vi "main4ChBK.vi"() -> ()   [LabVIEW 2024]
doc: "Main VI for FLS imaging system."
uses:
  <userlib>/_OpenG.lib/file/file.llb/openg_file.lvlib
  <vilib>/event_ctls.llb/usereventprio.ctl
  <instrlib>/niScope/Acquire/Fetch/niScope Multi Fetch Binary 16.vi
  <instrlib>/niScope/Controls/niScope trigger source.ctl
  <userlib>/_OpenG.lib/time/time.llb/openg_time.lvlib
  LaguerreDeconLib/DeconEngineClass/LaguerreDeconEngineClass.lvclass
  SubVI/GlobalVariables.vi
  SubVI/LabJack/LJ Pin Setting.ctl
  <vilib>/Utility/error.llb/DialogType.ctl
  <vilib>/Analysis/NI_AALBase.lvlib
  <vilib>/Utility/miscctls.llb/LVMinMaxIncTypeDef.ctl
  <vilib>/Analysis/baseanly.llb/Mean (DBL).vi
  <vilib>/Utility/miscctls.llb/LVPointTypeDef.ctl
  SubVI/APD/APDClass.lvclass
  ConfigFiles/AimingBeamVideoConfig.ctl
  <vilib>/addons/control/pid/NI_PID_pid.lvlib
  <vilib>/addons/control/pid/pid.llb/PID (DBL).vi
  <vilib>/Instr/_visa.llb/VISA Configure Serial Port (Instr).vi
  SubVI/DigitizerConfiguration/FLImDAQ.ctl
panel:
  out "Record Backlog 2":i32
  in  "Auto gain ch4":bool=TRUE caption="Auto gain ch3"
  in  "V 4":dbl caption="Gain 3" min=0.0 max=4.66 step=0.1
  out "Gain4":dbl
  out "Lifetime 4":dbl caption="Lifetime 3"
  out "IntR4":dbl format="%#_2g"
  out "SNR4":dbl format="%#_3g"
  out "Channel 4":dbl[][](graph) caption="Channel 3"
  out "RunStartTime":u32
  out "Dig1 Temp":dbl
  out "Dig2 Temp":dbl
  out "Visualization PC video source":T1
  in  "V target(1.0)":dbl=1.0 caption="V target(1.5)" min=0.3 max=1.5 step=0.1 format="%#_4g"
  out "SNR3":dbl format="%#_3g"
  out "SNR2":dbl format="%#_3g"
  out "SNR1":dbl format="%#_3g"
  in  "Show BG removed?":bool=TRUE
  out "IntR3":dbl format="%#_2g"
  out "IntR2":dbl format="%#_2g"
  out "IntR1":dbl format="%#_2g"
  in  "Video Display":bool
  out "Gain3":dbl
  out "Gain2":dbl
  out "Gain1":dbl
  in  "Skip Data Save?":bool
  out "Aq Loop?":bool
  out "ML?":bool
  out "aquisition loop Error Out":errorcluster
  out "Laser f (Hz)":dbl
  out "Record Backlog":i32
  out "Fetch Record #":i32
  out "Sync Success?":bool
  out "Disclamer":picture
  out "Calibration #":i8
  out "BG #":i8
  in  "TCP Connect":bool
  out "Help":string
  in  "355nm Laser toggle":bool caption="355nm 460Hz"
  in  "Cali&iRF alignment":bool
  in  "Background":bool
  in  "Aiming beam toggle":bool caption="445nm 15Hz 20mA"
  out "Lifetime 3":dbl
  out "Lifetime 2":dbl
  in  "Auto gain ch3":bool=TRUE
  in  "Auto gain ch2":bool=TRUE
  in  "Auto gain ch1":bool=TRUE
  out "Run #":i8
  in  "StopButton":bool caption="Stop"
  out "Aquisition Status:":bool
  in  "StartButton":bool caption="Start"
  in  "V 3":dbl caption="Gain 3" min=0.0 max=4.65 step=0.1
  in  "V 2":dbl caption="Gain 2" min=0.0 max=4.59 step=0.1
  out "Lifetime 1":dbl
  in  "V 1":dbl caption="Gain 1" min=0.0 max=4.63 step=0.1 format="%#_4g"
  in  "Video Source":enum32{"Camera", "FrameGrabber"}(radio)
  out "Case #":string
  out "System Hardware Connection Status":T2
  out "Channel 3":dbl[][](graph)
  out "Channel 2":dbl[][](graph)
  out "Channel 1":dbl[][](graph)
  in  "Tab Control":T3(tab)
  out "display loop timing(ms)":u32
  out "Aquisition loop timing(ms)":u32 format="%.2f"
  out "DisplayLoop":i32
  out "PID loop":i32 caption="processing loop"
  out "PID loop timing(ms)":u32 caption="processing loop timing(ms)"
  out "Communication loop(ms)":u32
  out "laser EM lamp V":dbl format="%0.6f"
  out "Decon Loop timing (ms)":dbl
  out "Auisition Loop idx":i32
  out "LJ process (ms)":u32
  out "LJ time(ms)":u32[](array[numeric])
  in  "Show BG":bool
  out "iRF length":i32
  out "BG length":i32
  out "data length":i32
  out "SysConfigCluster":T4
  out "LJ Pinout":T5={"Ch1 Bias"="DAC0", "Ch2 Bias"="DAC1", "Ch3 Bias"="DAC2", "Ch4 Bias"="DAC0", "355 PWM"="FIO0", "AimingBeam PWM"="FIO2", "Laser Ready"="FIO3", "Interlock"="FIO1", "Laser Start/Stop"="FIO1", "Red LED"="FIO1", "Green LED"="DIO3", "Foot Pedal"="DIO15"}
  out "FLImDAQ":T6={"Digitizer 1"="", "Digitizer 2"="", "Channel"=enum."Channel 0", "trigger source"="VAL_EXTERNAL", "trigger level"=0.5, "trigger delay"=1.35e-07, "min sample rate"=12500000000.0, "min record length"=2500, "vertical range"=1.0, "vertical offset"=-0.25, "Waveform to Avg"=2000} caption="FLIm DAQ Configuration" {"trigger delay" format="%^#.4e"; "trigger level" min=0.0 max=3.5 step=0.5 format="%.2f"; "vertical offset" format="%.4f"; "vertical range" format="%.2f"; "min sample rate" format="%#.2p"}
  in  "Sys Reconfig":bool
  out "data out(communcation loop)":string
  out "PID loop error out":errorcluster caption="processing Error Out"
  out "decon error out":errorcluster
  out "Laser Rep Rate":dbl
  out "V4 Size":i32 caption="V3 Size"
  in  "Data Class":enum16{"Data", "BG", "Cali"}(ring)
  out "V1 Size":i32
  out "V2 Size":i32
  out "V3 Size":i32
  out "data Size":i32[](array[numeric])
  out "State log":string
  in  "Ch4 PID gains":T8={"proportional gain (Kc)"=30.0, "integral time (Ti, min)"=0.0003, "derivative time (Td, min)"=1e-05}
  in  "Ch3 PID gains":T8={"proportional gain (Kc)"=30.0, "integral time (Ti, min)"=0.0003, "derivative time (Td, min)"=1e-05}
  in  "Ch2 PID gains":T8={"proportional gain (Kc)"=30.0, "integral time (Ti, min)"=0.0003, "derivative time (Td, min)"=1e-05}
  in  "Ch1 PID gains":T8={"proportional gain (Kc)"=30.0, "integral time (Ti, min)"=0.0003, "derivative time (Td, min)"=1e-05}
  in  "Quit":bool
  in  "Radio Buttons":T9(radio)=enum."Ch2" caption="DeCon Chan"
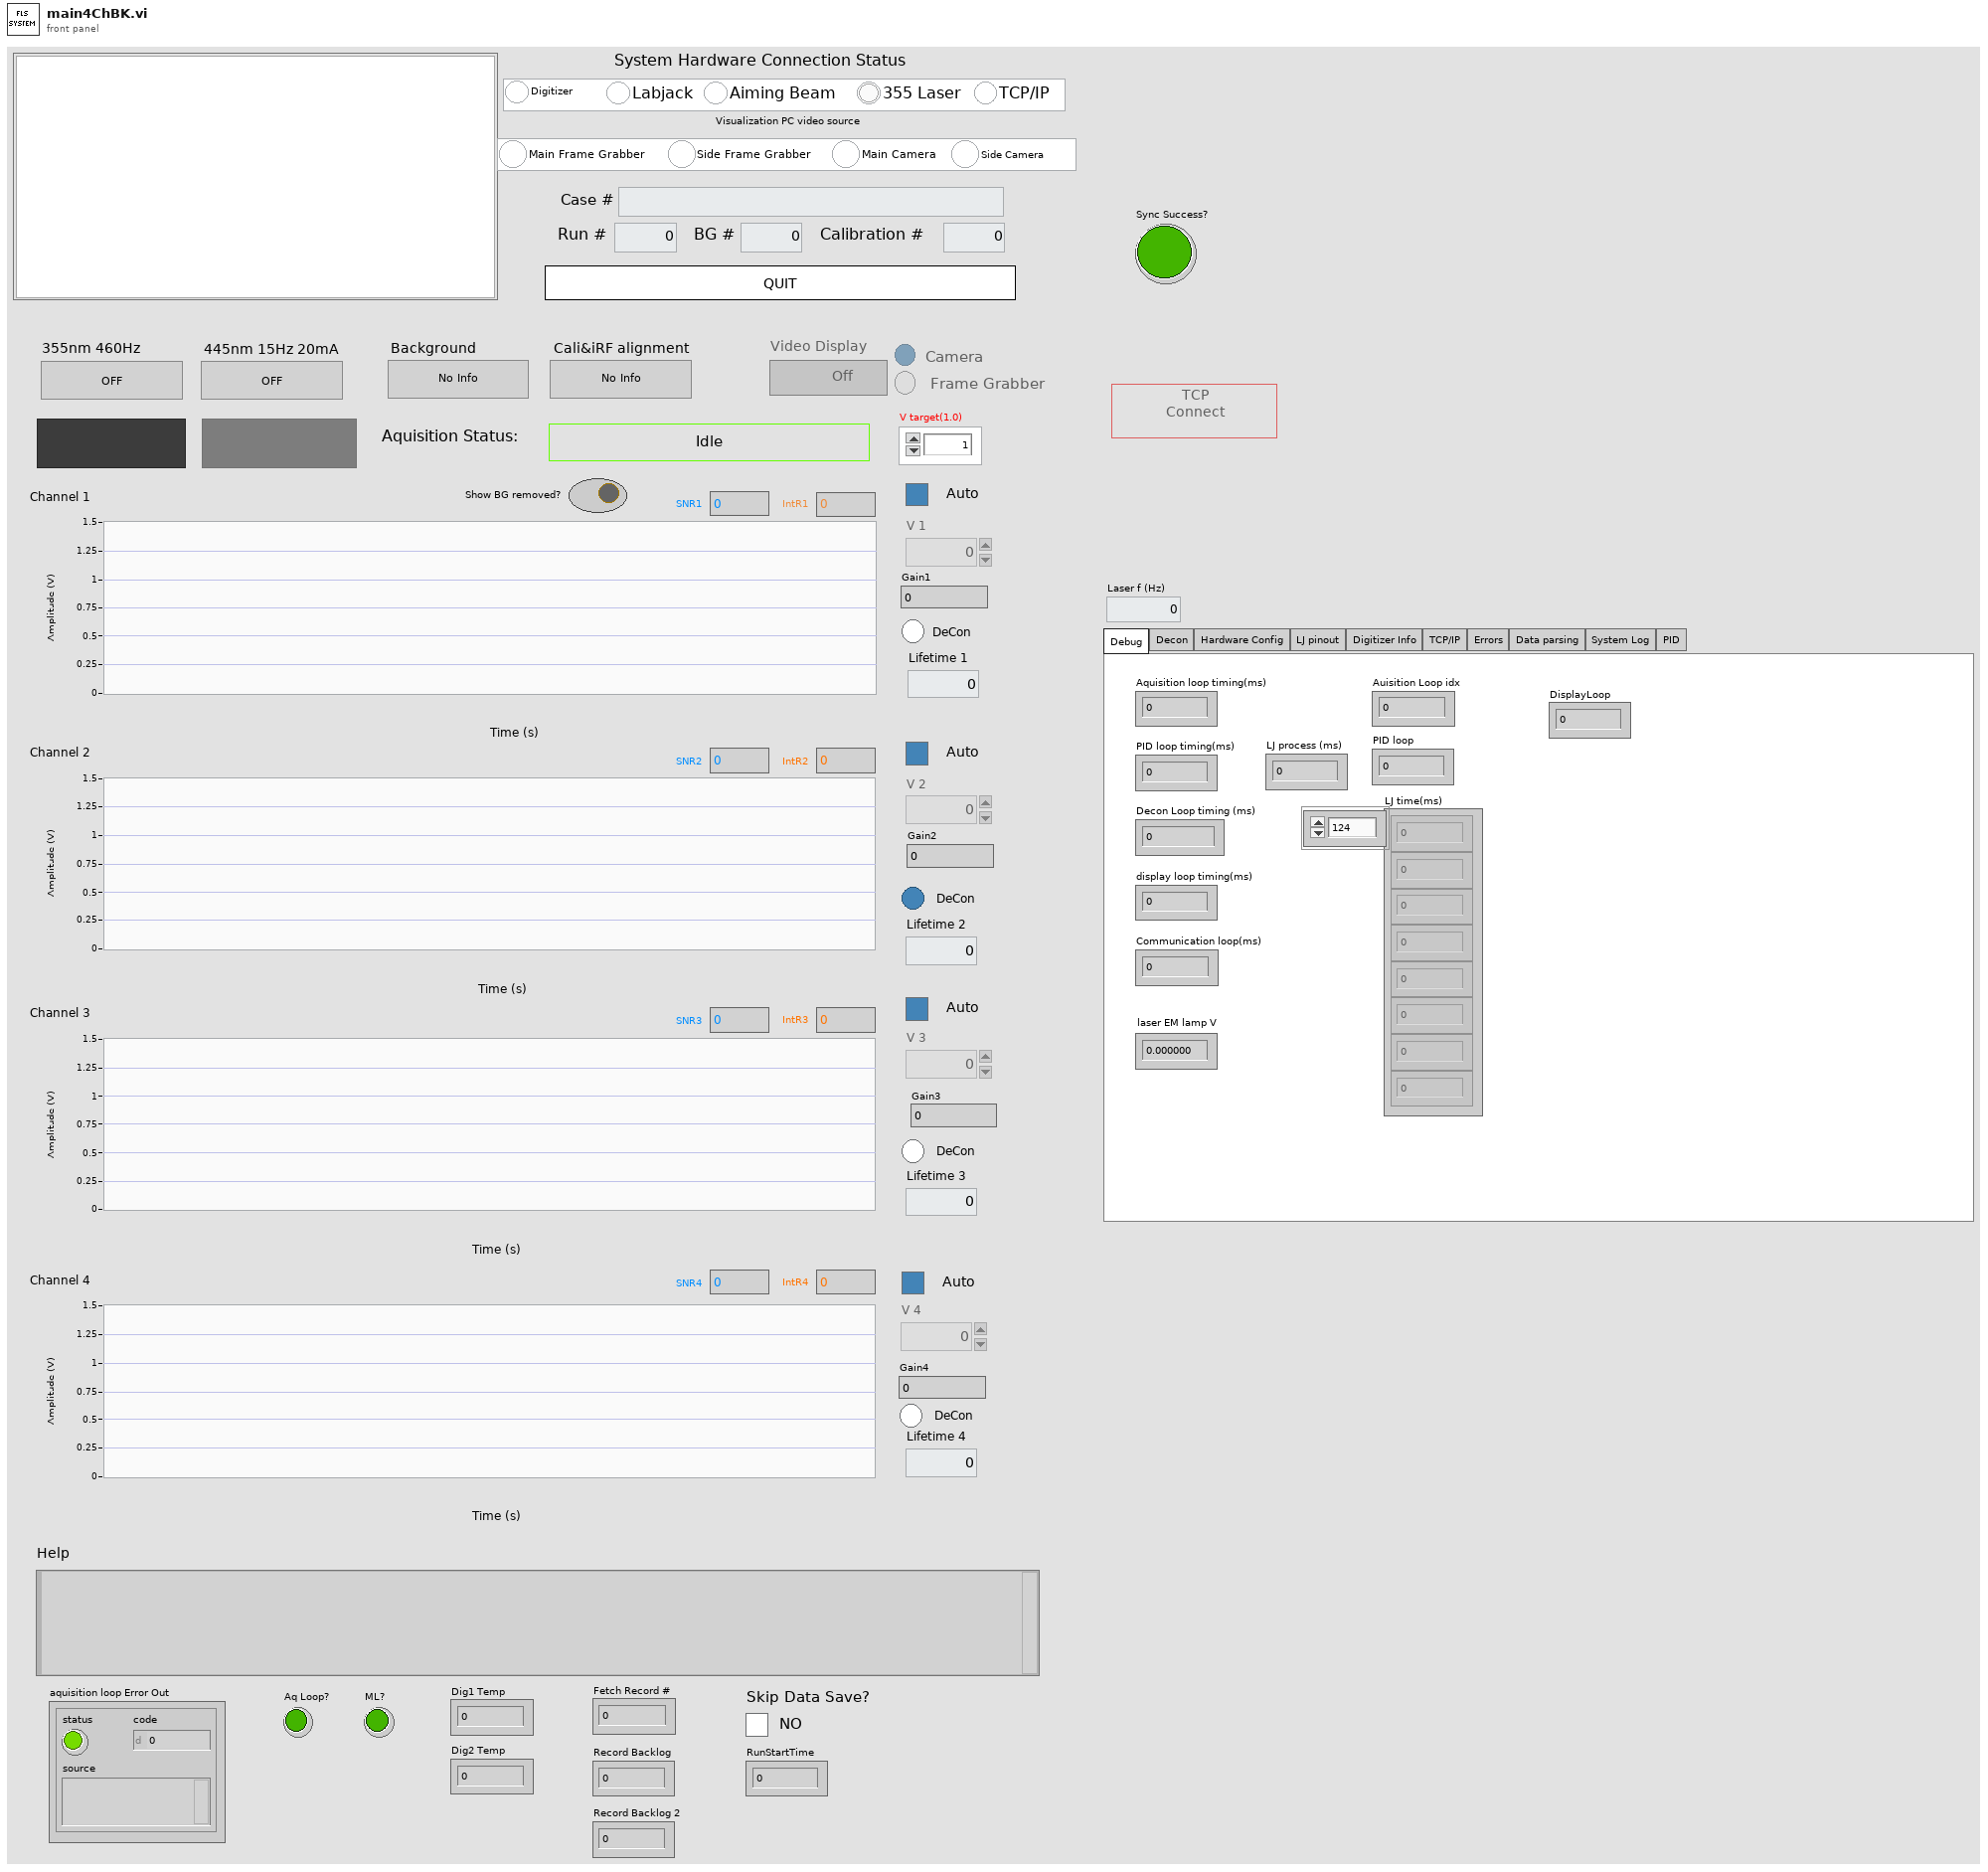
[diagram p1: front panel]
types:
  T1 = cluster{"Main Frame Grabber":bool, "Side Frame Grabber":bool, "Main Camera":bool, "Side Camera":bool}
  T2 = cluster{"Digitizer":bool, "Labjack":bool, "Aiming Beam":bool, "355 Laser":bool, "TCP/IP":bool}
  T3 = enum32{"Debug", "Decon", "Hardware Config", "LJ pinout", "Digitizer Info", "TCP/IP", "Errors", "Data parsing", "System Log", "PID"}
  T4 = cluster{"Ch1Enable?":bool, "Ch2Enable?":bool, "Ch3Enable?":bool, "Ch1AutoGain?":bool, "Ch2AutoGain?":bool, "Ch3AutoGain?":bool, "AimingBeamEnable?":bool}
  T5 = typedef "LJ Pin Setting.ctl" = cluster{"Ch1 Bias":string, "Ch2 Bias":string, "Ch3 Bias":string, "Ch4 Bias":string, "355 PWM":string, "AimingBeam PWM":string, "Laser Ready":string, "Interlock":string, "Laser Start/Stop":string, "Red LED":string, "Green LED":string, "Foot Pedal":string}
  T6 = typedef "FLImDAQ.ctl" = cluster{"Digitizer 1":refnum<k15>, "Digitizer 2":refnum<k15>, "Channel":enum16{"Channel 0", "Channel 1", "Channel 0&1"}, "trigger source":T7, "trigger level":dbl, "trigger delay":dbl, "min sample rate":dbl, "min record length":i32, "vertical range":dbl, "vertical offset":dbl, "Waveform to Avg":i16}
  T7 = typedef "niScope trigger source.ctl" = string
  T8 = cluster{"proportional gain (Kc)":dbl, "integral time (Ti, min)":dbl, "derivative time (Td, min)":dbl}
  T9 = enum32{"No Selection", "Ch1", "Ch2", "Ch3", "Ch4"}
  T10 = cluster{"remote start event":refnum<user-event>, "remote stop  event":refnum<user-event>}
  T11 = enum8{"Enabled", "Disabled", "Disabled and Grayed Out"}
  T12 = enum16{"open", "replace", "create", "open or create", "replace or create", "replace or create with confirmation"}
  T13 = cluster{"CH1":dbl[][], "CH2":dbl[][], "CH3":dbl[][], "CH4":dbl[][], "Gain cluster":cluster{"V1":dbl, "V2":dbl, "V3":dbl, "V4":dbl}}
  T14 = cluster{"idx":i32, "CH1&2":dbl[][], "CH3":dbl[][], "V cluster":cluster{"V1":dbl, "V2":dbl, "V3":dbl, "V4":dbl}}
  T15 = cluster{"Ch1 iRF":dbl[], "Ch2 iRF":dbl[], "Ch3 iRF":dbl[], "Ch4 iRF":dbl[]}
  T16 = enum16{"open", "open or create", "create or replace", "create", "open (read-only)"}
  T17 = enum32{"Invalid", "Standard", "Closed", "Hidden", "Minimized", "Maximized"}
  T18 = enum32{"invalid app kind", "Development System", "Run Time System", "Student Edition", "Embedded LabVIEW", "Evaluation", "Custom"}
  T19 = typedef "usereventprio.ctl" = enum32{"high priority", "normal priority"}
  T20 = enum32{"Bad", "Idle", "Run top level", "Running"}
  T21 = enum16{"Standard", "Buffered", "CRLF", "Immediate"}
  T22 = typedef "AimingBeamVideoConfig.ctl" = cluster{"DeCon Channel":enum16{"1", "2", "3"}, "Scale Bar":bool, "Scale Low":dbl, "Scale High":dbl, "ANSI":dbl, "Radius":dbl, "3D?":bool, "Firefly?":bool, "Pentero?":bool}
  T23 = cluster{"Core":cluster{"Current VI Reference":refnum<vi>, "Close Panel on Exit?":bool}, "SysConfigCluster":cluster{"Ch1Enable?":bool, "Ch2Enable?":bool, "Ch3Enable?":bool, "Ch1AutoGain?":bool, "Ch2AutoGain?":bool, "Ch3AutoGain?":bool, "AimingBeamEnable?":bool}, "System Status":cluster{"Digitizer":bool, "Labjack":bool, "Aiming Beam":bool, "355 Laser":bool, "TCP/IP":bool}, "IDs":cluster{"RunID":i8, "BG ID":i8, "Cali ID":i8}, "CaseID":string, "DefaultPath":path, "Pathes":cluster{"DataPath":path, "BG Path":path, "iRFPath":path, "CaliPath":path}, "FLImDAQ":cluster{"resource name":refnum<k15>, "resource name 2":refnum<k15>, "Channel":enum16{"Channel 0", "Channel 1", "Channel 0&1"}, "trigger source":T7, "trigger level":dbl, "trigger delay":dbl, "min sample rate":dbl, "min record length":i32, "vertical range":dbl, "vertical offset":dbl, "Waveform to Avg":i32}, "SysRunning?":bool, "AB Cluster":cluster{"Aiming Beam COM Port":refnum<visa-resource-name>, "Min Current":dbl, "Max Current":dbl, "Default Current":dbl, "Freq":i32}, "LJ Pinout":T5, "355 PWM setting":cluster{"DIO_EF_CLOCK1_DIVISOR":i16, "DIO_EF_CLOCK1_ROLL_VALUE":i32, "DIO#_EF_INDEX":i16, "DIO#_EF_OPTIONS":i16, "DIO#_EF_CONFIG_A":i32}, "AB PWM setting":cluster{"DIO_EF_CLOCK1_DIVISOR":i16, "DIO_EF_CLOCK1_ROLL_VALUE":i32, "DIO#_EF_INDEX":i16, "DIO#_EF_OPTIONS":i16, "DIO#_EF_CONFIG_A":i32}, "Last Trigger":u32, "niTClk sessions":refnum<k20>[], "Laser start tic":u32, "TCP attempt count":i32, "Ch1Data":dbl[][], "Ch2Data":dbl[][], "Ch3Data":dbl[][], "Ch4Data":dbl[][], "V1":dbl[], "V2":dbl[], "V3":dbl[], "V4":dbl[], "SlowTimer":u32, "FastTimer":u32, "listener ID":refnum<k5>, "TempPath":path, "CaliPath":path, "LED vi reference":refnum<vi>, "Aquisition Timer":u32, "APDSerialNum":cluster{"Ch1APDSerial#":string, "Ch2APDSerial#":string, "Ch3APDSerial#":string, "Ch4APDSerial#":string}, "VideoConfig":T22, "LED vi ref open?":bool, "video source":cluster{"Main Frame Grabber":bool, "Side Frame Grabber":bool, "Main Camera":bool, "Side Camera":bool}, "bothVidSourceAvail":bool}
  T24 = typedef "LVCursorListTypeDef.ctl" = cluster{"Name":string, "Color":u32, "Style":u8, "Point Style":u8, "Name Visible":bool, "Allow Drag":bool, "Cursor Mode":u32, "Plot":i32, "Index":i32, "Position":cluster{"X":dbl, "Y":dbl}, "X Scale":u32, "Y Scale":u32, "Watch Plots":i32[], "Watch All Plots":bool, "Plot Area":i32, "Label Offset":cluster{"X":dbl, "Y":dbl}}[]
  T25 = cluster{"Name":string, "Color":u32, "Style":u8, "Point Style":u8, "Name Visible":bool, "Allow Drag":bool, "Cursor Mode":u32, "Plot":i32, "Index":i32, "Position":cluster{"X":dbl, "Y":dbl}, "X Scale":u32, "Y Scale":u32, "Watch Plots":i32[], "Watch All Plots":bool, "Plot Area":i32, "Label Offset":cluster{"X":dbl, "Y":dbl}}
  T26 = cluster{"Ch1APDSerial#":string, "Ch2APDSerial#":string, "Ch3APDSerial#":string, "Ch4APDSerial#":string}
  T27 = cluster{"DataPath":path, "BG Path":path, "iRFPath":path, "CaliPath":path}
  T28 = cluster{"DIO_EF_CLOCK1_DIVISOR":i16, "DIO_EF_CLOCK1_ROLL_VALUE":i32, "DIO#_EF_INDEX":i16, "DIO#_EF_OPTIONS":i16, "DIO#_EF_CONFIG_A":i32}
  T29 = cluster{"Aiming Beam COM Port":refnum<visa-resource-name>, "Min Current":dbl, "Max Current":dbl, "Default Current":dbl, "Freq":i32}
  T30 = cluster{"resource name":refnum<k15>, "resource name 2":refnum<k15>, "Channel":enum16{"Channel 0", "Channel 1", "Channel 0&1"}, "trigger source":T7, "trigger level":dbl, "trigger delay":dbl, "min sample rate":dbl, "min record length":i32, "vertical range":dbl, "vertical offset":dbl, "Waveform to Avg":i32}
  T31 = cluster{"Current VI Reference":refnum<vi>, "Close Panel on Exit?":bool}
  T32 = typedef "iRFData.ctl" = cluster{"dt":dbl, "NumOfWFs":i32, "WFLength":i32, "iRFCtrlV":dbl[], "iRFWFsAvg":dbl[][], "iRFRaw":dbl[][]}
  T33 = cluster{"V 1":dbl[], "V 2":dbl[], "V 3":dbl[], "V 4":dbl[]}
  T34 = cluster{"Channel 1":dbl[], "Channel 2":dbl[], "Channel 3":dbl[], "Channel 4":dbl[]}
  T35 = cluster{"Ch1 WF":dbl[], "Ch2 WF":dbl[], "Ch3 WF":dbl[], "Ch4 WF":dbl[], "V1":dbl, "V2":dbl, "V3":dbl, "V4":dbl}
  T36 = cluster{"mean":dbl, "mean":dbl, "mean":dbl, "mean":dbl}
  T37 = cluster{"V1":dbl, "V2":dbl, "V3":dbl, "V4":dbl}[]
  T38 = cluster{"DataPath":path, "CaseID":string, "RunID":i16, "Ch1Data":dbl[][], "Ch2Data":dbl[][], "Ch3Data":dbl[][], "Ch4Data":dbl[][], "V1":dbl[], "V2":dbl[], "V3":dbl[], "V4":dbl[], "LaserRepRate":u16, "WFAverage":i16, "RunStartTime":u64}
  T39 = typedef "DialogType.ctl" = u16
  T40 = typedef "LJ PWM Setting.ctl" = cluster{"DIO_EF_CLOCK1_DIVISOR":i16, "DIO_EF_CLOCK1_ROLL_VALUE":i32, "DIO#_EF_INDEX":i16, "DIO#_EF_OPTIONS":i16, "DIO#_EF_CONFIG_A":i32}
  T41 = typedef "AimingBeam.ctl" = cluster{"Aiming Beam COM Port":refnum<visa-resource-name>, "Min Current":dbl, "Max Current":dbl, "Default Current":dbl, "Frequency(Hz)":u32}
  T42 = cluster{"DC1":i32, "DC2":i32, "BG1":i32, "BG2":i32}
  T43 = typedef "LVMinMaxIncTypeDef.ctl" = cluster{"Minimum":dbl, "Maximum":dbl, "Increment":dbl}
  T44 = typedef "LVBoundsTypeDef.ctl" = cluster{"Width":u32, "Height":u32}
  T45 = typedef "imagedata.ctl" = cluster{"image type":i32, "image depth":i32, "image":u8[], "mask":u8[], "colors":u32[], "Rectangle":cluster{"left":i16, "top":i16, "right":i16, "bottom":i16}}
  T46 = cluster{"DC Idx1":i32, "DC Idx2":i32, "BG Idx1":i32, "BG Idx2":i32}
  T47 = cluster{dbl[][], dbl[][], dbl[][], dbl[][], "V cluster":cluster{"V1":dbl, "V2":dbl, "V3":dbl, "V4":dbl}}
  T48 = typedef "LVPointTypeDef.ctl" = cluster{"Horizontal":i16, "Vertical":i16}
  T49 = cluster{"actualSamples":i32, "absoluteInitialX":dbl, "relativeInitialX":dbl, "xIncrement":dbl, "offset":dbl, "gain":dbl, "reserved1":dbl, "reserved2":dbl}[]
  T50 = cluster{"V1 out":dbl, "V2 out":dbl, "V3 out":dbl, "V3 out":dbl}
  T51 = cluster{i32, dbl[][], dbl[][], cluster{"V1 out":dbl, "V2 out":dbl, "V3 out":dbl, "V3 out":dbl}}
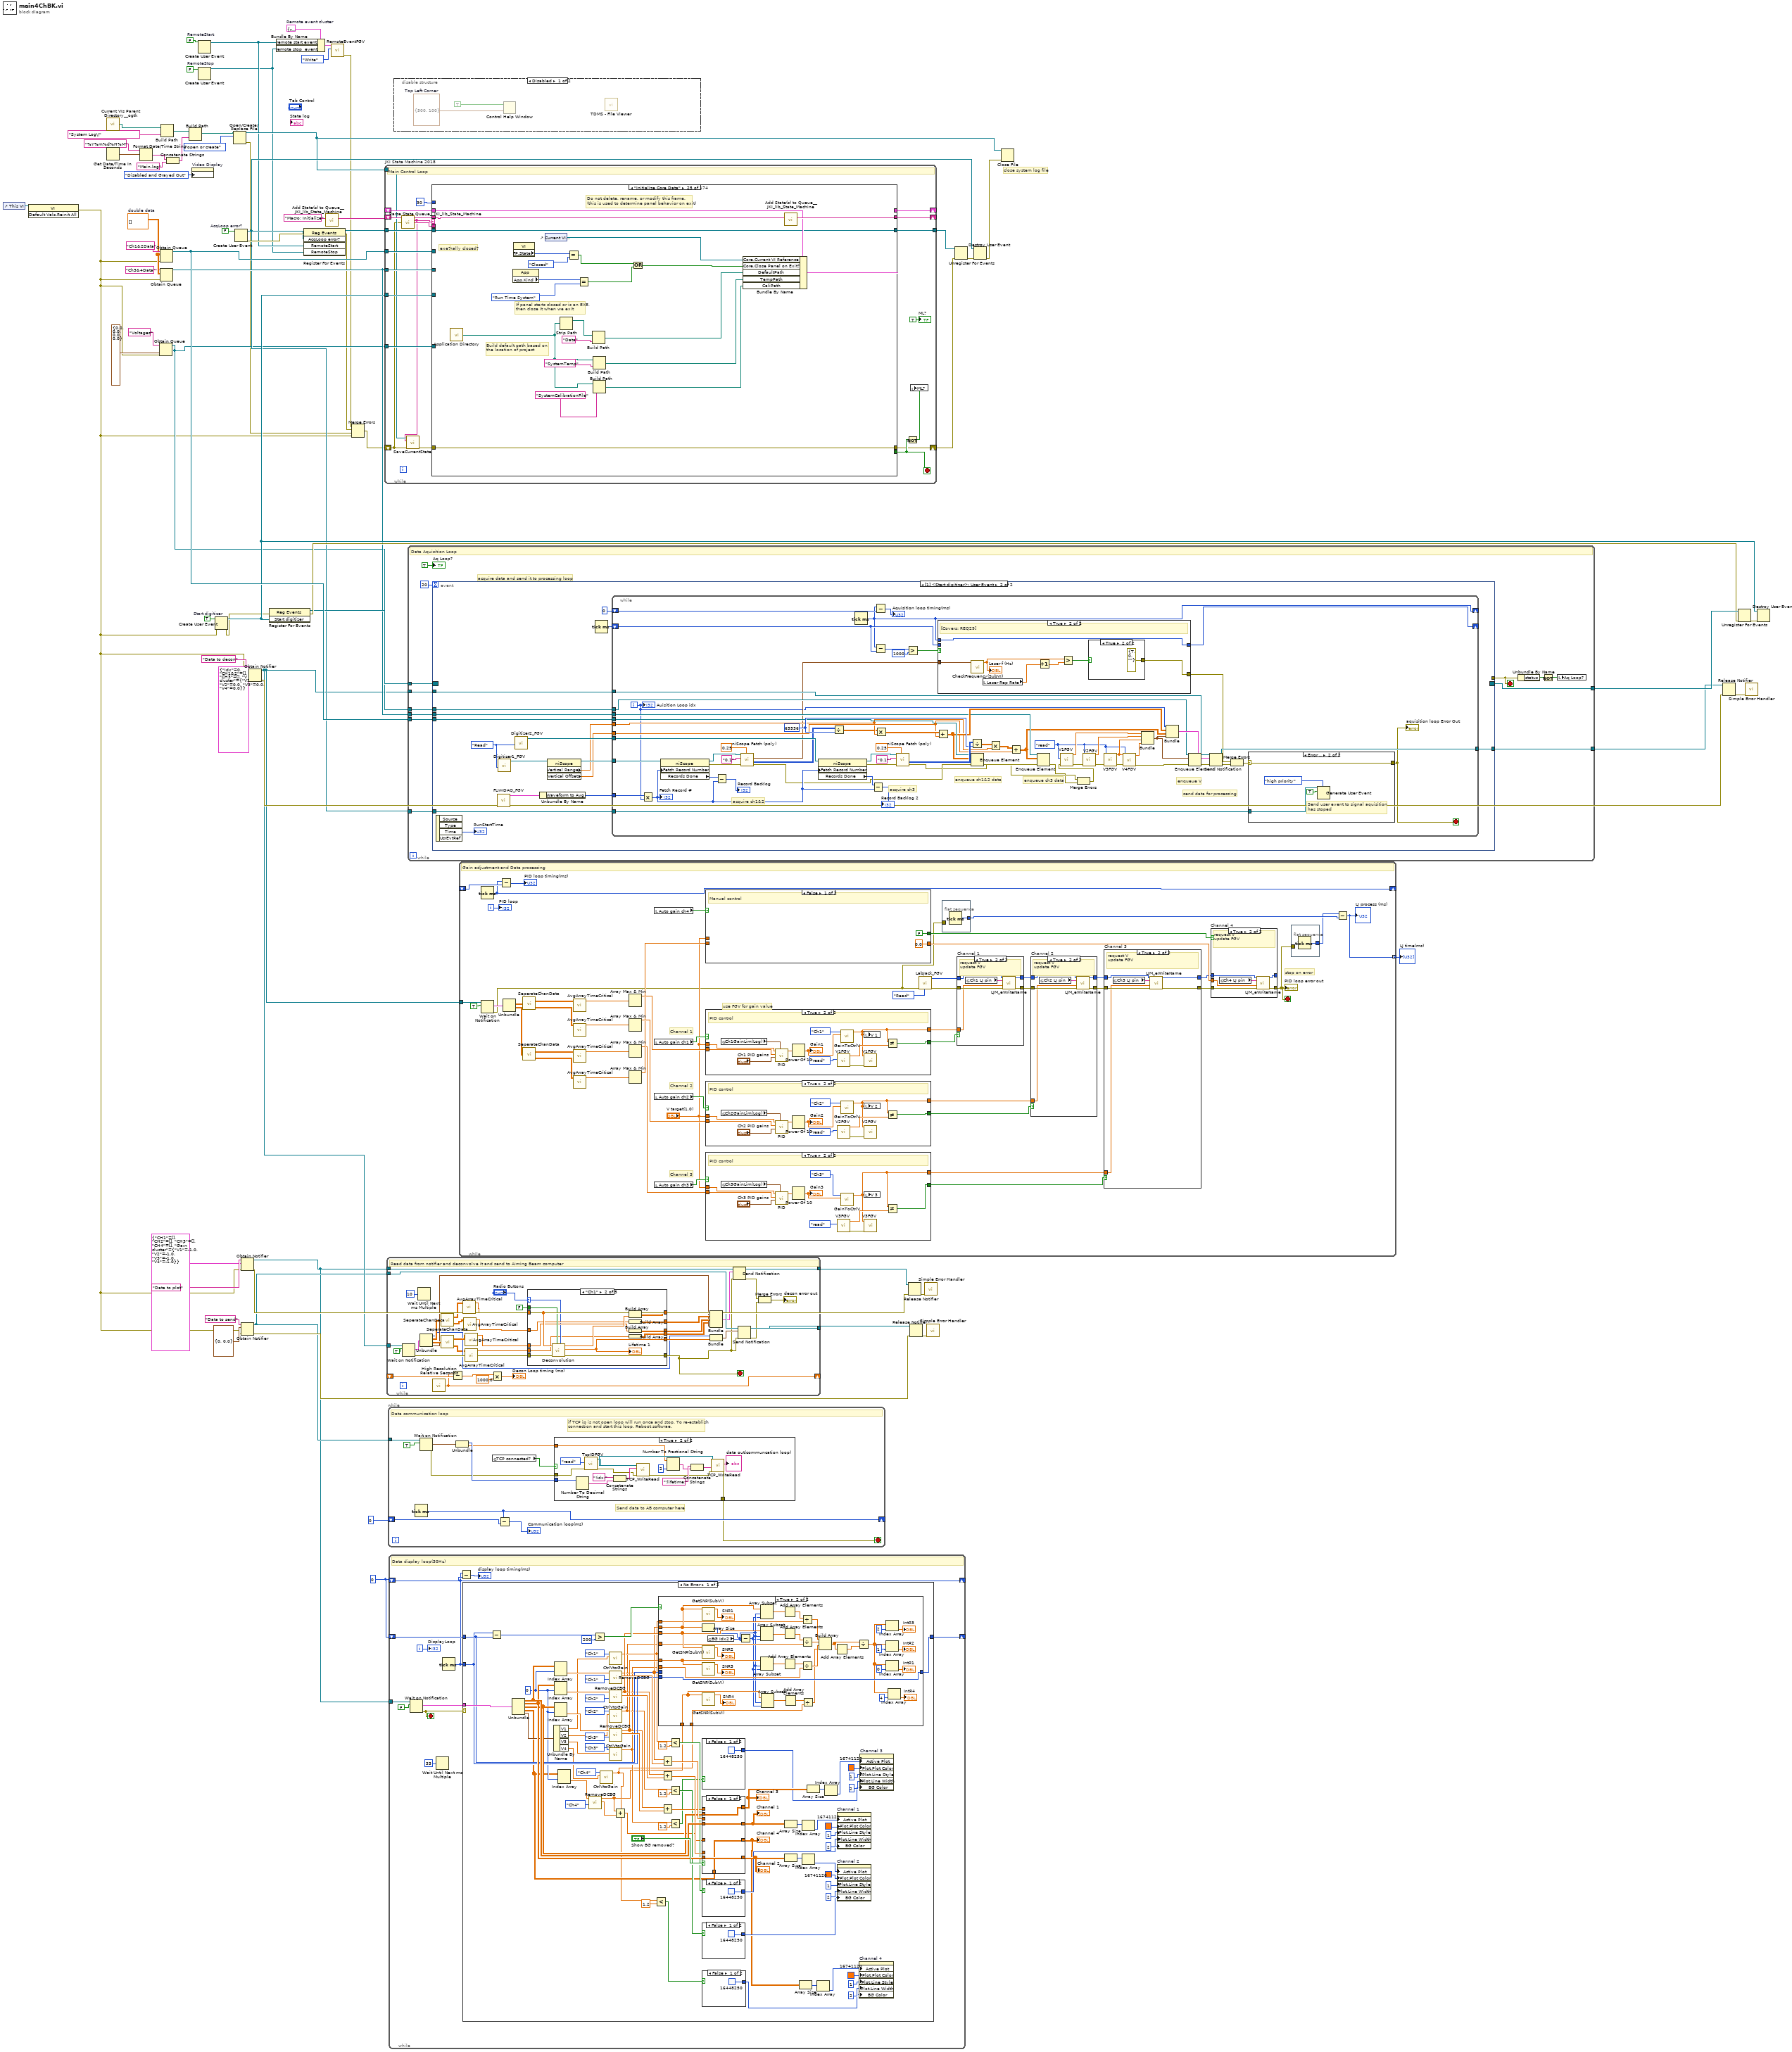
[diagram p0: block diagram]
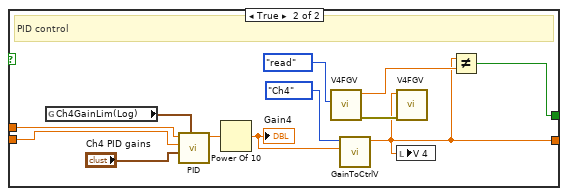
[diagram p6: hidden frame]
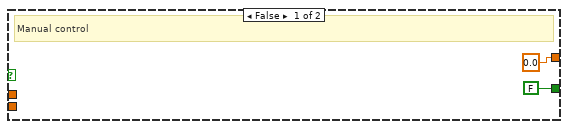
[diagram p7: hidden frame]
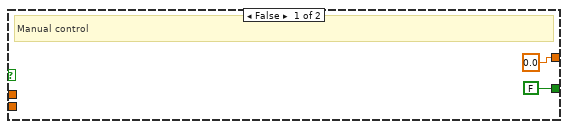
[diagram p8: hidden frame]
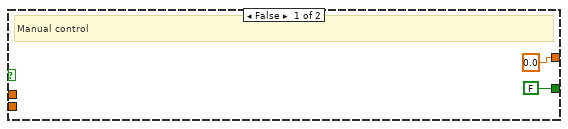
[diagram p9: hidden frame]
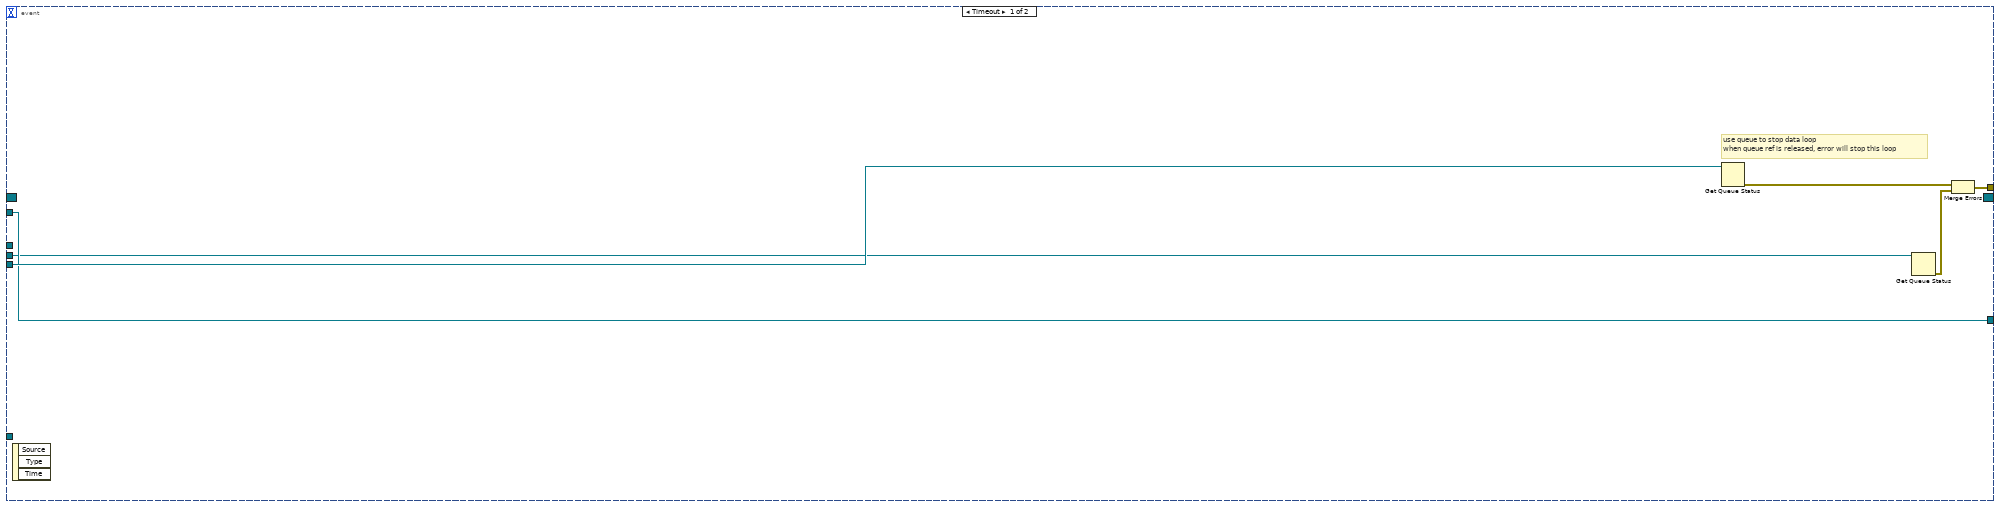
[diagram p10: hidden frame]
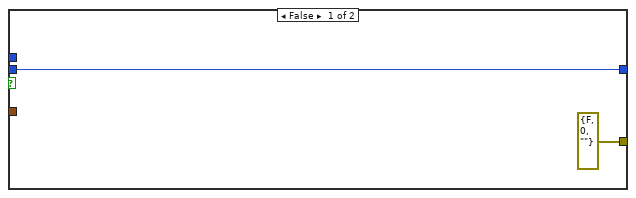
[diagram p11: hidden frame]
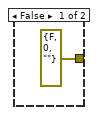
[diagram p12: hidden frame]
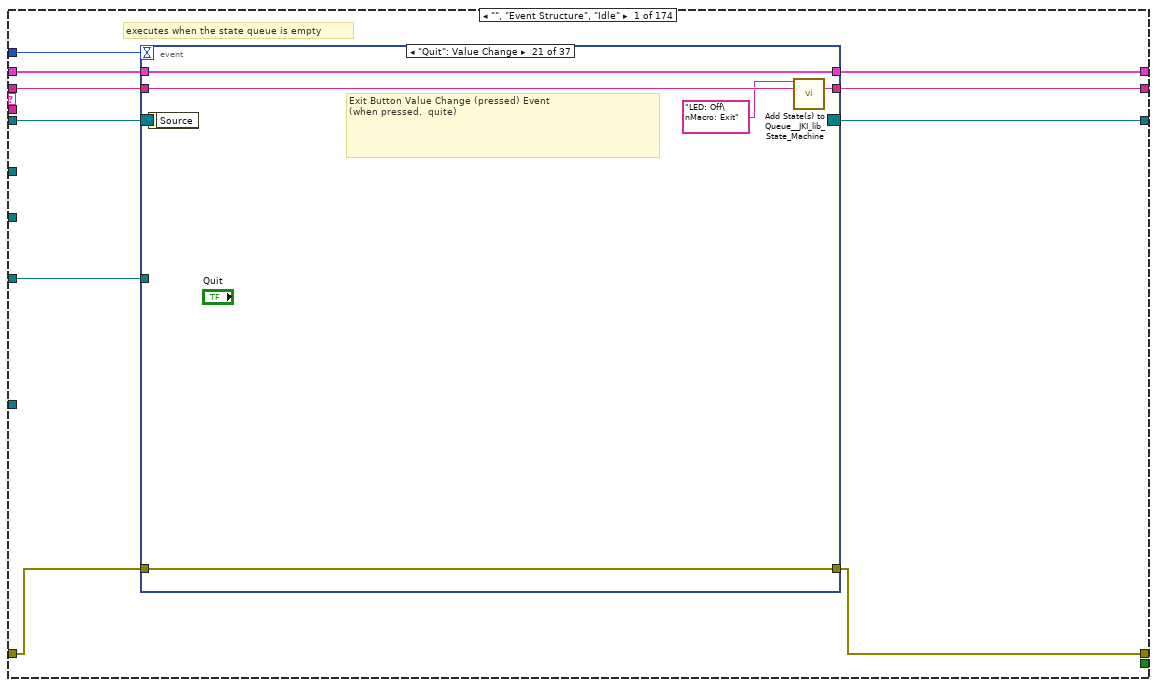
[diagram p14: hidden frame]
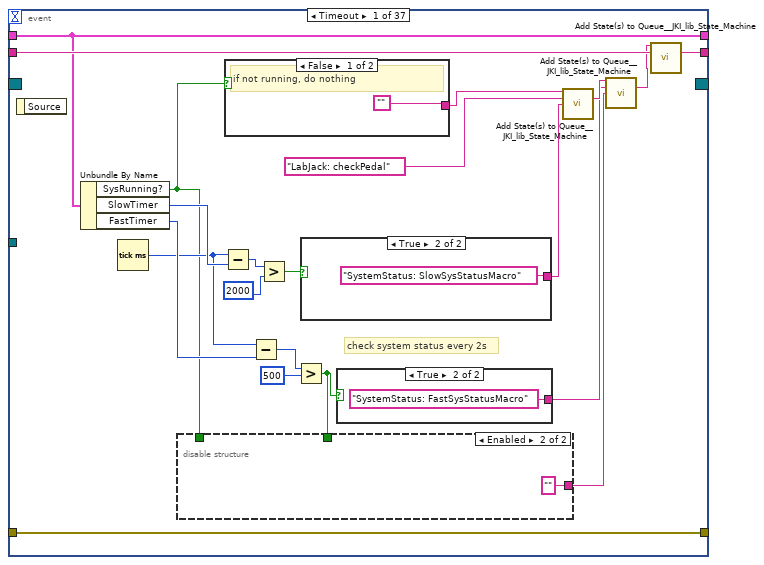
[diagram p15: hidden frame]
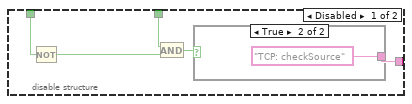
[diagram p16: hidden frame]
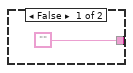
[diagram p17: hidden frame]
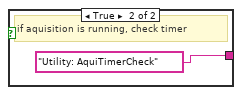
[diagram p18: hidden frame]
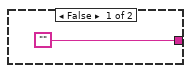
[diagram p19: hidden frame]
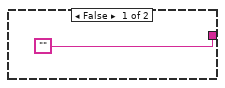
[diagram p20: hidden frame]
diagram:
  w8 = T10 {"remote start event"=refnum, "remote stop  event"=refnum}  # Remote event cluster
  w11 = FALSE  # RemoteStop
  w12 = FALSE  # RemoteStart
  w15 = u32 0 ("millisecond timer value")
  w54 = FALSE  # AcqLoop error?
  w64 = TRUE  # Start digitizer
  w67 = dbl[][] []  # double data
  # "close system log file"
  n1 = control-ref of="This VI"() -> (w69:refnum<vi>)
  n2 = invoke on="Invoke Node" class="VI" method="Default Vals.Reinit All"(reference=w69) -> (error out=w23:errorcluster)  [unwired: 2 in, 2 out]
  n3 = call <userlib>:"Current VIs Parent Directory__ogtk.vi"() -> ("Parent Directory (+ Relative)"=w34:path)  [unwired: 5 in]
  n4 = Get Date/Time In Seconds() -> (seconds since 1Jan1904=w32:timestamp)
  n5 = Format Date/Time String(time format string (%c)="%Y%m%d%H%M", seconds (now)=w32) -> (date/time string=w29:string)  [unwired: 1 in]
  n6 = Obtain Queue(name (unnamed)="Voltages", element data type=cluster{"V1":dbl, "V2":dbl, "V3":dbl, "V4":dbl} {"V1"=0.0, "V2"=0.0, "V3"=0.0, "V4"=0.0}, error in (no error)=w23) -> (queue out=w35:refnum<queue>)  [unwired: 2 in, 2 out]
  n7 = Obtain Queue(name (unnamed)="Ch3&4Data", element data type=w67, error in (no error)=w23) -> (queue out=w48:refnum<queue>)  [unwired: 2 in, 2 out]
  n8 = Obtain Queue(name (unnamed)="Ch1&2Data", element data type=w67, error in (no error)=w23) -> (queue out=w65:refnum<queue>)  [unwired: 2 in, 2 out]
  n9 = Build Path(base path=w34, name or relative path="System Log\\") -> (appended path=w25:path)
  n10 = Concatenate Strings(w29, "Main.log" ("string")) -> (w27:string)
  n11 = Build Path(base path=w25, name or relative path=w27) -> (appended path=w30:path)
  n12 = property on="Video Display" class="Bool (strict)"("DisabledEnum"=T11."Disabled and Grayed Out" ("Disabled")) -> ()  [unwired: 2 in, 2 out]
  n13 = Create User Event(user event datatype=w12) -> (user event=w10:refnum<user-event>)  [unwired: 1 in, 1 out]
  n14 = Create User Event(user event datatype=w11) -> (user event=w9:refnum<user-event>)  [unwired: 1 in, 1 out]
  n15 = Create User Event(user event datatype=w64, error in=w23) -> (user event=w53:refnum<user-event>, error out=w40:errorcluster)
  n16 = Open/Create/Replace File(file path (use dialog)=w30, operation (0:open)=T12."open or create") -> (refnum out=w21:refnum<file>, error out=w22:errorcluster)  [unwired: 4 in, 1 out]
  n17 = Create User Event(user event datatype=w54) -> (user event=w39:refnum<user-event>, error out=w41:errorcluster)  [unwired: 1 in]
  n18 = Obtain Notifier(name (unnamed)="Data to plot", notification data type=T13 {"CH1"=[], "CH2"=[], "CH3"=[], "CH4"=[], "Gain cluster"={"V1"=-1.0, "V2"=-1.0, "V3"=-1.0, "V4"=-1.0}}, error in (no error)=w23) -> (notifier out=w13:refnum<notifier>, error out=w49:errorcluster)  [unwired: 1 in, 1 out]
  n19 = Obtain Notifier(name (unnamed)="Data to send", notification data type=cluster{"idx":i32, "lifetime":dbl} {"idx"=0, "lifetime"=0.0}, error in (no error)=w23) -> (notifier out=w18:refnum<notifier>, error out=w38:errorcluster)  [unwired: 1 in, 1 out]
  n20 = Obtain Notifier(name (unnamed)="Data to decon", notification data type=T14 {"idx"=0, "CH1&2"=[], "CH3"=[], "V cluster"={"V1"=0.0, "V2"=0.0, "V3"=0.0, "V4"=0.0}}, error in (no error)=w23) -> (notifier out=w19:refnum<notifier>, error out=w58:errorcluster)  [unwired: 1 in, 1 out]
  n21 = register-events(error in=w40, w53) -> (reference out=w55:refnum<event-registration>, error out=w61:errorcluster)  [unwired: 1 in]
  n22 = Bundle By Name(cluster=w8, "remote start event"=w10, "remote stop  event"=w9) -> (w6:T10)
  n23 = register-events(error in=w41, w39, w10, w9) -> (reference out=w47:refnum<event-registration>, error out=w5:errorcluster)  [unwired: 1 in]
  n24 = call <vilib>:"Add State(s) to Queue__JKI_lib_State_Machine.vi"("State(s) in (\"\")"="Macro: Initialize") -> ("States Out"=w71:string)  [unwired: 14 in]
  n25 = call "RemoteEventFGV.vi"("Operation (Read)"=enum16{"Read", "Write"}."Write", "Remote Event in"=w6) -> ("Error Out"=w2:errorcluster)  [unwired: 8 in, 1 out]
  n26 = Merge Errors(w2, w5, w22, w23) -> (w24:errorcluster)
  n27 = while "JKI State Machine 2018" {
    shift-right: [w88] -> _
    shift-left: _ -> [w87]
    shift-right: [w72] -> w4
    shift-left: w24 -> [w74]
    shift-right: [w89] -> _
    shift-left: w71 -> [w90]
    tunnel: w65 -> [w85]
    tunnel: w48 -> [w84]
    tunnel: w53 -> [w83]
    tunnel: w47 -> [w82]
    tunnel: [w81] -> w46
    tunnel: w35 -> [w77]
    tunnel: w21 -> [w76]
    stop <- w80 stop-if-true
    # "Main Control Loop"
    n28 = call <vilib>:"Parse State Queue__JKI_lib_State_Machine.vi"("State Queue"=w90, "Error In (no error)"=w74) -> ("Remaining States"=w92:string, "Current State"=w75:string, "Arguments"=w91:string)  [unwired: 11 in]
    n29 = call "SaveCurrentState.vi"("error in (no error)"=w74, "Current State"=w75, "Byte Stream File in"=w76) -> ("error out"=w73:errorcluster)  [unwired: 8 in]
    n30 = case shown="\"Initialize Core Data\"" w75 {
      selector: w75 -> [_ _ _ _ _ _ _ _ _ _ _ _ _ _ _ _ _ _ _ _ _ _ _ w1018 _ _ _ _ _ _ _ _ _ _ _ _ _ _ _ _ _ _ _ _ _ _ _ _ _ _ _ _ _ _ _ _ _ _ _ _ _ _ _ _ _ _ _ _ _ _ _ _ _ _ _ _ _ _ _ _ _ _ _ _ _ _ _ _ _ _ _ _ _ _ _ _ _ _ _ _ _ _ _ _ _ _ _ _ _ _ _ _ _ _ _ _ _ _ _ _ _ _ _ _ _ _ _ _ _ _ _ _ _ _ _ _ _ _ _ _ _ _ _ _ _ _ _ _ _ _ _ _ _ _ _ _ _ _ _ _ _ _ _ _ _ _ _ _ _ _ _ _ _ _]
      tunnel: w92 -> [w102 w478 w487 w493 w499 w521 w534 w576 w620 w635 w665 w708 w721 w748 w780 w794 w823 w837 w922 w959 w998 w1011 w1016 w1022 w1050 w1058 w1081 w1086 w1099 w1118 w1146 w1174 w1212 w1217 w1223 w1249 w1275 w1301 w1327 w1332 w1349 w1396 w1418 w1434 w1449 w1469 w1474 w1486 w1515 w1541 w1553 w1591 w1604 w1610 w1621 w1633 w1664 w1677 w1691 w1706 w1725 w1760 w1765 w1779 w1789 w1805 w1817 w1829 w1857 w1872 w1877 w1888 w1900 w1905 w1913 w1921 w1930 w1939 w1944 w1952 w1961 w1979 w1996 w2016 w2027 w2049 w2064 w2081 w2086 w2094 w2102 w2107 w2115 w2122 w2130 w2137 w2147 w2175 w2183 w2190 w2198 w2203 w2211 w2218 w2224 w2233 w2249 w2254 w2261 w2273 w2343 w2355 w2364 w2381 w2390 w2413 w2430 w2441 w2454 w2479 w2502 w2508 w2524 w2546 w2554 w2560 w2565 w2572 w2582 w2594 w2603 w2608 w2620 w2625 w2635 w2641 w2647 w2652 w2657 w2662 w2672 w2694 w2713 w2718 w2729 w2754 w2781 w2804 w2809 w2824 w2875 w2921 w2966 w2977 w2995 w3015 w3029 w3042 w3050 w3067 w3089 w3113 w3132 w3150 w3168 w3186 w3200 w3214 w3233 w3247 w3262 w3277 w3286 w3291]
      tunnel: w91 -> [_ _ _ _ _ _ _ _ _ _ _ _ _ _ _ _ _ _ _ _ _ _ _ _ _ _ _ _ _ _ _ _ _ _ _ _ _ _ _ _ _ _ _ _ _ _ _ _ _ _ _ _ _ _ _ w1631 _ _ _ _ _ _ _ _ _ _ _ _ _ _ _ _ _ _ _ _ _ _ _ _ _ _ _ _ _ _ _ _ _ _ _ _ _ _ _ _ w2138 _ _ _ _ _ _ _ _ _ _ _ w2256 w2267 _ _ _ _ w2387 _ _ _ _ _ w2498 _ _ _ _ _ _ w2567 _ _ _ _ _ _ w2631 _ _ _ _ _ _ _ _ _ _ _ _ _ _ _ _ _ _ _ _ _ _ _ _ _ _ _ _ _ _ _ _ _ _ _ _ _ _ _]
      tunnel: w87 -> [w100 w475 w483 w490 w496 w518 w531 _ w617 w625 w661 w704 w717 w740 w771 w791 w820 w834 w882 w951 w986 w1006 w1013 w1020 w1043 w1055 w1079 w1083 w1087 w1108 w1138 w1166 w1208 w1214 w1220 w1227 w1254 w1280 w1306 w1329 w1342 w1386 w1415 w1419 w1446 w1466 w1471 w1475 w1504 w1531 w1546 w1574 w1602 w1607 w1614 w1629 w1647 w1672 w1683 w1701 w1718 w1743 w1762 w1775 w1783 w1802 w1814 w1826 w1845 w1861 w1874 w1886 w1898 w1902 w1907 w1914 w1926 w1935 w1941 w1948 w1958 w1966 w1983 w2011 w2017 w2046 w2057 w2079 w2083 w2087 w2095 w2104 w2113 w2119 w2127 w2134 w2144 w2172 w2180 w2187 w2195 w2200 w2205 w2216 w2221 w2227 w2246 w2251 w2259 w2269 w2340 w2345 w2358 w2379 w2388 w2403 w2427 w2438 w2448 w2472 w2499 w2505 w2517 w2542 w2551 w2557 w2562 w2569 w2576 w2590 w2600 w2605 w2617 w2622 w2628 w2638 w2644 w2649 w2654 w2659 w2669 w2692 w2711 w2715 w2727 w2752 w2779 w2802 w2806 w2817 w2869 w2917 w2963 w2973 w2990 w3010 w3024 w3038 w3044 w3062 w3084 w3108 w3127 w3145 w3163 w3181 w3195 w3209 w3228 w3242 w3257 w3274 w3284 w3288]
      tunnel: [w93 w476 w485 w491 w497 w519 w532 w574 w586 w633 w657 w700 w719 w728 w760 w784 w811 w835 w858 w948 w985 w1007 w1014 w1024 w1047 errorcluster {"status"=FALSE, "code"=0, "source"=""} ("error out") w1078 w1084 w1097 w1116 w1130 w1153 w1210 w1215 w1221 w1228 w1255 w1281 w1307 w1330 w1333 w1378 w1409 w1423 w1447 w1457 w1472 w1478 w1502 w1530 w1545 w1561 w1596 w1608 w1619 w1623 w1638 w1667 w1679 w1697 w1717 w1734 w1763 w1767 w1785 w1800 w1812 w1824 w1847 w1862 w1875 w1878 w1895 w1903 w1911 w1919 w1923 w1932 w1942 w1945 w1954 w1969 w1991 w2010 w2021 w2039 w2061 w2077 w2084 w2092 w2100 w2105 w2112 w2120 w2128 w2135 w2145 w2173 w2181 w2188 w2196 w2201 w2209 w2215 w2222 w2230 w2247 w2252 w2257 w2270 w2341 w2349 w2361 w2371 w2384 w2404 w2428 w2437 w2450 w2474 w2500 w2506 w2514 w2536 w2552 w2558 w2563 w2570 w2580 w2592 w2601 w2606 w2618 w2623 w2633 w2639 w2645 w2650 w2655 w2660 w2670 w2682 w2704 w2716 w2720 w2739 w2771 w2796 w2807 w2811 w2870 w2918 w2964 w2972 w2992 w3012 w3026 w3040 w3046 w3064 w3086 w3110 w3129 w3147 w3165 w3183 w3197 w3211 w3230 w3244 w3258 w3275 w3282 w3289] -> w72
      tunnel: w73 -> [w99 w476 w485 w491 w497 w519 w532 w574 w586 w633 w655 w701 w719 w729 w767 w784 w801 w835 w858 w949 w988 w1008 w1014 w1023 w1047 w1051 w1078 w1084 w1097 w1116 w1129 w1165 w1210 w1215 w1221 w1232 w1259 w1285 w1311 w1330 w1340 w1381 w1408 w1422 w1447 w1459 w1472 w1477 w1503 w1521 w1551 w1572 w1595 w1608 w1616 w1626 w1637 w1666 w1682 w1696 w1716 w1733 w1763 w1773 w1786 w1799 w1811 w1823 w1846 w1863 w1875 w1882 w1890 w1903 w1911 w1919 w1922 w1931 w1942 w1946 w1955 w1974 w1990 w2009 w2020 w2045 w2060 w2076 w2084 w2092 w2100 w2105 w2112 w2120 w2128 w2135 w2145 w2173 w2181 w2188 w2196 w2201 w2209 w2215 w2222 w2230 w2247 w2252 w2258 w2271 w2341 w2350 w2360 w2367 w2383 w2405 w2428 w2437 w2445 w2477 w2500 w2506 w2519 w2535 w2552 w2558 w2563 w2570 w2580 w2592 w2601 w2606 w2618 w2623 w2633 w2639 w2645 w2650 w2655 w2660 w2670 w2681 w2703 w2716 w2719 w2738 w2761 w2787 w2807 _ w2871 w2918 w2964 w2971 w2991 w3011 w3025 w3040 w3045 w3063 w3085 w3109 w3128 w3146 w3164 w3182 w3196 w3210 w3229 w3243 w3256 w3275 w3281 w3289]
      tunnel: [w101 w477 w486 w492 w498 w520 w533 w575 w619 w634 w664 w707 w720 w747 w779 w793 w822 w836 w921 w958 w997 w1010 w1015 w1021 w1049 w1057 w1080 w1085 w1098 w1117 w1145 w1173 w1211 w1216 w1222 w1248 w1274 w1300 w1326 w1331 w1348 w1395 w1417 w1433 w1448 w1468 w1473 w1485 w1514 w1540 w1552 w1590 w1603 w1609 w1620 w1632 w1663 w1676 w1690 w1705 w1724 w1759 w1764 w1778 w1788 w1804 w1816 w1828 w1856 w1871 w1876 w1887 w1899 w1904 w1912 w1920 w1929 w1938 w1943 w1951 w1960 w1978 w1995 w2015 w2026 w2048 w2063 w2080 w2085 w2093 w2101 w2106 w2114 w2121 w2129 w2136 w2146 w2174 w2182 w2189 w2197 w2202 w2210 w2217 w2223 w2232 w2248 w2253 w2260 w2272 w2342 w2354 w2363 w2380 w2389 w2412 w2429 w2440 w2453 w2478 w2501 w2507 w2523 w2545 w2553 w2559 w2564 w2571 w2581 w2593 w2602 w2607 w2619 w2624 w2634 w2640 w2646 w2651 w2656 w2661 w2671 w2693 w2712 w2717 w2728 w2753 w2780 w2803 w2808 w2823 w2874 w2920 w2965 w2976 w2994 w3014 w3028 w3041 w3049 w3066 w3088 w3112 w3131 w3149 w3167 w3185 w3199 w3213 w3232 w3246 w3261 w3276 w3285 w3290] -> w89
      tunnel: [_ _ _ _ _ _ _ _ _ _ _ _ _ _ _ _ _ _ _ _ _ _ _ _ _ _ TRUE _ _ _ _ _ _ _ _ _ _ _ _ _ _ _ _ _ _ _ _ _ _ _ _ _ _ _ _ _ _ _ _ _ _ _ _ _ _ _ _ _ _ _ _ _ _ _ _ _ _ _ _ _ _ _ _ _ _ _ _ _ _ _ _ _ _ _ _ _ _ _ _ _ _ _ _ _ _ _ _ _ _ _ _ _ _ _ _ _ _ _ _ _ _ _ _ _ _ _ _ _ _ _ _ _ _ _ _ _ _ _ _ _ _ _ _ _ _ _ _ _ _ _ _ _ _ _ _ _ _ _ _ _ _ _ _ _ _ _ _ _ _ _ _ _ _ _] -> w80
      tunnel: [w98 w475 w483 w490 w496 w518 w531 w549 w617 w625 w661 w704 w717 w740 w771 w791 w820 w834 w882 w952 w987 w1006 w1013 w1020 w1048 w1055 w1079 w1083 w1088 w1109 w1139 w1167 w1209 w1214 w1220 w1227 w1254 w1280 w1306 w1329 w1342 w1387 w1415 w1420 w1446 w1467 w1471 w1476 w1504 w1531 w1550 w1574 w1602 w1607 w1617 w1629 w1647 w1672 w1683 w1701 w1718 w1743 w1762 w1776 w1783 w1802 w1814 w1826 w1845 w1861 w1874 w1886 w1898 w1902 w1908 w1915 w1927 w1936 w1941 w1949 w1959 w1967 w1989 w1998 w2022 w2047 w2058 w2079 w2083 w2088 w2096 w2104 w2113 w2119 w2127 w2134 w2144 w2172 w2180 w2187 w2195 w2200 w2205 w2216 w2221 w2227 w2246 w2251 w2259 w2269 w2340 w2346 w2359 w2379 w2388 w2403 w2427 w2438 w2449 w2473 w2499 w2505 w2518 w2542 w2551 w2557 w2562 w2569 w2577 w2590 w2600 w2605 w2617 w2622 w2628 w2638 w2644 w2649 w2654 w2659 w2669 w2692 w2711 w2715 w2727 w2752 w2779 w2802 w2806 w2822 w2868 w2917 w2963 w2973 w2990 w3010 w3024 w3038 w3044 w3062 w3084 w3108 w3127 w3145 w3163 w3181 w3195 w3209 w3228 w3242 w3259 w3274 w3284 w3288] -> w88
      tunnel: 30 ("Timeout") -> [w97 _ _ _ _ _ _ _ _ _ _ _ _ _ _ _ _ _ _ _ _ _ _ _ _ _ _ _ _ _ _ _ _ _ _ _ _ _ _ _ _ _ _ _ _ _ _ _ _ _ _ _ _ _ _ _ _ _ _ _ _ _ _ _ _ _ _ _ _ _ _ _ _ _ _ _ _ _ _ _ _ _ _ _ _ _ _ _ _ _ _ _ _ _ _ _ _ _ _ _ _ _ _ _ _ _ _ _ _ _ _ _ _ _ _ _ _ _ _ _ _ _ _ _ _ _ _ _ _ _ _ _ _ _ _ _ _ _ _ _ _ _ _ _ _ _ _ _ _ _ _ _ _ _ _ _ _ _ _ _ _ _ _ _ _ _ _ _ _ _ _ _ _ _]
      tunnel: w85 -> [_ _ _ _ _ _ _ _ _ _ _ _ _ _ _ _ _ _ _ w956 _ _ _ _ _ _ _ _ _ _ _ _ _ _ _ _ _ _ _ _ _ _ _ _ _ _ _ _ _ _ _ _ _ _ _ _ _ _ _ _ _ _ _ _ _ _ _ _ _ _ _ w1883 w1894 _ _ _ _ _ _ _ _ _ _ _ _ _ _ _ _ _ _ _ _ _ _ _ _ _ _ _ _ _ _ _ _ _ _ _ _ _ _ _ _ _ _ _ _ _ _ _ _ _ _ _ _ _ _ _ _ _ _ _ _ _ _ _ _ _ _ _ _ _ _ _ _ _ _ _ _ _ _ _ _ _ _ _ _ _ _ _ _ _ _ _ _ _ _ _ _ _ _ _ _ _]
      tunnel: w84 -> [_ _ _ _ _ _ _ _ _ _ _ _ _ _ _ _ _ _ _ w955 _ _ _ _ _ _ _ _ _ _ _ _ _ _ _ _ _ _ _ _ _ _ _ _ _ _ _ _ _ _ _ _ _ _ _ _ _ _ _ _ _ _ _ _ _ _ _ _ _ _ _ w1884 w1893 _ _ _ _ _ _ _ _ _ _ _ _ _ _ _ _ _ _ _ _ _ _ _ _ _ _ _ _ _ _ _ _ _ _ _ _ _ _ _ _ _ _ _ _ _ _ _ _ _ _ _ _ _ _ _ _ _ _ _ _ _ _ _ _ _ _ _ _ _ _ _ _ _ _ _ _ _ _ _ _ _ _ _ _ _ _ _ _ _ _ _ _ _ _ _ _ _ _ _ _ _]
      tunnel: w83 -> [w96 _ _ _ _ _ _ _ _ _ _ _ _ _ _ _ _ _ _ _ _ _ _ _ _ _ _ _ _ _ _ _ _ _ _ _ _ _ _ _ _ _ w1411 _ _ _ _ _ _ _ _ _ _ _ _ _ _ _ _ _ _ _ _ _ _ _ _ _ _ _ _ _ _ _ _ _ _ _ _ _ _ _ _ _ _ _ _ _ _ _ _ _ _ _ _ _ _ _ _ _ _ _ _ _ _ _ _ _ _ _ _ _ _ _ _ _ _ _ _ _ _ _ _ _ _ _ _ _ _ _ _ _ _ _ _ _ _ _ _ _ _ _ _ _ _ _ _ _ _ _ _ _ _ _ _ _ _ _ _ _ _ _ _ _ _ _ _ _ _ _ _ _ _ _]
      tunnel: w82 -> [w95 w474 w484 w489 w495 w510 w530 w559 w618 w632 w663 w706 w718 w746 w778 w792 w821 w833 w920 w957 w996 w1005 w1012 w1017 w1035 w1054 w1077 w1082 w1096 w1115 w1144 w1164 w1207 w1213 w1219 w1226 w1253 w1279 w1305 w1328 w1337 w1361 w1416 w1432 w1445 w1454 w1470 w1484 w1513 w1539 w1544 w1589 w1594 w1606 w1613 w1622 w1634 w1665 w1681 w1695 w1715 w1730 w1761 w1777 w1787 w1803 w1815 w1827 w1855 w1858 w1873 w1885 w1892 w1901 w1910 w1918 w1925 w1934 w1940 w1950 w1953 w1965 w1984 w1999 w2018 w2044 w2062 w2078 w2082 w2090 w2098 w2103 w2111 w2118 w2126 w2133 w2143 w2171 w2179 w2186 w2191 w2199 w2208 w2214 w2220 w2229 w2241 w2250 w2255 w2266 w2339 w2344 w2356 w2366 w2382 w2411 w2426 w2439 w2451 w2475 w2495 w2503 w2516 w2544 w2549 w2555 w2561 w2568 w2579 w2591 w2599 w2604 w2616 w2621 w2632 w2637 w2643 w2648 w2653 w2658 w2668 w2691 w2710 w2714 w2726 w2751 w2778 w2801 w2805 w2821 w2873 w2919 w2960 w2975 w2993 w3013 w3027 w3039 w3048 w3065 w3087 w3111 w3130 w3148 w3166 w3184 w3198 w3212 w3231 w3245 w3260 w3273 w3283 w3287]
      tunnel: [w94 w474 w484 w489 w495 w510 w530 w559 w618 w632 w663 w706 w718 w746 w778 w792 w821 w833 w920 w957 w996 w1005 w1012 w1017 w1035 w1054 w1077 w1082 w1096 w1115 w1144 w1164 w1207 w1213 w1219 w1226 w1253 w1279 w1305 w1328 w1337 w1361 w1416 w1432 w1445 w1454 w1470 w1484 w1513 w1539 w1544 w1589 w1594 w1606 w1613 w1622 w1634 w1665 w1681 w1695 w1715 w1730 w1761 w1777 w1787 w1803 w1815 w1827 w1855 w1858 w1873 w1885 w1892 w1901 w1910 w1918 w1925 w1934 w1940 w1950 w1953 w1965 w1984 w1999 w2018 w2044 w2062 w2078 w2082 w2090 w2098 w2103 w2111 w2118 w2126 w2133 w2143 w2171 w2179 w2186 w2191 w2199 w2208 w2214 w2220 w2229 w2241 w2250 w2255 w2266 w2339 w2344 w2356 w2366 w2382 w2411 w2426 w2439 w2451 w2475 w2495 w2503 w2516 w2544 w2549 w2555 w2561 w2568 w2579 w2591 w2599 w2604 w2616 w2621 w2632 w2637 w2643 w2648 w2653 w2658 w2668 w2691 w2710 w2714 w2726 w2751 w2778 w2801 w2805 w2821 w2873 w2919 w2960 w2975 w2993 w3013 w3027 w3039 w3048 w3065 w3087 w3111 w3130 w3148 w3166 w3184 w3198 w3212 w3231 w3245 w3260 w3273 w3283 w3287] -> w81
      tunnel: w77 -> [_ _ _ _ _ _ _ _ _ _ _ _ _ _ _ _ _ _ _ w950 _ _ _ _ _ _ _ _ _ _ _ _ _ _ _ _ _ _ _ _ _ _ _ _ _ _ _ _ _ _ _ _ _ _ _ _ _ _ _ _ _ _ _ _ _ _ _ _ _ _ _ w1880 w1891 _ _ _ _ _ _ _ _ _ _ _ _ _ _ _ _ _ _ _ _ _ _ _ _ _ _ _ _ _ _ _ _ _ _ _ _ _ _ _ _ _ _ _ _ _ _ _ _ _ _ _ _ _ _ _ _ _ _ _ _ _ _ _ _ _ _ _ _ _ _ _ _ _ _ _ _ _ _ _ _ _ _ _ _ _ _ _ _ _ _ _ _ _ _ _ _ _ _ _ _ _]
      frame "", "Event Structure", "Idle" {
        # "executes when the state queue is empty"
        n31 = event shown="[20] \"Quit\": Value Change" {
          selector: w95 -> [_ _ _ _ _ _ _ _ _ _ _ _ _ _ _ _ _ _ _ _ _ _ _ _ _ _ _ _ _ _ _ _ _ _ _ _ _]
          dyn-events: [_ _ _ _ _ _ _ _ _ _ _ _ _ _ _ _ _ _ _ _ _ _ _ _ _ _ _ _ _ _ _ _ _ _ _ _ _] -> w94
          timeout: w97 -> [_ _ _ _ _ _ _ _ _ _ _ _ _ _ _ _ _ _ _ _ _ _ _ _ _ _ _ _ _ _ _ _ _ _ _ _ _]
          tunnel: w102 -> [w122 w141 w149 w153 w157 w165 w171 w179 w187 w197 w204 w229 w245 w261 w265 w272 w295 w309 w323 w337 w342 w345 w351 w358 w365 w371 w377 w383 w390 w403 w414 w426 w433 w437 w441 w457 w473]
          tunnel: [w123 w141 w148 w153 w156 w165 w171 w179 w187 w197 w203 w229 w245 w261 w265 w271 w295 w309 w323 w337 w341 w344 w351 w359 w366 w370 w376 w383 w391 w404 w414 w427 w433 w437 w440 w458 w472] -> w101
          tunnel: w100 -> [w106 w139 w143 w151 w158 w164 w172 w180 w188 w195 w199 w227 w243 w259 w263 w267 w294 w308 w322 w336 w338 w346 w349 w354 w361 w373 w378 w381 w385 w398 w412 w422 w431 w435 w442 w455 w470]
          tunnel: [w121 w140 w144 w152 w159 w163 w170 w178 w186 w196 w205 w228 w244 w260 w264 w273 w292 w296 w319 w334 w340 w347 w350 w355 w362 w374 w379 w382 w389 w402 w413 w423 w432 w436 w443 w459 w471] -> w93
          tunnel: w99 -> [w121 w140 w144 w152 w159 w163 w170 w178 w186 w196 w205 w228 w244 w260 w264 w273 w289 w298 w310 w326 w340 w347 w350 w355 w362 w374 w379 w382 w389 w402 w413 w425 w432 w436 w443 w459 w471]
          tunnel: [w106 w139 w143 w151 w158 w164 w172 w180 w188 w195 w200 w227 w243 w259 w263 w268 w294 w308 w322 w336 w338 w346 w349 w356 w363 w373 w378 w381 w386 w399 w412 w428 w431 w435 w442 w456 w470] -> w98
          tunnel: w96 -> [_ _ _ _ _ _ _ _ _ _ _ _ _ _ _ _ _ _ _ _ _ _ _ _ _ _ _ _ _ _ _ _ _ _ _ _ _]
          event Timeout {
            # "check system status every 2s"
            n32 = event-data() -> ()  [unwired: 1 in, 1 out]
            n33 = Unbundle By Name(w106) -> ("SysRunning?"=w104:bool, "SlowTimer"=w120:u32, "FastTimer"=w114:u32)
            n34 = Tick Count (ms)() -> (millisecond timer value=w107:u32)
            n35 = Subtract(x=w107, y=w120) -> (x-y=w117:u32)
            n36 = case shown="False" w104 {
              tunnel: ["" "Utility: AquiTimerCheck" ("State(s) in Front (\"\")")] -> w112
              frame False {
                # "if not running, do nothing"
              }
              frame True {
                # "if aquisition is running, check timer"
              }
            }
            n37 = Subtract(x=w107, y=w114) -> (x-y=w115:u32)
            n38 = Greater?(x=w117, y=u32 2000) -> (0:w118:bool)
            n39 = Greater?(x=w115, y=u32 500) -> (0:w105:bool)
            n40 = disable-structure shown="Enabled" {
              disable-tunnel: w105 -> [w128 _]
              disable-tunnel: w104 -> [w127 _]
              disable-tunnel: [w124 "" ("State(s) at Back (\"\")")] -> w103
              frame Disabled {
                n41 = Not(x=w127) -> (.not. x?=w126:bool)
                n42 = And(x=w128, y=w126) -> (x .and. y?=w125:bool)
                n43 = case shown="True" w125 {
                  tunnel: ["" ("Empty String Constant") "TCP: checkSource" ("State(s) in Front (\"\")")] -> w124
                  frame False {
                  }
                  frame True {
                  }
                }
              }
              frame Enabled {
              }
            }
            n44 = case shown="True" w118 {
              tunnel: ["" ("Empty String Constant") "SystemStatus: SlowSysStatusMacro" ("State(s) in Front (\"\")")] -> w110
              frame False {
              }
              frame True {
              }
            }
            n45 = case shown="True" w105 {
              tunnel: ["" ("Empty String Constant") "SystemStatus: FastSysStatusMacro" ("State(s) in Front (\"\")")] -> w108
              frame False {
              }
              frame True {
              }
            }
            n46 = call <vilib>:"Add State(s) to Queue__JKI_lib_State_Machine.vi"("State(s) in Front (\"\")"=w112, "State(s) in (\"\")"="LabJack: checkPedal" ("State(s) in Front (\"\")"), "State(s) at Back (\"\")"=w110) -> ("States Out"=w109:string)  [unwired: 12 in]
            n47 = call <vilib>:"Add State(s) to Queue__JKI_lib_State_Machine.vi"("State(s) in Front (\"\")"=w109, "State(s) in (\"\")"=w108, "State(s) at Back (\"\")"=w103) -> ("States Out"=w113:string)  [unwired: 12 in]
            n48 = call <vilib>:"Add State(s) to Queue__JKI_lib_State_Machine.vi"("State(s) in Front (\"\")"=w113, "State(s) in (\"\")"=w122) -> ("States Out"=w123:string)  [unwired: 13 in]
          }
          event "355nm Laser toggle": Mouse Enter {
            n49 = event-data() -> ()  [unwired: 1 in, 4 out]
            n50 = local write "Help"("Toggle 355nm laser." ("Help")) -> ()
          }
          event "355nm Laser toggle": Value Change {
            # "[Covers: REQ34]"
            n51 = event-data() -> ()  [unwired: 1 in, 6 out]
            n52 = Select(t="LabJack: 355_PWM_Start\nLabJack: AB_Start", s="355nm Laser toggle", f="LabJack: 355_PWM_Stop\nLabJack: AB_Stop") -> (s? t:f=w146:string)
            n53 = call <vilib>:"Add State(s) to Queue__JKI_lib_State_Machine.vi"("State(s) in Front (\"\")"=w146, "State(s) in (\"\")"=w149) -> ("States Out"=w148:string)  [unwired: 13 in]
          }
          event "Aiming beam toggle": Mouse Enter {
            n54 = event-data() -> ()  [unwired: 1 in, 4 out]
            n55 = local write "Help"("Toggle aiming beam laser." ("Help")) -> ()
          }
          event "Aiming beam toggle": Value Change {
            # "[Covers: REQ33]"
            n56 = event-data() -> ()  [unwired: 1 in, 6 out]
            n57 = case shown="True" "Aiming beam toggle" {
              tunnel: ["LabJack: AB_Stop" ("State(s) in Front (\"\")") "LabJack: AB_Start" ("State(s) in Front (\"\")")] -> w155
              frame False {
              }
              frame True {
              }
            }
            n58 = call <vilib>:"Add State(s) to Queue__JKI_lib_State_Machine.vi"("State(s) in Front (\"\")"=w155, "State(s) in (\"\")"=w157) -> ("States Out"=w156:string)  [unwired: 13 in]
          }
          event "Auto gain ch1": Value Change {
            n59 = event-data() -> ("NewVal"=w162:bool)  [unwired: 1 in, 5 out]
            n60 = case shown="True" w162 {
              frame False {
                n61 = local read "V 1"() -> (w166:dbl)
                n62 = call "V1FGV.vi"("action (write)"=enum16{"write", "read"}."write" ("action"), "V1 in"=w166) -> ()  [unwired: 8 in, 2 out]
                n63 = property on="V 1" class="DigNum (strict)"("DisabledEnum"=T11."Enabled" ("Disabled")) -> ()  [unwired: 2 in, 2 out]
              }
              frame True {
                n64 = property on="V 1" class="DigNum (strict)"("DisabledEnum"=T11."Disabled and Grayed Out" ("Disabled")) -> ()  [unwired: 2 in, 2 out]
              }
            }
          }
          event "Auto gain ch2": Value Change {
            n65 = event-data() -> ("NewVal"=w173:bool)  [unwired: 1 in, 5 out]
            n66 = case shown="False" w173 {
              frame False {
                n67 = local read "V 2"() -> (w174:dbl)
                n68 = property on="V 2" class="DigNum (strict)"("DisabledEnum"=T11."Enabled" ("Disabled")) -> ()  [unwired: 2 in, 2 out]
                n69 = call "V2FGV.vi"("action(write)"=enum16{"write", "read"}."write" ("action"), "V2 in"=w174) -> ()  [unwired: 8 in, 2 out]
              }
              frame True {
                n70 = property on="V 2" class="DigNum (strict)"("DisabledEnum"=T11."Disabled and Grayed Out" ("Disabled")) -> ()  [unwired: 2 in, 2 out]
              }
            }
          }
          event "Auto gain ch3": Value Change {
            n71 = event-data() -> ("NewVal"=w181:bool)  [unwired: 1 in, 5 out]
            n72 = case shown="False" w181 {
              frame False {
                n73 = local read "V 3"() -> (w182:dbl)
                n74 = property on="V 3" class="DigNum (strict)"("DisabledEnum"=T11."Enabled" ("Disabled")) -> ()  [unwired: 2 in, 2 out]
                n75 = call "V3FGV.vi"("action(write)"=enum16{"write", "read"}."write" ("action"), "V3 in"=w182) -> ()  [unwired: 8 in, 2 out]
              }
              frame True {
                n76 = property on="V 3" class="DigNum (strict)"("DisabledEnum"=T11."Disabled and Grayed Out" ("Disabled")) -> ()  [unwired: 2 in, 2 out]
              }
            }
          }
          event "Auto gain ch4": Value Change {
            n77 = event-data() -> ("NewVal"=w189:bool)  [unwired: 1 in, 5 out]
            n78 = case shown="False" w189 {
              frame False {
                n79 = local read "V 4"() -> (w190:dbl)
                n80 = property on="V 4" class="DigNum (strict)"("DisabledEnum"=T11."Enabled" ("Disabled")) -> ()  [unwired: 2 in, 2 out]
                n81 = call "V4FGV.vi"("action(write)"=enum16{"write", "read"}."write" ("action"), "V3 in"=w190) -> ()  [unwired: 8 in, 2 out]
              }
              frame True {
                n82 = property on="V 4" class="DigNum (strict)"("DisabledEnum"=T11."Disabled and Grayed Out" ("Disabled")) -> ()  [unwired: 2 in, 2 out]
              }
            }
          }
          event "Background": Mouse Enter {
            n83 = event-data() -> ()  [unwired: 1 in, 4 out]
            n84 = local write "Help"("Click to record a background." ("Help")) -> ()
          }
          event "Background": Value Change {
            n85 = event-data() -> ("NewVal"=w201:bool)  [unwired: 1 in, 5 out]
            n86 = case shown="True" w201 {
              tunnel: ["Utility: SetAllChanManualGain\nQueue: Flash\nUtility: Dewelling >> 2500\nLabJack: 355_PWM_Stop\nLabJack: AB_Stop" "Utility: SetDataClass >> Bg\nUI: Update\nLabJack: 355_PWM_Start\nLabJack: AB_Start\nUtility: SaveDeconChan\nUtility: Dewelling >> 50\nLabJack: SetV\nDigitizer: Start\nUtility: AquiTimerReset\nLED: BreathGreen\nUI: duringBGAcquire"] -> w202
              tunnel: [FALSE TRUE] -> w198
              frame False {
                n87 = local read "Skip Data Save?"() -> (w206:bool)
                n88 = case shown="False" w206 {
                  frame False {
                    n89 = property on="Background" class="Bool (strict)"("BoolText.Text"="Done!" ("Boolean Text.Text")) -> ()  [unwired: 2 in, 2 out]
                  }
                  frame True {
                  }
                }
              }
              frame True {
                # "[Covers: REQ6]"
                n90 = property on="Background" class="Bool (strict)"("BoolText.Text"="Running" ("Boolean Text.Text"), "Colors [4]"=cluster{u32, u32}[] [{6618880, 6618880}, {16711680, 16711680}]) -> ()  [unwired: 2 in, 2 out]
              }
            }
            n91 = Bundle By Name(cluster=w199, "SysRunning?"=w198) -> (w200:T23)
            n92 = call <vilib>:"Add State(s) to Queue__JKI_lib_State_Machine.vi"("State(s) in Front (\"\")"=w202, "State(s) in (\"\")"=w204) -> ("States Out"=w203:string)  [unwired: 13 in]
          }
          event "Channel 1": Cursor Move {
            n93 = event-data() -> ("CursIdx"=w218:i32, "CursLoc"=w225:cluster{"X":dbl, "Y":dbl})  [unwired: 1 in, 7 out]
            n94 = Unbundle By Name(w225) -> ("X"=w223:dbl)
            n95 = property on="Channel 2" class="WFGraph (strict)"() -> ("CrsrList"=w222:T24)  [unwired: 2 in, 2 out]
            n96 = property on="Channel 3" class="WFGraph (strict)"() -> ("CrsrList"=w219:T24)  [unwired: 2 in, 2 out]
            n97 = Index Array(array=w222, index=w218) -> (element=w226:T25)
            n98 = Index Array(array=w219, index=w218) -> (element=w224:T25)
            n99 = Bundle By Name(cluster=w224, "Position.X"=w223) -> (w217:T25)
            n100 = Bundle By Name(cluster=w226, "Position.X"=w223) -> (w221:T25)
            n101 = control-ref of="Channel 1"() -> (w214:refnum<vi>)
            n102 = Replace Array Subset(array=w222, new element=w221, index=w218) -> (w220:T24)
            n103 = Replace Array Subset(array=w219, new element=w217, index=w218) -> (w216:T24)
            n104 = property on="Channel 2" class="WFGraph (strict)"("CrsrList"=w220) -> ()  [unwired: 2 in, 2 out]
            n105 = property on="Channel 3" class="WFGraph (strict)"("CrsrList"=w216) -> (error out=w215:errorcluster)  [unwired: 2 in, 1 out]
            n106 = call "UpdateCurserIdx(SubVI).vi"("error in (no error)"=w215, "WaveformGraph in"=w214) -> ()  [unwired: 9 in, 1 out]
          }
          event "Channel 2": Cursor Move {
            n107 = event-data() -> ("CursIdx"=w236:i32, "CursLoc"=w242:cluster{"X":dbl, "Y":dbl})  [unwired: 1 in, 7 out]
            n108 = Unbundle By Name(w242) -> ("X"=w239:dbl)
            n109 = property on="Channel 1" class="WFGraph (strict)"() -> ("CrsrList"=w234:T24)  [unwired: 2 in, 2 out]
            n110 = property on="Channel 3" class="WFGraph (strict)"() -> ("CrsrList"=w237:T24)  [unwired: 2 in, 2 out]
            n111 = Index Array(array=w234, index=w236) -> (element=w241:T25)
            n112 = Index Array(array=w237, index=w236) -> (element=w240:T25)
            n113 = Bundle By Name(cluster=w241, "Position.X"=w239) -> (w238:T25)
            n114 = Bundle By Name(cluster=w240, "Position.X"=w239) -> (w235:T25)
            n115 = Replace Array Subset(array=w234, new element=w238, index=w236) -> (w233:T24)
            n116 = Replace Array Subset(array=w237, new element=w235, index=w236) -> (w232:T24)
            n117 = control-ref of="Channel 1"() -> (w231:refnum<vi>)
            n118 = property on="Channel 1" class="WFGraph (strict)"("CrsrList"=w233) -> ()  [unwired: 2 in, 2 out]
            n119 = property on="Channel 3" class="WFGraph (strict)"("CrsrList"=w232) -> (error out=w230:errorcluster)  [unwired: 2 in, 1 out]
            n120 = call "UpdateCurserIdx(SubVI).vi"("error in (no error)"=w230, "WaveformGraph in"=w231) -> ()  [unwired: 9 in, 1 out]
          }
          event "Channel 3": Cursor Move {
            n121 = event-data() -> ("CursIdx"=w251:i32, "CursLoc"=w258:cluster{"X":dbl, "Y":dbl})  [unwired: 1 in, 7 out]
            n122 = Unbundle By Name(w258) -> ("X"=w255:dbl)
            n123 = property on="Channel 1" class="WFGraph (strict)"() -> ("CrsrList"=w254:T24)  [unwired: 2 in, 2 out]
            n124 = property on="Channel 2" class="WFGraph (strict)"() -> ("CrsrList"=w252:T24)  [unwired: 2 in, 2 out]
            n125 = Index Array(array=w254, index=w251) -> (element=w257:T25)
            n126 = Index Array(array=w252, index=w251) -> (element=w256:T25)
            n127 = Bundle By Name(cluster=w257, "Position.X"=w255) -> (w253:T25)
            n128 = Bundle By Name(cluster=w256, "Position.X"=w255) -> (w250:T25)
            n129 = Replace Array Subset(array=w254, new element=w253, index=w251) -> (w249:T24)
            n130 = Replace Array Subset(array=w252, new element=w250, index=w251) -> (w248:T24)
            n131 = control-ref of="Channel 1"() -> (w246:refnum<vi>)
            n132 = property on="Channel 1" class="WFGraph (strict)"("CrsrList"=w249) -> ()  [unwired: 2 in, 2 out]
            n133 = property on="Channel 2" class="WFGraph (strict)"("CrsrList"=w248) -> (error out=w247:errorcluster)  [unwired: 2 in, 1 out]
            n134 = call "UpdateCurserIdx(SubVI).vi"("error in (no error)"=w247, "WaveformGraph in"=w246) -> ()  [unwired: 9 in, 1 out]
          }
          event "Cali&iRF alignment": Mouse Enter {
            n135 = event-data() -> ()  [unwired: 1 in, 4 out]
            n136 = local write "Help"("Click to run system intensity calibration and irf alignment" ("Help")) -> ()
          }
          event "Cali&iRF alignment": Value Change {
            n137 = event-data() -> ("NewVal"=w269:bool)  [unwired: 1 in, 5 out]
            n138 = case shown="False" w269 {
              tunnel: ["Utility: SetAllChanManualGain\nQueue: Flash\nUtility: Dewelling >> 2500\nLabJack: 355_PWM_Stop\nLabJack: AB_Stop" "Utility: SetDataClass >> Cali\nUI: Update\nUtility: SaveDeconChan\nLabJack: 355_PWM_Start\nLabJack: AB_Start\nLabJack: SetV\nDigitizer: Start\nUtility: AquiTimerReset\nLED: BreathGreen\nUI: duringIRFAlign"] -> w270
              tunnel: [FALSE TRUE] -> w266
              frame False {
                n139 = local read "Skip Data Save?"() -> (w274:bool)
                n140 = case shown="False" w274 {
                  frame False {
                    n141 = property on="Cali&iRF alignment" class="Bool (strict)"("BoolText.Text"="Done!" ("Boolean Text.Text")) -> ()  [unwired: 2 in, 2 out]
                  }
                  frame True {
                  }
                }
              }
              frame True {
                n142 = property on="Cali&iRF alignment" class="Bool (strict)"("BoolText.Text"="Running" ("Boolean Text.Text"), "Colors [4]"=cluster{u32, u32}[] [{6618880, 6618880}, {16711680, 16711680}]) -> ()  [unwired: 2 in, 2 out]
              }
            }
            n143 = Bundle By Name(cluster=w267, "SysRunning?"=w266) -> (w268:T23)
            n144 = call <vilib>:"Add State(s) to Queue__JKI_lib_State_Machine.vi"("State(s) in Front (\"\")"=w270, "State(s) in (\"\")"=w272) -> ("States Out"=w271:string)  [unwired: 13 in]
          }
          event "V 1": Value Change {
            n145 = event-data() -> ()  [unwired: 1 in, 6 out]
            n146 = call "LabJack_FGV.vi"("Operation(Read)"=enum16{"Write", "Read"}."Read" ("Operation"), "error in (no error)"=w289) -> ("error out"=w286:errorcluster, "Read data"=w287:i32)  [unwired: 8 in]
            n147 = global read "GlobalVariables.vi" "Ch1 LJ pin"() -> (w285:string)
            n148 = call "LJM_eWriteName.vi"("Handle In"=w287, "Name"=w285, "Value"="V 1", "error in"=w286) -> ("error out"=w283:errorcluster)  [unwired: 10 in, 1 out]
            n149 = call "V1FGV.vi"("Error In"=w283, "action (write)"=enum16{"write", "read"}."write" ("action"), "V1 in"="V 1") -> ("Error Out"=w282:errorcluster)  [unwired: 7 in, 1 out]
            n150 = call "CtrlVtoGain.vi"("error in (no error)"=w282, "CtrlV(V)"="V 1", "Channel"=enum16{"Ch1", "Ch2", "Ch3"}."Ch1" ("Enum")) -> ("error out"=w292:errorcluster, "Gain"=w291:dbl)  [unwired: 7 in]
            n151 = local write "Gain1"(w291) -> ()
          }
          event "V 2": Value Change {
            n152 = event-data() -> ()  [unwired: 1 in, 6 out]
            n153 = call "LabJack_FGV.vi"("Operation(Read)"=enum16{"Write", "Read"}."Read" ("Operation"), "error in (no error)"=w298) -> ("error out"=w303:errorcluster, "Read data"=w304:i32)  [unwired: 8 in]
            n154 = global read "GlobalVariables.vi" "Ch2 LJ pin"() -> (w302:string)
            n155 = call "LJM_eWriteName.vi"("Handle In"=w304, "Name"=w302, "Value"="V 2", "error in"=w303) -> ("error out"=w301:errorcluster)  [unwired: 10 in, 1 out]
            n156 = call "V2FGV.vi"("Error In"=w301, "action(write)"=enum16{"write", "read"}."write" ("action"), "V2 in"="V 2") -> ("Error Out"=w300:errorcluster)  [unwired: 7 in, 1 out]
            n157 = call "CtrlVtoGain.vi"("error in (no error)"=w300, "CtrlV(V)"="V 2", "Channel"=enum16{"Ch1", "Ch2", "Ch3"}."Ch2" ("Enum")) -> ("error out"=w296:errorcluster, "Gain"=w297:dbl)  [unwired: 7 in]
            n158 = local write "Gain2"(w297) -> ()
          }
          event "V 3": Value Change {
            n159 = event-data() -> ()  [unwired: 1 in, 6 out]
            n160 = call "LabJack_FGV.vi"("Operation(Read)"=enum16{"Write", "Read"}."Read" ("Operation"), "error in (no error)"=w310) -> ("error out"=w315:errorcluster, "Read data"=w316:i32)  [unwired: 8 in]
            n161 = global read "GlobalVariables.vi" "Ch3 LJ pin"() -> (w314:string)
            n162 = call "LJM_eWriteName.vi"("Handle In"=w316, "Name"=w314, "Value"="V 3", "error in"=w315) -> ("error out"=w312:errorcluster)  [unwired: 10 in, 1 out]
            n163 = call "V3FGV.vi"("Error In"=w312, "action(write)"=enum16{"write", "read"}."write" ("action"), "V3 in"="V 3") -> ("Error Out"=w311:errorcluster)  [unwired: 7 in, 1 out]
            n164 = call "CtrlVtoGain.vi"("error in (no error)"=w311, "CtrlV(V)"="V 3", "Channel"=enum16{"Ch1", "Ch2", "Ch3"}."Ch3" ("Enum")) -> ("error out"=w319:errorcluster, "Gain"=w318:dbl)  [unwired: 7 in]
            n165 = local write "Gain3"(w318) -> ()
          }
          event "V 4": Value Change {
            n166 = event-data() -> ()  [unwired: 1 in, 6 out]
            n167 = call "LabJack_FGV.vi"("Operation(Read)"=enum16{"Write", "Read"}."Read" ("Operation"), "error in (no error)"=w326) -> ("error out"=w330:errorcluster, "Read data"=w331:i32)  [unwired: 8 in]
            n168 = global read "GlobalVariables.vi" "Ch4 LJ pin"() -> (w329:string)
            n169 = call "LJM_eWriteName.vi"("Handle In"=w331, "Name"=w329, "Value"="V 4", "error in"=w330) -> ("error out"=w328:errorcluster)  [unwired: 10 in, 1 out]
            n170 = call "V4FGV.vi"("Error In"=w328, "action(write)"=enum16{"write", "read"}."write" ("action"), "V3 in"="V 4") -> ("Error Out"=w327:errorcluster)  [unwired: 7 in, 1 out]
            n171 = call "CtrlVtoGain.vi"("error in (no error)"=w327, "CtrlV(V)"="V 4", "Channel"=enum16{"Ch1", "Ch2", "Ch3", "Ch4"}."Ch4") -> ("error out"=w334:errorcluster, "Gain"=w333:dbl)  [unwired: 7 in]
            n172 = local write "Gain4"(w333) -> ()
          }
          event "Quit": Value Change {
            # "Exit Button Value Change (pressed) Event\n(when pressed.  quite)"
            n173 = event-data() -> ()  [unwired: 1 in, 1 out]
            n174 = call <vilib>:"Add State(s) to Queue__JKI_lib_State_Machine.vi"("State(s) in Front (\"\")"="LED: Off\nMacro: Exit", "State(s) in (\"\")"=w342) -> ("States Out"=w341:string)  [unwired: 13 in]
          }
          event "Show BG": Value Change {
            n175 = event-data() -> ()  [unwired: 1 in, 6 out]
            n176 = call <vilib>:"Add State(s) to Queue__JKI_lib_State_Machine.vi"("State(s) in Front (\"\")"="Data: showBG" ("State(s) in Front (\"\")"), "State(s) in (\"\")"=w345) -> ("States Out"=w344:string)  [unwired: 13 in]
          }
          event "StartButton": Mouse Enter {
            n177 = event-data() -> ()  [unwired: 1 in, 4 out]
            n178 = local write "Help"("Press to start aquisition." ("Help")) -> ()
          }
          event "StartButton": Value Change {
            # "[Covers: REQ32]"
            # "start PWM before acquisition"
            # "Initialize both digitizer aquisition and\n send user event to trigger aquisition loop"
            n179 = event-data() -> ()  [unwired: 1 in, 6 out]
            n180 = local write "StartButton"(FALSE ("StartButton")) -> ()
            n181 = Bundle By Name(cluster=w354, "SysRunning?"=TRUE) -> (w356:T23)
            n182 = call <vilib>:"Add State(s) to Queue__JKI_lib_State_Machine.vi"("State(s) in Front (\"\")"="TCP: stopCam\nUtility: SetDataClass >> Data\nQueue: Flash\nUI: Update\nUtility: StartBeep\nLabJack: 355_PWM_Start\nLabJack: AB_Start\nLabJack: SetV\nDigitizer: Start\nUtility: AquiTimerReset\nUI: DuringAquisition\nLED: BreathGreen\nTCP: sendRunNum\nTCP: sendVideoSource\nTCP: sendChannel\nTCP: startRun", "State(s) in (\"\")"=w358) -> ("States Out"=w359:string)  [unwired: 13 in]
          }
          event User Event {
            # "[Covers: REQ32]"
            # "start PWM before acquisition"
            # "Initialize both digitizer aquisition and\n send user event to trigger aquisition loop"
            n183 = event-data() -> ()  [unwired: 1 in, 5 out]
            n184 = Bundle By Name(cluster=w361, "SysRunning?"=TRUE) -> (w363:T23)
            n185 = call <vilib>:"Add State(s) to Queue__JKI_lib_State_Machine.vi"("State(s) in Front (\"\")"="TCP: stopCam\nUtility: SetDataClass >> Data\nQueue: Flash\nUI: Update\nUtility: StartBeep\nLabJack: 355_PWM_Start\nLabJack: AB_Start\nLabJack: SetV\nDigitizer: Start\nUtility: AquiTimerReset\nUI: DuringAquisition\nLED: BreathGreen\nTCP: sendRunNum\nTCP: sendVideoSource\nTCP: sendChannel\nTCP: startRun", "State(s) in (\"\")"=w365) -> ("States Out"=w366:string)  [unwired: 13 in]
          }
          event "Video Display": Value Change {
            n186 = event-data() -> ("NewVal"=w372:bool)  [unwired: 1 in, 5 out]
            n187 = Select(t="TCP: startCam", s=w372, f="TCP: stopCam") -> (s? t:f=w369:string)
            n188 = call <vilib>:"Add State(s) to Queue__JKI_lib_State_Machine.vi"("State(s) in (\"\")"=w371, "State(s) at Back (\"\")"=w369) -> ("States Out"=w370:string)  [unwired: 13 in]
          }
          event "Video Source": Value Change {
            n189 = event-data() -> ()  [unwired: 1 in, 6 out]
            n190 = call <vilib>:"Add State(s) to Queue__JKI_lib_State_Machine.vi"("State(s) in Front (\"\")"="TCP: sendVideoSource" ("State(s) in Front (\"\")"), "State(s) in (\"\")"=w377) -> ("States Out"=w376:string)  [unwired: 13 in]
          }
          event "StopButton": Mouse Enter {
            n191 = event-data() -> ()  [unwired: 1 in, 4 out]
            n192 = local write "Help"("Press to stop data aquisition." ("Help")) -> ()
          }
          event "StopButton": Value Change {
            # "if system is running, send stop command, if not do nothing."
            # "stop aquisition\nupdate UI"
            n193 = event-data() -> ()  [unwired: 1 in, 6 out]
            n194 = Unbundle By Name(w385) -> ("SysRunning?"=w387:bool)
            n195 = case shown="True" w387 {
              tunnel: ["" ("Empty String Constant") "LabJack: AB_Stop\nLabJack: 355_PWM_Stop\n/*Digitizer: Abort"] -> w388
              tunnel: w385 -> [w392 w396]
              tunnel: [w392 w395] -> w386
              frame False {
              }
              frame True {
                n196 = Bundle By Name(cluster=w396, "SysRunning?"=FALSE) -> (w395:T23)
              }
            }
            n197 = call <vilib>:"Add State(s) to Queue__JKI_lib_State_Machine.vi"("State(s) in Front (\"\")"=w388, "State(s) in (\"\")"=w390) -> ("States Out"=w391:string)  [unwired: 13 in]
            n198 = local write "StopButton"(FALSE ("StopButton")) -> ()
          }
          event User Event {
            # "if system is running, send stop command, if not do nothing."
            # "stop aquisition\nupdate UI"
            n199 = event-data() -> ()  [unwired: 1 in, 5 out]
            n200 = Unbundle By Name(w398) -> ("SysRunning?"=w400:bool)
            n201 = case shown="True" w400 {
              tunnel: ["" ("Empty String Constant") "LabJack: AB_Stop\nLabJack: 355_PWM_Stop\n/*Digitizer: Abort"] -> w401
              tunnel: w398 -> [w405 w409]
              tunnel: [w405 w408] -> w399
              frame False {
              }
              frame True {
                n202 = Bundle By Name(cluster=w409, "SysRunning?"=FALSE) -> (w408:T23)
              }
            }
            n203 = call <vilib>:"Add State(s) to Queue__JKI_lib_State_Machine.vi"("State(s) in Front (\"\")"=w401, "State(s) in (\"\")"=w403) -> ("States Out"=w404:string)  [unwired: 13 in]
          }
          event "Sys Reconfig": Mouse Enter {
            n204 = event-data() -> ()  [unwired: 1 in, 4 out]
            n205 = local write "Help"("Click to reconfig digitizer settings." ("Help")) -> ()
          }
          event "Sys Reconfig": Value Change {
            # "everytime the user change data aquisition setting, need to reinitilize decon engine and realign iRF.\ncheck whether data length has changed, if changed, reinitialize Decon engine\nreset BG ready, need a new BG"
            # "update DAQ FGV"
            n206 = event-data() -> ()  [unwired: 1 in, 6 out]
            n207 = call "SystemConfigEditorV6.vi"("error in"=w425) -> ("error out"=w424:errorcluster, "FLImDAQ out"=w419:T6)  [unwired: 1 in]
            n208 = Unbundle By Name(w422) -> ("FLImDAQ.min record length"=w421:i32)
            n209 = Unbundle By Name(w419) -> ("min record length"=w420:i32)
            n210 = call "FLImDAQ_FGV.vi"("error in (no error)"=w424, "Operation (Read)"=enum16{"Write", "Read"}."Write" ("Operation"), "Write data"=w419) -> ("error out"=w423:errorcluster, "Read data"=w418:T6)  [unwired: 7 in]
            n211 = Equal?(x=w421, y=w420) -> (x = y?=w417:bool)
            n212 = case shown="False" w417 {
              tunnel: ["UI: Cursor Set >> Busy\nDigitizer: Config\nDeconEngine: InitializeCh1\nDeconEngine: InitializeCh2\nDeconEngine: InitializeCh3\nUI: CaliAndiRFNotReady\n/*UI iRF not ready\nUI: Update\nUI: Cursor Set >> Idle" "UI: Cursor Set >> Busy\nDigitizer: Config\nUI: Update\nUI: Cursor Set >> Idle"] -> w416
              frame False {
              }
              frame True {
              }
            }
            n213 = Bundle By Name(cluster=w422, "FLImDAQ"=w418) -> (w428:T23)
            n214 = call <vilib>:"Add State(s) to Queue__JKI_lib_State_Machine.vi"("State(s) in Front (\"\")"=w416, "State(s) in (\"\")"=w426) -> ("States Out"=w427:string)  [unwired: 13 in]
          }
          event "System Hardware Connection Status", "StartButton", "StopButton", "355nm Laser toggle", "Aiming beam toggle", "Cali&iRF alignment", "Background", "Sys Reconfig": Mouse Leave {
            n215 = event-data() -> ()  [unwired: 1 in, 4 out]
            n216 = invoke on="Help" class="Str" method="Reinit To Default"() -> ()  [unwired: 3 in, 3 out]
          }
          event "System Hardware Connection Status.Digitizer": Mouse Enter {
            n217 = event-data() -> ()  [unwired: 1 in, 4 out]
            n218 = local write "Help"("Status of hardware connections. TCP/IP is optional." ("Help")) -> ()
          }
          event "TCP Connect": Value Change {
            n219 = event-data() -> ("NewVal"=w438:bool)  [unwired: 1 in, 5 out]
            n220 = case shown="True" w438 {
              tunnel: ["TCP: Close\nUI: Update" ("State(s) in Front (\"\")") "TCP: SendSettingMacro\nUI: Update" ("State(s) in Front (\"\")")] -> w439
              frame False {
              }
              frame True {
              }
            }
            n221 = call <vilib>:"Add State(s) to Queue__JKI_lib_State_Machine.vi"("State(s) in Front (\"\")"=w439, "State(s) in (\"\")"=w441) -> ("States Out"=w440:string)  [unwired: 13 in]
          }
          event User Event {
            # "if aquisition loop is error out. Stop digitizer, update front panel indicator, stop both laser and \nOption 1: parse and save data\nOption 2: Flash queue if scout run. [Covers: REQ23]"
            n222 = event-data() -> ()  [unwired: 1 in, 5 out]
            n223 = case shown="\"Data\", Default" "Data Class" {
              tunnel: [w463 "UI: Cursor Set >> Busy\nUtility: SetAllChanAutoGain\nUtility: RestoreDeConChan\nData: parseRunData\nData: irfAlignment\nUI: Cursor Set >> Idle" "UI: Cursor Set >> Busy\nUtility: SetAllChanAutoGain\nUtility: RestoreDeConChan\nData: parseRunData\nData: saveBGtoFGV\nData: saveBGtoFile\nUI: Cursor Set >> Idle\nData: showBG\nRun: BGIncrement"] -> w453
              frame "Data", Default {
                n224 = local read "Video Display"() -> (w465:bool)
                n225 = Select(t="TCP: startCam", s=w465, f="") -> (s? t:f=w461:string)
                n226 = call <vilib>:"Add State(s) to Queue__JKI_lib_State_Machine.vi"("State(s) in Front (\"\")"="UI: Cursor Set >> Busy\nData: parseRunData\nData: saveRunData\nUI: Cursor Set>>Idle" ("State(s) in Front (\"\")"), "State(s) in (\"\")"=w461) -> ("States Out"=w463:string)  [unwired: 13 in]
              }
              frame "Cali" {
              }
              frame "BG" {
              }
            }
            n227 = Bundle By Name(cluster=w455, "SysRunning?"=FALSE) -> (w456:T23)
            n228 = Select(t="" ("State(s) in Front (\"\")"), s="Skip Data Save?", f=w453) -> (s? t:f=w450:string)
            n229 = call <vilib>:"Add State(s) to Queue__JKI_lib_State_Machine.vi"("State(s) in Front (\"\")"="TCP: stopRun\nUI: Update\nLabJack: AB_Stop\nLabJack: 355_PWM_Stop\nDigitizer: Abort\nLabJack: ZeroV\nUtility: EndBeep\nLED: BreathOff" ("State(s) in Front (\"\")"), "State(s) in (\"\")"=w450, "State(s) at Back (\"\")"="Macro: SysReadyForAq\nUI: Update" ("State(s) in Front (\"\")")) -> ("States Out"=w448:string)  [unwired: 12 in]
            n230 = call <vilib>:"Add State(s) to Queue__JKI_lib_State_Machine.vi"("State(s) in Front (\"\")"=w448, "State(s) in (\"\")"=w457) -> ("States Out"=w458:string)  [unwired: 13 in]
          }
          event Panel Close? {
            # "Discard the event because we'll close the front panel ourselves in Macro: Exit"
            # "Close Panel button (pressed) Event\n(this executes Macro: Exit to terminate the VI)"
            n231 = event-data() -> ()  [unwired: 1 in, 1 out]
            n232 = event-data ("Event Filter Node")("Discard?"=TRUE) -> ()  [unwired: 1 in, 1 out]
            n233 = call <vilib>:"Add State(s) to Queue__JKI_lib_State_Machine.vi"("State(s) in Front (\"\")"="Macro: Exit", "State(s) in (\"\")"=w473) -> ("States Out"=w472:string)  [unwired: 13 in]
          }
        }
      }
      frame "---------- Macro ----------" {
        # "Do not put any code in this frame.\n(It is a separator no-op. You can make a copy of this frame to create a new Macro frame)"
        n234 = call <vilib>:"Add State(s) to Queue__JKI_lib_State_Machine.vi"("State(s) in (\"\")"=w478) -> ("States Out"=w477:string)  [unwired: 14 in]
      }
      frame "Macro: Initialize" {
        # "load Labjack setting 1st as it contaisn laser pin infortmation"
        # "start laser 1st, need 7.5s for laser to get ready"
        # "Initialization Macro\n(This is called once, when the VI starts)"
        n235 = call <vilib>:"Add State(s) to Queue__JKI_lib_State_Machine.vi"("State(s) in Front (\"\")"="UI: showDisclaimer\nUI: Cursor Set >> Busy\nData: Initialize\nInitialize Core Data\nUI: Initialize\nUI: Front Panel State >> Open\nMacro: LoadSysConfig\nTCP: InitializeNew\nTCP: checkSource\nUI: Update\nLabJack: Open\nLabJack: SetDefaultSub\nLED: OpenVIRef\nLED: BreathOrange\nUI: Update\n355 Laser: CheckControllerStatus\n355 Laser: Laser enable\n355 Laser: Dewelling>>500\n355 Laser: CheckControllerStatus\nUI: Update\nLabJack: 355_PWM_Config\nLabJack: AB_PWM_Config\nUI: Update", "State(s) in (\"\")"="Digitizer: Initialize\nDigitizer: Config\nUI: Update\n/*AimingBeam: Initialize\n/*AimingBeam: Set Status>>Enable\n/*AimingBeam: Set Current\nUI: Update\n355 Laser: Check Dewelling\nUI: Cursor Set >> Idle\nCase: GetID\nUI: Update\nTCP: SendSettingMacro\nCase: CreatFileStruct\nUI: Update\nData: loadLastUseMacro\nDeconEngine: InitilizeMacro\nGraph: SetXMultiplier\nGraph: AddCursors\nAPD: Initialize\nAPD: LoadFromSerial\nAPD: UpdateCtrlVLimit\nAPD: GetGainLimits\nPID: loadPID\nLED: BreathOff\nMacro: SysReadyForAq") -> ("States Out"=w479:string)  [unwired: 13 in]
        n236 = call <vilib>:"Add State(s) to Queue__JKI_lib_State_Machine.vi"("State(s) in Front (\"\")"=w479, "State(s) in (\"\")"=w487) -> ("States Out"=w486:string)  [unwired: 13 in]
        "Help" <- "Hover over controls to see help!" ("Help")
      }
      frame "Macro: LoadSysConfig" {
        # "System configuration Macro. [Covers: REQ15]\n(Load configurations for different component of the system)"
        n237 = call <vilib>:"Add State(s) to Queue__JKI_lib_State_Machine.vi"("State(s) in Front (\"\")"="SysConfig: Load Sys Config\nSysConfig: Load Digitizer Setting\nSysConfig: Load AB setting\nSysConfig: Load LJ Pinout\nSysConfig: Load 355 PWM\nSysConfig: LoadAPDSerialNumber\nSysConfig: LoadABVideoSetting\nSysConfig: LoadCursorLocation", "State(s) in (\"\")"=w493) -> ("States Out"=w492:string)  [unwired: 13 in]
      }
      frame "Macro: SysReadyForAq" {
        # "Macro for system ready\n(It is a separator no-op. You can make a copy of this frame to create a new Macro frame)"
        n238 = call <vilib>:"Add State(s) to Queue__JKI_lib_State_Machine.vi"("State(s) in Front (\"\")"="UI: ReadyForAquisition\nLED: Green" ("State(s) in Front (\"\")"), "State(s) in (\"\")"=w499) -> ("States Out"=w498:string)  [unwired: 13 in]
      }
      frame "Macro: Exit" {
        # "close LJ last"
        # "check whether hardware is initilized, if so close, if not do nothing"
        # "Exit Macro, close all hardware\n(This is called once, when the VI exits)"
        n239 = Unbundle By Name(w518) -> ("System Status.Digitizer"=w514:bool, "System Status.Aiming Beam"=w513:bool, "System Status.355 Laser"=w512:bool, "System Status.Labjack"=w503:bool, "Core.Close Panel on Exit?"=w507:bool)
        n240 = case shown="True" w514 {
          tunnel: ["" ("Empty String Constant") "Digitizer: Close"] -> w509
          frame False {
          }
          frame True {
          }
        }
        n241 = case shown="True" w503 {
          tunnel: ["" ("Empty String Constant") "LabJack: SetDefaultAndClose"] -> w500
          frame False {
          }
          frame True {
          }
        }
        n242 = case shown="True" w513 {
          tunnel: ["" ("Empty String Constant") "/*AimingBeam: Set Status >> Disable\n/*AimingBeam: Close"] -> w502
          frame False {
          }
          frame True {
          }
        }
        n243 = case shown="True" w512 {
          tunnel: ["" ("Empty String Constant") "355 Laser: Close\n355 Laser: CheckControllerStatus"] -> w501
          frame False {
          }
          frame True {
          }
        }
        n244 = Select(t="UI: Front Panel State >> Close", s=w507, f="" ("Empty String Constant")) -> (s? t:f=w504:string)
        n245 = call <vilib>:"Add State(s) to Queue__JKI_lib_State_Machine.vi"("State(s) in Front (\"\")"="TCP: Close", "State(s) in (\"\")"=w509, "State(s) at Back (\"\")"=w502) -> ("States Out"=w511:string)  [unwired: 12 in]
        n246 = call <vilib>:"Add State(s) to Queue__JKI_lib_State_Machine.vi"("State(s) in Front (\"\")"=w511, "State(s) in (\"\")"=w501, "State(s) at Back (\"\")"=w500) -> ("States Out"=w506:string)  [unwired: 12 in]
        n247 = call <vilib>:"Add State(s) to Queue__JKI_lib_State_Machine.vi"("State(s) in Front (\"\")"=w506, "State(s) in (\"\")"="UI: Update\nUI: Reset\nGraph: SaveCursorLoc\nLED: CloseVIRef\nQueue: Destory\nData: Cleanup\nExit", "State(s) at Back (\"\")"=w504) -> ("States Out"=w515:string)  [unwired: 12 in]
        n248 = call <vilib>:"Add State(s) to Queue__JKI_lib_State_Machine.vi"("State(s) in Front (\"\")"=w515, "State(s) in (\"\")"=w521) -> ("States Out"=w520:string)  [unwired: 13 in]
      }
      frame "---------- Data ----------" {
        # "Do not put any code in this frame.\n(It is a separator no-op. You can make a copy of this frame to create a new Data frame)"
        n249 = call <vilib>:"Add State(s) to Queue__JKI_lib_State_Machine.vi"("State(s) in (\"\")"=w534) -> ("States Out"=w533:string)  [unwired: 14 in]
      }
      frame "Data: Initialize" {
        w535 = path ""  # CaliPath
        w536 = dbl[] []  # V4
        w537 = dbl[][] []  # Ch4Data
        w538 = FALSE  # bothVidSourceAvail
        w539 = T1 {"Main Frame Grabber"=FALSE, "Side Frame Grabber"=FALSE, "Main Camera"=FALSE, "Side Camera"=FALSE}  # video source
        w540 = FALSE  # LED vi ref open?
        w542 = T22 {"DeCon Channel"=enum."1", "Scale Bar"=FALSE, "Scale Low"=3.0, "Scale High"=8.0, "ANSI"=20.0, "Radius"=1.0, "3D?"=FALSE, "Firefly?"=FALSE, "Pentero?"=FALSE}  # VideoConfig
        w543 = T26 {"Ch1APDSerial#"="", "Ch2APDSerial#"="", "Ch3APDSerial#"="", "Ch4APDSerial#"=""}  # APDSerialNum
        w544 = u32 0  # Aquisition Timer
        w545 = cluster{"RunID":i8, "BG ID":i8, "Cali ID":i8} {"RunID"=1, "BG ID"=1, "Cali ID"=1}  # IDs
        w546 = refnum<vi> refnum  # LED vi reference
        w547 = path ""  # TempPath
        w548 = T27 {"DataPath"=path "", "BG Path"=path "", "iRFPath"=path "", "CaliPath"=path ""}  # Pathes
        w550 = dbl[] []  # V3
        w551 = dbl[] []  # V2
        w552 = dbl[] []  # V1
        w554 = u32 0  # FastTimer
        w555 = u32 0  # SlowTimer
        w556 = dbl[][] []  # Ch3Data
        w557 = dbl[][] []  # Ch2Data
        w541 = dbl[][] []  # Ch1Data
        w560 = T2 {"Digitizer"=FALSE, "Labjack"=FALSE, "Aiming Beam"=FALSE, "355 Laser"=FALSE, "TCP/IP"=FALSE}  # System Status
        w561 = T28 {"DIO_EF_CLOCK1_DIVISOR"=16, "DIO_EF_CLOCK1_ROLL_VALUE"=25000, "DIO#_EF_INDEX"=0, "DIO#_EF_OPTIONS"=1, "DIO#_EF_CONFIG_A"=6250}  # AB PWM setting
        w562 = T5 {"Ch1 Bias"="TDA11", "Ch2 Bias"="DAC10", "Ch3 Bias"="DAC0", "Ch4 Bias"="DAC0", "355 PWM"="FIO0", "AimingBeam PWM"="FIO2", "Laser Ready"="FIO3", "Interlock"="FIO1", "Laser Start/Stop"="FIO1", "Red LED"="FIO1", "Green LED"="FIO1", "Foot Pedal"="DIO15"}  # LJ Pinout
        w563 = 0  # TCP attempt count
        w564 = u32 0  # Laser start tic
        w565 = refnum<k20>[] []  # niTClk sessions
        w566 = u32 0  # Last Trigger
        w567 = T28 {"DIO_EF_CLOCK1_DIVISOR"=16, "DIO_EF_CLOCK1_ROLL_VALUE"=25000, "DIO#_EF_INDEX"=0, "DIO#_EF_OPTIONS"=1, "DIO#_EF_CONFIG_A"=6250}  # 355 PWM setting
        w568 = T29 {"Aiming Beam COM Port"="COM3", "Min Current"=0.0, "Max Current"=63.0, "Default Current"=20.0, "Freq"=0}  # AB Cluster
        w569 = T30 {"resource name"="", "resource name 2"="", "Channel"=enum."Channel 0", "trigger source"="VAL_EXTERNAL", "trigger level"=0.5, "trigger delay"=1.35e-07, "min sample rate"=12500000000.0, "min record length"=2500, "vertical range"=1.0, "vertical offset"=-0.25, "Waveform to Avg"=2000}  # FLImDAQ
        w570 = FALSE  # SysRunning?
        w558 = path ""  # DefaultPath
        w571 = ""  # CaseID
        w572 = T4 {"Ch1Enable?"=FALSE, "Ch2Enable?"=FALSE, "Ch3Enable?"=FALSE, "Ch1AutoGain?"=FALSE, "Ch2AutoGain?"=FALSE, "Ch3AutoGain?"=FALSE, "AimingBeamEnable?"=FALSE}  # SysConfigCluster
        w573 = T31 {"Current VI Reference"=refnum, "Close Panel on Exit?"=FALSE}  # Core
        # "Initialize the shift-register data, here.\n(data names are defined by what you wire into the bundle function)"
        n250 = Bundle("Core"=w573, "SysConfigCluster"=w572, "System Status"=w560, "IDs"=w545, "CaseID"=w571, "DefaultPath"=w558, "Pathes"=w548, "FLImDAQ"=w569, "SysRunning?"=w570, "AB Cluster"=w568, "LJ Pinout"=w562, "355 PWM setting"=w567, "AB PWM setting"=w561, "Last Trigger"=w566, "niTClk sessions"=w565, "Laser start tic"=w564, "TCP attempt count"=w563, "Ch1Data"=w541, "Ch2Data"=w557, "Ch3Data"=w556, "Ch4Data"=w537, "V1"=w552, "V2"=w551, "V3"=w550, "V4"=w536, "SlowTimer"=w555, "FastTimer"=w554, "listener ID"=refnum<k5> refnum, "TempPath"=w547, "CaliPath"=w535, "LED vi reference"=w546, "Aquisition Timer"=w544, "APDSerialNum"=w543, "VideoConfig"=w542, "LED vi ref open?"=w540, "video source"=w539, "bothVidSourceAvail"=w538) -> (w549:T23)  [unwired: 1 in]
        n251 = call <vilib>:"Add State(s) to Queue__JKI_lib_State_Machine.vi"("State(s) in (\"\")"=w576) -> ("States Out"=w575:string)  [unwired: 14 in]
      }
      frame "Data: LoadAPDData" {
        w587 = T15 {"Ch1 iRF"=[], "Ch2 iRF"=[], "Ch3 iRF"=[], "Ch4 iRF"=[]}  # LastUseiRF
        # "only load the last iRF for the moment"
        # "Load APD detector data\n(It is a separator no-op. You can make a copy of this frame to create a new Data frame)"
        n252 = Unbundle By Name(w617) -> ("APDSerialNum.Ch1APDSerial#"=w616:string, "APDSerialNum.Ch2APDSerial#"=w590:string, "APDSerialNum.Ch3APDSerial#"=w589:string, "APDSerialNum.Ch4APDSerial#"=w585:string)
        n253 = call "CreatFromSerialNumNoRaw.vi"("error in (no error)"=w586, "APD Serial #"=w616) -> ("error out"=w614:errorcluster, "APDClass out"=w615:refnum<class "APDClass.lvclass">)  [unwired: 8 in]
        n254 = call "CreatFromSerialNumNoRaw.vi"("error in (no error)"=w586, "APD Serial #"=w590) -> ("error out"=w603:errorcluster, "APDClass out"=w604:refnum<class "APDClass.lvclass">)  [unwired: 8 in]
        n255 = call "CreatFromSerialNumNoRaw.vi"("error in (no error)"=w586, "APD Serial #"=w589) -> ("error out"=w596:errorcluster, "APDClass out"=w597:refnum<class "APDClass.lvclass">)  [unwired: 8 in]
        n256 = call "CreatFromSerialNumNoRaw.vi"("error in (no error)"=w586, "APD Serial #"=w585) -> ("error out"=w583:errorcluster, "APDClass out"=w584:refnum<class "APDClass.lvclass">)  [unwired: 8 in]
        n257 = call-dynamic "Read iRFData.vi"("error in (no error)"=w614, "APDClass in"=w615) -> ("iRFData"=w613:T32)  [unwired: 7 in, 2 out]
        n258 = call-dynamic "Read iRFData.vi"("error in (no error)"=w603, "APDClass in"=w604) -> ("iRFData"=w608:T32)  [unwired: 7 in, 2 out]
        n259 = call-dynamic "Read iRFData.vi"("error in (no error)"=w596, "APDClass in"=w597) -> ("iRFData"=w601:T32)  [unwired: 7 in, 2 out]
        n260 = call-dynamic "Read iRFData.vi"("error in (no error)"=w583, "APDClass in"=w584) -> ("iRFData"=w582:T32)  [unwired: 7 in, 2 out]
        n261 = Unbundle By Name(w613) -> ("iRFWFsAvg"=w612:dbl[][])
        n262 = Unbundle By Name(w608) -> ("iRFWFsAvg"=w607:dbl[][])
        n263 = Unbundle By Name(w601) -> ("iRFWFsAvg"=w600:dbl[][])
        n264 = Unbundle By Name(w582) -> ("iRFWFsAvg"=w578:dbl[][])
        n265 = Array Size(array=w612) -> (size(s)=w611:i32[])
        n266 = Array Size(array=w607) -> (size(s)=w602:i32[])
        n267 = Array Size(array=w600) -> (size(s)=w595:i32[])
        n268 = Array Size(array=w578) -> (size(s)=w579:i32[])
        n269 = Index Array(array=w611, index=1) -> (element=w609:i32)
        n270 = Index Array(array=w602, index=1) -> (element=w605:i32)
        n271 = Index Array(array=w595, index=1) -> (element=w598:i32)
        n272 = Index Array(array=w579, index=1) -> (element=w580:i32)
        n273 = Index Array(array=w612, index (row)=w609) -> (element=w594:dbl[])  [unwired: 1 in]
        n274 = Index Array(array=w607, index (row)=w605) -> (element=w593:dbl[])  [unwired: 1 in]
        n275 = Index Array(array=w600, index (row)=w598) -> (element=w592:dbl[])  [unwired: 1 in]
        n276 = Index Array(array=w578, index (row)=w580) -> (element=w577:dbl[])  [unwired: 1 in]
        n277 = Bundle(cluster=w587, "Ch1 iRF"=w594, "Ch2 iRF"=w593, "Ch3 iRF"=w592, "Ch4 iRF"=w577) -> (w588:T15)
        n278 = global write "GlobalVariables.vi" "LastUseiRF"(w588) -> ()
        n279 = call <vilib>:"Add State(s) to Queue__JKI_lib_State_Machine.vi"("State(s) in Front (\"\")"="UI: CaliAndiRFLoaded" ("State(s) in Front (\"\")"), "State(s) in (\"\")"=w620) -> ("States Out"=w619:string)  [unwired: 13 in]
      }
      frame "Data: loadLastUseiRF" {
        # "Load last use iRF.\n()"
        n280 = Unbundle By Name(w625) -> ("TempPath"=w624:path)
        n281 = Build Path(base path=w624, name or relative path="iRF.tdms") -> (appended path=w630:path)
        n282 = TDMS Open(11:w630) -> (0:w628:errorcluster, 3:w629:refnum<k34>)  [unwired: 6 in]
        n283 = TDMS Read(0:w629, 11:w628, 12:dbl[][] []) -> (4:w622:refnum<k34>, 10:w626:dbl[][], 15:w621:errorcluster)  [unwired: 5 in, 3 out]
        n284 = TDMS Close(8:w621, 11:w622) -> ()  [unwired: 2 out]
        n285 = case shown="No Error" w621 {
          tunnel: w626 -> [w649 _]
          tunnel: ["UI: CaliAndiRFLoaded" ("State(s) in Front (\"\")") "" ("Empty String Constant")] -> w623
          frame No Error {
            w636 = T15 {"Ch1 iRF"=[], "Ch2 iRF"=[], "Ch3 iRF"=[], "Ch4 iRF"=[]}  # LastUseiRF
            n286 = Index Array(array=w649, index (row)=0) -> (element=w645:dbl[])  [unwired: 1 in]
            n287 = Index Array(array=w649, index (row)=1) -> (element=w642:dbl[])  [unwired: 1 in]
            n288 = Index Array(array=w649, index (row)=2) -> (element=w639:dbl[])  [unwired: 1 in]
            n289 = Add Array Elements(numeric array=w645) -> (sum=w644:dbl)
            n290 = Add Array Elements(numeric array=w642) -> (sum=w641:dbl)
            n291 = Add Array Elements(numeric array=w639) -> (sum=w638:dbl)
            n292 = Divide(x=w645, y=w644) -> (x/y=w643:dbl[])
            n293 = Divide(x=w642, y=w641) -> (x/y=w640:dbl[])
            n294 = Divide(x=w639, y=w638) -> (x/y=w637:dbl[])
            n295 = Bundle(cluster=w636, "Ch1 iRF"=w643, "Ch2 iRF"=w640, "Ch3 iRF"=w637) -> (w648:T15)  [unwired: 1 in]
            n296 = Array Size(array=w645) -> (size(s)=→"iRF length":i32)
            n297 = global write "GlobalVariables.vi" "LastUseiRF"(w648) -> ()
          }
          frame Error {
          }
        }
        n298 = call <vilib>:"Add State(s) to Queue__JKI_lib_State_Machine.vi"("State(s) in Front (\"\")"=w623, "State(s) in (\"\")"=w635) -> ("States Out"=w634:string)  [unwired: 13 in]
      }
      frame "Data: loadSystemCali" {
        # "Load last use calibration.\n()"
        n299 = Unbundle By Name(w661) -> ("CaliPath"=w660:path)
        n300 = Build Path(base path=w660, name or relative path="Calibration.tdms") -> (appended path=w656:path)
        n301 = call "ReadBGorCali (SubVI).vi"("DataType"=enum16{"BG", "Cali"}."Cali", "error in (no error)"=w655, "file path in"=w656) -> ("error out"=w657:errorcluster, "CtrlVCluster"=w659:T33, "AvgDataCluster"=w658:T34)  [unwired: 6 in]
        n302 = case shown="No Error" w657 {
          tunnel: w659 -> [w680 _]
          tunnel: w658 -> [w679 _]
          frame No Error {
            w670 = T35 {"Ch1 WF"=[], "Ch2 WF"=[], "Ch3 WF"=[], "Ch4 WF"=[], "V1"=0.0, "V2"=0.0, "V3"=0.0, "V4"=0.0}  # SysCaliData
            n303 = Unbundle By Name(w679) -> ("Channel 1"=w678:dbl[], "Channel 2"=w677:dbl[], "Channel 3"=w676:dbl[], "Channel 4"=w669:dbl[])
            n304 = Unbundle By Name(w680) -> ("V 1"=w675:dbl[], "V 2"=w674:dbl[], "V 3"=w668:dbl[], "V 4"=w666:dbl[])
            n305 = Index Array(array=w675) -> (element=w673:dbl)  [unwired: 1 in]
            n306 = Index Array(array=w674) -> (element=w672:dbl)  [unwired: 1 in]
            n307 = Index Array(array=w668) -> (element=w671:dbl)  [unwired: 1 in]
            n308 = Index Array(array=w666) -> (element=w667:dbl)  [unwired: 1 in]
            n309 = Bundle By Name(cluster=w670, "Ch1 WF"=w678, "Ch2 WF"=w677, "Ch3 WF"=w676, "Ch4 WF"=w669, "V1"=w673, "V2"=w672, "V3"=w671, "V4"=w667) -> (w681:T35)
            n310 = global write "GlobalVariables.vi" "SysCaliData"(w681) -> ()
          }
          frame Error {
          }
        }
        n311 = call <vilib>:"Add State(s) to Queue__JKI_lib_State_Machine.vi"("State(s) in (\"\")"=w665) -> ("States Out"=w664:string)  [unwired: 14 in]
      }
      frame "Data: loadLastUseBG" {
        w684 = enum16{"write", "read"}."write" ("action")
        # "Load last use BG.\n()"
        n312 = Unbundle By Name(w704) -> ("TempPath"=w703:path)
        n313 = call "FLImDAQ_FGV.vi"() -> ("Read data"=w699:T6)  [unwired: 10 in, 1 out]
        n314 = Build Path(base path=w703, name or relative path="Background.tdms") -> (appended path=w702:path)
        n315 = call "ReadBGorCali (SubVI).vi"("DataType"=enum16{"BG", "Cali"}."BG", "error in (no error)"=w701, "file path in"=w702) -> ("error out"=w700:errorcluster, "AvgDataCluster"=w695:T34)  [unwired: 6 in, 1 out]
        n316 = Unbundle By Name(w695) -> ("Channel 1"=w687:dbl[], "Channel 2"=w694:dbl[], "Channel 3"=w686:dbl[], "Channel 4"=w683:dbl[])
        n317 = Unbundle By Name(w699) -> ("min record length"=w691:i32)
        n318 = Array Size(array=w686) -> (size(s)=w693:i32)
        "BG length" <- w693
        n319 = Equal?(x=w693, y=w691) -> (x = y?=w692:bool)
        n320 = Select(t="UI: BGLoaded" ("State(s) in Front (\"\")"), s=w692, f="UI: BGSizeError" ("State(s) in Front (\"\")")) -> (s? t:f=w696:string)
        n321 = case shown="False" w692 {
          tunnel: w687 -> [_ w715]
          tunnel: w694 -> [_ w714]
          tunnel: w686 -> [_ w713]
          tunnel: w691 -> [w710 _]
          tunnel: [w709 w715] -> w690
          tunnel: [w709 w714] -> w689
          tunnel: [w709 w713] -> w688
          tunnel: w683 -> [_ w712]
          tunnel: [w709 w712] -> w682
          frame False {
            # "If error set BG all 0, update UI"
            n322 = for {
              N: w710 -> [_]
              tunnel: [0.0] -> w709 mode=indexing
            }
          }
          frame True {
            # "If no error, check size match"
          }
        }
        n323 = call "BG4FGV.vi"("action"=w684, "BG4 in"=w682) -> ()  [unwired: 8 in, 2 out]
        n324 = call "BG3FGV.vi"("action"=w684, "BG3 in"=w688) -> ()  [unwired: 8 in, 2 out]
        n325 = call "BG1FGV.vi"("action"=w684, "BG1 in"=w690) -> ()  [unwired: 8 in, 2 out]
        n326 = call "BG2FGV.vi"("action"=w684, "BG2 in"=w689) -> ()  [unwired: 8 in, 2 out]
        n327 = call <vilib>:"Add State(s) to Queue__JKI_lib_State_Machine.vi"("State(s) in Front (\"\")"=w696, "State(s) in (\"\")"=w708) -> ("States Out"=w707:string)  [unwired: 13 in]
      }
      frame "Data: loadLastUseMacro" {
        # "Load last use BG and Cali and iRF.\n(It is a separator no-op. You can make a copy of this frame to create a new Data frame)"
        n328 = call <vilib>:"Add State(s) to Queue__JKI_lib_State_Machine.vi"("State(s) in Front (\"\")"="Data: loadLastUseBG\nData: loadSystemCali\nData: loadLastUseiRF\n/*Data: LoadAPDData" ("State(s) in Front (\"\")"), "State(s) in (\"\")"=w721) -> ("States Out"=w720:string)  [unwired: 13 in]
      }
      frame "Data: saveCalibration" {
        # "Average data and save calibration file. [Covers: REQ11]\n(It is a separator no-op. You can make a copy of this frame to create a new Data frame)"
        n329 = Unbundle By Name(w740) -> ("Ch1Data"=w739:dbl[][], "V1"=w738:dbl[], "Ch2Data"=w737:dbl[][], "V2"=w736:dbl[], "Ch3Data"=w735:dbl[][], "V3"=w734:dbl[], "Ch4Data"=w725:dbl[][], "V4"=w724:dbl[], "Pathes.CaliPath"=w743:path, "IDs.Cali ID"=w742:i8)
        n330 = Increment(x=w742) -> (x+1=w726:i8)
        n331 = Bundle("Ch1Data"=w739, "V1"=w738) -> (w733:cluster{"Ch1Data":dbl[][], "V1":dbl[]})  [unwired: 1 in]
        n332 = Bundle("Ch4Data"=w725, "V4"=w724) -> (w723:cluster{"Ch4Data":dbl[][], "V4":dbl[]})  [unwired: 1 in]
        n333 = Bundle("Ch2Data"=w737, "V2"=w736) -> (w732:cluster{"Ch2Data":dbl[][], "V2":dbl[]})  [unwired: 1 in]
        n334 = Bundle("Ch3Data"=w735, "V3"=w734) -> (w731:cluster{"Ch3Data":dbl[][], "V3":dbl[]})  [unwired: 1 in]
        n335 = Format Value(string ("")="Calibration" ("default name"), format string="%02d", value (0)=w726) -> (output string=w745:string)
        n336 = Build Path(base path=w743, name or relative path=w745) -> (appended path=w730:path)
        n337 = call "SaveBGorCali (SubVI).vi"("Channel1"=w733, "BG path"=w730, "DataType"=enum16{"BG", "Cali"}."Cali", "Channel 2"=w732, "Channel 3"=w731, "Channel 4"=w723, "error in (no error)"=w729, "SytemID"="UCDVetMed") -> ("error out"=w728:errorcluster)  [unwired: 7 in]
        n338 = call <vilib>:"Add State(s) to Queue__JKI_lib_State_Machine.vi"("State(s) in (\"\")"=w748) -> ("States Out"=w747:string)  [unwired: 14 in]
      }
      frame "Data: saveiRF" {
        w754 = enum16{"write", "read"}."read" ("action")
        # "Get iRF from decon stracture and save it on disk.\n(It is a separator no-op. You can make a copy of this frame to create a new Data frame)"
        n339 = Unbundle By Name(w771) -> ("TempPath"=w770:path)
        n340 = call "Ch1DeconEngineFGV.vi"("action(read)"=w754) -> ("Error Out"=w776:errorcluster, "Ch1DeconEngine out"=w777:refnum<class "LaguerreDeconEngineClass.lvclass">)  [unwired: 9 in]
        n341 = call "Ch2DeconEngineFGV.vi"("action(read)"=w754) -> ("Error Out"=w774:errorcluster, "Ch2DeconEngine out"=w775:refnum<class "LaguerreDeconEngineClass.lvclass">)  [unwired: 9 in]
        n342 = call "Ch3DeconEngineFGV.vi"("action(read)"=w754) -> ("Error Out"=w772:errorcluster, "Ch3DeconEngine out"=w773:refnum<class "LaguerreDeconEngineClass.lvclass">)  [unwired: 9 in]
        n343 = call "Ch4DeconEngineFGV.vi"("action(read)"=w754) -> ("Error Out"=w753:errorcluster, "Ch3DeconEngine out"=w752:refnum<class "LaguerreDeconEngineClass.lvclass">)  [unwired: 9 in]
        n344 = Build Path(base path=w770, name or relative path="iRF" ("default name")) -> (appended path=w768:path)
        n345 = call "getIRF.vi"("error in (no error)"=w753, "LaguerreDeconEngineClass in"=w752) -> ("iRF"=w751:dbl[])  [unwired: 7 in, 2 out]
        n346 = call "getIRF.vi"("error in (no error)"=w776, "LaguerreDeconEngineClass in"=w777) -> ("iRF"=w759:dbl[])  [unwired: 7 in, 2 out]
        n347 = call "getIRF.vi"("error in (no error)"=w774, "LaguerreDeconEngineClass in"=w775) -> ("iRF"=w758:dbl[])  [unwired: 7 in, 2 out]
        n348 = call "getIRF.vi"("error in (no error)"=w772, "LaguerreDeconEngineClass in"=w773) -> ("iRF"=w757:dbl[])  [unwired: 7 in, 2 out]
        n349 = TDMS Open(8:w767, 10:T16."create or replace" ("operation (0:open)"), 11:w768) -> (0:w764:errorcluster, 3:w765:refnum<k34>)  [unwired: 4 in]
        n350 = Bundle(cluster=T15 {"Ch1 iRF"=[], "Ch2 iRF"=[], "Ch3 iRF"=[], "Ch4 iRF"=[]} ("LastUseiRF"), "Ch1 iRF"=w759, "Ch2 iRF"=w758, "Ch3 iRF"=w757, "Ch4 iRF"=w751) -> (w755:T15)
        n351 = Build Array(w759, w758, w757, w751) -> (w763:dbl[][])
        n352 = global write "GlobalVariables.vi" "LastUseiRF"(w755) -> ()
        n353 = TDMS Write(0:w765, 5:"iRF" ("group name in (Untitled)"), 7:string[] ["Ch1", "Ch2", "Ch3", "Ch4"] ("channel name(s) in (Untitled)"), 9:w763, 11:w764) -> (4:w762:refnum<k34>, 15:w761:errorcluster)  [unwired: 1 in, 2 out]
        n354 = TDMS Close(8:w761, 11:w762) -> (0:w760:errorcluster)  [unwired: 1 out]
        n355 = call <vilib>:"Add State(s) to Queue__JKI_lib_State_Machine.vi"("State(s) in (\"\")"=w780) -> ("States Out"=w779:string)  [unwired: 14 in]
      }
      frame "Data: saveBGtoFGV" {
        w781 = enum16{"write", "read"}."write" ("action")
        # "Save BG and pass it to FGV.\n(save BG to disk and set it to FGV)"
        n356 = Unbundle By Name(w791) -> ("Ch1Data"=w790:dbl[][], "Ch2Data"=w789:dbl[][], "Ch3Data"=w788:dbl[][], "Ch4Data"=w783:dbl[][])
        n357 = call "AvgArrayTimeCritical.vi"("2D array"=w790) -> ("1D Avg"=w787:dbl[])  [unwired: 10 in]
        n358 = call "AvgArrayTimeCritical.vi"("2D array"=w789) -> ("1D Avg"=w786:dbl[])  [unwired: 10 in]
        n359 = call "AvgArrayTimeCritical.vi"("2D array"=w788) -> ("1D Avg"=w785:dbl[])  [unwired: 10 in]
        n360 = call "AvgArrayTimeCritical.vi"("2D array"=w783) -> ("1D Avg"=w782:dbl[])  [unwired: 10 in]
        n361 = call "BG1FGV.vi"("action"=w781, "BG1 in"=w787) -> ()  [unwired: 8 in, 2 out]
        n362 = call "BG2FGV.vi"("action"=w781, "BG2 in"=w786) -> ()  [unwired: 8 in, 2 out]
        n363 = call "BG3FGV.vi"("action"=w781, "BG3 in"=w785) -> ()  [unwired: 8 in, 2 out]
        n364 = call "BG4FGV.vi"("action"=w781, "BG4 in"=w782) -> ()  [unwired: 8 in, 2 out]
        n365 = call <vilib>:"Add State(s) to Queue__JKI_lib_State_Machine.vi"("State(s) in (\"\")"=w794) -> ("States Out"=w793:string)  [unwired: 14 in]
      }
      frame "Data: saveBGtoFile" {
        w816 = "Background" ("name or relative path")
        # "Save BG to file.\n(save BG to disk both data folder and temp folder)"
        n366 = Unbundle By Name(w820) -> ("Pathes.BG Path"=w813:path, "IDs.BG ID"=w812:i8, "Ch1Data"=w810:dbl[][], "V1"=w809:dbl[], "Ch2Data"=w808:dbl[][], "V2"=w807:dbl[], "Ch3Data"=w806:dbl[][], "V3"=w805:dbl[], "Ch4Data"=w797:dbl[][], "V4"=w796:dbl[], "TempPath"=w818:path)
        n367 = Increment(x=w812) -> (x+1=w817:i8)
        n368 = Format Value(string ("")=w816, format string="%02d", value (0)=w817) -> (output string=w815:string)
        n369 = Build Path(base path=w818, name or relative path=w816) -> (appended path=w799:path)
        n370 = call "File Dialog2"("start path"=w813, "prompt"="Please select BG name, DO NOT CANCEL!", "default name"=w815) -> ("selected path"=w800:path)  [unwired: 9 in, 3 out]
        n371 = Bundle("Ch1Data"=w810, "V1"=w809) -> (w804:cluster{"Ch1Data":dbl[][], "V1":dbl[]})  [unwired: 1 in]
        n372 = Bundle("Ch4Data"=w797, "V4"=w796) -> (w795:cluster{"Ch4Data":dbl[][], "V4":dbl[]})  [unwired: 1 in]
        n373 = Bundle("Ch2Data"=w808, "V2"=w807) -> (w803:cluster{"Ch2Data":dbl[][], "V2":dbl[]})  [unwired: 1 in]
        n374 = Bundle("Ch3Data"=w806, "V3"=w805) -> (w802:cluster{"Ch3Data":dbl[][], "V3":dbl[]})  [unwired: 1 in]
        n375 = Build Array(w800, w799) -> (w798:path[])
        n376 = for {
          tunnel: w804 -> [w831]
          tunnel: w803 -> [w830]
          tunnel: w802 -> [w829]
          shift-right: [w832] -> w811
          shift-left: w801 -> [w828]
          tunnel: w798 -> [w827] mode=indexing
          tunnel: w795 -> [w825]
          n377 = call "SaveBGorCali (SubVI).vi"("Channel1"=w831, "BG path"=w827, "DataType"=enum16{"BG", "Cali"}."BG", "Channel 2"=w830, "Channel 3"=w829, "Channel 4"=w825, "error in (no error)"=w828, "SytemID"="UCDVetMed") -> ("error out"=w832:errorcluster)  [unwired: 7 in]
        }
        n378 = call <vilib>:"Add State(s) to Queue__JKI_lib_State_Machine.vi"("State(s) in (\"\")"=w823) -> ("States Out"=w822:string)  [unwired: 14 in]
      }
      frame "Data: showBG" {
        # "Show BG in seperate window.\n()"
        n379 = call "showBG.vi"() -> ()  [unwired: 12 in]
        n380 = call <vilib>:"Add State(s) to Queue__JKI_lib_State_Machine.vi"("State(s) in (\"\")"=w837) -> ("States Out"=w836:string)  [unwired: 14 in]
      }
      frame "Data: irfAlignment" {
        w904 = enum16{"write", "read"}."write" ("action")
        # "do iRF alignment in this state\n(It is a separator no-op. You can make a copy of this frame to create a new Data frame)"
        n381 = Unbundle By Name(w882) -> ("Ch1Data"=w919:dbl[][], "Ch2Data"=w918:dbl[][], "Ch3Data"=w917:dbl[][], "Ch4Data"=w859:dbl[][])
        n382 = call "Ch1DeconEngineFGV.vi"("Error In"=w858) -> ("Error Out"=w915:errorcluster, "Ch1DeconEngine out"=w916:refnum<class "LaguerreDeconEngineClass.lvclass">)  [unwired: 9 in]
        n383 = call "Ch2DeconEngineFGV.vi"("Error In"=w858) -> ("Error Out"=w913:errorcluster, "Ch2DeconEngine out"=w914:refnum<class "LaguerreDeconEngineClass.lvclass">)  [unwired: 9 in]
        n384 = call "Ch3DeconEngineFGV.vi"("Error In"=w858) -> ("Error Out"=w911:errorcluster, "Ch3DeconEngine out"=w912:refnum<class "LaguerreDeconEngineClass.lvclass">)  [unwired: 9 in]
        n385 = call "Ch4DeconEngineFGV.vi"("Error In"=w858) -> ("Error Out"=w849:errorcluster, "Ch3DeconEngine out"=w848:refnum<class "LaguerreDeconEngineClass.lvclass">)  [unwired: 9 in]
        n386 = call "AvgArray.vi"("2D array in"=w918) -> ("1D Avg out"=w864:dbl[])  [unwired: 10 in]
        n387 = call "AvgArray.vi"("2D array in"=w917) -> ("1D Avg out"=w863:dbl[])  [unwired: 10 in]
        n388 = call "AvgArray.vi"("2D array in"=w859) -> ("1D Avg out"=w838:dbl[])  [unwired: 10 in]
        n389 = call "AvgArray.vi"("2D array in"=w919) -> ("1D Avg out"=w865:dbl[])  [unwired: 10 in]
        n390 = call "RemoveDCBG.vi"("WF in"=w865) -> ("DC"=w872:dbl, "WF out"=w862:dbl[])  [unwired: 8 in, 1 out]
        n391 = call "RemoveDCBG.vi"("WF in"=w864) -> ("DC"=w869:dbl, "WF out"=w875:dbl[])  [unwired: 8 in, 1 out]
        n392 = call "RemoveDCBG.vi"("WF in"=w863) -> ("DC"=w867:dbl, "WF out"=w874:dbl[])  [unwired: 8 in, 1 out]
        n393 = call "RemoveDCBG.vi"("WF in"=w838) -> ("DC"=w842:dbl, "WF out"=w840:dbl[])  [unwired: 8 in, 1 out]
        n394 = call "computeIRFAlignment.vi"("error in (no error)"=w915, "fIRF temp"=w862, "LaguerreDeconEngineClass in"=w916) -> ("error out"=w907:errorcluster, "LaguerreDeconEngineClass out"=w908:refnum<class "LaguerreDeconEngineClass.lvclass">)  [unwired: 6 in, 1 out]
        n395 = call "computeIRFAlignment.vi"("error in (no error)"=w913, "fIRF temp"=w875, "LaguerreDeconEngineClass in"=w914) -> ("error out"=w905:errorcluster, "LaguerreDeconEngineClass out"=w906:refnum<class "LaguerreDeconEngineClass.lvclass">)  [unwired: 6 in, 1 out]
        n396 = call "computeIRFAlignment.vi"("error in (no error)"=w911, "fIRF temp"=w874, "LaguerreDeconEngineClass in"=w912) -> ("error out"=w909:errorcluster, "LaguerreDeconEngineClass out"=w910:refnum<class "LaguerreDeconEngineClass.lvclass">)  [unwired: 6 in, 1 out]
        n397 = call "computeIRFAlignment.vi"("error in (no error)"=w849, "fIRF temp"=w840, "LaguerreDeconEngineClass in"=w848) -> ("error out"=w856:errorcluster, "LaguerreDeconEngineClass out"=w857:refnum<class "LaguerreDeconEngineClass.lvclass">)  [unwired: 6 in, 1 out]
        n398 = call "Ch1DeconEngineFGV.vi"("Error In"=w907, "action(read)"=w904, "Ch1DeconEngine in"=w908) -> ("Error Out"=w902:errorcluster, "Ch1DeconEngine out"=w903:refnum<class "LaguerreDeconEngineClass.lvclass">)  [unwired: 7 in]
        n399 = call "Ch2DeconEngineFGV.vi"("Error In"=w905, "action(read)"=w904, "Ch2DeconEngine in"=w906) -> ("Error Out"=w892:errorcluster, "Ch2DeconEngine out"=w893:refnum<class "LaguerreDeconEngineClass.lvclass">)  [unwired: 7 in]
        n400 = call "Ch3DeconEngineFGV.vi"("Error In"=w909, "action(read)"=w904, "Ch3DeconEngine in"=w910) -> ("Error Out"=w886:errorcluster, "Ch3DeconEngine out"=w887:refnum<class "LaguerreDeconEngineClass.lvclass">)  [unwired: 7 in]
        n401 = call "Ch3DeconEngineFGV.vi"("Error In"=w856, "Ch3DeconEngine in"=w857) -> ("Error Out"=w850:errorcluster, "Ch3DeconEngine out"=w851:refnum<class "LaguerreDeconEngineClass.lvclass">)  [unwired: 8 in]
        n402 = call "setfIRF.vi"("error in (no error)"=w886, "fIRF"=w874, "LaguerreDeconEngineClass in"=w887) -> ("error out"=w890:errorcluster, "LaguerreDeconEngineClass out"=w891:refnum<class "LaguerreDeconEngineClass.lvclass">)  [unwired: 7 in]
        n403 = call "setfIRF.vi"("error in (no error)"=w850, "fIRF"=w840, "LaguerreDeconEngineClass in"=w851) -> ("error out"=w854:errorcluster, "LaguerreDeconEngineClass out"=w855:refnum<class "LaguerreDeconEngineClass.lvclass">)  [unwired: 7 in]
        n404 = call "setfIRF.vi"("error in (no error)"=w892, "fIRF"=w875, "LaguerreDeconEngineClass in"=w893) -> ("error out"=w896:errorcluster, "LaguerreDeconEngineClass out"=w897:refnum<class "LaguerreDeconEngineClass.lvclass">)  [unwired: 7 in]
        n405 = call "setfIRF.vi"("error in (no error)"=w902, "fIRF"=w862, "LaguerreDeconEngineClass in"=w903) -> ("error out"=w900:errorcluster, "LaguerreDeconEngineClass out"=w901:refnum<class "LaguerreDeconEngineClass.lvclass">)  [unwired: 7 in]
        n406 = Unbundle By Name(w882) -> ("V1"=w861:dbl[], "V2"=w881:dbl[], "V3"=w880:dbl[], "V4"=w847:dbl[])
        n407 = call "computeLCs.vi"("error in (no error)"=w900, "LaguerreDeconClass in"=w901) -> ("error out"=w898:errorcluster, "LaguerreDeconClass out"=w899:refnum<class "LaguerreDeconEngineClass.lvclass">)  [unwired: 8 in]
        n408 = call "computeLCs.vi"("error in (no error)"=w896, "LaguerreDeconClass in"=w897) -> ("error out"=w894:errorcluster, "LaguerreDeconClass out"=w895:refnum<class "LaguerreDeconEngineClass.lvclass">)  [unwired: 8 in]
        n409 = call "computeLCs.vi"("error in (no error)"=w890, "LaguerreDeconClass in"=w891) -> ("error out"=w888:errorcluster, "LaguerreDeconClass out"=w889:refnum<class "LaguerreDeconEngineClass.lvclass">)  [unwired: 8 in]
        n410 = call "computeLCs.vi"("error in (no error)"=w854, "LaguerreDeconClass in"=w855) -> ("error out"=w852:errorcluster, "LaguerreDeconClass out"=w853:refnum<class "LaguerreDeconEngineClass.lvclass">)  [unwired: 8 in]
        n411 = call-poly <vilib>:"Mean.vi"("X"=w861) -> ("mean"=w860:dbl)  [unwired: 1 out]
        n412 = call-poly <vilib>:"Mean.vi"("X"=w847) -> ("mean"=w846:dbl)  [unwired: 1 out]
        n413 = call-poly <vilib>:"Mean.vi"("X"=w881) -> ("mean"=w879:dbl)  [unwired: 1 out]
        n414 = call "getFitting.vi"("error in (no error)"=w898, "LaguerreDeconEngineClass in"=w899) -> ("Fitting"=w871:dbl[])  [unwired: 7 in, 2 out]
        n415 = call "getFitting.vi"("error in (no error)"=w894, "LaguerreDeconEngineClass in"=w895) -> ("Fitting"=w868:dbl[])  [unwired: 7 in, 2 out]
        n416 = call "getFitting.vi"("error in (no error)"=w888, "LaguerreDeconEngineClass in"=w889) -> ("Fitting"=w844:dbl[])  [unwired: 7 in, 2 out]
        n417 = call "getFitting.vi"("error in (no error)"=w852, "LaguerreDeconEngineClass in"=w853) -> ("Fitting"=w843:dbl[])  [unwired: 7 in, 2 out]
        n418 = Add(x=w872, y=w871) -> (x+y=w873:dbl[])
        n419 = Add(x=w869, y=w868) -> (x+y=w870:dbl[])
        n420 = call-poly <vilib>:"Mean.vi"("X"=w880) -> ("mean"=w878:dbl)  [unwired: 1 out]
        n421 = Add(x=w867, y=w844) -> (x+y=w866:dbl[])
        n422 = Build Array(w865, w873) -> (w885:dbl[][])
        n423 = Build Array(w864, w870) -> (w884:dbl[][])
        n424 = Build Array(w863, w866) -> (w883:dbl[][])
        n425 = Add(x=w842, y=w843) -> (x+y=w841:dbl[])
        n426 = Bundle("mean"=w860, "mean"=w879, "mean"=w878, "mean"=w846) -> (w845:T36)  [unwired: 1 in]
        n427 = Build Array(w838, w841) -> (w839:dbl[][])
        n428 = call "Calib_and_iRFAlign_confirm.vi"("Current V"=w845, "Ch4 Data"=w839, "Ch3 Data"=w883, "Ch2 Data"=w884, "Ch1 Data"=w885) -> ("Save?"=w877:bool)  [unwired: 6 in]
        n429 = case shown="True" w877 {
          tunnel: ["" ("Empty String Constant") "Data: saveCalibration\nData: saveiRF\nRun: CaliIncrement"] -> w876
          frame False {
          }
          frame True {
            # "[Covers: REQ2]"
          }
        }
        n430 = call <vilib>:"Add State(s) to Queue__JKI_lib_State_Machine.vi"("State(s) in Front (\"\")"=w876, "State(s) in (\"\")"=w922) -> ("States Out"=w921:string)  [unwired: 13 in]
      }
      frame "Data: parseRunData" {
        # "All APD bias"
        # "flash queue"
        # "Ch3&4"
        # "Ch1&2"
        # "Flash data from queue and save it in structure\n()"
        n431 = Flush Queue(queue=w950, error in (no error)=w949) -> (remaining elements=w944:T37, error out=w945:errorcluster)  [unwired: 1 out]
        n432 = Flush Queue(queue=w955, error in (no error)=w949) -> (remaining elements=w953:cluster{"double data":dbl[][]}[], error out=w946:errorcluster)  [unwired: 1 out]
        n433 = Flush Queue(queue=w956, error in (no error)=w949) -> (remaining elements=w954:cluster{"double data":dbl[][]}[], error out=w947:errorcluster)  [unwired: 1 out]
        n434 = for {
          tunnel: w954 -> [w972] mode=indexing
          tunnel: [w970] -> w939 mode=concatenating
          tunnel: [w969] -> w940 mode=concatenating
          n435 = Unbundle By Name(w972) -> ("double data"=w971:dbl[][])
          n436 = call "SeperateChanData.vi"("Input (Ch1&2)"=w971) -> ("Ch1"=w970:dbl[][], "Ch2"=w969:dbl[][])
        }
        n437 = for {
          tunnel: w953 -> [w968] mode=indexing
          tunnel: [w967] -> w929 mode=concatenating
          tunnel: [w965] -> w930 mode=concatenating
          n438 = Unbundle By Name(w968) -> ("double data"=w966:dbl[][])
          n439 = call "SeperateChanData.vi"("Input (Ch1&2)"=w966) -> ("Ch1"=w967:dbl[][], "Ch2"=w965:dbl[][])
        }
        n440 = call "FLImDAQ_FGV.vi"() -> ("Read data"=w937:T6)  [unwired: 10 in, 1 out]
        n441 = Unbundle By Name(w937) -> ("Waveform to Avg"=w927:i16)
        n442 = for {
          tunnel: w944 -> [w964] mode=indexing
          tunnel: [w963] -> w936 mode=indexing
          tunnel: [w962] -> w934 mode=indexing
          tunnel: [w961] -> w932 mode=indexing
          tunnel: [w960] -> w928 mode=indexing
          n443 = Unbundle By Name(w964) -> ("V1"=w963:dbl, "V2"=w962:dbl, "V3"=w961:dbl, "V4"=w960:dbl)
        }
        n444 = call "DuplicateV(SubVI).vi"("Averaging"=w927, "V in"=w936) -> ("V out"=w935:dbl[])  [unwired: 9 in]
        n445 = Array Size(array=w929) -> (size(s)=→"data Size":i32[])
        n446 = call "DuplicateV(SubVI).vi"("Averaging"=w927, "V in"=w934) -> ("V out"=w933:dbl[])  [unwired: 9 in]
        n447 = call "DuplicateV(SubVI).vi"("Averaging"=w927, "V in"=w932) -> ("V out"=w931:dbl[])  [unwired: 9 in]
        n448 = call "DuplicateV(SubVI).vi"("Averaging"=w927, "V in"=w928) -> ("V out"=w925:dbl[])  [unwired: 9 in]
        n449 = Bundle By Name(cluster=w951, "Ch1Data"=w939, "Ch2Data"=w940, "Ch3Data"=w929, "Ch4Data"=w930, "V1"=w935, "V2"=w933, "V3"=w931, "V4"=w925) -> (w952:T23)
        n450 = Merge Errors(w947, w946, w945) -> (w948:errorcluster)
        n451 = Array Size(array=w935) -> (size(s)=→"V1 Size":i32)
        n452 = Array Size(array=w933) -> (size(s)=→"V2 Size":i32)
        n453 = Array Size(array=w931) -> (size(s)=→"V3 Size":i32)
        n454 = Array Size(array=w925) -> (size(s)=→"V4 Size":i32)
        n455 = call <vilib>:"Add State(s) to Queue__JKI_lib_State_Machine.vi"("State(s) in (\"\")"=w959) -> ("States Out"=w958:string)  [unwired: 14 in]
      }
      frame "Data: saveRunData" {
        w975 = T38 {"DataPath"=path "", "CaseID"="", "RunID"=0, "Ch1Data"=[], "Ch2Data"=[], "Ch3Data"=[], "Ch4Data"=[], "V1"=[], "V2"=[], "V3"=[], "V4"=[], "LaserRepRate"=0, "WFAverage"=0, "RunStartTime"=0}  # Data cluster
        # "Save FLIm data to disk.\n(Save to LV tdms file format)"
        n456 = Unbundle By Name(w986) -> ("Pathes.DataPath"=w982:path, "CaseID"=w994:string, "IDs.RunID"=w984:i8, "Ch1Data"=w993:dbl[][], "Ch2Data"=w992:dbl[][], "Ch3Data"=w981:dbl[][], "Ch4Data"=w974:dbl[][], "V1"=w976:dbl[], "V2"=w991:dbl[], "V3"=w990:dbl[], "V4"=w973:dbl[])
        n457 = call "FLImDAQ_FGV.vi"() -> ("Read data"=w979:T6)  [unwired: 10 in, 1 out]
        n458 = Unbundle By Name(w979) -> ("Waveform to Avg"=w978:i16)
        n459 = local read "RunStartTime"() -> (w977:u32)
        n460 = local read "Laser Rep Rate"() -> (w980:dbl)
        n461 = Increment(x=w984) -> (x+1=w983:i8)
        n462 = Bundle By Name(cluster=w975, "DataPath"=w982, "CaseID"=w994, "RunID"=w983, "Ch1Data"=w993, "Ch2Data"=w992, "Ch3Data"=w981, "Ch4Data"=w974, "V1"=w976, "V2"=w991, "V3"=w990, "V4"=w973, "LaserRepRate"=w980, "WFAverage"=w978, "RunStartTime"=w977) -> (w989:T38)
        n463 = call "SaveRunData(SubVI).vi"("Data cluster"=w989, "error in (no error)"=w988) -> ("error out"=w985:errorcluster)  [unwired: 13 in]
        n464 = flat-sequence {
          tunnel: w986 -> [w1002]
          tunnel: [w1001] -> w987
          tunnel: w985 -> [_]
          frame #0 {
            w999 = dbl[][] [] ("Ch1Data")
            w1000 = dbl[] [] ("V1")
            # "reset local data"
            n465 = Bundle By Name(cluster=w1002, "Ch1Data"=w999, "Ch2Data"=w999, "Ch3Data"=w999, "Ch4Data"=w999, "V1"=w1000, "V2"=w1000, "V3"=w1000, "V4"=w1000) -> (w1001:T23)
          }
        }
        n466 = case shown="No Error" w985 {
          tunnel: ["Run: Increment" "" ("Empty String Constant")] -> w995
          frame No Error {
          }
          frame Error {
          }
        }
        n467 = call <vilib>:"Add State(s) to Queue__JKI_lib_State_Machine.vi"("State(s) in Front (\"\")"=w995, "State(s) in (\"\")"=w998) -> ("States Out"=w997:string)  [unwired: 13 in]
      }
      frame "Data: Cleanup" {
        # "Cleanup any data and references, here.\n(this is called automatically, by the Macro: Exit)"
        n468 = Unbundle By Name(w1006) -> ("Core.Current VI Reference"=w1009:refnum<vi>)
        n469 = Close Reference(reference=w1009, error in (no error)=w1008) -> (error out=w1007:errorcluster)
        n470 = call <vilib>:"Add State(s) to Queue__JKI_lib_State_Machine.vi"("State(s) in (\"\")"=w1011) -> ("States Out"=w1010:string)  [unwired: 14 in]
      }
      frame "---------- Core ----------" {
        # "Do not put any code in this frame.\n(it is a separator no-op)"
        n471 = call <vilib>:"Add State(s) to Queue__JKI_lib_State_Machine.vi"("State(s) in (\"\")"=w1016) -> ("States Out"=w1015:string)  [unwired: 14 in]
      }
      frame Default {
        w1027 = 42 items=["No error", "Argument error", "Memory is full", "Out of zone", "End of file", "File already open", "Generic file I/O error", "File not found", "File permission error", "Disk is full", "Duplicate path", "Too many files open", "System feature not enabled", "Resource file not found", "Cannot add resource", "Resource not found", "Image not found", "Image memory error", "Pen does not exist", "Config type invalid", "Config token not found", "Config parse error", "Config memory error", "Bad external code format", "Bad external code offset", "External code not present", "Null window", "Destroy window error", "Null menu", "Print aborted", "Bad print record", "Print driver error", "Windows error during printing", "Memory error during printing", "Print dialog error", "Generic print error", "Invalid device refnum", "Device not found", "Device parameter error", "Device unit error", "Cannot open device", "Device call aborted", "Generic error", "Cancelled by user", "Object ID too low", "Object ID too high", "Object not in heap", "Unknown heap", "Unknown object (invalid DefProc)", "Unknown object (DefProc not in table)", "Message out of range", "Invalid (null) method", "Unknown message", "Manager call not supported", "Bad address", "Network operation in progress", "Network operation timed out", "Connection is busy", "Network attribute not supported", "Network error", "Address in use", "System out of memory", "Connection aborted", "Connection refused", "Not connected", "Already connected", "Connection closed", "Initialization error (interapplication manager)", "Bad occurrence", "Wait on unbound occurrence handler", "Occurrence queue overflow", "Datalog type conflict", "Unused", "Unrecognized type (interapplication manager)", "Memory corrupt", "Failed to make temporary DLL", "Old CIN version", "Drag socket not found", "Failed to load drop-object", "Failed to register OLE object", "Failed to release OLE object", "Format specifier type mismatch", "Unknown format specifier", "Too few format specifiers", "Too many format specifiers", "Scan failed", "Newer CIN version", "Error converting to variant", "Runtime menu error", "Password tampered", "Variant attribute not found", "Incompatible variant data type", "Event data is not available", "Event Store is not present", "Occurrence is not found", "Event Queue is not created", "Event info is not available", "Refnum passed is NULL", "Error retrieving Class GUID", "Error retrieving CoClass GUID", "Error retrieving TypeLib GUID.", "Bad built application magic bytes.", "Specific driver is different from the specific driver associated with the Logical Name.", "There is no session opened to the class driver.", "Max Error", "MAX - Error with config objects", "MAX - Error loading configuration", "MAX - Group not supported"]
        # "Current State"
        # "Do not delete, rename, or modify this frame.\n(this is used to capture unhandled states and typos)"
        # "Handle mistyped state name (developer tool)"
        n472 = Format Into String(format string="Software Exception: Unhandled State \"%s\"." ("message"), error in=w1023, w1018) -> (resulting string=w1026:string, error out=w1025:errorcluster)  [unwired: 1 in]
        n473 = call <vilib>:"Error Cluster From Error Code.vi"("show call chain? (False)"=TRUE, "error in (no error)"=w1025, "error message (\"\")"=w1026, "error code (0)"=w1027) -> ("error out"=w1024:errorcluster)  [unwired: 5 in]
        n474 = call <vilib>:"Add State(s) to Queue__JKI_lib_State_Machine.vi"("State(s) in (\"\")"=w1022) -> ("States Out"=w1021:string)  [unwired: 14 in]
      }
      frame "Initialize Core Data" {
        # "Build default path based on the location of project"
        # "Do not delete, rename, or modify this frame.\n(this is used to determine panel behavior on exit)"
        # "originally closed?"
        # "exe?"
        # "If panel starts closed or is an EXE, then close it when we exit"
        n475 = call <vilib>:"Application Directory.vi"() -> ("Application Directory"=w1030:path)
        n476 = property on="Property Node" class="App"() -> ("App.Kind"=w1046:T18)  [unwired: 2 in, 2 out]
        n477 = property on="Property Node" class="VI"() -> ("FP.State"=w1040:T17)  [unwired: 2 in, 2 out]
        n478 = control-ref of="Current VI Reference"() -> (w1041:refnum<vi>)
        n479 = Strip Path(path=w1030) -> (stripped path=w1029:path)  [unwired: 1 out]
        n480 = Equal?(x=w1040, y=T17."Closed" ("Front Panel Window:State")) -> (x = y?=w1038:bool)
        n481 = Equal?(x=w1046, y=T18."Run Time System" ("Application:Kind")) -> (x = y?=w1044:bool)
        n482 = Build Path(base path=w1029, name or relative path="Data") -> (appended path=w1036:path)
        n483 = Build Path(base path=w1030, name or relative path="SystemTemp") -> (appended path=w1033:path)
        n484 = Build Path(base path=w1030, name or relative path="SystemCalibrationFile") -> (appended path=w1031:path)
        n485 = Or(x=w1038, y=w1044) -> (x .or. y?=w1042:bool)
        n486 = Bundle By Name(cluster=w1043, "Core.Current VI Reference"=w1041, "Core.Close Panel on Exit?"=w1042, "DefaultPath"=w1036, "TempPath"=w1033, "CaliPath"=w1031) -> (w1048:T23)
        n487 = call <vilib>:"Add State(s) to Queue__JKI_lib_State_Machine.vi"("State(s) in (\"\")"=w1050) -> ("States Out"=w1049:string)  [unwired: 14 in]
      }
      frame "Error Handler" {
        # "Unhandled Error -- Display it"
        # "Handle any errors here.\nYou can also output any states to clean-up after errors occur"
        # "Clear error"
        n488 = Unbundle By Name(w1051) -> ("code"=w1053:i32)
        n489 = case shown="Default" w1053 {
          tunnel: ["Macro: Exit" w1063 w1069] -> w1052
          tunnel: w1051 -> [w1059 _ _]
          frame Default {
            w1061 = T39 1 items=["no dialog", "OK message", "continue or stop message", "OK message + warnings", "continue/stop + warnings"] ("type of dialog (OK msg:1)")
            n490 = call <vilib>:"General Error Handler.vi"("type of dialog (OK msg:1)"=w1061, "error in (no error)"=w1059) -> ()  [unwired: 9 in, 5 out]
          }
          frame 5002 {
            n491 = Two Button Dialog(message="Laser interlock open! Please close interlock and try again! ", 1:"Safely Shutdown" ("F button name (\"Cancel\")"), 2:"OK" ("T button name (\"OK\")")) -> (T button?=w1064:bool)
            n492 = case shown="True" w1064 {
              tunnel: ["Macro: Exit" "355 Laser: CheckControllerStatus"] -> w1063
              frame False {
              }
              frame True {
              }
            }
          }
          frame 5001 {
            n493 = Two Button Dialog(message="Unable to connect to imaging computer, do you want to run data aquisiton alone? ", 1:"No" ("F button name (\"Cancel\")"), 2:"Yes" ("T button name (\"OK\")")) -> (T button?=w1070:bool)
            n494 = case shown="False" w1070 {
              tunnel: ["Macro: Exit" "" ("Empty String Constant")] -> w1069
              frame False {
              }
              frame True {
              }
            }
          }
        }
        n495 = call <vilib>:"Add State(s) to Queue__JKI_lib_State_Machine.vi"("State(s) in Front (\"\")"=w1052, "State(s) in (\"\")"=w1058) -> ("States Out"=w1057:string)  [unwired: 13 in]
      }
      frame "Exit" {
        # "Do not put any code in this frame.\n(No errors that occur here will be handled.)"
        n496 = call <vilib>:"Add State(s) to Queue__JKI_lib_State_Machine.vi"("State(s) in (\"\")"=w1081) -> ("States Out"=w1080:string)  [unwired: 14 in]
      }
      frame "---------- Case ----------" {
        # "Template Separator\n(You can make a copy of, or modify, this frame)"
        n497 = call <vilib>:"Add State(s) to Queue__JKI_lib_State_Machine.vi"("State(s) in (\"\")"=w1086) -> ("States Out"=w1085:string)  [unwired: 14 in]
      }
      frame "Case: getCaliID" {
        # "Get Calibration file #\n(You can make a copy of, or modify, this frame)"
        n498 = Unbundle By Name(w1087) -> ("Pathes.CaliPath"=w1090:path)
        n499 = call <vilib>:"Recursive File List.vi"("pattern"="*.tdms", "Treat LLBs as Folders?"=FALSE, "Folder Path"=w1090) -> ("All Files in Dir"=w1095:path[])  [unwired: 4 in, 4 out]
        n500 = for {
          tunnel: w1095 -> [w1105] mode=indexing
          tunnel: [w1104] -> w1094 mode=indexing
          tunnel: "Calibration" -> [w1101]
          n501 = Strip Path(path=w1105) -> (name=w1102:string)  [unwired: 1 out]
          n502 = Search and Replace String(input string=w1102, search string=w1101) -> (result string=w1100:string)  [unwired: 6 in, 3 out]
          n503 = Scan From String(format string="%d" ("string"), input string=w1100) -> (output 1=w1104:i32)  [unwired: 3 in, 3 out]
        }
        n504 = Array Max & Min(array=w1094) -> (max value=w1093:i32)  [unwired: 3 out]
        n505 = Bundle By Name(cluster=w1087, "IDs.Cali ID"=w1093) -> (w1088:T23)
        n506 = call <vilib>:"Add State(s) to Queue__JKI_lib_State_Machine.vi"("State(s) in (\"\")"=w1099) -> ("States Out"=w1098:string)  [unwired: 14 in]
      }
      frame "Case: getBGID" {
        # "Get background #\n(You can make a copy of, or modify, this frame)"
        n507 = Unbundle By Name(w1108) -> ("Pathes.BG Path"=w1113:path)
        n508 = call <vilib>:"Recursive File List.vi"("pattern"="*.tdms", "Treat LLBs as Folders?"=FALSE, "Folder Path"=w1113) -> ("All Files in Dir"=w1111:path[])  [unwired: 4 in, 4 out]
        n509 = for {
          tunnel: w1111 -> [w1128] mode=indexing
          tunnel: "Background" ("name or relative path") -> [w1126]
          shift-right: [w1119] -> w1106
          shift-left: 0 -> [w1123]
          n510 = Strip Path(path=w1128) -> (name=w1127:string)  [unwired: 1 out]
          n511 = Search and Replace String(input string=w1127, search string=w1126) -> (number of replacements=w1125:i32)  [unwired: 6 in, 3 out]
          n512 = Greater Than 0?(x=w1125) -> (x > 0?=w1124:bool)
          n513 = Select(t=1, s=w1124, f=0) -> (s? t:f=w1122:i32)
          n514 = Add(x=w1122, y=w1123) -> (x+y=w1119:i32)
        }
        n515 = Bundle By Name(cluster=w1108, "IDs.BG ID"=w1106) -> (w1109:T23)
        n516 = call <vilib>:"Add State(s) to Queue__JKI_lib_State_Machine.vi"("State(s) in (\"\")"=w1118) -> ("States Out"=w1117:string)  [unwired: 14 in]
      }
      frame "Case: getRunID" {
        # "Check folder for run ID\n(You can make a copy of, or modify, this frame)"
        n517 = Unbundle By Name(w1138) -> ("Pathes.DataPath"=w1137:path, "CaseID"=w1133:string)
        n518 = Build Array("Background" ("name or relative path"), "Calibration", "3DScanData" ("element")) -> (w1143:string[])
        n519 = call <vilib>:"Recursive File List.vi"("Folders to Exclude"=w1143, "pattern"="*.tdms", "Treat LLBs as Folders?"=FALSE, "Folder Path"=w1137) -> ("All Files in Dir"=w1134:path[])  [unwired: 3 in, 4 out]
        n520 = for {
          tunnel: w1134 -> [w1152] mode=indexing
          tunnel: [w1151] -> w1140 mode=indexing
          tunnel: w1133 -> [w1148]
          n521 = Strip Path(path=w1152) -> (name=w1149:string)  [unwired: 1 out]
          n522 = Search and Replace String(input string=w1149, search string=w1148) -> (result string=w1147:string)  [unwired: 6 in, 3 out]
          n523 = Scan From String(format string="_%d" ("string"), input string=w1147) -> (output 1=w1151:i32)  [unwired: 3 in, 3 out]
        }
        n524 = Array Max & Min(array=w1140) -> (max value=w1131:i32)  [unwired: 3 out]
        n525 = Bundle By Name(cluster=w1138, "IDs.RunID"=w1131) -> (w1139:T23)
        n526 = call "RunIDFGV.vi"("Error In"=w1129, "RunID in"=w1131) -> ("Error Out"=w1130:errorcluster)  [unwired: 8 in, 1 out]
        n527 = call <vilib>:"Add State(s) to Queue__JKI_lib_State_Machine.vi"("State(s) in (\"\")"=w1146) -> ("States Out"=w1145:string)  [unwired: 14 in]
      }
      frame "Case: CreatFileStruct" {
        # "Creat case file structure"
        n528 = Unbundle By Name(w1166) -> ("DefaultPath"=w1172:path, "CaseID"=w1159:string)
        n529 = Build Path(base path=w1172, name or relative path=w1159) -> (appended path=w1171:path)
        n530 = call <vilib>:"Check if File or Folder Exists.vi"("error in (no error)"=w1165, "path"=w1171) -> ("error out"=w1168:errorcluster, "file or folder exists?"=w1170:bool, "dup path"=w1169:path)  [unwired: 7 in]
        n531 = case shown="True" w1170 {
          tunnel: w1169 -> [w1189 w1197]
          tunnel: w1168 -> [w1187 w1192]
          tunnel: [w1181 w1197] -> w1157
          tunnel: [w1185 w1199] -> w1156
          tunnel: [u32 0 u32 0] -> w1155
          tunnel: [w1183 w1202] -> w1163
          tunnel: "Background" ("name or relative path") -> [w1182 w1194]
          tunnel: "Calibration" -> [w1180 w1193]
          tunnel: [w1176 w1195] -> w1160
          tunnel: w1159 -> [_ _]
          tunnel: ["" ("Empty String Constant") "Case: getRunID\nCase: getBGID\nCase: getCaliID\nUI: Update"] -> w1158
          frame False {
            # "Folder not exist. Creat folders."
            n532 = Create Folder(path (use dialog)=w1189, error in=w1187) -> (created path=w1181:path, error out=w1178:errorcluster)  [unwired: 1 in, 1 out]
            n533 = Build Path(base path=w1181, name or relative path=w1180) -> (appended path=w1179:path)
            n534 = Build Path(base path=w1181, name or relative path=w1182) -> (appended path=w1188:path)
            n535 = Create Folder(path (use dialog)=w1188, error in=w1178) -> (created path=w1183:path, error out=w1184:errorcluster)  [unwired: 1 in, 1 out]
            n536 = Create Folder(path (use dialog)=w1179, error in=w1178) -> (created path=w1176:path, error out=w1177:errorcluster)  [unwired: 1 in, 1 out]
            n537 = Merge Errors(w1184, w1177) -> (w1185:errorcluster)
          }
          frame True {
            # "Folder exsit, check file #"
            n538 = Build Path(base path=w1197, name or relative path=w1193) -> (appended path=w1198:path)
            n539 = Build Path(base path=w1197, name or relative path=w1194) -> (appended path=w1203:path)
            n540 = call <vilib>:"Check if File or Folder Exists.vi"("path"=w1198) -> ("file or folder exists?"=w1196:bool, "dup path"=w1195:path)  [unwired: 8 in, 1 out]
            n541 = call <vilib>:"Check if File or Folder Exists.vi"("path"=w1203) -> ("file or folder exists?"=w1201:bool, "dup path"=w1202:path)  [unwired: 8 in, 1 out]
            n542 = And(x=w1201, y=w1196) -> (x .and. y?=w1200:bool)
            n543 = case shown="False" w1200 {
              tunnel: w1192 -> [_ w1205]
              tunnel: [errorcluster {"status"=TRUE, "code"=5003, "source"="File structure error."} ("error out") w1205] -> w1199
              frame False {
              }
              frame True {
              }
            }
          }
        }
        n544 = Bundle By Name(cluster=w1166, "Pathes.DataPath"=w1157, "Pathes.BG Path"=w1163, "Pathes.CaliPath"=w1160, "IDs.RunID"=w1155, "IDs.BG ID"=w1155, "IDs.Cali ID"=w1155) -> (w1167:T23)
        n545 = call "DataRootPathFGV.vi"("Error In"=w1156, "PathIn"=w1157) -> ("Error Out"=w1154:errorcluster)  [unwired: 8 in, 1 out]
        n546 = call "RunIDFGV.vi"("Error In"=w1154, "RunID in"=w1155) -> ("Error Out"=w1153:errorcluster)  [unwired: 8 in, 1 out]
        n547 = call <vilib>:"Add State(s) to Queue__JKI_lib_State_Machine.vi"("State(s) in Front (\"\")"=w1158, "State(s) in (\"\")"=w1174) -> ("States Out"=w1173:string)  [unwired: 13 in]
      }
      frame "Case: GetID" {
        # "Template Separator\n(You can make a copy of, or modify, this frame)"
        n548 = call "set_subjectID.vi"() -> ("subject_id"=w1206:string)  [unwired: 10 in]
        n549 = Bundle By Name(cluster=w1208, "CaseID"=w1206) -> (w1209:T23)
        n550 = call <vilib>:"Add State(s) to Queue__JKI_lib_State_Machine.vi"("State(s) in (\"\")"=w1212) -> ("States Out"=w1211:string)  [unwired: 14 in]
      }
      frame "---------- DeconEngine ----------" {
        # "start data aquisition and then set irfAligh to ture and decon channel to 1,2 and 3."
        # "Template Separator\n(You can make a copy of, or modify, this frame)"
        n551 = call <vilib>:"Add State(s) to Queue__JKI_lib_State_Machine.vi"("State(s) in (\"\")"=w1217) -> ("States Out"=w1216:string)  [unwired: 14 in]
      }
      frame "DeconEngine: InitilizeMacro" {
        # "start data aquisition and then set irfAligh to ture and decon channel to 1,2 and 3."
        # "Initilize Decon Engine for all channel\n(You can make a copy of, or modify, this frame)"
        n552 = call <vilib>:"Add State(s) to Queue__JKI_lib_State_Machine.vi"("State(s) in Front (\"\")"="DeconEngine: InitializeCh1\nDeconEngine: InitializeCh2\nDeconEngine: InitializeCh3\nDeconEngine: InitializeCh4" ("State(s) in Front (\"\")"), "State(s) in (\"\")"=w1223) -> ("States Out"=w1222:string)  [unwired: 13 in]
      }
      frame "DeconEngine: InitializeCh1" {
        w1247 = refnum<class "LaguerreDeconEngineClass.lvclass"> refnum  # Ch1DeconObj
        # "Initilize Laguerre Deconvolution engine Object\n(You can make a copy of, or modify, this frame)"
        n553 = call "FLImDAQ_FGV.vi"("error in (no error)"=w1232) -> ("error out"=w1243:errorcluster, "Read data"=w1242:T6)  [unwired: 9 in]
        n554 = global read "GlobalVariables.vi" "LastUseiRF"() -> (w1225:T15)
        n555 = Unbundle By Name(w1242) -> ("min record length"=w1241:i32)
        n556 = call "setLaguerreOrder.vi"("error in (no error)"=w1243, "LaguerreOrder"=u32 12, "LaguerreDeconClass in"=w1247) -> ("error out"=w1244:errorcluster, "LaguerreDeconClass out"=w1245:refnum<class "LaguerreDeconEngineClass.lvclass">)  [unwired: 7 in]
        n557 = Unbundle By Name(w1225) -> ("Ch1 iRF"=w1224:dbl[])
        n558 = call "setDataLength.vi"("error in (no error)"=w1244, "dataLength"=w1241, "LaguerreDeconClass in"=w1245) -> ("error out"=w1240:errorcluster, "LaguerreDeconClass out"=w1239:refnum<class "LaguerreDeconEngineClass.lvclass">)  [unwired: 7 in]
        n559 = call "setIRF.vi"("error in (no error)"=w1240, "iRF"=w1224, "LaguerreDeconClass in"=w1239) -> ("error out"=w1237:errorcluster, "LaguerreDeconClass out"=w1238:refnum<class "LaguerreDeconEngineClass.lvclass">)  [unwired: 7 in]
        n560 = call "computeAlpha.vi"("error in (no error)"=w1237, "LaguerreDeconClass in"=w1238) -> ("error out"=w1235:errorcluster, "LaguerreDeconClass out"=w1236:refnum<class "LaguerreDeconEngineClass.lvclass">)  [unwired: 8 in]
        n561 = call "dataInitilize.vi"("error in (no error)"=w1235, "LaguerreDeconClass in"=w1236) -> ("error out"=w1233:errorcluster, "LaguerreDeconClass out"=w1234:refnum<class "LaguerreDeconEngineClass.lvclass">)  [unwired: 8 in]
        n562 = call "computeDeconMatrix.vi"("error in (no error)"=w1233, "LaguerreDeconClass in"=w1234) -> ("error out"=w1229:errorcluster, "LaguerreDeconClass out"=w1231:refnum<class "LaguerreDeconEngineClass.lvclass">)  [unwired: 8 in]
        n563 = call "Ch1DeconEngineFGV.vi"("Error In"=w1229, "action(read)"=enum16{"write", "read"}."write" ("action"), "Ch1DeconEngine in"=w1231) -> ("Error Out"=w1228:errorcluster)  [unwired: 7 in, 1 out]
        n564 = call <vilib>:"Add State(s) to Queue__JKI_lib_State_Machine.vi"("State(s) in (\"\")"=w1249) -> ("States Out"=w1248:string)  [unwired: 14 in]
      }
      frame "DeconEngine: InitializeCh2" {
        w1273 = refnum<class "LaguerreDeconEngineClass.lvclass"> refnum  # Ch2DeconObj
        # "Initilize Laguerre Deconvolution engine Object\n(You can make a copy of, or modify, this frame)"
        n565 = global read "GlobalVariables.vi" "LastUseiRF"() -> (w1251:T15)
        n566 = call "FLImDAQ_FGV.vi"("error in (no error)"=w1259) -> ("error out"=w1252:errorcluster, "Read data"=w1269:T6)  [unwired: 9 in]
        n567 = call "setLaguerreOrder.vi"("error in (no error)"=w1252, "LaguerreOrder"=u32 12, "LaguerreDeconClass in"=w1273) -> ("error out"=w1270:errorcluster, "LaguerreDeconClass out"=w1271:refnum<class "LaguerreDeconEngineClass.lvclass">)  [unwired: 7 in]
        n568 = Unbundle By Name(w1269) -> ("min record length"=w1268:i32)
        n569 = Unbundle By Name(w1251) -> ("Ch2 iRF"=w1250:dbl[])
        n570 = call "setDataLength.vi"("error in (no error)"=w1270, "dataLength"=w1268, "LaguerreDeconClass in"=w1271) -> ("error out"=w1267:errorcluster, "LaguerreDeconClass out"=w1266:refnum<class "LaguerreDeconEngineClass.lvclass">)  [unwired: 7 in]
        n571 = call "setIRF.vi"("error in (no error)"=w1267, "iRF"=w1250, "LaguerreDeconClass in"=w1266) -> ("error out"=w1264:errorcluster, "LaguerreDeconClass out"=w1265:refnum<class "LaguerreDeconEngineClass.lvclass">)  [unwired: 7 in]
        n572 = call "computeAlpha.vi"("error in (no error)"=w1264, "LaguerreDeconClass in"=w1265) -> ("error out"=w1262:errorcluster, "LaguerreDeconClass out"=w1263:refnum<class "LaguerreDeconEngineClass.lvclass">)  [unwired: 8 in]
        n573 = call "dataInitilize.vi"("error in (no error)"=w1262, "LaguerreDeconClass in"=w1263) -> ("error out"=w1260:errorcluster, "LaguerreDeconClass out"=w1261:refnum<class "LaguerreDeconEngineClass.lvclass">)  [unwired: 8 in]
        n574 = call "computeDeconMatrix.vi"("error in (no error)"=w1260, "LaguerreDeconClass in"=w1261) -> ("error out"=w1256:errorcluster, "LaguerreDeconClass out"=w1258:refnum<class "LaguerreDeconEngineClass.lvclass">)  [unwired: 8 in]
        n575 = call "Ch2DeconEngineFGV.vi"("Error In"=w1256, "action(read)"=enum16{"write", "read"}."write" ("action"), "Ch2DeconEngine in"=w1258) -> ("Error Out"=w1255:errorcluster)  [unwired: 7 in, 1 out]
        n576 = call <vilib>:"Add State(s) to Queue__JKI_lib_State_Machine.vi"("State(s) in (\"\")"=w1275) -> ("States Out"=w1274:string)  [unwired: 14 in]
      }
      frame "DeconEngine: InitializeCh3" {
        w1276 = refnum<class "LaguerreDeconEngineClass.lvclass"> refnum  # Ch3DeconObj
        # "Initilize Laguerre Deconvolution engine Object\n(You can make a copy of, or modify, this frame)"
        n577 = call "FLImDAQ_FGV.vi"("error in (no error)"=w1285) -> ("error out"=w1296:errorcluster, "Read data"=w1295:T6)  [unwired: 9 in]
        n578 = global read "GlobalVariables.vi" "LastUseiRF"() -> (w1278:T15)
        n579 = call "setLaguerreOrder.vi"("error in (no error)"=w1296, "LaguerreOrder"=u32 12, "LaguerreDeconClass in"=w1276) -> ("error out"=w1297:errorcluster, "LaguerreDeconClass out"=w1298:refnum<class "LaguerreDeconEngineClass.lvclass">)  [unwired: 7 in]
        n580 = Unbundle By Name(w1295) -> ("min record length"=w1294:i32)
        n581 = Unbundle By Name(w1278) -> ("Ch3 iRF"=w1277:dbl[])
        n582 = call "setDataLength.vi"("error in (no error)"=w1297, "dataLength"=w1294, "LaguerreDeconClass in"=w1298) -> ("error out"=w1293:errorcluster, "LaguerreDeconClass out"=w1292:refnum<class "LaguerreDeconEngineClass.lvclass">)  [unwired: 7 in]
        n583 = call "setIRF.vi"("error in (no error)"=w1293, "iRF"=w1277, "LaguerreDeconClass in"=w1292) -> ("error out"=w1290:errorcluster, "LaguerreDeconClass out"=w1291:refnum<class "LaguerreDeconEngineClass.lvclass">)  [unwired: 7 in]
        n584 = call "computeAlpha.vi"("error in (no error)"=w1290, "LaguerreDeconClass in"=w1291) -> ("error out"=w1288:errorcluster, "LaguerreDeconClass out"=w1289:refnum<class "LaguerreDeconEngineClass.lvclass">)  [unwired: 8 in]
        n585 = call "dataInitilize.vi"("error in (no error)"=w1288, "LaguerreDeconClass in"=w1289) -> ("error out"=w1286:errorcluster, "LaguerreDeconClass out"=w1287:refnum<class "LaguerreDeconEngineClass.lvclass">)  [unwired: 8 in]
        n586 = call "computeDeconMatrix.vi"("error in (no error)"=w1286, "LaguerreDeconClass in"=w1287) -> ("error out"=w1282:errorcluster, "LaguerreDeconClass out"=w1284:refnum<class "LaguerreDeconEngineClass.lvclass">)  [unwired: 8 in]
        n587 = call "Ch3DeconEngineFGV.vi"("Error In"=w1282, "action(read)"=enum16{"write", "read"}."write" ("action"), "Ch3DeconEngine in"=w1284) -> ("Error Out"=w1281:errorcluster)  [unwired: 7 in, 1 out]
        n588 = call <vilib>:"Add State(s) to Queue__JKI_lib_State_Machine.vi"("State(s) in (\"\")"=w1301) -> ("States Out"=w1300:string)  [unwired: 14 in]
      }
      frame "DeconEngine: InitializeCh4" {
        w1302 = refnum<class "LaguerreDeconEngineClass.lvclass"> refnum  # Ch3DeconObj
        # "Initilize Laguerre Deconvolution engine Object\n(You can make a copy of, or modify, this frame)"
        n589 = call "FLImDAQ_FGV.vi"("error in (no error)"=w1311) -> ("error out"=w1322:errorcluster, "Read data"=w1321:T6)  [unwired: 9 in]
        n590 = global read "GlobalVariables.vi" "LastUseiRF"() -> (w1304:T15)
        n591 = call "setLaguerreOrder.vi"("error in (no error)"=w1322, "LaguerreOrder"=u32 12, "LaguerreDeconClass in"=w1302) -> ("error out"=w1323:errorcluster, "LaguerreDeconClass out"=w1324:refnum<class "LaguerreDeconEngineClass.lvclass">)  [unwired: 7 in]
        n592 = Unbundle By Name(w1321) -> ("min record length"=w1320:i32)
        n593 = Unbundle By Name(w1304) -> ("Ch3 iRF"=w1303:dbl[])
        n594 = call "setDataLength.vi"("error in (no error)"=w1323, "dataLength"=w1320, "LaguerreDeconClass in"=w1324) -> ("error out"=w1319:errorcluster, "LaguerreDeconClass out"=w1318:refnum<class "LaguerreDeconEngineClass.lvclass">)  [unwired: 7 in]
        n595 = call "setIRF.vi"("error in (no error)"=w1319, "iRF"=w1303, "LaguerreDeconClass in"=w1318) -> ("error out"=w1316:errorcluster, "LaguerreDeconClass out"=w1317:refnum<class "LaguerreDeconEngineClass.lvclass">)  [unwired: 7 in]
        n596 = call "computeAlpha.vi"("error in (no error)"=w1316, "LaguerreDeconClass in"=w1317) -> ("error out"=w1314:errorcluster, "LaguerreDeconClass out"=w1315:refnum<class "LaguerreDeconEngineClass.lvclass">)  [unwired: 8 in]
        n597 = call "dataInitilize.vi"("error in (no error)"=w1314, "LaguerreDeconClass in"=w1315) -> ("error out"=w1312:errorcluster, "LaguerreDeconClass out"=w1313:refnum<class "LaguerreDeconEngineClass.lvclass">)  [unwired: 8 in]
        n598 = call "computeDeconMatrix.vi"("error in (no error)"=w1312, "LaguerreDeconClass in"=w1313) -> ("error out"=w1308:errorcluster, "LaguerreDeconClass out"=w1310:refnum<class "LaguerreDeconEngineClass.lvclass">)  [unwired: 8 in]
        n599 = call "Ch3DeconEngineFGV.vi"("Error In"=w1308, "action(read)"=enum16{"write", "read"}."write" ("action"), "Ch3DeconEngine in"=w1310) -> ("Error Out"=w1307:errorcluster)  [unwired: 7 in, 1 out]
        n600 = call <vilib>:"Add State(s) to Queue__JKI_lib_State_Machine.vi"("State(s) in (\"\")"=w1327) -> ("States Out"=w1326:string)  [unwired: 14 in]
      }
      frame "---------- Digitizer ----------" {
        # "Template Separator\n(You can make a copy of, or modify, this frame)"
        n601 = call <vilib>:"Add State(s) to Queue__JKI_lib_State_Machine.vi"("State(s) in (\"\")"=w1332) -> ("States Out"=w1331:string)  [unwired: 14 in]
      }
      frame "Digitizer: Initialize" {
        # "reset digitizer to everytime the system runs"
        # "reset digitizer to everytime the system runs"
        # "Initialize digitizer.\nInitialize both digitizer and update status."
        n602 = call "FLImDAQ_FGV.vi"("error in (no error)"=w1340) -> ("error out"=w1334:errorcluster, "Read data"=w1339:T6)  [unwired: 9 in]
        n603 = Unbundle By Name(w1342) -> ("SysConfigCluster.Ch1Enable?"=w1347:bool, "SysConfigCluster.Ch2Enable?"=w1346:bool, "SysConfigCluster.Ch3Enable?"=w1344:bool)
        n604 = Unbundle By Name(w1339) -> ("Digitizer 1"=w1335:refnum<k15>, "Digitizer 2"=w1338:refnum<k15>)
        n605 = property on="Digitizer" class="Bool (strict)"("Blinking"=TRUE) -> ()  [unwired: 2 in, 2 out]
        n606 = Or(x=w1347, y=w1346) -> (x .or. y?=w1345:bool)
        n607 = case shown="True" w1345 {
          tunnel: w1334 -> [w1355 w1358]
          tunnel: [w1355 w1357] -> w1336
          tunnel: w1335 -> [_ w1359]
          frame False {
          }
          frame True {
            n608 = call <instrlib>:"niScope Initialize.vi"("resource name"=w1359, "reset device"=TRUE, "error in"=w1358) -> ("error out"=w1357:errorcluster)  [unwired: 11 in, 1 out]
          }
        }
        n609 = case shown="True" w1344 {
          tunnel: w1334 -> [w1350 w1352]
          tunnel: [w1350 w1354] -> w1341
          tunnel: w1338 -> [_ w1353]
          frame False {
          }
          frame True {
            n610 = call <instrlib>:"niScope Initialize.vi"("resource name"=w1353, "reset device"=TRUE, "error in"=w1352) -> ("error out"=w1354:errorcluster)  [unwired: 11 in, 1 out]
          }
        }
        n611 = Merge Errors(w1336, w1341) -> (w1333:errorcluster)
        n612 = call <vilib>:"Add State(s) to Queue__JKI_lib_State_Machine.vi"("State(s) in (\"\")"=w1349) -> ("States Out"=w1348:string)  [unwired: 14 in]
      }
      frame "Digitizer: Config" {
        # "Synchronize is taking time ~3s."
        # "Config  digitizer\nCall subVi to config digitizer"
        n613 = call "FLImDAQ_FGV.vi"() -> ("Read data"=w1377:T6)  [unwired: 10 in, 1 out]
        n614 = Unbundle By Name(w1386) -> ("SysConfigCluster.Ch1Enable?"=w1394:bool, "SysConfigCluster.Ch2Enable?"=w1393:bool, "SysConfigCluster.Ch3Enable?"=w1391:bool, "FLImDAQ"=w1388:T30)
        n615 = Unbundle By Name(w1377) -> ("Digitizer 1"=w1380:refnum<k15>, "Digitizer 2"=w1379:refnum<k15>)
        n616 = property on="Digitizer" class="Bool (strict)"(error in=w1381, "Blinking"=TRUE) -> (error out=w1382:errorcluster)  [unwired: 1 in, 1 out]
        n617 = Or(x=w1394, y=w1393) -> (x .or. y?=w1392:bool)
        n618 = case shown="True" w1392 {
          tunnel: w1388 -> [_ w1407]
          tunnel: w1382 -> [w1403 w1406]
          tunnel: [w1403 w1405] -> w1389
          tunnel: w1380 -> [_ w1404]
          frame False {
          }
          frame True {
            n619 = call "DigitizerConfig.vi"("error in (no error)"=w1406, "FLImDAQ"=w1407, "IVI Refnum in"=w1404) -> ("error out"=w1405:errorcluster)  [unwired: 7 in, 1 out]
          }
        }
        n620 = case shown="True" w1391 {
          tunnel: w1388 -> [_ w1402]
          tunnel: w1389 -> [w1397 w1401]
          tunnel: [w1397 w1400] -> w1365
          tunnel: w1379 -> [_ w1398]
          frame False {
          }
          frame True {
            n621 = call "DigitizerConfig.vi"("Config Trigger? (T)"=FALSE ("Config Trigge(T)r:"), "error in (no error)"=w1401, "FLImDAQ"=w1402, "IVI Refnum in"=w1398) -> ("error out"=w1400:errorcluster)  [unwired: 6 in, 1 out]
          }
        }
        n622 = call "Digitizer1_FGV.vi"("error in (no error)"=w1365) -> ("error out"=w1375:errorcluster, "Read data"=w1376:refnum<k15>)  [unwired: 9 in]
        n623 = call <instrlib>:"niScope Get Session Reference.vi"("instrument handle"=w1376, "error in"=w1375) -> ("session reference"=w1369:refnum<k20>, "error out"=w1367:errorcluster)  [unwired: 11 in, 1 out]
        n624 = call "Digitizer2_FGV.vi"("error in (no error)"=w1367) -> ("error out"=w1373:errorcluster, "Read data"=w1374:refnum<k15>)  [unwired: 9 in]
        n625 = call <instrlib>:"niScope Get Session Reference.vi"("instrument handle"=w1374, "error in"=w1373) -> ("session reference"=w1368:refnum<k20>, "error out"=w1366:errorcluster)  [unwired: 11 in, 1 out]
        n626 = Build Array(w1369, w1368) -> (w1372:refnum<k20>[])
        n627 = call <instrlib>:"niTClk Configure For Homogeneous Triggers.vi"("error in (no error)"=w1366, "sessions"=w1372) -> ("error out"=w1371:errorcluster, "sessions out"=w1370:refnum<k20>[])  [unwired: 8 in]
        n628 = call <instrlib>:"niTClk Synchronize.vi"("error in (no error)"=w1371, "sessions"=w1370) -> ("error out"=w1364:errorcluster, "sessions out"=w1362:refnum<k20>[])  [unwired: 8 in]
        n629 = call <userlib>:"Wait (ms)__ogtk.vi"("error in (no error)"=w1364, "milliseconds to wait"=u32 1500) -> ("error out"=w1360:errorcluster)  [unwired: 8 in, 1 out]
        n630 = Unbundle By Name(w1360) -> ("status"=w1385:bool)
        n631 = Not(x=w1385) -> (.not. x?=w1384:bool)
        n632 = Bundle By Name(cluster=w1386, "System Status.Digitizer"=w1384, "niTClk sessions"=w1362) -> (w1387:T23)
        n633 = property on="Digitizer" class="Bool (strict)"(error in=w1360, "Blinking"=FALSE) -> (error out=w1378:errorcluster)  [unwired: 1 in, 1 out]
        n634 = call <vilib>:"Add State(s) to Queue__JKI_lib_State_Machine.vi"("State(s) in (\"\")"=w1396) -> ("States Out"=w1395:string)  [unwired: 14 in]
      }
      frame "Digitizer: Start" {
        # "send trigger to start acquisition loop"
        # "initilize aquisition"
        # "Start Digitizer\n(TClk start)"
        n635 = Unbundle By Name(w1415) -> ("niTClk sessions"=w1414:refnum<k20>[])
        n636 = call <instrlib>:"niTClk Initiate.vi"("error in (no error)"=w1408, "sessions"=w1414) -> ("error out"=w1410:errorcluster)  [unwired: 8 in, 1 out]
        n637 = Generate User Event(priority (normal)=usereventprio."high priority", user event=w1411, event data cluster=TRUE ("event data"), error in=w1410) -> (error out=w1409:errorcluster)  [unwired: 1 out]
        n638 = call <vilib>:"Add State(s) to Queue__JKI_lib_State_Machine.vi"("State(s) in (\"\")"=w1418) -> ("States Out"=w1417:string)  [unwired: 14 in]
      }
      frame "Digitizer: Abort" {
        # "Template Separator\n(You can make a copy of, or modify, this frame)"
        n639 = call "Digitizer1_FGV.vi"("error in (no error)"=w1422, "Operation (Read)"=enum16{"Write", "Read"}."Read" ("Operation")) -> ("error out"=w1429:errorcluster, "Read data"=w1426:refnum<k15>)  [unwired: 8 in]
        n640 = call "Digitizer2_FGV.vi"("error in (no error)"=w1422, "Operation (Read)"=enum16{"Write", "Read"}."Read" ("Operation")) -> ("error out"=w1425:errorcluster, "Read data"=w1427:refnum<k15>)  [unwired: 8 in]
        n641 = Bundle By Name(cluster=w1419, "SysRunning?"=FALSE ("System Status")) -> (w1420:T23)
        n642 = call <instrlib>:"niScope Abort.vi"("instrument handle"=w1426, "error in"=w1429) -> ("error out"=w1431:errorcluster)  [unwired: 12 in, 1 out]
        n643 = call <instrlib>:"niScope Abort.vi"("instrument handle"=w1427, "error in"=w1425) -> ("error out"=w1430:errorcluster)  [unwired: 12 in, 1 out]
        n644 = Merge Errors(w1431, w1430) -> (w1423:errorcluster)
        n645 = call <vilib>:"Add State(s) to Queue__JKI_lib_State_Machine.vi"("State(s) in (\"\")"=w1434) -> ("States Out"=w1433:string)  [unwired: 14 in]
      }
      frame "Digitizer: checkTemp" {
        w1437 = 65.0 ("y")
        w1442 = enum16{"Write", "Read"}."Read" ("Operation")
        # "Template Separator\n(You can make a copy of, or modify, this frame)"
        n646 = call "Digitizer1_FGV.vi"("Operation (Read)"=w1442) -> ("error out"=w1443:errorcluster, "Read data"=w1444:refnum<k15>)  [unwired: 9 in]
        n647 = call "Digitizer2_FGV.vi"("Operation (Read)"=w1442) -> ("error out"=w1440:errorcluster, "Read data"=w1441:refnum<k15>)  [unwired: 9 in]
        n648 = property on="Property Node" class="niScope"(reference=w1441, error in=w1440) -> ("Device Temperature"=w1438:dbl)  [unwired: 2 out]
        "Dig2 Temp" <- w1438
        n649 = property on="Property Node" class="niScope"(reference=w1444, error in=w1443) -> ("Device Temperature"=w1439:dbl)  [unwired: 2 out]
        "Dig1 Temp" <- w1439
        n650 = Greater?(x=w1439, y=w1437) -> (0:w1436:bool)
        n651 = Greater?(x=w1438, y=w1437) -> (0:w1435:bool)
        n652 = case shown="True" w1436 {
          frame False {
          }
          frame True {
            n653 = One Button Dialog(message="Digitizer 1 over heating!", button name ("OK")="OK") -> ()  [unwired: 1 out]
          }
        }
        n654 = case shown="True" w1435 {
          frame False {
          }
          frame True {
            n655 = One Button Dialog(message="Digitizer 2 over heating!", button name ("OK")="OK") -> ()  [unwired: 1 out]
          }
        }
        n656 = call <vilib>:"Add State(s) to Queue__JKI_lib_State_Machine.vi"("State(s) in (\"\")"=w1449) -> ("States Out"=w1448:string)  [unwired: 14 in]
      }
      frame "Digitizer: Close" {
        # "Close Digitizer"
        n657 = call "Digitizer1_FGV.vi"("error in (no error)"=w1459, "Operation (Read)"=enum16{"Write", "Read"}."Read" ("Operation")) -> ("error out"=w1461:errorcluster, "Read data"=w1465:refnum<k15>)  [unwired: 8 in]
        n658 = call "Digitizer2_FGV.vi"("error in (no error)"=w1459, "Operation (Read)"=enum16{"Write", "Read"}."Read" ("Operation")) -> ("error out"=w1460:errorcluster, "Read data"=w1463:refnum<k15>)  [unwired: 8 in]
        n659 = call <instrlib>:"niScope Close.vi"("instrument handle"=w1465, "error in"=w1461) -> ("error out"=w1458:errorcluster)  [unwired: 13 in]
        n660 = call <instrlib>:"niScope Close.vi"("instrument handle"=w1463, "error in"=w1460) -> ("error out"=w1457:errorcluster)  [unwired: 13 in]
        n661 = Merge Errors(w1458, w1457) -> (w1456:errorcluster)
        n662 = Unbundle By Name(w1456) -> ("status"=w1455:bool)
        n663 = Bundle By Name(cluster=w1466, "System Status.Digitizer"=w1455) -> (w1467:T23)
        n664 = call <vilib>:"Add State(s) to Queue__JKI_lib_State_Machine.vi"("State(s) in (\"\")"=w1469) -> ("States Out"=w1468:string)  [unwired: 14 in]
      }
      frame "---------- LabJack ----------" {
        # "Template Separator\n(You can make a copy of, or modify, this frame)"
        n665 = call <vilib>:"Add State(s) to Queue__JKI_lib_State_Machine.vi"("State(s) in (\"\")"=w1474) -> ("States Out"=w1473:string)  [unwired: 14 in]
      }
      frame "LabJack: checkPedal" {
        # "Template Separator\n(You can make a copy of, or modify, this frame)"
        n666 = Unbundle By Name(w1475) -> ("LJ Pinout.Foot Pedal"=w1479:string)
        n667 = call "LabJack_FGV.vi"("Operation(Read)"=enum16{"Write", "Read"}."Read" ("Operation"), "error in (no error)"=w1477) -> ("error out"=w1481:errorcluster, "Read data"=w1482:i32)  [unwired: 8 in]
        n668 = call "LJM_eReadName.vi"("Handle In"=w1482, "Name"=w1479, "error in"=w1481) -> ("Value"=w1480:dbl, "error out"=w1478:errorcluster)  [unwired: 10 in, 1 out]
        n669 = case shown="1" w1480 {
          tunnel: w1475 -> [w1487 w1490]
          tunnel: [w1487 w1488] -> w1476
          frame 0, Default {
          }
          frame 1 {
            # "If Pedal pressed"
            n670 = Tick Count (ms)() -> (millisecond timer value=w1494:u32)
            n671 = Unbundle By Name(w1490) -> ("Last Trigger"=w1489:u32)
            n672 = Subtract(x=w1494, y=w1489) -> (x-y=w1493:u32)
            n673 = Greater Or Equal?(x=w1493, y=u32 2000) -> (x >= y?=w1491:bool)
            n674 = case shown="True" w1491 {
              tunnel: w1490 -> [w1495 w1496]
              tunnel: w1489 -> [_ _]
              tunnel: [w1495 w1497] -> w1488
              frame False {
              }
              frame True {
                n675 = Tick Count (ms)() -> (millisecond timer value=w1498:u32)
                n676 = Unbundle By Name(w1496) -> ("SysRunning?"=w1499:bool)
                n677 = case shown="False" w1499 {
                  frame False {
                    n678 = property on="StartButton" class="Bool (strict)"("Val(Sgnl)"=TRUE ("Value (Signaling)")) -> ()  [unwired: 2 in, 2 out]
                  }
                  frame True {
                    n679 = property on="StopButton" class="Bool (strict)"("Val(Sgnl)"=TRUE ("Value (Signaling)")) -> ()  [unwired: 2 in, 2 out]
                  }
                }
                n680 = Bundle By Name(cluster=w1496, "Last Trigger"=w1498) -> (w1497:T23)
              }
            }
          }
        }
        n681 = call <vilib>:"Add State(s) to Queue__JKI_lib_State_Machine.vi"("State(s) in (\"\")"=w1486) -> ("States Out"=w1485:string)  [unwired: 14 in]
      }
      frame "LabJack: ZeroV" {
        # "Just Zero V\nDO not update FGV and front panel\nWIll resume from last V"
        # "set bias to 0"
        # "Zero APD bias\n(You can make a copy of, or modify, this frame)"
        n682 = Unbundle By Name(w1504) -> ("LJ Pinout.Ch1 Bias"=w1509:string, "LJ Pinout.Ch2 Bias"=w1508:string, "LJ Pinout.Ch3 Bias"=w1507:string)
        n683 = Build Array(w1509, w1508, w1507) -> (w1506:string[])
        n684 = call "LabJack_FGV.vi"("Operation(Read)"=enum16{"Write", "Read"}."Read" ("Operation"), "error in (no error)"=w1503) -> ("error out"=w1510:errorcluster, "Read data"=w1511:i32)  [unwired: 8 in]
        n685 = call "LJM_eWriteNames.vi"("Handle In"=w1511, "aNames"=w1506, "aValuesIn"=dbl[] [0.0, 0.0, 0.0], "error in"=w1510) -> ("error out"=w1502:errorcluster)  [unwired: 9 in, 2 out]
        n686 = call <vilib>:"Add State(s) to Queue__JKI_lib_State_Machine.vi"("State(s) in (\"\")"=w1515) -> ("States Out"=w1514:string)  [unwired: 14 in]
      }
      frame "LabJack: SetV" {
        w1522 = enum16{"write", "read"}."read" ("action (write)")
        # "set bias to user specifid"
        # "Set APD bias\n(You can make a copy of, or modify, this frame)"
        n687 = Unbundle By Name(w1531) -> ("LJ Pinout.Ch1 Bias"=w1535:string, "LJ Pinout.Ch2 Bias"=w1534:string, "LJ Pinout.Ch3 Bias"=w1533:string, "LJ Pinout.Ch4 Bias"=w1525:string)
        n688 = call "V2FGV.vi"("Error In"=w1521, "action(write)"=w1522) -> ("Error Out"=w1519:errorcluster, "V2 out"=w1527:dbl)  [unwired: 8 in]
        n689 = call "V4FGV.vi"("Error In"=w1521, "action(write)"=w1522) -> ("Error Out"=w1517:errorcluster, "V3 out"=w1523:dbl)  [unwired: 8 in]
        n690 = call "V1FGV.vi"("Error In"=w1521, "action (write)"=w1522) -> ("Error Out"=w1520:errorcluster, "V1 out"=w1524:dbl)  [unwired: 8 in]
        n691 = call "V3FGV.vi"("Error In"=w1521, "action(write)"=w1522) -> ("Error Out"=w1518:errorcluster, "V3 out"=w1526:dbl)  [unwired: 8 in]
        n692 = local write "V 3"(w1526) -> ()
        n693 = local write "V 2"(w1527) -> ()
        n694 = local write "V 4"(w1523) -> ()
        n695 = local write "V 1"(w1524) -> ()
        n696 = Build Array(w1535, w1534, w1533, w1525) -> (w1532:string[])
        n697 = call "LabJack_FGV.vi"("Operation(Read)"=enum16{"Write", "Read"}."Read" ("Operation"), "error in (no error)"=w1521) -> ("error out"=w1536:errorcluster, "Read data"=w1537:i32)  [unwired: 8 in]
        n698 = Build Array(w1524, w1527, w1526, w1523) -> (w1528:dbl[])
        n699 = call "LJM_eWriteNames.vi"("Handle In"=w1537, "aNames"=w1532, "aValuesIn"=w1528, "error in"=w1536) -> ("error out"=w1529:errorcluster)  [unwired: 9 in, 2 out]
        n700 = Merge Errors(w1520, w1519, w1518, w1517) -> (w1516:errorcluster)
        n701 = call <vilib>:"Add State(s) to Queue__JKI_lib_State_Machine.vi"("State(s) in (\"\")"=w1541) -> ("States Out"=w1540:string)  [unwired: 14 in]
        n702 = Merge Errors(w1516, w1529) -> (w1530:errorcluster)
      }
      frame "LabJack: Open" {
        # "Initialize LabJack T7\nEstablish connection and initialize pins"
        n703 = call "LJ_Open.vi"("error in"=w1551, "DeviceType"="LJM_dtT7") -> ("error out"=w1548:errorcluster, "Success?"=w1549:bool, "Handle Out"=w1543:i32)  [unwired: 7 in]
        n704 = call "LabJack_FGV.vi"("Operation(Read)"=enum16{"Write", "Read"}."Write" ("Operation"), "error in (no error)"=w1548, "Write data"=w1543) -> ("error out"=w1545:errorcluster)  [unwired: 7 in, 1 out]
        n705 = Bundle By Name(cluster=w1546, "System Status.Labjack"=w1549) -> (w1550:T23)
        n706 = call <vilib>:"Add State(s) to Queue__JKI_lib_State_Machine.vi"("State(s) in (\"\")"=w1553) -> ("States Out"=w1552:string)  [unwired: 14 in]
      }
      frame "LabJack: SetDefaultSub" {
        w1563 = enum16{"write", "read"}."write" ("action")
        w1564 = 0.0 ("V1 in")
        w1577 = "_EF_ENABLE" ("string")
        # "1. Disable PWM\n2. Set all V to 0\n3. Set 355 relay to open\n4. Set LED to off"
        # "read once to set DIO to input"
        # "set all initila V to 0. Set footpedal to input. Set PWM to low. Set laser relay to open. Set LEDs to yellow."
        # "Set Labjack to correct input and output state and initial values"
        n707 = disable-structure shown="Disabled" {
          frame Disabled {
            (unwired) dbl[] [0.0, 0.0, 0.0, 0.0, 0.0, 0.0, 0.0, 0.0, 0.0] ("aValuesIn")
          }
          frame Enabled {
          }
        }
        n708 = Unbundle By Name(w1574) -> ("LJ Pinout.355 PWM"=w1579:string, "LJ Pinout.AimingBeam PWM"=w1578:string, "LJ Pinout.Ch1 Bias"=w1584:string, "LJ Pinout.Ch2 Bias"=w1554:string, "LJ Pinout.Ch3 Bias"=w1588:string, "LJ Pinout.Ch4 Bias"=w1568:string, "LJ Pinout.Laser Start/Stop"=w1587:string, "LJ Pinout.Red LED"=w1586:string, "LJ Pinout.Green LED"=w1585:string)
        n709 = call "V1FGV.vi"("Error In"=w1572, "action (write)"=w1563, "V1 in"=w1564) -> ("Error Out"=w1567:errorcluster, "V1 out"=w1571:dbl)  [unwired: 7 in]
        n710 = local write "V 1"(w1571) -> ()
        n711 = call "V2FGV.vi"("Error In"=w1567, "action(write)"=w1563, "V2 in"=w1564) -> ("Error Out"=w1566:errorcluster, "V2 out"=w1570:dbl)  [unwired: 7 in]
        n712 = call "LabJack_FGV.vi"("Operation(Read)"=enum16{"Write", "Read"}."Read" ("Operation"), "error in (no error)"=w1572) -> ("error out"=w1560:errorcluster, "Read data"=w1582:i32)  [unwired: 8 in]
        n713 = Concatenate Strings(w1579, w1577) -> (w1576:string)
        n714 = Concatenate Strings(w1578, w1577) -> (w1575:string)
        n715 = local write "V 2"(w1570) -> ()
        n716 = call "V3FGV.vi"("Error In"=w1566, "action(write)"=w1563, "V3 in"=w1564) -> ("Error Out"=w1565:errorcluster, "V3 out"=w1569:dbl)  [unwired: 7 in]
        n717 = Build Array(w1576, w1575, w1584, w1554, w1588, w1568, w1587, w1586, w1585) -> (w1558:string[])
        n718 = local write "V 3"(w1569) -> ()
        n719 = call "V4FGV.vi"("Error In"=w1565, "action(write)"=w1563, "V3 in"=w1564) -> ("Error Out"=w1561:errorcluster, "V3 out"=w1562:dbl)  [unwired: 7 in]
        n720 = Array Size(array=w1558) -> (size(s)=w1557:i32)
        n721 = local write "V 4"(w1562) -> ()
        n722 = Initialize Array(0.0 ("element"), w1557) -> (w1555:dbl[])
        n723 = Unbundle By Name(w1574) -> ("LJ Pinout.Foot Pedal"=w1573:string)
        n724 = call "LJM_eWriteNames.vi"("Handle In"=w1582, "aNames"=w1558, "aValuesIn"=w1555, "error in"=w1560) -> ("Handle Out"=w1581:i32, "error out"=w1580:errorcluster)  [unwired: 9 in, 1 out]
        n725 = call "LJM_eReadName.vi"("Handle In"=w1581, "Name"=w1573, "error in"=w1580) -> ("error out"=w1559:errorcluster)  [unwired: 10 in, 2 out]
        n726 = case shown="Error .." w1559 {
          frame No Error {
            # "no error"
          }
          frame Error {
            # "handle error"
            n727 = One Button Dialog(message="Labjack error! The pin assignment is likely wrong. Please check pin setting of Labjack. Program will terminate.", button name ("OK")="OK") -> ()  [unwired: 1 out]
          }
        }
        n728 = call <vilib>:"Add State(s) to Queue__JKI_lib_State_Machine.vi"("State(s) in (\"\")"=w1591) -> ("States Out"=w1590:string)  [unwired: 14 in]
      }
      frame "LabJack: FootPedalConfig" {
        # "Setup footPedal\n(You can make a copy of, or modify, this frame)"
        n729 = call "LabJack_FGV.vi"("Operation(Read)"=enum16{"Write", "Read"}."Read" ("Operation"), "error in (no error)"=w1595) -> ("error out"=w1599:errorcluster, "Read data"=w1600:i32)  [unwired: 8 in]
        n730 = call "LJM_eWriteName.vi"("Handle In"=w1600, "Name"="DIO15", "Value"=1.0, "error in"=w1599) -> ("error out"=w1596:errorcluster)  [unwired: 10 in, 1 out]
        n731 = call <vilib>:"Add State(s) to Queue__JKI_lib_State_Machine.vi"("State(s) in (\"\")"=w1604) -> ("States Out"=w1603:string)  [unwired: 14 in]
      }
      frame "LabJack: SetDefaultAndClose" {
        # "Template Separator\n(You can make a copy of, or modify, this frame)"
        n732 = call <vilib>:"Add State(s) to Queue__JKI_lib_State_Machine.vi"("State(s) in Front (\"\")"="LabJack: SetDefaultSub\nLabJack: Close" ("State(s) in Front (\"\")"), "State(s) in (\"\")"=w1610) -> ("States Out"=w1609:string)  [unwired: 13 in]
      }
      frame "LabJack: Close" {
        # "Close LabJack Refnum"
        n733 = call "LabJack_FGV.vi"("Operation(Read)"=enum16{"Write", "Read"}."Read" ("Operation"), "error in (no error)"=w1616) -> ("error out"=w1611:errorcluster, "Read data"=w1612:i32)  [unwired: 8 in]
        n734 = Bundle By Name(cluster=w1614, "System Status.Labjack"=FALSE ("System Status.Gain Control")) -> (w1617:T23)
        n735 = call "LJM_Close.vi"("error in"=w1611, "Handle"=w1612) -> ("error out"=w1619:errorcluster)  [unwired: 9 in]
        n736 = call <vilib>:"Add State(s) to Queue__JKI_lib_State_Machine.vi"("State(s) in (\"\")"=w1621) -> ("States Out"=w1620:string)  [unwired: 14 in]
      }
      frame "LabJack: Interlock enable/disable" {
        w1630 = i8 0  # int8
        # "[Covers: REQ8]"
        # "Interlock enable/disable\n(Usage: \"LabJack: Interlock enable/disable >> 1|0\")"
        n737 = Fract/Exp String To Number(string=w1631, default (0 dbl)=w1630) -> (number=w1627:i8)  [unwired: 2 in, 1 out]
        n738 = Unbundle By Name(w1629) -> ("LJ Pinout.Interlock"=w1628:string)
        n739 = call "LabJack_FGV.vi"("Operation(Read)"=enum16{"Write", "Read"}."Read" ("Operation")) -> ("Read data"=w1625:i32)  [unwired: 9 in, 1 out]
        n740 = call "LJM_eWriteName.vi"("Handle In"=w1625, "Name"=w1628, "Value"=w1627, "error in"=w1626) -> ("error out"=w1623:errorcluster)  [unwired: 10 in, 1 out]
        n741 = call <vilib>:"Add State(s) to Queue__JKI_lib_State_Machine.vi"("State(s) in (\"\")"=w1633) -> ("States Out"=w1632:string)  [unwired: 14 in]
      }
      frame "LabJack: 355_PWM_Config" {
        w1635 = 0.0 ("element")
        w1655 = "DIO_EF_CLOCK1_ENABLE"
        # "Config PWM frequency"
        n742 = Unbundle By Name(w1647) -> ("LJ Pinout.355 PWM"=w1654:string)
        n743 = Unbundle By Name(w1647) -> ("355 PWM setting.DIO_EF_CLOCK1_DIVISOR"=w1646:i16, "355 PWM setting.DIO_EF_CLOCK1_ROLL_VALUE"=w1645:i32, "355 PWM setting.DIO#_EF_INDEX"=w1642:i16, "355 PWM setting.DIO#_EF_OPTIONS"=w1641:i16, "355 PWM setting.DIO#_EF_CONFIG_A"=w1640:i32)
        n744 = Concatenate Strings(w1654, "_EF_ENABLE" ("string")) -> (w1650:string)
        n745 = Concatenate Strings(w1654, "_EF_INDEX") -> (w1653:string)
        n746 = Concatenate Strings(w1654, "_EF_OPTIONS") -> (w1652:string)
        n747 = Concatenate Strings(w1654, "_EF_CONFIG_A") -> (w1651:string)
        n748 = call "LabJack_FGV.vi"("Operation(Read)"=enum16{"Write", "Read"}."Read" ("Operation")) -> ("Read data"=w1648:i32)  [unwired: 9 in, 1 out]
        n749 = Build Array(w1635, w1635, w1646, w1645, 1.0 ("element"), 0.0 ("element"), w1642, w1641, w1640) -> (w1639:dbl[])
        n750 = Build Array("DIO_EF_CLOCK0_ENABLE", w1655, "DIO_EF_CLOCK1_DIVISOR", "DIO_EF_CLOCK1_ROLL_VALUE", w1655, w1650, w1653, w1652, w1651) -> (w1649:string[])
        n751 = call "LJM_eWriteNames.vi"("Handle In"=w1648, "aNames"=w1649, "aValuesIn"=w1639, "error in"=w1637) -> ("error out"=w1638:errorcluster)  [unwired: 9 in, 2 out]
        n752 = call <vilib>:"Add State(s) to Queue__JKI_lib_State_Machine.vi"("State(s) in (\"\")"=w1664) -> ("States Out"=w1663:string)  [unwired: 14 in]
      }
      frame "LabJack: 355_PWM_Start" {
        # "Template Separator\n(You can make a copy of, or modify, this frame)"
        n753 = Unbundle By Name(w1672) -> ("LJ Pinout.355 PWM"=w1671:string)
        n754 = call "LabJack_FGV.vi"("Operation(Read)"=enum16{"Write", "Read"}."Read" ("Operation"), "error in (no error)"=w1666) -> ("error out"=w1673:errorcluster, "Read data"=w1674:i32)  [unwired: 8 in]
        n755 = Concatenate Strings(w1671, "_EF_ENABLE" ("string")) -> (w1669:string)
        n756 = call "LJM_eWriteName.vi"("Handle In"=w1674, "Name"=w1669, "Value"=1.0, "error in"=w1673) -> ("error out"=w1667:errorcluster)  [unwired: 10 in, 1 out]
        n757 = call <vilib>:"Add State(s) to Queue__JKI_lib_State_Machine.vi"("State(s) in (\"\")"=w1677) -> ("States Out"=w1676:string)  [unwired: 14 in]
      }
      frame "LabJack: 355_PWM_Stop" {
        # "Template Separator\n(You can make a copy of, or modify, this frame)"
        n758 = Unbundle By Name(w1683) -> ("LJ Pinout.355 PWM"=w1687:string)
        n759 = call "LabJack_FGV.vi"("Operation(Read)"=enum16{"Write", "Read"}."Read" ("Operation"), "error in (no error)"=w1682) -> ("error out"=w1688:errorcluster, "Read data"=w1680:i32)  [unwired: 8 in]
        n760 = Concatenate Strings(w1687, "_EF_ENABLE" ("string")) -> (w1685:string)
        n761 = call "LJM_eWriteName.vi"("Handle In"=w1680, "Name"=w1685, "Value"=0.0, "error in"=w1688) -> ("error out"=w1679:errorcluster)  [unwired: 10 in, 1 out]
        n762 = local write "355nm Laser toggle"(FALSE ("355nm Laser toggle")) -> ()
        n763 = call <vilib>:"Add State(s) to Queue__JKI_lib_State_Machine.vi"("State(s) in (\"\")"=w1691) -> ("States Out"=w1690:string)  [unwired: 14 in]
      }
      frame "LabJack: AB_Start" {
        # "Aiming Beam Start\n(Based on aimging beam frequency, set LabJack pin)"
        n764 = Unbundle By Name(w1701) -> ("AB Cluster.Freq"=w1693:i32, "LJ Pinout.AimingBeam PWM"=w1700:string)
        n765 = Greater Than 0?(x=w1693) -> (x > 0?=w1692:bool)
        n766 = case shown="False" w1692 {
          tunnel: w1700 -> [w1707 w1710]
          tunnel: [w1707 w1708] -> w1699
          frame False {
            # "if 0 freq, set PWM pin"
          }
          frame True {
            # "if non zero freq, set PWM enable"
            n767 = Concatenate Strings(w1710, "_EF_ENABLE" ("string")) -> (w1708:string)
          }
        }
        n768 = call "LabJack_FGV.vi"("Operation(Read)"=enum16{"Write", "Read"}."Read" ("Operation"), "error in (no error)"=w1696) -> ("error out"=w1702:errorcluster, "Read data"=w1703:i32)  [unwired: 8 in]
        n769 = call "LJM_eWriteName.vi"("Handle In"=w1703, "Name"=w1699, "Value"=1.0, "error in"=w1702) -> ("error out"=w1697:errorcluster)  [unwired: 10 in, 1 out]
        n770 = local write "Aiming beam toggle"(TRUE ("Aiming beam toggle")) -> ()
        n771 = call <vilib>:"Add State(s) to Queue__JKI_lib_State_Machine.vi"("State(s) in (\"\")"=w1706) -> ("States Out"=w1705:string)  [unwired: 14 in]
      }
      frame "LabJack: AB_Stop" {
        # "Aiming Beam Stop\n(Based on aiming beam frequency, set LabJack pin low)"
        n772 = Unbundle By Name(w1718) -> ("AB Cluster.Freq"=w1713:i32, "LJ Pinout.AimingBeam PWM"=w1720:string)
        n773 = Greater Than 0?(x=w1713) -> (x > 0?=w1712:bool)
        n774 = case shown="False" w1712 {
          tunnel: w1720 -> [w1726 w1729]
          tunnel: [w1726 w1727] -> w1711
          frame False {
          }
          frame True {
            n775 = Concatenate Strings(w1729, "_EF_ENABLE" ("string")) -> (w1727:string)
          }
        }
        n776 = call "LabJack_FGV.vi"("Operation(Read)"=enum16{"Write", "Read"}."Read" ("Operation"), "error in (no error)"=w1716) -> ("error out"=w1721:errorcluster, "Read data"=w1722:i32)  [unwired: 8 in]
        n777 = call "LJM_eWriteName.vi"("Handle In"=w1722, "Name"=w1711, "Value"=0.0, "error in"=w1721) -> ("error out"=w1717:errorcluster)  [unwired: 10 in, 1 out]
        n778 = local write "Aiming beam toggle"(FALSE ("Aiming beam toggle")) -> ()
        n779 = call <vilib>:"Add State(s) to Queue__JKI_lib_State_Machine.vi"("State(s) in (\"\")"=w1725) -> ("States Out"=w1724:string)  [unwired: 14 in]
      }
      frame "LabJack: AB_PWM_Config" {
        w1731 = 0.0 ("element")
        w1751 = "DIO_EF_CLOCK2_ENABLE"
        # "Config PWM frequency"
        n780 = Unbundle By Name(w1743) -> ("LJ Pinout.AimingBeam PWM"=w1750:string)
        n781 = Unbundle By Name(w1743) -> ("AB PWM setting.DIO_EF_CLOCK1_DIVISOR"=w1742:i16, "AB PWM setting.DIO_EF_CLOCK1_ROLL_VALUE"=w1741:i32, "AB PWM setting.DIO#_EF_INDEX"=w1738:i16, "AB PWM setting.DIO#_EF_OPTIONS"=w1737:i16, "AB PWM setting.DIO#_EF_CONFIG_A"=w1736:i32)
        n782 = Concatenate Strings(w1750, "_EF_ENABLE" ("string")) -> (w1746:string)
        n783 = Concatenate Strings(w1750, "_EF_INDEX") -> (w1749:string)
        n784 = Concatenate Strings(w1750, "_EF_OPTIONS") -> (w1748:string)
        n785 = Concatenate Strings(w1750, "_EF_CONFIG_A") -> (w1747:string)
        n786 = call "LabJack_FGV.vi"("Operation(Read)"=enum16{"Write", "Read"}."Read" ("Operation")) -> ("Read data"=w1744:i32)  [unwired: 9 in, 1 out]
        n787 = Build Array(w1731, w1731, w1742, w1741, 1.0 ("element"), 0.0 ("element"), w1738, w1737, w1736) -> (w1735:dbl[])
        n788 = Build Array("DIO_EF_CLOCK0_ENABLE", w1751, "DIO_EF_CLOCK2_DIVISOR", "DIO_EF_CLOCK2_ROLL_VALUE", w1751, w1746, w1749, w1748, w1747) -> (w1745:string[])
        n789 = call "LJM_eWriteNames.vi"("Handle In"=w1744, "aNames"=w1745, "aValuesIn"=w1735, "error in"=w1733) -> ("error out"=w1734:errorcluster)  [unwired: 9 in, 2 out]
        n790 = call <vilib>:"Add State(s) to Queue__JKI_lib_State_Machine.vi"("State(s) in (\"\")"=w1760) -> ("States Out"=w1759:string)  [unwired: 14 in]
      }
      frame "---------- LED ----------" {
        # "Template Separator\n(You can make a copy of, or modify, this frame)"
        n791 = call <vilib>:"Add State(s) to Queue__JKI_lib_State_Machine.vi"("State(s) in (\"\")"=w1765) -> ("States Out"=w1764:string)  [unwired: 14 in]
      }
      frame "LED: OpenVIRef" {
        # "Template Separator\n(You can make a copy of, or modify, this frame)"
        n792 = call <vilib>:"Application Directory.vi"() -> ("Application Directory"=w1772:path)
        n793 = Build Path(base path=w1772, name or relative path="SubVI") -> (appended path=w1770:path)
        n794 = Build Path(base path=w1770, name or relative path="LEDBreath.vi") -> (appended path=w1768:path)
        n795 = Open VI Reference(vi path=w1768, error in (no error)=w1773) -> (vi reference=w1774:refnum<vi>, error out=w1767:errorcluster)  [unwired: 4 in]
        n796 = case shown="Error .." w1767 {
          tunnel: [TRUE FALSE] -> w1766
          frame No Error {
          }
          frame Error {
          }
        }
        n797 = Bundle By Name(cluster=w1775, "LED vi reference"=w1774, "LED vi ref open?"=w1766) -> (w1776:T23)
        n798 = call <vilib>:"Add State(s) to Queue__JKI_lib_State_Machine.vi"("State(s) in (\"\")"=w1779) -> ("States Out"=w1778:string)  [unwired: 14 in]
      }
      frame "LED: CloseVIRef" {
        # "Template Separator\n(You can make a copy of, or modify, this frame)"
        n799 = Unbundle By Name(w1783) -> ("LED vi reference"=w1784:refnum<vi>, "LED vi ref open?"=w1782:bool)
        n800 = case shown="True" w1782 {
          tunnel: w1786 -> [w1790 w1793]
          tunnel: [w1790 w1792] -> w1785
          tunnel: w1784 -> [_ w1791]
          frame False {
          }
          frame True {
            n801 = Close Reference(reference=w1791, error in (no error)=w1793) -> (error out=w1792:errorcluster)
          }
        }
        n802 = call <vilib>:"Add State(s) to Queue__JKI_lib_State_Machine.vi"("State(s) in (\"\")"=w1789) -> ("States Out"=w1788:string)  [unwired: 14 in]
      }
      frame "LED: BreathGreen" {
        w1794 = FALSE ("Wait Until Done")
        # "Breath system LED\n(LED: Breath >> True/False)"
        n803 = Unbundle By Name(w1802) -> ("LED vi reference"=w1801:refnum<vi>)
        n804 = invoke class="VI" method="Ctrl Val.Set"(reference=w1801, error in=w1799, "Control Name"="Color", "Value"=0) -> (reference out=w1798:refnum<vi>, error out=w1797:errorcluster)  [unwired: 1 in, 3 out]
        n805 = invoke on="Invoke Node" class="VI" method="Run VI"(reference=w1798, error in=w1797, "Wait until done"=w1794, "Auto Dispose Ref"=w1794) -> (error out=w1800:errorcluster)  [unwired: 1 in, 4 out]
        n806 = call <vilib>:"Add State(s) to Queue__JKI_lib_State_Machine.vi"("State(s) in (\"\")"=w1805) -> ("States Out"=w1804:string)  [unwired: 14 in]
      }
      frame "LED: BreathOrange" {
        w1806 = FALSE ("Wait Until Done")
        # "Breath system LED\n(LED: Breath >> True/False)"
        n807 = Unbundle By Name(w1814) -> ("LED vi reference"=w1813:refnum<vi>)
        n808 = invoke class="VI" method="Ctrl Val.Set"(reference=w1813, error in=w1811, "Control Name"="Color", "Value"=1) -> (reference out=w1810:refnum<vi>, error out=w1809:errorcluster)  [unwired: 1 in, 3 out]
        n809 = invoke on="Invoke Node" class="VI" method="Run VI"(reference=w1810, error in=w1809, "Wait until done"=w1806, "Auto Dispose Ref"=w1806) -> (error out=w1812:errorcluster)  [unwired: 1 in, 4 out]
        n810 = call <vilib>:"Add State(s) to Queue__JKI_lib_State_Machine.vi"("State(s) in (\"\")"=w1817) -> ("States Out"=w1816:string)  [unwired: 14 in]
      }
      frame "LED: BreathOff" {
        # "System LED Breath Off\n(Breath off, check VI status to make sure it is off)"
        n811 = Unbundle By Name(w1826) -> ("LED vi reference"=w1825:refnum<vi>)
        n812 = invoke on="Invoke Node" class="VI" method="Ctrl Val.Set"(reference=w1825, error in=w1823, "Control Name"="Stop", "Value"=TRUE) -> (reference out=w1818:refnum<vi>, error out=w1819:errorcluster)  [unwired: 1 in, 3 out]
        n813 = case shown="No Error" w1819 {
          selector: w1819 -> [w1831 _]
          tunnel: [w1830 errorcluster {"status"=FALSE, "code"=0, "source"=""} ("error IO")] -> w1824
          tunnel: ["" ("State(s) in Front (\"\")") "LED: BreathOff" ("State(s) in Front (\"\")")] -> w1822
          tunnel: w1818 -> [w1832 _]
          frame No Error {
            # "No error, wait for VI to stop"
            n814 = while {
              tunnel: w1832 -> [w1840]
              shift-right: [w1834] -> w1830
              shift-left: w1831 -> [w1839]
              stop <- w1836 stop-if-true
              # "continue check whether vi is running"
              n815 = property class="VI"(reference=w1840, error in=w1839) -> (error out=w1834:errorcluster, "Exec.State"=w1838:T20)  [unwired: 1 out]
              n816 = Wait (ms)(milliseconds to wait=u32 50) -> ()  [unwired: 1 out]
              n817 = Equal?(x=w1838, y=T20."Idle") -> (x = y?=w1836:bool)
            }
          }
          frame Error {
            # "try again when error"
          }
        }
        n818 = call <vilib>:"Add State(s) to Queue__JKI_lib_State_Machine.vi"("State(s) in Front (\"\")"=w1822, "State(s) in (\"\")"=w1829) -> ("States Out"=w1828:string)  [unwired: 13 in]
      }
      frame "LED: Off" {
        # "set LED to red"
        # "Template Separator\n(You can make a copy of, or modify, this frame)"
        n819 = Unbundle By Name(w1845) -> ("LJ Pinout.Red LED"=w1844:string, "LJ Pinout.Green LED"=w1843:string)
        n820 = call "LabJack_FGV.vi"("Operation(Read)"=enum16{"Write", "Read"}."Read" ("Operation"), "error in (no error)"=w1846) -> ("error out"=w1853:errorcluster, "Read data"=w1852:i32)  [unwired: 8 in]
        n821 = call "LJM_eWriteName.vi"("Handle In"=w1852, "Name"=w1844, "Value"=0.0, "error in"=w1853) -> ("Handle Out"=w1850:i32, "error out"=w1849:errorcluster)  [unwired: 10 in]
        n822 = call "LJM_eWriteName.vi"("Handle In"=w1850, "Name"=w1843, "Value"=0.0, "error in"=w1849) -> ("error out"=w1847:errorcluster)  [unwired: 10 in, 1 out]
        n823 = call <vilib>:"Add State(s) to Queue__JKI_lib_State_Machine.vi"("State(s) in (\"\")"=w1857) -> ("States Out"=w1856:string)  [unwired: 14 in]
      }
      frame "LED: Green" {
        # "set LED to green"
        # "Template Separator\n(You can make a copy of, or modify, this frame)"
        n824 = Unbundle By Name(w1861) -> ("LJ Pinout.Red LED"=w1859:string, "LJ Pinout.Green LED"=w1860:string)
        n825 = call "LabJack_FGV.vi"("Operation(Read)"=enum16{"Write", "Read"}."Read" ("Operation"), "error in (no error)"=w1863) -> ("error out"=w1869:errorcluster, "Read data"=w1868:i32)  [unwired: 8 in]
        n826 = call "LJM_eWriteName.vi"("Handle In"=w1868, "Name"=w1859, "Value"=0.0, "error in"=w1869) -> ("Handle Out"=w1866:i32, "error out"=w1865:errorcluster)  [unwired: 10 in]
        n827 = call "LJM_eWriteName.vi"("Handle In"=w1866, "Name"=w1860, "Value"=9.0, "error in"=w1865) -> ("error out"=w1862:errorcluster)  [unwired: 10 in, 1 out]
        n828 = call <vilib>:"Add State(s) to Queue__JKI_lib_State_Machine.vi"("State(s) in (\"\")"=w1872) -> ("States Out"=w1871:string)  [unwired: 14 in]
      }
      frame "---------- Queue ----------" {
        # "Template Separator\n(You can make a copy of, or modify, this frame)"
        n829 = call <vilib>:"Add State(s) to Queue__JKI_lib_State_Machine.vi"("State(s) in (\"\")"=w1877) -> ("States Out"=w1876:string)  [unwired: 14 in]
      }
      frame "Queue: Flash" {
        # "Clear queue contnet\n(clear queue content by flash it)"
        n830 = Flush Queue(queue=w1883, error in (no error)=w1882) -> (error out=w1881:errorcluster)  [unwired: 2 out]
        n831 = Flush Queue(queue=w1884, error in (no error)=w1881) -> (error out=w1879:errorcluster)  [unwired: 2 out]
        n832 = Flush Queue(queue=w1880, error in (no error)=w1879) -> (error out=w1878:errorcluster)  [unwired: 2 out]
        n833 = call <vilib>:"Add State(s) to Queue__JKI_lib_State_Machine.vi"("State(s) in (\"\")"=w1888) -> ("States Out"=w1887:string)  [unwired: 14 in]
      }
      frame "Queue: Destory" {
        # "Destory Data Queue\nDistory data queue ref so the aquisition loop stop"
        n834 = Release Queue(queue=w1894, error in (no error)=w1890) -> (error out=w1897:errorcluster)  [unwired: 1 in, 2 out]
        n835 = Release Queue(queue=w1893, error in (no error)=w1890) -> (error out=w1896:errorcluster)  [unwired: 1 in, 2 out]
        n836 = Release Queue(queue=w1891, error in (no error)=w1890) -> (error out=w1889:errorcluster)  [unwired: 1 in, 2 out]
        n837 = Merge Errors(w1897, w1896, w1889) -> (w1895:errorcluster)
        n838 = call <vilib>:"Simple Error Handler.vi"("error in (no error)"=w1895) -> ()  [unwired: 4 in, 5 out]
        n839 = call <vilib>:"Add State(s) to Queue__JKI_lib_State_Machine.vi"("State(s) in (\"\")"=w1900) -> ("States Out"=w1899:string)  [unwired: 14 in]
      }
      frame "---------- Run ----------" {
        # "Template Separator\n(You can make a copy of, or modify, this frame)"
        n840 = call <vilib>:"Add State(s) to Queue__JKI_lib_State_Machine.vi"("State(s) in (\"\")"=w1905) -> ("States Out"=w1904:string)  [unwired: 14 in]
      }
      frame "Run: CaliIncrement" {
        # "Increment Calibration #\n(You can make a copy of, or modify, this frame)"
        n841 = Unbundle By Name(w1907) -> ("IDs.Cali ID"=w1909:i8)
        n842 = Increment(x=w1909) -> (x+1=w1906:i8)
        n843 = Bundle By Name(cluster=w1907, "IDs.Cali ID"=w1906) -> (w1908:T23)
        n844 = call <vilib>:"Add State(s) to Queue__JKI_lib_State_Machine.vi"("State(s) in (\"\")"=w1913) -> ("States Out"=w1912:string)  [unwired: 14 in]
      }
      frame "Run: BGIncrement" {
        # "Increment BG #\n(You can make a copy of, or modify, this frame)"
        n845 = Unbundle By Name(w1914) -> ("IDs.BG ID"=w1917:i8)
        n846 = Increment(x=w1917) -> (x+1=w1916:i8)
        n847 = Bundle By Name(cluster=w1914, "IDs.BG ID"=w1916) -> (w1915:T23)
        n848 = call <vilib>:"Add State(s) to Queue__JKI_lib_State_Machine.vi"("State(s) in (\"\")"=w1921) -> ("States Out"=w1920:string)  [unwired: 14 in]
      }
      frame "Run: Increment" {
        # "Increase Run# by 1"
        n849 = Unbundle By Name(w1926) -> ("IDs.RunID"=w1928:i8)
        n850 = Increment(x=w1928) -> (x+1=w1924:i8)
        n851 = Bundle By Name(cluster=w1926, "IDs.RunID"=w1924) -> (w1927:T23)
        n852 = call "RunIDFGV.vi"("Error In"=w1922, "RunID in"=w1924) -> ("Error Out"=w1923:errorcluster)  [unwired: 8 in, 1 out]
        n853 = call <vilib>:"Add State(s) to Queue__JKI_lib_State_Machine.vi"("State(s) in (\"\")"=w1930) -> ("States Out"=w1929:string)  [unwired: 14 in]
      }
      frame "Run: Decrement" {
        # "Increase Run# by 1"
        n854 = Unbundle By Name(w1935) -> ("IDs.RunID"=w1937:i8)
        n855 = Decrement(x=w1937) -> (x-1=w1933:i8)
        n856 = Bundle By Name(cluster=w1935, "IDs.RunID"=w1933) -> (w1936:T23)
        n857 = call "RunIDFGV.vi"("Error In"=w1931, "RunID in"=w1933) -> ("Error Out"=w1932:errorcluster)  [unwired: 8 in, 1 out]
        n858 = call <vilib>:"Add State(s) to Queue__JKI_lib_State_Machine.vi"("State(s) in (\"\")"=w1939) -> ("States Out"=w1938:string)  [unwired: 14 in]
      }
      frame "---------- SysConfig ----------" {
        # "Template Separator\n(You can make a copy of, or modify, this frame)"
        n859 = call <vilib>:"Add State(s) to Queue__JKI_lib_State_Machine.vi"("State(s) in (\"\")"=w1944) -> ("States Out"=w1943:string)  [unwired: 14 in]
      }
      frame "SysConfig: LoadAPDSerialNumber" {
        # "Template Separator\n(You can make a copy of, or modify, this frame)"
        n860 = call "readAPDSerial.vi"("Error In"=w1946) -> ("Error Out"=w1945:errorcluster, "output cluster"=w1947:T26)  [unwired: 9 in]
        n861 = Bundle By Name(cluster=w1948, "APDSerialNum"=w1947) -> (w1949:T23)
        n862 = call <vilib>:"Add State(s) to Queue__JKI_lib_State_Machine.vi"("State(s) in (\"\")"=w1952) -> ("States Out"=w1951:string)  [unwired: 14 in]
      }
      frame "SysConfig: Load Sys Config" {
        # "[Covers: REQ5]"
        # "Load System config"
        # "Load system configuration\n(Load both hardware and DAQ config)"
        n863 = call "LoadSysConfig.vi"("Error In"=w1955, "Enum"=enum16{"LastUse", "Default"}."LastUse") -> ("Error Out"=w1954:errorcluster, "SysConfigCluster"=w1957:T4)  [unwired: 8 in]
        "SysConfigCluster" <- w1957
        n864 = Bundle By Name(cluster=w1958, "SysConfigCluster"=w1957) -> (w1959:T23)
        n865 = call <vilib>:"Add State(s) to Queue__JKI_lib_State_Machine.vi"("State(s) in (\"\")"=w1961) -> ("States Out"=w1960:string)  [unwired: 14 in]
      }
      frame "SysConfig: Load Digitizer Setting" {
        w1962 = enum16{"Write", "Read"}."Write" ("Operation")
        # "Load DAQ config\nSave to FGV"
        # "Template Separator\n(You can make a copy of, or modify, this frame)"
        n866 = call <userlib>:"Current VIs Parent Directory__ogtk.vi"() -> ("Parent Directory (+ Relative)"=w1976:path)  [unwired: 5 in]
        n867 = Build Path(base path=w1976, name or relative path="SubVI\\DigitizerConfiguration\\V6_Scope_last_use.config") -> (appended path=w1977:path)
        n868 = call "ReadDigitizerConfig(SubVI).vi"("error in (no error)"=w1974, "appended path"=w1977) -> ("error out"=w1970:errorcluster, "FLImDAQ"=w1968:T6)  [unwired: 8 in]
        n869 = call "FLImDAQ_FGV.vi"("error in (no error)"=w1970, "Operation (Read)"=w1962, "Write data"=w1968) -> ("error out"=w1972:errorcluster)  [unwired: 7 in, 1 out]
        n870 = Unbundle By Name(w1968) -> ("min record length"=→"data length":i32, "Digitizer 1"=w1964:refnum<k15>, "Digitizer 2"=w1971:refnum<k15>)
        n871 = Bundle By Name(cluster=w1966, "FLImDAQ"=w1968) -> (w1967:T23)
        n872 = call "Digitizer1_FGV.vi"("error in (no error)"=w1972, "Operation (Read)"=w1962, "Write data"=w1964) -> ("error out"=w1973:errorcluster)  [unwired: 7 in, 1 out]
        n873 = call "Digitizer2_FGV.vi"("error in (no error)"=w1973, "Operation (Read)"=w1962, "Write data"=w1971) -> ("error out"=w1969:errorcluster)  [unwired: 7 in, 1 out]
        n874 = call <vilib>:"Add State(s) to Queue__JKI_lib_State_Machine.vi"("State(s) in (\"\")"=w1979) -> ("States Out"=w1978:string)  [unwired: 14 in]
      }
      frame "SysConfig: Load LJ Pinout" {
        # "Template Separator\n(You can make a copy of, or modify, this frame)"
        n875 = call <userlib>:"Current VIs Parent Directory__ogtk.vi"() -> ("Parent Directory (+ Relative)"=w1994:path)  [unwired: 5 in]
        n876 = Build Path(base path=w1994, name or relative path="SubVI\\LabJack\\LJ_pin_setting.config") -> (appended path=w1992:path)
        n877 = call "ReadLabjackConfig(SubVI).vi"("error in (no error)"=w1990, "appended path"=w1992) -> ("error out"=w1991:errorcluster, "Utility"=w1988:T5)  [unwired: 8 in]
        n878 = Unbundle By Name(w1988) -> ("Ch1 Bias"=w1987:string, "Ch2 Bias"=w1986:string, "Ch3 Bias"=w1985:string, "Ch4 Bias"=w1980:string, "Red LED"=w1982:string, "Green LED"=w1981:string)
        n879 = global write "GlobalVariables.vi" "LED Green pin"(w1981) -> ()
        n880 = global write "GlobalVariables.vi" "Ch1 LJ pin"(w1987) -> ()
        n881 = global write "GlobalVariables.vi" "Ch2 LJ pin"(w1986) -> ()
        n882 = global write "GlobalVariables.vi" "Ch3 LJ pin"(w1985) -> ()
        n883 = global write "GlobalVariables.vi" "Ch4 LJ pin"(w1980) -> ()
        n884 = global write "GlobalVariables.vi" "LED Red pin"(w1982) -> ()
        n885 = Bundle By Name(cluster=w1983, "LJ Pinout"=w1988) -> (w1989:T23)
        n886 = call <vilib>:"Add State(s) to Queue__JKI_lib_State_Machine.vi"("State(s) in (\"\")"=w1996) -> ("States Out"=w1995:string)  [unwired: 14 in]
      }
      frame "SysConfig: Load 355 PWM" {
        # "Template Separator\n(You can make a copy of, or modify, this frame)"
        n887 = call <userlib>:"Current VIs Parent Directory__ogtk.vi"() -> ("Parent Directory (+ Relative)"=w2014:path)  [unwired: 5 in]
        n888 = Build Path(base path=w2014, name or relative path="SubVI\\LabJack\\PWM_setting_355.config") -> (appended path=w2012:path)
        n889 = call "ReadPWMConfig(SubVI).vi"("error in (no error)"=w2009, "appended path"=w2012) -> ("error out"=w2010:errorcluster, "PWM Setting"=w2008:T40)  [unwired: 8 in]
        n890 = Unbundle By Name(w2008) -> ("DIO_EF_CLOCK1_DIVISOR"=w2005:i16, "DIO_EF_CLOCK1_ROLL_VALUE"=w2004:i32)
        n891 = Multiply(x=w2005, y=w2004) -> (x*y=w2006:i32)
        n892 = Bundle By Name(cluster=w2011, "355 PWM setting"=w2008) -> (w1998:T23)
        n893 = Divide(x=80000000.0, y=w2006) -> (x/y=w2003:dbl)
        "Laser Rep Rate" <- w2003
        n894 = Number To Decimal String(number=w2003) -> (decimal integer string=w2002:string)  [unwired: 1 in]
        n895 = Concatenate Strings("355nm " ("string"), w2002, "Hz" ("string")) -> (w2000:string)
        n896 = property on="355nm Laser toggle" class="Bool (strict)"("Caption.Text"=w2000) -> ()  [unwired: 2 in, 2 out]
        n897 = call <vilib>:"Add State(s) to Queue__JKI_lib_State_Machine.vi"("State(s) in (\"\")"=w2016) -> ("States Out"=w2015:string)  [unwired: 14 in]
      }
      frame "SysConfig: Load AB PWM" {
        # "Template Separator\n(You can make a copy of, or modify, this frame)"
        n898 = call <userlib>:"Current VIs Parent Directory__ogtk.vi"() -> ("Parent Directory (+ Relative)"=w2025:path)  [unwired: 5 in]
        n899 = Build Path(base path=w2025, name or relative path="SubVI\\LabJack\\PWM_setting_AB.config") -> (appended path=w2023:path)
        n900 = call "ReadPWMConfig(SubVI).vi"("error in (no error)"=w2020, "appended path"=w2023) -> ("error out"=w2021:errorcluster, "PWM Setting"=w2019:T40)  [unwired: 8 in]
        n901 = Bundle By Name(cluster=w2017, "AB PWM setting"=w2019) -> (w2022:T23)
        n902 = call <vilib>:"Add State(s) to Queue__JKI_lib_State_Machine.vi"("State(s) in (\"\")"=w2027) -> ("States Out"=w2026:string)  [unwired: 14 in]
      }
      frame "SysConfig: Load AB setting" {
        # "load aming beam setting\n(check frequency, if 0 do nothing, if not zero, config PWM)"
        n903 = call "readAimingBeamSetting.vi"("error in (no error)"=w2045) -> ("error out"=w2040:errorcluster, "Aiming Beam Setting"=w2032:T41)  [unwired: 9 in]
        n904 = Unbundle By Name(w2032) -> ("Default Current"=w2031:dbl)
        n905 = Unbundle By Name(w2032) -> ("Frequency(Hz)"=w2028:u32)
        n906 = Equal To 0?(x=w2028) -> (x = 0?=w2038:bool)
        n907 = Select(t="", s=w2038, f="SysConfig: Load AB PWM" ("State(s) in Front (\"\")")) -> (s? t:f=w2041:string)
        n908 = Number To Decimal String(number=w2028) -> (decimal integer string=w2037:string)  [unwired: 1 in]
        n909 = Number To Decimal String(number=w2031, width (-)=i16 2) -> (decimal integer string=w2030:string)
        n910 = Concatenate Strings("445nm " ("string"), w2037, "Hz " ("string"), w2030, "mA" ("string")) -> (w2036:string)
        n911 = property on="Aiming beam toggle" class="Bool (strict)"("Caption.Text"=w2036) -> ()  [unwired: 2 in, 2 out]
        n912 = case shown="False" w2038 {
          tunnel: w2040 -> [w2053 w2056]
          tunnel: [w2052 w2056] -> w2039
          tunnel: w2028 -> [w2051 _]
          frame False {
            n913 = call "LJ_calculate_PWM_parameters.vi"("Duty Cycle (%)"=u32 10, "Error In"=w2053, "Show Confirmation"=FALSE, "Laser Rep Rate (Hz)"=w2051, "Laser"=enum16{"355nm", "AimingBeam"}."AimingBeam") -> ("Error Out"=w2052:errorcluster)  [unwired: 5 in, 1 out]
          }
          frame True {
          }
        }
        n914 = Bundle By Name(cluster=w2046, "AB Cluster"=w2032) -> (w2047:T23)
        n915 = call <vilib>:"Add State(s) to Queue__JKI_lib_State_Machine.vi"("State(s) in Front (\"\")"=w2041, "State(s) in (\"\")"=w2049) -> ("States Out"=w2048:string)  [unwired: 13 in]
      }
      frame "SysConfig: LoadABVideoSetting" {
        # "Load AB video setting form ini file\n()"
        n916 = call "readVideoConfig.vi"("error in (no error)"=w2060) -> ("error out"=w2061:errorcluster, "Aiming Beam Config"=w2059:T22)  [unwired: 8 in, 1 out]
        n917 = Bundle By Name(cluster=w2057, "VideoConfig"=w2059) -> (w2058:T23)
        n918 = call <vilib>:"Add State(s) to Queue__JKI_lib_State_Machine.vi"("State(s) in (\"\")"=w2064) -> ("States Out"=w2063:string)  [unwired: 14 in]
      }
      frame "SysConfig: LoadCursorLocation" {
        # "Load cursor location from ini file\n(load cursor from system setting ini file)"
        n919 = call "readCursorConfigMain.vi"("error in (no error)"=w2076) -> ("error out"=w2077:errorcluster, "Cursor Locations"=w2075:T42)  [unwired: 9 in]
        n920 = Unbundle By Name(w2075) -> ("DC1"=w2074:i32, "DC2"=w2073:i32, "BG1"=w2068:i32, "BG2"=w2067:i32)
        n921 = Build Array(w2074, w2073) -> (w2072:i32[])
        n922 = Build Array(w2068, w2067) -> (w2069:i32[])
        n923 = Array Max & Min(array=w2072) -> (max value=w2071:i32, min value=w2070:i32)  [unwired: 2 out]
        n924 = Array Max & Min(array=w2069) -> (max value=w2066:i32, min value=w2065:i32)  [unwired: 2 out]
        n925 = global write "GlobalVariables.vi" "DC Idx2"(w2071) -> ()
        n926 = global write "GlobalVariables.vi" "DC Idx1"(w2070) -> ()
        n927 = global write "GlobalVariables.vi" "BG Idx2"(w2066) -> ()
        n928 = global write "GlobalVariables.vi" "BG Idx1"(w2065) -> ()
        n929 = call <vilib>:"Add State(s) to Queue__JKI_lib_State_Machine.vi"("State(s) in (\"\")"=w2081) -> ("States Out"=w2080:string)  [unwired: 14 in]
      }
      frame "---------- SystemStatus ----------" {
        # "Template Separator\n(You can make a copy of, or modify, this frame)"
        n930 = call <vilib>:"Add State(s) to Queue__JKI_lib_State_Machine.vi"("State(s) in (\"\")"=w2086) -> ("States Out"=w2085:string)  [unwired: 14 in]
      }
      frame "SystemStatus: SlowSysStatusMacro" {
        # "store system check time"
        # "Template Separator\n(You can make a copy of, or modify, this frame)"
        n931 = Tick Count (ms)() -> (millisecond timer value=w2089:u32)
        n932 = Bundle By Name(cluster=w2087, "SlowTimer"=w2089) -> (w2088:T23)
        n933 = call <vilib>:"Add State(s) to Queue__JKI_lib_State_Machine.vi"("State(s) in Front (\"\")"="Digitizer: checkTemp\nTCP: CheckConnection" ("State(s) in Front (\"\")"), "State(s) in (\"\")"=w2094) -> ("States Out"=w2093:string)  [unwired: 13 in]
      }
      frame "SystemStatus: FastSysStatusMacro" {
        # "store system check time"
        # "Template Separator\n(You can make a copy of, or modify, this frame)"
        n934 = Tick Count (ms)() -> (millisecond timer value=w2097:u32)
        n935 = Bundle By Name(cluster=w2095, "FastTimer"=w2097) -> (w2096:T23)
        n936 = call <vilib>:"Add State(s) to Queue__JKI_lib_State_Machine.vi"("State(s) in Front (\"\")"="355 Laser: CheckPWMStatus\n/*AimingBeam: GetPWMStatus\n/*355 Laser: CheckControllerStatus" ("State(s) in Front (\"\")"), "State(s) in (\"\")"=w2102) -> ("States Out"=w2101:string)  [unwired: 13 in]
      }
      frame "---------- UI ----------" {
        # "Do not put any code in this frame.\n(It is a separator no-op. You can make a copy of this frame to create a new UI frame)"
        n937 = call <vilib>:"Add State(s) to Queue__JKI_lib_State_Machine.vi"("State(s) in (\"\")"=w2107) -> ("States Out"=w2106:string)  [unwired: 14 in]
      }
      frame "UI: Initialize" {
        w2109 = T43 {"Minimum"=0.0, "Maximum"=4.6, "Increment"=0.1} ("Data Entry Limits")
        w2108 = T11."Disabled and Grayed Out" ("Disabled")
        # "Disable all button on startup"
        # "Initialize the User Interface, here.\n(this is called automatically, by the Macro: Init)"
        n938 = property on="V 1" class="DigNum (strict)"("DisabledEnum"=w2108) -> ()  [unwired: 2 in, 2 out]
        n939 = property on="V 2" class="DigNum (strict)"("DisabledEnum"=w2108) -> ()  [unwired: 2 in, 2 out]
        n940 = property on="StopButton" class="Bool (strict)"("DisabledEnum"=w2108) -> ()  [unwired: 2 in, 2 out]
        n941 = property on="Sys Reconfig" class="Bool"("DisabledEnum"=w2108) -> ()  [unwired: 2 in, 2 out]
        n942 = property on="StartButton" class="Bool (strict)"("DisabledEnum"=w2108) -> ()  [unwired: 2 in, 2 out]
        n943 = property on="355nm Laser toggle" class="Bool (strict)"("DisabledEnum"=w2108) -> ()  [unwired: 2 in, 2 out]
        n944 = property on="Aiming beam toggle" class="Bool (strict)"("DisabledEnum"=w2108) -> ()  [unwired: 2 in, 2 out]
        n945 = property on="Background" class="Bool (strict)"("DisabledEnum"=w2108) -> ()  [unwired: 2 in, 2 out]
        n946 = property on="Cali&iRF alignment" class="Bool (strict)"("DisabledEnum"=w2108) -> ()  [unwired: 2 in, 2 out]
        n947 = property on="V 3" class="DigNum (strict)"("DisabledEnum"=w2108) -> ()  [unwired: 2 in, 2 out]
        n948 = property on="Video Source" class="RadioBtnsControl (strict)"("DisabledEnum"=w2108) -> ()  [unwired: 2 in, 2 out]
        n949 = property on="V 1" class="DigNum (strict)"("Data Range"=w2109) -> ()  [unwired: 2 in, 2 out]
        n950 = property on="V 2" class="DigNum (strict)"("Data Range"=w2109) -> ()  [unwired: 2 in, 2 out]
        n951 = property on="V 3" class="DigNum (strict)"("Data Range"=w2109) -> ()  [unwired: 2 in, 2 out]
        n952 = call <vilib>:"Add State(s) to Queue__JKI_lib_State_Machine.vi"("State(s) in Front (\"\")"="UI: CaliAndiRFNotReady" ("State(s) in Front (\"\")"), "State(s) in (\"\")"=w2115) -> ("States Out"=w2114:string)  [unwired: 13 in]
      }
      frame "UI: BGLoaded" {
        # "[Covers: REQ24]"
        # "Do not put any code in this frame.\n(It is a separator no-op. You can make a copy of this frame to create a new UI frame)"
        n953 = property on="Background" class="Bool (strict)"("BoolText.Text"="Loaded!" ("Boolean Text.Text"), "Colors [4]"=cluster{u32, u32}[] [{15764023, 15764023}, {16711680, 16711680}]) -> ()  [unwired: 2 in, 2 out]
        n954 = call <vilib>:"Add State(s) to Queue__JKI_lib_State_Machine.vi"("State(s) in (\"\")"=w2122) -> ("States Out"=w2121:string)  [unwired: 14 in]
      }
      frame "UI: BGSizeError" {
        # "[Covers: REQ24]"
        # "Do not put any code in this frame.\n(It is a separator no-op. You can make a copy of this frame to create a new UI frame)"
        n955 = property on="Background" class="Bool (strict)"("BoolText.Text"="Loaded!" ("Boolean Text.Text"), "Colors [4]"=cluster{u32, u32}[] [{7171459, 7171459}, {16711680, 16711680}]) -> ()  [unwired: 2 in, 2 out]
        n956 = One Button Dialog(message="Background waveform length and current digitizer setting mismatch! Please take a new background before any aquisition!") -> ()  [unwired: 1 in, 1 out]
        n957 = call <vilib>:"Add State(s) to Queue__JKI_lib_State_Machine.vi"("State(s) in (\"\")"=w2130) -> ("States Out"=w2129:string)  [unwired: 14 in]
      }
      frame "UI: CaliAndiRFLoaded" {
        # "[Covers: REQ24]"
        # "Do not put any code in this frame.\n(It is a separator no-op. You can make a copy of this frame to create a new UI frame)"
        n958 = property on="Cali&iRF alignment" class="Bool (strict)"("BoolText.Text"="Loaded!" ("Boolean Text.Text"), "Colors [4]"=cluster{u32, u32}[] [{15764023, 15764023}, {16711680, 16711680}]) -> ()  [unwired: 2 in, 2 out]
        n959 = call <vilib>:"Add State(s) to Queue__JKI_lib_State_Machine.vi"("State(s) in (\"\")"=w2137) -> ("States Out"=w2136:string)  [unwired: 14 in]
      }
      frame "UI: WFAutoScale" {
        # "Set graph auto scale.\n(UI: WFAutoScale >> T/F)"
        n960 = Equal?(x=w2138, y="F") -> (x = y?=w2139:bool)
        n961 = Equal?(x=w2138, y="T") -> (x = y?=w2141:bool)
        n962 = case shown="True" w2141 {
          frame False {
          }
          frame True {
            w2157 = u8 2 ("Y Scale.Scale Fit")
            n963 = property on="Channel 1" class="WFGraph (strict)"("YScale.ScaleFit"=w2157) -> ()  [unwired: 2 in, 2 out]
            n964 = property on="Channel 2" class="WFGraph (strict)"("YScale.ScaleFit"=w2157) -> ()  [unwired: 2 in, 2 out]
            n965 = property on="Channel 3" class="WFGraph (strict)"("YScale.ScaleFit"=w2157) -> ()  [unwired: 2 in, 2 out]
          }
        }
        n966 = case shown="True" w2139 {
          frame False {
          }
          frame True {
            w2154 = 0.0 ("Y Scale.Range:Maximum")
            w2155 = 2.0 ("Y Scale.Range:Maximum")
            w2156 = u8 0 ("Y Scale.Scale Fit")
            n967 = property on="Channel 1" class="WFGraph (strict)"("YScale.ScaleFit"=w2156) -> (error out=w2153:errorcluster)  [unwired: 2 in, 1 out]
            n968 = property on="Channel 2" class="WFGraph (strict)"("YScale.ScaleFit"=w2156) -> (error out=w2152:errorcluster)  [unwired: 2 in, 1 out]
            n969 = property on="Channel 3" class="WFGraph (strict)"("YScale.ScaleFit"=w2156) -> (error out=w2151:errorcluster)  [unwired: 2 in, 1 out]
            n970 = property on="Channel 1" class="WFGraph (strict)"(error in=w2153, "YScale.Maximum"=w2155) -> (error out=w2150:errorcluster)  [unwired: 1 in, 1 out]
            n971 = property on="Channel 2" class="WFGraph (strict)"(error in=w2152, "YScale.Maximum"=w2155) -> (error out=w2149:errorcluster)  [unwired: 1 in, 1 out]
            n972 = property on="Channel 3" class="WFGraph (strict)"(error in=w2151, "YScale.Maximum"=w2155) -> (error out=w2148:errorcluster)  [unwired: 1 in, 1 out]
            n973 = property on="Channel 1" class="WFGraph (strict)"(error in=w2150, "YScale.Minimum"=w2154) -> ()  [unwired: 1 in, 2 out]
            n974 = property on="Channel 2" class="WFGraph (strict)"(error in=w2149, "YScale.Minimum"=w2154) -> ()  [unwired: 1 in, 2 out]
            n975 = property on="Channel 3" class="WFGraph (strict)"(error in=w2148, "YScale.Minimum"=w2154) -> ()  [unwired: 1 in, 2 out]
          }
        }
        n976 = call <vilib>:"Add State(s) to Queue__JKI_lib_State_Machine.vi"("State(s) in (\"\")"=w2147) -> ("States Out"=w2146:string)  [unwired: 14 in]
      }
      frame "UI: showDisclaimer" {
        # "Show disclamer window.\n(It is a separator no-op. You can make a copy of this frame to create a new UI frame)"
        n977 = call <vilib>:"Application Directory.vi"() -> ("Application Directory"=w2170:path)
        n978 = Build Path(base path=w2170, name or relative path="Disclamer.png") -> (appended path=w2168:path)
        n979 = property on="Disclamer" class="Pict"() -> ("Draw Area Size"=w2166:T44)  [unwired: 2 in, 2 out]
        n980 = disable-structure "Diagram Disable Structure" shown="Disabled" {
          frame Disabled {
            n981 = flat-sequence {
              frame #0 {
                n982 = call "disclaimer.vi"() -> ()  [unwired: 12 in]
              }
              frame #1 {
                n983 = Wait (ms)(milliseconds to wait=u32 250) -> ()  [unwired: 1 out]
              }
              frame #2 {
                n984 = call "SoftwareNote.vi"() -> ()  [unwired: 12 in]
              }
            }
          }
          frame Enabled {
          }
        }
        n985 = call <vilib>:"Read PNG File.vi"("path to PNG file"=w2168) -> ("image data"=w2165:T45)  [unwired: 8 in, 2 out]
        n986 = Unbundle By Name(w2165) -> ("Rectangle.right"=w2163:i16, "Rectangle.bottom"=w2161:i16)
        n987 = Unbundle By Name(w2166) -> ("Width"=w2164:u32, "Height"=w2162:u32)
        n988 = call <vilib>:"Draw Flattened Pixmap.vi"("image data"=w2165) -> ("new picture"=→"Disclamer":picture)  [unwired: 8 in]
        n989 = Divide(x=w2164, y=w2163) -> (x/y=w2160:dbl)
        n990 = Divide(x=w2162, y=w2161) -> (x/y=w2159:dbl)
        n991 = Max & Min(x=w2160, y=w2159) -> (min(x,y)=w2158:dbl)  [unwired: 1 out]
        n992 = property on="Disclamer" class="Pict"("ZoomFactor"=w2158) -> ()  [unwired: 2 in, 2 out]
        n993 = call <vilib>:"Add State(s) to Queue__JKI_lib_State_Machine.vi"("State(s) in (\"\")"=w2175) -> ("States Out"=w2174:string)  [unwired: 14 in]
      }
      frame "UI: CaliAndiRFNotReady" {
        # "Do not put any code in this frame.\n(It is a separator no-op. You can make a copy of this frame to create a new UI frame)"
        n994 = property on="Cali&iRF alignment" class="Bool (strict)"("BoolText.Text"="No Info" ("Boolean Text.Text"), "Colors [4]"=cluster{u32, u32}[] [{13816530, 13816530}, {16711680, 16711680}]) -> ()  [unwired: 2 in, 2 out]
        n995 = call <vilib>:"Add State(s) to Queue__JKI_lib_State_Machine.vi"("State(s) in (\"\")"=w2183) -> ("States Out"=w2182:string)  [unwired: 14 in]
      }
      frame "UI: BGnotReady" {
        # "Do not put any code in this frame.\n(It is a separator no-op. You can make a copy of this frame to create a new UI frame)"
        n996 = property on="Background" class="Bool (strict)"("BoolText.Text"="No Info" ("Boolean Text.Text"), "Colors [4]"=cluster{u32, u32}[] [{13816530, 13816530}, {16711680, 16711680}]) -> ()  [unwired: 2 in, 2 out]
        n997 = call <vilib>:"Add State(s) to Queue__JKI_lib_State_Machine.vi"("State(s) in (\"\")"=w2190) -> ("States Out"=w2189:string)  [unwired: 14 in]
      }
      frame "UI: Reset" {
        w2192 = cluster{u32, u32}[] [{13816530, 13816530}, {13816530, 13816530}] ("Colors [4]")
        # "Do not put any code in this frame.\n(It is a separator no-op. You can make a copy of this frame to create a new UI frame)"
        n998 = property on="Cali&iRF alignment" class="Bool (strict)"("BoolText.Text"="No Info" ("Boolean Text.Text"), "Colors [4]"=w2192) -> ()  [unwired: 2 in, 2 out]
        n999 = property on="Background" class="Bool (strict)"("BoolText.Text"="No Info" ("Boolean Text.Text"), "Colors [4]"=w2192) -> ()  [unwired: 2 in, 2 out]
        n1000 = call <vilib>:"Add State(s) to Queue__JKI_lib_State_Machine.vi"("State(s) in (\"\")"=w2198) -> ("States Out"=w2197:string)  [unwired: 14 in]
      }
      frame "UI: SetButtonText" {
        # "Set button text of 355nm laser and aiming beam."
        n1001 = call <vilib>:"Add State(s) to Queue__JKI_lib_State_Machine.vi"("State(s) in (\"\")"=w2203) -> ("States Out"=w2202:string)  [unwired: 14 in]
      }
      frame "UI: DuringAquisition" {
        w2206 = T11."Disabled and Grayed Out" ("Disabled")
        # "Do not put any code in this frame.\n(It is a separator no-op. You can make a copy of this frame to create a new UI frame)"
        n1002 = Unbundle By Name(w2205) -> ("bothVidSourceAvail"=w2204:bool)
        n1003 = case shown="True" w2204 {
          tunnel: w2206 -> [_ w2212]
          frame False {
          }
          frame True {
            n1004 = property on="Video Source" class="RadioBtnsControl (strict)"("DisabledEnum"=w2212) -> ()  [unwired: 2 in, 2 out]
          }
        }
        n1005 = property on="StartButton" class="Bool (strict)"("DisabledEnum"=w2206) -> ()  [unwired: 2 in, 2 out]
        n1006 = property on="Sys Reconfig" class="Bool"("DisabledEnum"=w2206) -> ()  [unwired: 2 in, 2 out]
        n1007 = property on="355nm Laser toggle" class="Bool (strict)"("DisabledEnum"=w2206) -> ()  [unwired: 2 in, 2 out]
        n1008 = property on="Aiming beam toggle" class="Bool (strict)"("DisabledEnum"=w2206) -> ()  [unwired: 2 in, 2 out]
        n1009 = property on="Background" class="Bool (strict)"("DisabledEnum"=w2206) -> ()  [unwired: 2 in, 2 out]
        n1010 = property on="Radio Buttons" class="RadioBtnsControl (strict)"("DisabledEnum"=w2206) -> ()  [unwired: 2 in, 2 out]
        n1011 = property on="Cali&iRF alignment" class="Bool (strict)"("DisabledEnum"=w2206) -> ()  [unwired: 2 in, 2 out]
        n1012 = property on="Quit" class="Bool"("DisabledEnum"=w2206) -> ()  [unwired: 2 in, 2 out]
        n1013 = property on="Skip Data Save?" class="Bool (strict)"("DisabledEnum"=w2206) -> ()  [unwired: 2 in, 2 out]
        n1014 = property on="Video Display" class="Bool (strict)"("DisabledEnum"=w2206) -> ()  [unwired: 2 in, 2 out]
        n1015 = property on="StopButton" class="Bool (strict)"("DisabledEnum"=T11."Enabled" ("Disabled")) -> ()  [unwired: 2 in, 2 out]
        n1016 = call <vilib>:"Add State(s) to Queue__JKI_lib_State_Machine.vi"("State(s) in (\"\")"=w2211) -> ("States Out"=w2210:string)  [unwired: 14 in]
      }
      frame "UI: duringIRFAlign" {
        w2213 = T11."Disabled and Grayed Out" ("Disabled")
        # "Set UI to during iRF alignment\n(It is a separator no-op. You can make a copy of this frame to create a new UI frame)"
        n1017 = property on="StartButton" class="Bool (strict)"("DisabledEnum"=w2213) -> ()  [unwired: 2 in, 2 out]
        n1018 = property on="Sys Reconfig" class="Bool"("DisabledEnum"=w2213) -> ()  [unwired: 2 in, 2 out]
        n1019 = property on="355nm Laser toggle" class="Bool (strict)"("DisabledEnum"=w2213) -> ()  [unwired: 2 in, 2 out]
        n1020 = property on="Aiming beam toggle" class="Bool (strict)"("DisabledEnum"=w2213) -> ()  [unwired: 2 in, 2 out]
        n1021 = property on="Background" class="Bool (strict)"("DisabledEnum"=w2213) -> ()  [unwired: 2 in, 2 out]
        n1022 = property on="StopButton" class="Bool (strict)"("DisabledEnum"=w2213) -> ()  [unwired: 2 in, 2 out]
        n1023 = call <vilib>:"Add State(s) to Queue__JKI_lib_State_Machine.vi"("State(s) in (\"\")"=w2218) -> ("States Out"=w2217:string)  [unwired: 14 in]
      }
      frame "UI: duringBGAcquire" {
        w2219 = T11."Disabled and Grayed Out" ("Disabled")
        # "Do not put any code in this frame.\n(It is a separator no-op. You can make a copy of this frame to create a new UI frame)"
        n1024 = property on="StartButton" class="Bool (strict)"("DisabledEnum"=w2219) -> ()  [unwired: 2 in, 2 out]
        n1025 = property on="StopButton" class="Bool (strict)"("DisabledEnum"=w2219) -> ()  [unwired: 2 in, 2 out]
        n1026 = property on="Sys Reconfig" class="Bool"("DisabledEnum"=w2219) -> ()  [unwired: 2 in, 2 out]
        n1027 = property on="355nm Laser toggle" class="Bool (strict)"("DisabledEnum"=w2219) -> ()  [unwired: 2 in, 2 out]
        n1028 = property on="Aiming beam toggle" class="Bool (strict)"("DisabledEnum"=w2219) -> ()  [unwired: 2 in, 2 out]
        n1029 = property on="Cali&iRF alignment" class="Bool (strict)"("DisabledEnum"=w2219) -> ()  [unwired: 2 in, 2 out]
        n1030 = call <vilib>:"Add State(s) to Queue__JKI_lib_State_Machine.vi"("State(s) in (\"\")"=w2224) -> ("States Out"=w2223:string)  [unwired: 14 in]
      }
      frame "UI: ReadyForAquisition" {
        w2228 = T11."Enabled" ("Disabled")
        # "Do not put any code in this frame.\n(It is a separator no-op. You can make a copy of this frame to create a new UI frame)"
        n1031 = Unbundle By Name(w2227) -> ("System Status.TCP/IP"=w2226:bool, "bothVidSourceAvail"=w2225:bool)
        n1032 = property on="StartButton" class="Bool (strict)"("DisabledEnum"=w2228) -> ()  [unwired: 2 in, 2 out]
        n1033 = property on="Sys Reconfig" class="Bool"("DisabledEnum"=w2228) -> ()  [unwired: 2 in, 2 out]
        n1034 = property on="355nm Laser toggle" class="Bool (strict)"("DisabledEnum"=w2228) -> ()  [unwired: 2 in, 2 out]
        n1035 = property on="Aiming beam toggle" class="Bool (strict)"("DisabledEnum"=w2228) -> ()  [unwired: 2 in, 2 out]
        n1036 = property on="Cali&iRF alignment" class="Bool (strict)"("DisabledEnum"=w2228) -> ()  [unwired: 2 in, 2 out]
        n1037 = property on="Background" class="Bool (strict)"("DisabledEnum"=w2228) -> ()  [unwired: 2 in, 2 out]
        n1038 = property on="Quit" class="Bool"("DisabledEnum"=w2228) -> ()  [unwired: 2 in, 2 out]
        n1039 = property on="Radio Buttons" class="RadioBtnsControl (strict)"("DisabledEnum"=w2228) -> ()  [unwired: 2 in, 2 out]
        n1040 = case shown="True" w2225 {
          tunnel: w2228 -> [_ w2234]
          frame False {
          }
          frame True {
            n1041 = property on="Video Source" class="RadioBtnsControl (strict)"("DisabledEnum"=w2234) -> ()  [unwired: 2 in, 2 out]
          }
        }
        n1042 = property on="Skip Data Save?" class="Bool (strict)"("DisabledEnum"=w2228) -> ()  [unwired: 2 in, 2 out]
        n1043 = case shown="True" w2226 {
          tunnel: w2228 -> [_ w2235]
          frame False {
          }
          frame True {
            n1044 = property on="Video Display" class="Bool (strict)"("DisabledEnum"=w2235) -> ()  [unwired: 2 in, 2 out]
          }
        }
        n1045 = property on="StopButton" class="Bool (strict)"("DisabledEnum"=T11."Disabled and Grayed Out" ("Disabled")) -> ()  [unwired: 2 in, 2 out]
        n1046 = call <vilib>:"Add State(s) to Queue__JKI_lib_State_Machine.vi"("State(s) in (\"\")"=w2233) -> ("States Out"=w2232:string)  [unwired: 14 in]
      }
      frame "UI: Update" {
        # "Do not put any code in this frame.\n(It is a separator no-op. You can make a copy of this frame to create a new UI frame)"
        n1047 = Unbundle By Name(w2246) -> ("System Status"=→"System Hardware Connection Status":T2, "IDs.RunID"=→"Run #":i8, "CaseID"=→"Case #":string, "FLImDAQ"=→"FLImDAQ":T30, "SysRunning?"=→"Aquisition Status:":bool, "LJ Pinout"=→"LJ Pinout":T5, "IDs.BG ID"=→"BG #":i8, "IDs.Cali ID"=→"Calibration #":i8, "video source"=→"Visualization PC video source":T1)
        n1048 = call <vilib>:"Add State(s) to Queue__JKI_lib_State_Machine.vi"("State(s) in (\"\")"=w2249) -> ("States Out"=w2248:string)  [unwired: 14 in]
      }
      frame "UI: updateVideoToggle" {
        # "Set video toggle based on visualization PC video source.\n(take )"
        n1049 = call <vilib>:"Add State(s) to Queue__JKI_lib_State_Machine.vi"("State(s) in (\"\")"=w2254) -> ("States Out"=w2253:string)  [unwired: 14 in]
      }
      frame "UI: Cursor Set" {
        # "Argument"
        # "Set and Unset Cursor Busy.\n(Usage: \"UI: Cursor Set >> Busy|Idle\")"
        n1050 = case shown="\"Idle\", Default" w2256 {
          tunnel: w2258 -> [w2263 w2265]
          tunnel: [w2262 w2264] -> w2257
          frame "Idle", Default {
            n1051 = call <vilib>:"Unset Busy.vi"("error in (no error)"=w2263) -> ("error out"=w2262:errorcluster)  [unwired: 10 in]
          }
          frame "Busy" {
            n1052 = call <vilib>:"Set Busy.vi"("error in (no error)"=w2265) -> ("error out"=w2264:errorcluster)  [unwired: 9 in, 1 out]
          }
        }
        n1053 = call <vilib>:"Add State(s) to Queue__JKI_lib_State_Machine.vi"("State(s) in (\"\")"=w2261) -> ("States Out"=w2260:string)  [unwired: 14 in]
      }
      frame "UI: Front Panel State" {
        # "Argument"
        # "Set Front Panel Open or Closed\n(Usage: \"UI: Front Panel State >> Open|Close\")"
        n1054 = Unbundle By Name(w2269) -> ("Core.Current VI Reference"=w2268:refnum<vi>)
        n1055 = case shown="\"Open\", \"Standard\", Default" w2267 {
          tunnel: w2271 -> [w2279 w2294 w2305 w2318 w2331]
          tunnel: [w2281 w2295 w2307 w2320 w2333] -> w2270
          tunnel: w2268 -> [w2280 w2292 w2306 w2319 w2332]
          frame "Open", "Standard", Default {
            w2274 = T17."Standard" ("State")
            n1056 = property on="Property Node" class="VI"(reference=w2280, error in=w2279) -> (reference out=w2277:refnum<vi>, error out=w2278:errorcluster, "FP.State"=w2276:T17)
            n1057 = Not Equal?(x=w2276, y=w2274) -> (x != y?=w2275:bool)
            n1058 = case shown="True" w2275 {
              tunnel: [w2285 w2287] -> w2281
              tunnel: w2278 -> [w2284 w2287]
              tunnel: w2277 -> [w2283 _]
              tunnel: w2274 -> [w2282 _]
              frame True {
                n1059 = invoke on="Invoke Node" class="VI" method="FP.Open"(reference=w2283, error in=w2284, "Activate"=TRUE, "State"=w2282) -> (error out=w2285:errorcluster)  [unwired: 1 in, 4 out]
              }
              frame False {
              }
            }
          }
          frame "Close", "Closed" {
            n1060 = property on="Property Node" class="VI"(reference=w2292, error in=w2294) -> (reference out=w2291:refnum<vi>, error out=w2293:errorcluster, "FP.State"=w2289:T17)
            n1061 = Not Equal?(x=w2289, y=T17."Closed" ("Front Panel Window:State")) -> (x != y?=w2288:bool)
            n1062 = case shown="True" w2288 {
              tunnel: [w2296 w2299] -> w2295
              tunnel: w2293 -> [w2296 w2298]
              tunnel: w2291 -> [_ w2297]
              frame False {
              }
              frame True {
                n1063 = invoke on="Invoke Node" class="VI" method="FP.Close"(reference=w2297, error in=w2298) -> (error out=w2299:errorcluster)  [unwired: 1 in, 2 out]
              }
            }
          }
          frame "Hidden", "Hide" {
            w2300 = T17."Hidden" ("State")
            n1064 = property on="Property Node" class="VI"(reference=w2306, error in=w2305) -> (reference out=w2303:refnum<vi>, error out=w2304:errorcluster, "FP.State"=w2302:T17)
            n1065 = Not Equal?(x=w2302, y=w2300) -> (x != y?=w2301:bool)
            n1066 = case shown="True" w2301 {
              tunnel: [w2311 w2312] -> w2307
              tunnel: w2304 -> [w2310 w2312]
              tunnel: w2303 -> [w2309 _]
              tunnel: w2300 -> [w2308 _]
              frame True {
                n1067 = invoke on="Invoke Node" class="VI" method="FP.Open"(reference=w2309, error in=w2310, "State"=w2308) -> (error out=w2311:errorcluster)  [unwired: 2 in, 4 out]
              }
              frame False {
              }
            }
          }
          frame "Minimize", "Minimized" {
            w2313 = T17."Minimized" ("State")
            n1068 = property on="Property Node" class="VI"(reference=w2319, error in=w2318) -> (reference out=w2316:refnum<vi>, error out=w2317:errorcluster, "FP.State"=w2315:T17)
            n1069 = Not Equal?(x=w2315, y=w2313) -> (x != y?=w2314:bool)
            n1070 = case shown="True" w2314 {
              tunnel: [w2324 w2325] -> w2320
              tunnel: w2317 -> [w2323 w2325]
              tunnel: w2316 -> [w2322 _]
              tunnel: w2313 -> [w2321 _]
              frame True {
                n1071 = invoke on="Invoke Node" class="VI" method="FP.Open"(reference=w2322, error in=w2323, "State"=w2321) -> (error out=w2324:errorcluster)  [unwired: 2 in, 4 out]
              }
              frame False {
              }
            }
          }
          frame "Maximize", "Maximized" {
            w2326 = T17."Maximized" ("State")
            n1072 = property on="Property Node" class="VI"(reference=w2332, error in=w2331) -> (reference out=w2329:refnum<vi>, error out=w2330:errorcluster, "FP.State"=w2328:T17)
            n1073 = Not Equal?(x=w2328, y=w2326) -> (x != y?=w2327:bool)
            n1074 = case shown="True" w2327 {
              tunnel: [w2337 w2338] -> w2333
              tunnel: w2330 -> [w2336 w2338]
              tunnel: w2329 -> [w2335 _]
              tunnel: w2326 -> [w2334 _]
              frame True {
                n1075 = invoke on="Invoke Node" class="VI" method="FP.Open"(reference=w2335, error in=w2336, "State"=w2334) -> (error out=w2337:errorcluster)  [unwired: 2 in, 4 out]
              }
              frame False {
              }
            }
          }
        }
        n1076 = call <vilib>:"Add State(s) to Queue__JKI_lib_State_Machine.vi"("State(s) in (\"\")"=w2273) -> ("States Out"=w2272:string)  [unwired: 14 in]
      }
      frame "---------- AimingBeam ----------" {
        # "Template Separator\n(You can make a copy of, or modify, this frame)"
        n1077 = call <vilib>:"Add State(s) to Queue__JKI_lib_State_Machine.vi"("State(s) in (\"\")"=w2343) -> ("States Out"=w2342:string)  [unwired: 14 in]
      }
      frame "AimingBeam: Initialize" {
        # "set aiming beam button color"
        # "Open COM port for Aiming Beam\n(Require USB connection)"
        n1078 = Unbundle By Name(w2345) -> ("AB Cluster.Aiming Beam COM Port"=w2353:refnum<visa-resource-name>)
        n1079 = call-poly "VISA Configure Serial Port"("VISA resource name"=w2353, "Enable Termination\nChar (T)"=TRUE ("Enable Termination\nChar (T)"), "baud rate (9600)"=u32 9600, "error in (no error)"=w2350) -> ("error out"=w2349:errorcluster)  [unwired: 10 in, 1 out]
        n1080 = Unbundle By Name(w2349) -> ("status"=w2348:bool)
        n1081 = Not(x=w2348) -> (.not. x?=w2347:bool)
        n1082 = Bundle By Name(cluster=w2345, "System Status.Aiming Beam"=w2347) -> (w2346:T23)
        n1083 = call <vilib>:"Add State(s) to Queue__JKI_lib_State_Machine.vi"("State(s) in (\"\")"=w2355) -> ("States Out"=w2354:string)  [unwired: 14 in]
      }
      frame "AimingBeam: Close" {
        # "Close Aiming Beam COM port\n(Require USB connection to Aiming Beam Laser)"
        n1084 = Unbundle By Name(w2358) -> ("AB Cluster.Aiming Beam COM Port"=w2362:refnum<visa-resource-name>)
        n1085 = VISA Close(VISA resource name=w2362, error in (no error)=w2360) -> (error out=w2361:errorcluster)
        n1086 = Bundle By Name(cluster=w2358, "System Status.Aiming Beam"=FALSE) -> (w2359:T23)
        n1087 = call <vilib>:"Add State(s) to Queue__JKI_lib_State_Machine.vi"("State(s) in (\"\")"=w2364) -> ("States Out"=w2363:string)  [unwired: 14 in]
      }
      frame "AimingBeam: Set Current" {
        # "Set Aiming Beam Current\n(You can make a copy of, or modify, this frame)"
        n1088 = Unbundle By Name(w2379) -> ("AB Cluster.Aiming Beam COM Port"=w2372:refnum<visa-resource-name>, "AB Cluster.Max Current"=w2368:dbl, "AB Cluster.Default Current"=w2370:dbl, "AB Cluster.Min Current"=w2369:dbl)
        n1089 = In Range and Coerce(upper limit=w2368, x=w2370, lower limit=w2369) -> (coerced(x)=w2365:dbl)  [unwired: 1 out]
        n1090 = Number To Fractional String(number=w2365, precision (6)=i16 2) -> (F-format string=w2373:string)  [unwired: 2 in]
        n1091 = Concatenate Strings("slc:", w2373, "\r" ("Carriage Return Constant"), "\n" ("Line Feed Constant")) -> (w2376:string)
        n1092 = VISA Write(VISA resource name=w2372, write buffer=w2376, error in (no error)=w2367) -> (error out=w2371:errorcluster)  [unwired: 2 out]
        n1093 = call <vilib>:"Add State(s) to Queue__JKI_lib_State_Machine.vi"("State(s) in (\"\")"=w2381) -> ("States Out"=w2380:string)  [unwired: 14 in]
      }
      frame "AimingBeam: Set Status" {
        # "Enable Aiming Beam\n(Usage: \"AimingBeam: Set >> Enable|Disable\")"
        n1094 = Unbundle By Name(w2388) -> ("AB Cluster.Aiming Beam COM Port"=w2385:refnum<visa-resource-name>)
        n1095 = case shown="\"Enable\"" w2387 {
          tunnel: [w2391 w2395] -> w2386
          frame "Disable", Default {
            n1096 = Concatenate Strings("cof", "\r" ("Carriage Return Constant"), "\n" ("Line Feed Constant")) -> (w2391:string)
          }
          frame "Enable" {
            n1097 = Concatenate Strings("con", "\r" ("Carriage Return Constant"), "\n" ("Line Feed Constant")) -> (w2395:string)
          }
        }
        n1098 = VISA Write(VISA resource name=w2385, write buffer=w2386, error in (no error)=w2383) -> (error out=w2384:errorcluster)  [unwired: 2 out]
        n1099 = call <vilib>:"Add State(s) to Queue__JKI_lib_State_Machine.vi"("State(s) in (\"\")"=w2390) -> ("States Out"=w2389:string)  [unwired: 14 in]
      }
      frame "AimingBeam: GetPWMStatus" {
        # "Get aiming beam PWM status\n()"
        n1100 = Unbundle By Name(w2403) -> ("AB Cluster.Freq"=w2402:i32, "LJ Pinout.AimingBeam PWM"=w2409:string)
        n1101 = Equal To 0?(x=w2402) -> (x = 0?=w2401:bool)
        n1102 = call "LabJack_FGV.vi"("Operation(Read)"=enum16{"Write", "Read"}."Read" ("Operation"), "error in (no error)"=w2405) -> ("error out"=w2407:errorcluster, "Read data"=w2408:i32)  [unwired: 8 in]
        n1103 = case shown="True" w2401 {
          tunnel: w2409 -> [w2422 _]
          tunnel: [w2420 "DIO_STATE"] -> w2406
          frame False {
            n1104 = Concatenate Strings(w2422, "_EF_ENABLE" ("string")) -> (w2420:string)
          }
          frame True {
          }
        }
        n1105 = call "LJM_eReadName.vi"("Handle In"=w2408, "Name"=w2406, "error in"=w2407) -> ("Value"=w2400:dbl, "error out"=w2404:errorcluster)  [unwired: 10 in, 1 out]
        n1106 = case shown="True" w2401 {
          tunnel: w2400 -> [w2415 w2419]
          tunnel: [w2414 w2416] -> w2399
          frame False {
            n1107 = Greater Than 0?(x=w2415) -> (x > 0?=w2414:bool)
          }
          frame True {
            n1108 = Number To Boolean Array(number=w2419) -> (Boolean array=w2418:bool[])
            n1109 = Index Array(array=w2418, index=3) -> (element=w2416:bool)
          }
        }
        n1110 = case shown="False" w2399 {
          frame False {
            # "PWM is off\nset color to dark green"
            n1111 = local write "Aiming beam toggle"(FALSE ("Aimging beam")) -> ()
          }
          frame True {
            # "PWM is on\nset color to light green"
            n1112 = local write "Aiming beam toggle"(TRUE ("Aimging beam")) -> ()
          }
        }
        n1113 = call <vilib>:"Add State(s) to Queue__JKI_lib_State_Machine.vi"("State(s) in (\"\")"=w2413) -> ("States Out"=w2412:string)  [unwired: 14 in]
      }
      frame "---------- 355 Laser ----------" {
        # "Template Separator\n(You can make a copy of, or modify, this frame)"
        n1114 = call <vilib>:"Add State(s) to Queue__JKI_lib_State_Machine.vi"("State(s) in (\"\")"=w2430) -> ("States Out"=w2429:string)  [unwired: 14 in]
      }
      frame "355 Laser: Check Dewelling" {
        # "if time laser start time is less than 7.5s before, wait 250ms then check again."
        # "Template Separator\n(You can make a copy of, or modify, this frame)"
        n1115 = Unbundle By Name(w2438) -> ("Laser start tic"=w2435:u32)
        n1116 = Tick Count (ms)() -> (millisecond timer value=w2436:u32)
        n1117 = Subtract(x=w2436, y=w2435) -> (x-y=w2434:u32)
        n1118 = Greater?(x=w2434, y=u32 5000) -> (0:w2432:bool)
        n1119 = case shown="False" w2432 {
          tunnel: ["355 Laser: Check Dewelling" ""] -> w2431
          frame False {
            n1120 = Wait (ms)(milliseconds to wait=u32 250) -> ()  [unwired: 1 out]
          }
          frame True {
          }
        }
        n1121 = call <vilib>:"Add State(s) to Queue__JKI_lib_State_Machine.vi"("State(s) in Front (\"\")"=w2431, "State(s) in (\"\")"=w2441) -> ("States Out"=w2440:string)  [unwired: 13 in]
      }
      frame "355 Laser: Laser enable" {
        # "Laser enable/disable\n(Usage: \"LabJack: Laser enable/disable >> 1|0\")"
        n1122 = Unbundle By Name(w2448) -> ("LJ Pinout.Laser Start/Stop"=w2452:string, "System Status.355 Laser"=w2446:bool)
        n1123 = case shown="False" w2446 {
          tunnel: w2445 -> [w2467 w2468]
          tunnel: w2452 -> [w2461 _]
          tunnel: [w2456 w2468] -> w2450
          tunnel: [w2455 u32 0 ("millisecond timer value")] -> w2447
          frame False {
            n1124 = call "LabJack_FGV.vi"("Operation(Read)"=enum16{"Write", "Read"}."Read" ("Operation")) -> ("Read data"=w2463:i32)  [unwired: 9 in, 1 out]
            n1125 = call "LJM_eWriteName.vi"("Handle In"=w2463, "Name"=w2461, "Value"=1.0, "error in"=w2467) -> ("Handle Out"=w2462:i32, "error out"=w2460:errorcluster)  [unwired: 10 in]
            n1126 = call <userlib>:"Wait (ms)__ogtk.vi"("error in (no error)"=w2460, "milliseconds to wait"=u32 250) -> ("error out"=w2459:errorcluster)  [unwired: 8 in, 1 out]
            n1127 = call "LJM_eWriteName.vi"("Handle In"=w2462, "Name"=w2461, "Value"=0.0, "error in"=w2459) -> ("error out"=w2457:errorcluster)  [unwired: 10 in, 1 out]
            n1128 = call <userlib>:"Tick Count (ms)__ogtk.vi"("error in (no error)"=w2457) -> ("error out"=w2456:errorcluster, "millisecond timer value"=w2455:u32)  [unwired: 9 in]
          }
          frame True {
          }
        }
        n1129 = Bundle By Name(cluster=w2448, "Laser start tic"=w2447) -> (w2449:T23)
        n1130 = call <vilib>:"Add State(s) to Queue__JKI_lib_State_Machine.vi"("State(s) in (\"\")"=w2454) -> ("States Out"=w2453:string)  [unwired: 14 in]
      }
      frame "355 Laser: Laser disable" {
        # "Laser enable/disable\n(Usage: \"LabJack: Laser enable/disable >> 1|0\")"
        n1131 = Unbundle By Name(w2472) -> ("LJ Pinout.Laser Start/Stop"=w2476:string, "System Status.355 Laser"=w2470:bool)
        n1132 = case shown="True" w2470 {
          tunnel: w2477 -> [w2480 w2494]
          tunnel: w2476 -> [_ w2488]
          tunnel: [w2480 w2483] -> w2474
          tunnel: [u32 0 ("millisecond timer value") w2482] -> w2471
          frame False {
          }
          frame True {
            n1133 = call "LabJack_FGV.vi"("Operation(Read)"=enum16{"Write", "Read"}."Read" ("Operation")) -> ("Read data"=w2490:i32)  [unwired: 9 in, 1 out]
            n1134 = call "LJM_eWriteName.vi"("Handle In"=w2490, "Name"=w2488, "Value"=1.0, "error in"=w2494) -> ("Handle Out"=w2489:i32, "error out"=w2487:errorcluster)  [unwired: 10 in]
            n1135 = call <userlib>:"Wait (ms)__ogtk.vi"("error in (no error)"=w2487, "milliseconds to wait"=u32 250) -> ("error out"=w2486:errorcluster)  [unwired: 8 in, 1 out]
            n1136 = call "LJM_eWriteName.vi"("Handle In"=w2489, "Name"=w2488, "Value"=0.0, "error in"=w2486) -> ("error out"=w2484:errorcluster)  [unwired: 10 in, 1 out]
            n1137 = call <userlib>:"Tick Count (ms)__ogtk.vi"("error in (no error)"=w2484) -> ("error out"=w2483:errorcluster, "millisecond timer value"=w2482:u32)  [unwired: 9 in]
          }
        }
        n1138 = Bundle By Name(cluster=w2472, "Laser start tic"=w2471) -> (w2473:T23)
        n1139 = call <vilib>:"Add State(s) to Queue__JKI_lib_State_Machine.vi"("State(s) in (\"\")"=w2479) -> ("States Out"=w2478:string)  [unwired: 14 in]
      }
      frame "355 Laser: Dewelling" {
        # "Wait some time (ms)\n(355 Laser: Dewelling >> #)"
        n1140 = Fract/Exp String To Number(string=w2498, default (0 dbl)=0) -> (number=w2496:i32)  [unwired: 2 in, 1 out]
        n1141 = Wait (ms)(milliseconds to wait=w2496) -> ()  [unwired: 1 out]
        n1142 = call <vilib>:"Add State(s) to Queue__JKI_lib_State_Machine.vi"("State(s) in (\"\")"=w2502) -> ("States Out"=w2501:string)  [unwired: 14 in]
      }
      frame "355 Laser: Close" {
        # "Template Separator\n(You can make a copy of, or modify, this frame)"
        n1143 = call <vilib>:"Add State(s) to Queue__JKI_lib_State_Machine.vi"("State(s) in Front (\"\")"="355 Laser: CheckControllerStatus\n355 Laser: Laser disable\n355 Laser: Dewelling >>1000", "State(s) in (\"\")"=w2508) -> ("States Out"=w2507:string)  [unwired: 13 in]
      }
      frame "355 Laser: CheckControllerStatus" {
        # "if average < 2, laser no power\nif average 2 < average < 9.3, laser on\nif 9.3<average<10, interlock open, blink indicator\nif average > 10, laser off\n[Covers: REQ30]"
        # "take 10 measuremt and look at average"
        # "Check 355 laser controller status\nBy probing Emisison Lamp negative terminal voltage"
        n1144 = Unbundle By Name(w2517) -> ("LJ Pinout.Laser Ready"=w2520:string)
        n1145 = call "LabJack_FGV.vi"("Operation(Read)"=enum16{"Write", "Read"}."Read" ("Operation")) -> ("Read data"=w2521:i32)  [unwired: 9 in, 1 out]
        n1146 = for {
          N: 20 -> [_]
          tunnel: w2521 -> [w2532]
          tunnel: w2520 -> [w2531]
          shift-right: [w2530] -> w2513
          shift-left: w2519 -> [w2529]
          tunnel: [w2527] -> w2512 mode=indexing
          n1147 = call "LJM_eReadName.vi"("Handle In"=w2532, "Name"=w2531, "error in"=w2529) -> ("Value"=w2527:dbl, "error out"=w2530:errorcluster)  [unwired: 10 in, 1 out]
          n1148 = Wait (ms)(milliseconds to wait=u32 25) -> ()  [unwired: 1 out]
        }
        n1149 = call "checkLaserStatus.vi"("error in (no error)"=w2513, "Laser LED voltage"=w2512) -> ("error out"=w2514:errorcluster, "Interlock open?"=w2509:bool, "Laser on?"=w2511:bool, "Mean voltage"=→"laser EM lamp V":dbl)  [unwired: 6 in]
        n1150 = Bundle By Name(cluster=w2517, "System Status.355 Laser"=w2511) -> (w2518:T23)
        n1151 = case shown="True" w2509 {
          frame False {
            n1152 = property on="355 Laser" class="Bool (strict)"("Blinking"=FALSE) -> ()  [unwired: 2 in, 2 out]
          }
          frame True {
            n1153 = property on="355 Laser" class="Bool (strict)"("Blinking"=TRUE) -> ()  [unwired: 2 in, 2 out]
          }
        }
        n1154 = call <vilib>:"Add State(s) to Queue__JKI_lib_State_Machine.vi"("State(s) in (\"\")"=w2524) -> ("States Out"=w2523:string)  [unwired: 14 in]
      }
      frame "355 Laser: CheckPWMStatus" {
        # "Check 355 laser PWM status\n(Read LJ DIO#EF_ENABLE register to determine PWM status)"
        n1155 = Unbundle By Name(w2542) -> ("LJ Pinout.355 PWM"=w2541:string)
        n1156 = call "LabJack_FGV.vi"("Operation(Read)"=enum16{"Write", "Read"}."Read" ("Operation"), "error in (no error)"=w2535) -> ("error out"=w2538:errorcluster, "Read data"=w2539:i32)  [unwired: 8 in]
        n1157 = Concatenate Strings(w2541, "_EF_ENABLE" ("string")) -> (w2537:string)
        n1158 = call "LJM_eReadName.vi"("Handle In"=w2539, "Name"=w2537, "error in"=w2538) -> ("Value"=w2534:dbl, "error out"=w2536:errorcluster)  [unwired: 10 in, 1 out]
        n1159 = Greater Than 0?(x=w2534) -> (x > 0?=w2533:bool)
        n1160 = case shown="False" w2533 {
          frame False {
            # "PWM is off\nset color to gray"
            n1161 = local write "355nm Laser toggle"(FALSE ("355nm Laser")) -> ()
          }
          frame True {
            # "PWM is on\nset color to light green"
            n1162 = local write "355nm Laser toggle"(TRUE ("355nm Laser")) -> ()
          }
        }
        n1163 = call <vilib>:"Add State(s) to Queue__JKI_lib_State_Machine.vi"("State(s) in (\"\")"=w2546) -> ("States Out"=w2545:string)  [unwired: 14 in]
      }
      frame "355 Laser: Start" {
        # "Template Separator\n(You can make a copy of, or modify, this frame)"
        n1164 = call <vilib>:"Add State(s) to Queue__JKI_lib_State_Machine.vi"("State(s) in Front (\"\")"="LabJack: 355_PWM_Start", "State(s) in (\"\")"=w2554) -> ("States Out"=w2553:string)  [unwired: 13 in]
      }
      frame "355 Laser: Stop" {
        # "Template Separator\n(You can make a copy of, or modify, this frame)"
        n1165 = call <vilib>:"Add State(s) to Queue__JKI_lib_State_Machine.vi"("State(s) in Front (\"\")"="LabJack: 355_PWM_Stop", "State(s) in (\"\")"=w2560) -> ("States Out"=w2559:string)  [unwired: 13 in]
      }
      frame "---------- Utility ----------" {
        # "Template Separator\n(You can make a copy of, or modify, this frame)"
        n1166 = call <vilib>:"Add State(s) to Queue__JKI_lib_State_Machine.vi"("State(s) in (\"\")"=w2565) -> ("States Out"=w2564:string)  [unwired: 14 in]
      }
      frame "Utility: SetDataClass" {
        # "Set Data Class in Queues\n(Set data class to either Data, Bg or Cali)"
        n1167 = case shown="\"Cali\"" w2567 {
          tunnel: [enum16{"Data", "BG", "Cali"}."Data" ("Data Class") enum16{"Data", "BG", "Cali"}."BG" ("Data Class") enum16{"Data", "BG", "Cali"}."Cali" ("Data Class")] -> w2566
          frame "Data", Default {
          }
          frame "Bg" {
          }
          frame "Cali" {
          }
        }
        n1168 = local write "Data Class"(w2566) -> ()
        n1169 = call <vilib>:"Add State(s) to Queue__JKI_lib_State_Machine.vi"("State(s) in (\"\")"=w2572) -> ("States Out"=w2571:string)  [unwired: 14 in]
      }
      frame "Utility: AquiTimerReset" {
        # "Set Aquisition Timer\n(You can make a copy of, or modify, this frame)"
        n1170 = Tick Count (ms)() -> (millisecond timer value=w2578:u32)
        n1171 = Bundle By Name(cluster=w2576, "Aquisition Timer"=w2578) -> (w2577:T23)
        n1172 = call <vilib>:"Add State(s) to Queue__JKI_lib_State_Machine.vi"("State(s) in (\"\")"=w2582) -> ("States Out"=w2581:string)  [unwired: 14 in]
      }
      frame "Utility: AquiTimerCheck" {
        # "5min to ms"
        # "Set Aquisition Timer\n([Covers: REQ35])"
        n1173 = Unbundle By Name(w2590) -> ("Aquisition Timer"=w2588:u32)
        n1174 = Tick Count (ms)() -> (millisecond timer value=w2589:u32)
        n1175 = Subtract(x=w2589, y=w2588) -> (x-y=w2587:u32)
        n1176 = Multiply(x=1000, y=300) -> (x*y=w2584:i32)
        n1177 = Greater Or Equal?(x=w2587, y=w2584) -> (x >= y?=w2583:bool)
        n1178 = case shown="True" w2583 {
          frame False {
            # "do nothing"
          }
          frame True {
            # "if timed out, stop aquisition"
            n1179 = property on="StopButton" class="Bool (strict)"("Val(Sgnl)"=TRUE ("Value (Signaling)")) -> ()  [unwired: 2 in, 2 out]
          }
        }
        n1180 = call <vilib>:"Add State(s) to Queue__JKI_lib_State_Machine.vi"("State(s) in (\"\")"=w2594) -> ("States Out"=w2593:string)  [unwired: 14 in]
      }
      frame "Utility: StartBeep" {
        # "Beep\n([Covers: REQ18])"
        n1181 = call <vilib>:"Beep.vi"("use system alert? (T)"=FALSE, "duration (msec)"=u32 1000, "frequency (Hz)"=u32 2000) -> ()  [unwired: 9 in]
        n1182 = call <vilib>:"Add State(s) to Queue__JKI_lib_State_Machine.vi"("State(s) in (\"\")"=w2603) -> ("States Out"=w2602:string)  [unwired: 14 in]
      }
      frame "Utility: EndBeep" {
        # "Beep\n([Covers: REQ18])"
        n1183 = flat-sequence {
          frame #0 {
            n1184 = call <vilib>:"Beep.vi"("use system alert? (T)"=FALSE, "duration (msec)"=u32 500, "frequency (Hz)"=u32 2000) -> ()  [unwired: 9 in]
          }
          frame #1 {
            n1185 = call <vilib>:"Beep.vi"("use system alert? (T)"=FALSE, "duration (msec)"=u32 500, "frequency (Hz)"=u32 2000) -> ()  [unwired: 9 in]
          }
        }
        n1186 = call <vilib>:"Add State(s) to Queue__JKI_lib_State_Machine.vi"("State(s) in (\"\")"=w2608) -> ("States Out"=w2607:string)  [unwired: 14 in]
      }
      frame "Utility: RestoreDeConChan" {
        # "Template Separator\n(You can make a copy of, or modify, this frame)"
        n1187 = global read "GlobalVariables.vi" "DeconChan Temp"() -> (w2615:T9)
        n1188 = local write "Radio Buttons"(w2615) -> ()
        n1189 = call <vilib>:"Add State(s) to Queue__JKI_lib_State_Machine.vi"("State(s) in (\"\")"=w2620) -> ("States Out"=w2619:string)  [unwired: 14 in]
      }
      frame "Utility: SaveDeconChan" {
        # "Save Decon Channel to global temp\n(You can make a copy of, or modify, this frame)"
        n1190 = flat-sequence {
          frame #0 {
            n1191 = local read "Radio Buttons"() -> (w2626:T9)
            n1192 = global write "GlobalVariables.vi" "DeconChan Temp"(w2626) -> ()
          }
          frame #1 {
            n1193 = local write "Radio Buttons"(T9."No Selection" ("Radio Buttons")) -> ()
          }
        }
        n1194 = flat-sequence {
          frame #0 {
          }
          frame #1 {
            (unwired) enum32{"No Selection", "Ch1", "Ch2", "Ch3"}."No Selection" ("Radio Buttons")
          }
        }
        n1195 = call <vilib>:"Add State(s) to Queue__JKI_lib_State_Machine.vi"("State(s) in (\"\")"=w2625) -> ("States Out"=w2624:string)  [unwired: 14 in]
      }
      frame "Utility: Dewelling" {
        # "Main loop dewell\n(Dewelling >> #)"
        n1196 = Fract/Exp String To Number(string=w2631, default (0 dbl)=0) -> (number=w2629:i32)  [unwired: 2 in, 1 out]
        n1197 = Wait (ms)(milliseconds to wait=w2629) -> ()  [unwired: 1 out]
        n1198 = call <vilib>:"Add State(s) to Queue__JKI_lib_State_Machine.vi"("State(s) in (\"\")"=w2635) -> ("States Out"=w2634:string)  [unwired: 14 in]
      }
      frame "Utility: SetAllChanManualGain" {
        w2636 = FALSE ("Value (Signaling)")
        # "Set all channel to manual gain\n(You can make a copy of, or modify, this frame)"
        n1199 = property on="Auto gain ch1" class="Bool (strict)"("Val(Sgnl)"=w2636) -> ()  [unwired: 2 in, 2 out]
        n1200 = property on="Auto gain ch2" class="Bool (strict)"("Val(Sgnl)"=w2636) -> ()  [unwired: 2 in, 2 out]
        n1201 = property on="Auto gain ch3" class="Bool (strict)"("Val(Sgnl)"=w2636) -> ()  [unwired: 2 in, 2 out]
        n1202 = property on="Auto gain ch4" class="Bool (strict)"("Val(Sgnl)"=w2636) -> ()  [unwired: 2 in, 2 out]
        n1203 = call <vilib>:"Add State(s) to Queue__JKI_lib_State_Machine.vi"("State(s) in (\"\")"=w2641) -> ("States Out"=w2640:string)  [unwired: 14 in]
      }
      frame "Utility: SetAllChanAutoGain" {
        w2642 = TRUE ("Value (Signaling)")
        # "Set all channels to auto gain\n(You can make a copy of, or modify, this frame)"
        n1204 = property on="Auto gain ch1" class="Bool (strict)"("Val(Sgnl)"=w2642) -> ()  [unwired: 2 in, 2 out]
        n1205 = property on="Auto gain ch2" class="Bool (strict)"("Val(Sgnl)"=w2642) -> ()  [unwired: 2 in, 2 out]
        n1206 = property on="Auto gain ch3" class="Bool (strict)"("Val(Sgnl)"=w2642) -> ()  [unwired: 2 in, 2 out]
        n1207 = property on="Auto gain ch4" class="Bool (strict)"("Val(Sgnl)"=w2642) -> ()  [unwired: 2 in, 2 out]
        n1208 = call <vilib>:"Add State(s) to Queue__JKI_lib_State_Machine.vi"("State(s) in (\"\")"=w2647) -> ("States Out"=w2646:string)  [unwired: 14 in]
      }
      frame "---------- SysLog ----------" {
        # "Template Separator\n(You can make a copy of, or modify, this frame)"
        n1209 = call <vilib>:"Add State(s) to Queue__JKI_lib_State_Machine.vi"("State(s) in (\"\")"=w2652) -> ("States Out"=w2651:string)  [unwired: 14 in]
      }
      frame "SysLog: OpenLogFile" {
        # "Template Separator\n(You can make a copy of, or modify, this frame)"
        n1210 = call <vilib>:"Add State(s) to Queue__JKI_lib_State_Machine.vi"("State(s) in (\"\")"=w2657) -> ("States Out"=w2656:string)  [unwired: 14 in]
      }
      frame "---------- Graph ----------" {
        # "Template Separator\n(You can make a copy of, or modify, this frame)"
        n1211 = call <vilib>:"Add State(s) to Queue__JKI_lib_State_Machine.vi"("State(s) in (\"\")"=w2662) -> ("States Out"=w2661:string)  [unwired: 14 in]
      }
      frame "Graph: SetXMultiplier" {
        # "Set X multiplier of WF graphs\n(You can make a copy of, or modify, this frame)"
        n1212 = call "Digitizer1_FGV.vi"() -> ("error out"=w2666:errorcluster, "Read data"=w2667:refnum<k15>)  [unwired: 10 in]
        n1213 = property class="niScope"(reference=w2667, error in=w2666) -> ("Min Sample Rate"=w2665:dbl)  [unwired: 2 out]
        n1214 = Divide(x=1.0, y=w2665) -> (x/y=w2663:dbl)
        n1215 = property on="Channel 1" class="WFGraph (strict)"("XScale.Multiplier"=w2663) -> ()  [unwired: 2 in, 2 out]
        n1216 = property on="Channel 2" class="WFGraph (strict)"("XScale.Multiplier"=w2663) -> ()  [unwired: 2 in, 2 out]
        n1217 = property on="Channel 3" class="WFGraph (strict)"("XScale.Multiplier"=w2663) -> ()  [unwired: 2 in, 2 out]
        n1218 = call <vilib>:"Add State(s) to Queue__JKI_lib_State_Machine.vi"("State(s) in (\"\")"=w2672) -> ("States Out"=w2671:string)  [unwired: 14 in]
      }
      frame "Graph: AddCursors" {
        # "Add BG and DC cursor to all graphs\n(You can make a copy of, or modify, this frame)"
        n1219 = property on="Channel 1" class="WFGraph (strict)"() -> ("XScale.Multiplier"=w2679:dbl)  [unwired: 2 in, 2 out]
        n1220 = global read "GlobalVariables.vi" "DC Idx1"() -> (w2678:i32)
        n1221 = global read "GlobalVariables.vi" "DC Idx2"() -> (w2677:i32)
        n1222 = global read "GlobalVariables.vi" "BG Idx1"() -> (w2676:i32)
        n1223 = global read "GlobalVariables.vi" "BG Idx2"() -> (w2675:i32)
        n1224 = property on="Channel 2" class="WFGraph (strict)"() -> ("CrsrList"=w2687:T24)  [unwired: 2 in, 2 out]
        n1225 = property on="Channel 3" class="WFGraph (strict)"() -> ("CrsrList"=w2686:T24)  [unwired: 2 in, 2 out]
        n1226 = property on="Channel 1" class="WFGraph (strict)"(error in=w2681) -> ("CrsrList"=w2690:T24)  [unwired: 1 in, 2 out]
        n1227 = Build Array(w2678, w2677, w2676, w2675) -> (w2674:i32[])
        n1228 = Multiply(x=w2674, y=w2679) -> (x*y=w2673:dbl[])
        n1229 = for {
          tunnel: w2690 -> [w2702] mode=indexing
          tunnel: w2673 -> [w2698] mode=indexing
          tunnel: [w2701] -> w2689 mode=indexing
          tunnel: u32[] [6618880, 6618880, 16711680, 16711680] -> [w2697] mode=indexing
          tunnel: w2687 -> [w2700] mode=indexing
          tunnel: w2686 -> [w2699] mode=indexing
          tunnel: [w2696] -> w2685 mode=indexing
          tunnel: [w2695] -> w2684 mode=indexing
          n1230 = Bundle By Name(cluster=w2702, "Position.X"=w2698, "Color"=w2697) -> (w2701:T25)
          n1231 = Bundle By Name(cluster=w2700, "Position.X"=w2698, "Color"=w2697) -> (w2696:T25)
          n1232 = Bundle By Name(cluster=w2699, "Position.X"=w2698, "Color"=w2697) -> (w2695:T25)
        }
        n1233 = control-ref of="Channel 1"() -> (w2683:refnum<vi>)
        n1234 = property on="Channel 1" class="WFGraph (strict)"("CrsrList"=w2689) -> (error out=w2680:errorcluster)  [unwired: 2 in, 1 out]
        n1235 = property on="Channel 2" class="WFGraph (strict)"("CrsrList"=w2685) -> ()  [unwired: 2 in, 2 out]
        n1236 = property on="Channel 3" class="WFGraph (strict)"("CrsrList"=w2684) -> ()  [unwired: 2 in, 2 out]
        n1237 = call "UpdateCurserIdx(SubVI).vi"("error in (no error)"=w2680, "WaveformGraph in"=w2683) -> ("error out"=w2682:errorcluster)  [unwired: 9 in]
        n1238 = call <vilib>:"Add State(s) to Queue__JKI_lib_State_Machine.vi"("State(s) in (\"\")"=w2694) -> ("States Out"=w2693:string)  [unwired: 14 in]
      }
      frame "Graph: SaveCursorLoc" {
        # "Save cursor location to ini file\n(Save cursor location to system setting ini file)"
        n1239 = global read "GlobalVariables.vi" "DC Idx1"() -> (w2709:i32)
        n1240 = global read "GlobalVariables.vi" "DC Idx2"() -> (w2708:i32)
        n1241 = global read "GlobalVariables.vi" "BG Idx1"() -> (w2707:i32)
        n1242 = global read "GlobalVariables.vi" "BG Idx2"() -> (w2706:i32)
        n1243 = Bundle("DC Idx1"=w2709, "DC Idx2"=w2708, "BG Idx1"=w2707, "BG Idx2"=w2706) -> (w2705:T46)  [unwired: 1 in]
        n1244 = call "writeCursorConfigMain.vi"("error in (no error)"=w2703, "Cursor Locations"=w2705) -> ("error out"=w2704:errorcluster)  [unwired: 9 in]
        n1245 = call <vilib>:"Add State(s) to Queue__JKI_lib_State_Machine.vi"("State(s) in (\"\")"=w2713) -> ("States Out"=w2712:string)  [unwired: 14 in]
      }
      frame "---------- APD ----------" {
        # "Template Separator\n(You can make a copy of, or modify, this frame)"
        n1246 = call <vilib>:"Add State(s) to Queue__JKI_lib_State_Machine.vi"("State(s) in (\"\")"=w2718) -> ("States Out"=w2717:string)  [unwired: 14 in]
      }
      frame "APD: Initialize" {
        w2725 = enum16{"Read", "Write"}."Write" ("Operation (Read)")
        w2724 = refnum<class "APDClass.lvclass"> refnum  # APDClass.lvclass
        # "Initialize APD FGV\n(Initialized APD FGV for holding data)"
        n1247 = call "APD1FGV.vi"("Error In"=w2719, "Operation (Read)"=w2725, "APDClass in"=w2724) -> ("Error Out"=w2723:errorcluster)  [unwired: 7 in, 1 out]
        n1248 = call "APD2FGV.vi"("Error In"=w2719, "Operation (Read)"=w2725, "APDClass in"=w2724) -> ("Error Out"=w2722:errorcluster)  [unwired: 7 in, 1 out]
        n1249 = call "APD3FGV.vi"("Error In"=w2719, "Operation (Read)"=w2725, "APDClass in"=w2724) -> ("Error Out"=w2721:errorcluster)  [unwired: 7 in, 1 out]
        n1250 = Merge Errors(w2723, w2722, w2721) -> (w2720:errorcluster)
        n1251 = call <vilib>:"Add State(s) to Queue__JKI_lib_State_Machine.vi"("State(s) in (\"\")"=w2729) -> ("States Out"=w2728:string)  [unwired: 14 in]
      }
      frame "APD: LoadFromSerial" {
        w2731 = enum16{"Read", "Write"}."Write" ("Operation (Read)")
        # "Load APD data from tdms file\n(load and update FGV)"
        n1252 = call "readAPDSerial.vi"("Error In"=w2738) -> ("Error Out"=w2734:errorcluster, "output cluster"=w2737:T26)  [unwired: 9 in]
        n1253 = Unbundle By Name(w2737) -> ("Ch1APDSerial#"=w2750:string, "Ch2APDSerial#"=w2736:string, "Ch3APDSerial#"=w2749:string, "Ch4APDSerial#"=w2735:string)
        n1254 = call "CreatFromSerialNumNoRaw.vi"("error in (no error)"=w2734, "APD Serial #"=w2750) -> ("error out"=w2747:errorcluster, "APDClass out"=w2748:refnum<class "APDClass.lvclass">)  [unwired: 8 in]
        n1255 = call "CreatFromSerialNumNoRaw.vi"("error in (no error)"=w2734, "APD Serial #"=w2736) -> ("error out"=w2745:errorcluster, "APDClass out"=w2746:refnum<class "APDClass.lvclass">)  [unwired: 8 in]
        n1256 = call "CreatFromSerialNumNoRaw.vi"("error in (no error)"=w2734, "APD Serial #"=w2749) -> ("error out"=w2743:errorcluster, "APDClass out"=w2744:refnum<class "APDClass.lvclass">)  [unwired: 8 in]
        n1257 = call "CreatFromSerialNumNoRaw.vi"("error in (no error)"=w2734, "APD Serial #"=w2735) -> ("error out"=w2732:errorcluster, "APDClass out"=w2733:refnum<class "APDClass.lvclass">)  [unwired: 8 in]
        n1258 = call "APD1FGV.vi"("Error In"=w2747, "Operation (Read)"=w2731, "APDClass in"=w2748) -> ("Error Out"=w2742:errorcluster)  [unwired: 7 in, 1 out]
        n1259 = call "APD2FGV.vi"("Error In"=w2745, "Operation (Read)"=w2731, "APDClass in"=w2746) -> ("Error Out"=w2740:errorcluster)  [unwired: 7 in, 1 out]
        n1260 = call "APD3FGV.vi"("Error In"=w2743, "Operation (Read)"=w2731, "APDClass in"=w2744) -> ("Error Out"=w2741:errorcluster)  [unwired: 7 in, 1 out]
        n1261 = call "APD4FGV.vi"("Error In"=w2732, "Operation (Read)"=w2731, "APDClass in"=w2733) -> ("Error Out"=w2730:errorcluster)  [unwired: 7 in, 1 out]
        n1262 = Merge Errors(w2742, w2740, w2741, w2730) -> (w2739:errorcluster)
        n1263 = call <vilib>:"Add State(s) to Queue__JKI_lib_State_Machine.vi"("State(s) in (\"\")"=w2754) -> ("States Out"=w2753:string)  [unwired: 14 in]
      }
      frame "APD: UpdateCtrlVLimit" {
        w2760 = enum16{"Read", "Write"}."Read" ("Operation (Read)")
        # "Set V limit\n(You can make a copy of, or modify, this frame)"
        n1264 = call "APD1FGV.vi"("Error In"=w2761, "Operation (Read)"=w2760) -> ("Error Out"=w2776:errorcluster, "APDClass out"=w2777:refnum<class "APDClass.lvclass">)  [unwired: 8 in]
        n1265 = call "APD2FGV.vi"("Error In"=w2761, "Operation (Read)"=w2760) -> ("Error Out"=w2774:errorcluster, "APDClass out"=w2775:refnum<class "APDClass.lvclass">)  [unwired: 8 in]
        n1266 = call "APD3FGV.vi"("Error In"=w2761, "Operation (Read)"=w2760) -> ("Error Out"=w2772:errorcluster, "APDClass out"=w2773:refnum<class "APDClass.lvclass">)  [unwired: 8 in]
        n1267 = call "APD4FGV.vi"("Error In"=w2761, "Operation (Read)"=w2760) -> ("Error Out"=w2758:errorcluster, "APDClass out"=w2759:refnum<class "APDClass.lvclass">)  [unwired: 8 in]
        n1268 = call-dynamic "ReadMaxCtrlV.vi"("error in (no error)"=w2776, "APDClass in"=w2777) -> ("error out"=w2767:errorcluster, "Numeric"=w2770:dbl)  [unwired: 7 in, 1 out]
        n1269 = call-dynamic "ReadMaxCtrlV.vi"("error in (no error)"=w2774, "APDClass in"=w2775) -> ("error out"=w2765:errorcluster, "Numeric"=w2769:dbl)  [unwired: 7 in, 1 out]
        n1270 = call-dynamic "ReadMaxCtrlV.vi"("error in (no error)"=w2772, "APDClass in"=w2773) -> ("error out"=w2763:errorcluster, "Numeric"=w2768:dbl)  [unwired: 7 in, 1 out]
        n1271 = call-dynamic "ReadMaxCtrlV.vi"("error in (no error)"=w2758, "APDClass in"=w2759) -> ("error out"=w2756:errorcluster, "Numeric"=w2757:dbl)  [unwired: 7 in, 1 out]
        n1272 = property on="V 1" class="DigNum (strict)"(error in=w2767, "Maximum"=w2770) -> (error out=w2766:errorcluster)  [unwired: 1 in, 1 out]
        n1273 = property on="V 2" class="DigNum (strict)"(error in=w2765, "Maximum"=w2769) -> (error out=w2764:errorcluster)  [unwired: 1 in, 1 out]
        n1274 = property on="V 4" class="DigNum (strict)"(error in=w2756, "Maximum"=w2757) -> (error out=w2755:errorcluster)  [unwired: 1 in, 1 out]
        n1275 = property on="V 3" class="DigNum (strict)"(error in=w2763, "Maximum"=w2768) -> (error out=w2762:errorcluster)  [unwired: 1 in, 1 out]
        n1276 = Merge Errors(w2766, w2764, w2762, w2755) -> (w2771:errorcluster)
        n1277 = call <vilib>:"Add State(s) to Queue__JKI_lib_State_Machine.vi"("State(s) in (\"\")"=w2781) -> ("States Out"=w2780:string)  [unwired: 14 in]
      }
      frame "APD: GetGainLimits" {
        w2786 = enum16{"Read", "Write"}."Read" ("Operation (Read)")
        # "Template Separator\n(You can make a copy of, or modify, this frame)"
        n1278 = call "APD1FGV.vi"("Error In"=w2787, "Operation (Read)"=w2786) -> ("Error Out"=w2792:errorcluster, "APDClass out"=w2793:refnum<class "APDClass.lvclass">)  [unwired: 8 in]
        n1279 = call "APD2FGV.vi"("Error In"=w2787, "Operation (Read)"=w2786) -> ("Error Out"=w2799:errorcluster, "APDClass out"=w2800:refnum<class "APDClass.lvclass">)  [unwired: 8 in]
        n1280 = call "APD3FGV.vi"("Error In"=w2787, "Operation (Read)"=w2786) -> ("Error Out"=w2797:errorcluster, "APDClass out"=w2798:refnum<class "APDClass.lvclass">)  [unwired: 8 in]
        n1281 = call "APD4FGV.vi"("Error In"=w2787, "Operation (Read)"=w2786) -> ("Error Out"=w2784:errorcluster, "APDClass out"=w2785:refnum<class "APDClass.lvclass">)  [unwired: 8 in]
        n1282 = call-dynamic "Read Gain Limits(Log).vi"("error in (no error)"=w2792, "APDClass in"=w2793) -> ("error out"=w2791:errorcluster, "GainLimits(Log)"=w2788:cluster{"GainMax":dbl, "GainMin":dbl})  [unwired: 7 in, 1 out]
        n1283 = call-dynamic "Read Gain Limits(Log).vi"("error in (no error)"=w2799, "APDClass in"=w2800) -> ("error out"=w2795:errorcluster, "GainLimits(Log)"=w2790:cluster{"GainMax":dbl, "GainMin":dbl})  [unwired: 7 in, 1 out]
        n1284 = call-dynamic "Read Gain Limits(Log).vi"("error in (no error)"=w2797, "APDClass in"=w2798) -> ("error out"=w2794:errorcluster, "GainLimits(Log)"=w2789:cluster{"GainMax":dbl, "GainMin":dbl})  [unwired: 7 in, 1 out]
        n1285 = call-dynamic "Read Gain Limits(Log).vi"("error in (no error)"=w2784, "APDClass in"=w2785) -> ("error out"=w2782:errorcluster, "GainLimits(Log)"=w2783:cluster{"GainMax":dbl, "GainMin":dbl})  [unwired: 7 in, 1 out]
        n1286 = Merge Errors(w2791, w2795, w2794, w2782) -> (w2796:errorcluster)
        n1287 = global write "GlobalVariables.vi" "Ch1GainLim(Log)"(w2788) -> ()
        n1288 = global write "GlobalVariables.vi" "Ch2GainLim(Log)"(w2790) -> ()
        n1289 = global write "GlobalVariables.vi" "Ch3GainLim(Log)"(w2789) -> ()
        n1290 = global write "GlobalVariables.vi" "Ch4GainLim(Log)"(w2783) -> ()
        n1291 = call <vilib>:"Add State(s) to Queue__JKI_lib_State_Machine.vi"("State(s) in (\"\")"=w2804) -> ("States Out"=w2803:string)  [unwired: 14 in]
      }
      frame "---------- TCP ----------" {
        # "Template Separator\n(You can make a copy of, or modify, this frame)"
        n1292 = call <vilib>:"Add State(s) to Queue__JKI_lib_State_Machine.vi"("State(s) in (\"\")"=w2809) -> ("States Out"=w2808:string)  [unwired: 14 in]
      }
      frame "TCP: InitializeNew" {
        # "if unsuccessful and count <10, increament count \nand try again"
        # "Initialize TCP connection to aimging beam computer\n(You can make a copy of, or modify, this frame)"
        n1293 = TCP Create Listener(10:u16 2100 ("port"), 11:"RTLT" ("service name")) -> (0:w2818:errorcluster, 3:w2810:refnum<k5>)  [unwired: 3 in, 1 out]
        n1294 = while {
          tunnel: w2810 -> [w2838]
          tunnel: w2818 -> [w2837]
          tunnel: [w2828] -> w2816
          tunnel: [w2825] -> w2812
          i -> [w2834]
          stop <- w2825 stop-if-true
          n1295 = TCP Wait On Listener(8:w2837, 9:100 ("timeout ms (wait forever: -1)"), 11:w2838) -> (0:w2835:errorcluster, 4:w2832:refnum<k5>)  [unwired: 1 in, 3 out]
          n1296 = Less Or Equal?(x=50, y=w2834) -> (x <= y?=w2831:bool)
          n1297 = case shown="No Error" w2835 {
            selector: w2835 -> [w2848 w2858]
            tunnel: w2832 -> [w2849 _]
            tunnel: [errorcluster {"status"=TRUE, "code"=0, "source"=""} ("No error") w2859] -> w2827
            tunnel: [w2840 FALSE ("TCP connected?")] -> w2828
            frame No Error {
              # "connection is ready, read data"
              n1298 = TCP Read(connection ID=w2849, bytes to read=512, error in (no error)=w2848, 7:T21."CRLF" ("mode (standard)"), 9:5000 ("timeout ms (25000)")) -> (connection ID out=w2842:refnum<k5>, data out=w2844:string, error out=w2841:errorcluster)
              n1299 = Concatenate Strings("alive" ("string"), "\r\n" ("End of Line Constant")) -> (w2845:string)
              n1300 = Equal?(x=w2845, y=w2844) -> (x = y?=w2843:bool)
              n1301 = case shown="False" w2843 {
                tunnel: w2842 -> [_ w2854]
                tunnel: w2841 -> [_ _]
                tunnel: [FALSE ("TCP connected?") TRUE ("TCP connected?")] -> w2840
                frame False {
                }
                frame True {
                  n1302 = call "TcpIDFGV.vi"("action"=enum16{"write", "read"}."write", "connection ID in"=w2854) -> ()  [unwired: 8 in, 2 out]
                }
              }
            }
            frame Error {
              # "connection not ready, keep waiting"
              n1303 = Unbundle By Name(w2858) -> ("code"=w2860:i32)
              n1304 = case shown="56" w2860 {
                tunnel: w2858 -> [w2861 _]
                tunnel: [w2861 w2862] -> w2859
                frame Default {
                }
                frame 56 {
                  w2862 = errorcluster {"status"=FALSE, "code"=0, "source"=""}  # No error
                }
              }
            }
          }
          n1305 = Select(t=errorcluster {"status"=TRUE, "code"=5001, "source"=""} ("error in (no error)"), s=w2831, f=errorcluster {"status"=FALSE, "code"=0, "source"=""} ("error in (no error)")) -> (s? t:f=w2826:errorcluster)
          n1306 = Merge Errors(w2827, w2826) -> (w2825:errorcluster)
        }
        n1307 = Unbundle By Name(w2812) -> ("code"=w2815:i32)
        n1308 = Bundle By Name(cluster=w2817, "System Status.TCP/IP"=w2816, "listener ID"=w2810) -> (w2822:T23)
        n1309 = global write "GlobalVariables.vi" "TCP connected?"(w2816) -> ()
        n1310 = Equal To 0?(x=w2815) -> (x = 0?=w2814:bool)
        n1311 = Select(t=errorcluster {"status"=FALSE, "code"=0, "source"=""} ("error in (no error)"), s=w2814, f=w2812) -> (s? t:f=w2811:errorcluster)
        n1312 = call <vilib>:"Add State(s) to Queue__JKI_lib_State_Machine.vi"("State(s) in (\"\")"=w2824) -> ("States Out"=w2823:string)  [unwired: 14 in]
      }
      frame "TCP: checkSource" {
        # "Check visualization PC video source\n(send !video_source message, listen for response, then parse it to binary mask)"
        n1313 = Unbundle By Name(w2869) -> ("System Status.TCP/IP"=w2872:bool)
        n1314 = case shown="True" w2872 {
          tunnel: w2871 -> [w2877 w2900]
          tunnel: [w2877 w2884] -> w2870
          tunnel: [w2876 w2889] -> w2867
          tunnel: [w2876 w2887] -> w2866
          tunnel: [w2876 w2888] -> w2865
          tunnel: [w2876 w2886] -> w2864
          tunnel: [w2876 w2878] -> w2863
          frame False {
            w2876 = FALSE
          }
          frame True {
            n1315 = call "TcpIDFGV.vi"("Error In"=w2900, "action"=enum16{"write", "read"}."read") -> ("Error Out"=w2897:errorcluster, "connection ID out"=w2899:refnum<k5>)  [unwired: 8 in]
            n1316 = call "TCP_WriteRead.vi"("error in (no error)"=w2897, "data in"="!video_source", "connectin ID in"=w2899) -> ("error out"=w2894:errorcluster, "data out"=w2896:string)  [unwired: 4 in, 1 out]
            n1317 = Scan From String(format string="!video_source:%d", input string=w2896, error in=w2894) -> (error out=w2885:errorcluster, output 1=w2883:i32)  [unwired: 2 in, 2 out]
            n1318 = case shown="5..7, 9..11, 13..15" w2883 {
              tunnel: w2885 -> [_ _ _ _]
              tunnel: [errorcluster {"status"=TRUE, "code"=5007, "source"="Visualization PC"} ("error out") errorcluster {"status"=FALSE, "code"=0, "source"=""} ("error out") errorcluster {"status"=FALSE, "code"=0, "source"=""} ("error out") errorcluster {"status"=FALSE, "code"=0, "source"=""} ("error out")] -> w2884
              tunnel: [FALSE FALSE FALSE TRUE] -> w2878
              frame 0, Default {
                # "No video source available or default"
                n1319 = property on="Video Source" class="RadioBtnsControl (strict)"("DisabledEnum"=T11."Disabled and Grayed Out" ("Disabled")) -> ()  [unwired: 2 in, 2 out]
              }
              frame 1..3 {
                # "one or both camera available"
                n1320 = local write "Video Source"(enum32{"Camera", "FrameGrabber"}."Camera" ("Video Source")) -> ()
                n1321 = property on="Video Source" class="RadioBtnsControl (strict)"("DisabledEnum"=T11."Disabled and Grayed Out" ("Disabled")) -> ()  [unwired: 2 in, 2 out]
              }
              frame 4, 8, 12 {
                # "one or both frame grabber available"
                n1322 = local write "Video Source"(enum32{"Camera", "FrameGrabber"}."FrameGrabber" ("Video Source")) -> ()
                n1323 = property on="Video Source" class="RadioBtnsControl (strict)"("DisabledEnum"=T11."Disabled and Grayed Out" ("Disabled")) -> ()  [unwired: 2 in, 2 out]
              }
              frame 5..7, 9..11, 13..15 {
                n1324 = property on="Video Source" class="RadioBtnsControl (strict)"("DisabledEnum"=T11."Enabled" ("Disabled")) -> ()  [unwired: 2 in, 2 out]
              }
            }
            n1325 = Integer to Fixed-Point Cast(fixed-point type=fxp<+,4,4> 0.0, integer=w2883) -> (fixed-point=w2882:fxp<+,4,4>)
            n1326 = Number To Boolean Array(number=w2882) -> (Boolean array=w2880:bool[])
            n1327 = Reverse 1D Array(array=w2880) -> (reversed array=w2879:bool[])
            n1328 = Index Array(array=w2879, index=0) -> (element=w2889:bool)
            n1329 = Index Array(array=w2879, index=1) -> (element=w2887:bool)
            n1330 = Index Array(array=w2879, index=2) -> (element=w2888:bool)
            n1331 = Index Array(array=w2879, index=3) -> (element=w2886:bool)
          }
        }
        n1332 = Bundle By Name(cluster=w2869, "video source.Main Frame Grabber"=w2867, "video source.Side Frame Grabber"=w2866, "video source.Main Camera"=w2865, "video source.Side Camera"=w2864, "bothVidSourceAvail"=w2863) -> (w2868:T23)
        n1333 = call <vilib>:"Add State(s) to Queue__JKI_lib_State_Machine.vi"("State(s) in (\"\")"=w2875) -> ("States Out"=w2874:string)  [unwired: 14 in]
      }
      frame "TCP: SyncTime" {
        # "Template Separator\n(You can make a copy of, or modify, this frame)"
        n1334 = Unbundle By Name(w2917) -> ("System Status.TCP/IP"=w2916:bool)
        n1335 = case shown="True" w2916 {
          tunnel: w2918 -> [_ w2926]
          frame False {
          }
          frame True {
            n1336 = call "TcpIDFGV.vi"("Error In"=w2926, "action"=enum16{"write", "read"}."read") -> ("Error Out"=w2925:errorcluster, "connection ID out"=w2922:refnum<k5>)  [unwired: 8 in]
            n1337 = call <userlib>:"Tick Count (ms)__ogtk.vi"("error in (no error)"=w2925) -> ("error out"=w2924:errorcluster, "millisecond timer value"=w2923:u32)  [unwired: 9 in]
            n1338 = while {
              tunnel: w2924 -> [w2946]
              tunnel: w2922 -> [w2945]
              tunnel: w2923 -> [w2934]
              stop <- w2929 stop-if-true
              n1339 = Concatenate Strings("latencycheck" ("string"), "\r\n" ("End of Line Constant")) -> (w2941:string)
              n1340 = TCP Read(connection ID=w2945, bytes to read=512, error in (no error)=w2946, 7:T21."CRLF" ("mode (standard)"), 9:2000 ("timeout ms (25000)")) -> (connection ID out=w2938:refnum<k5>, data out=w2936:string, error out=w2928:errorcluster)
              n1341 = Tick Count (ms)() -> (millisecond timer value=w2935:u32)
              n1342 = Subtract(x=w2935, y=w2934) -> (x-y=w2933:u32)
              n1343 = Equal?(x=w2936, y=w2941) -> (x = y?=w2937:bool)
              n1344 = case shown="True" w2937 {
                tunnel: w2938 -> [_ w2959]
                tunnel: w2936 -> [w2951 _]
                tunnel: [w2947 FALSE] -> w2931
                tunnel: w2928 -> [_ w2953]
                frame False {
                  n1345 = Concatenate Strings("synctimer" ("string"), "\r\n" ("End of Line Constant")) -> (w2948:string)
                  n1346 = Equal?(x=w2951, y=w2948) -> (x = y?=w2947:bool)
                  "Sync Success?" <- w2947
                }
                frame True {
                  n1347 = Concatenate Strings("latencycheck:" ("string"), "\r\n" ("End of Line Constant")) -> (w2958:string)
                  n1348 = TCP Write(connection ID=w2959, data in=w2958, error in (no error)=w2953, 9:1000 ("timeout ms (25000)")) -> (error out=w2952:errorcluster)  [unwired: 2 out]
                  n1349 = call <vilib>:"Clear Errors.vi"("error in (no error)"=w2952) -> ()  [unwired: 5 in, 2 out]
                }
              }
              n1350 = Greater?(x=w2933, y=u32 10000 ("x-y")) -> (0:w2930:bool)
              n1351 = Or(x=w2931, y=w2930) -> (x .or. y?=w2929:bool)
            }
          }
        }
        n1352 = call <vilib>:"Add State(s) to Queue__JKI_lib_State_Machine.vi"("State(s) in (\"\")"=w2921) -> ("States Out"=w2920:string)  [unwired: 14 in]
      }
      frame "TCP: SendSettingMacro" {
        # "Template Separator\n(You can make a copy of, or modify, this frame)"
        n1353 = Unbundle By Name(w2963) -> ("System Status.TCP/IP"=w2962:bool)
        n1354 = case shown="True" w2962 {
          tunnel: ["" ("Empty String Constant") "TCP: sendSubjectID\nTCP: sendScaleBarSetting\nTCP: sendScaleMaxMin\nTCP: sendDeconChannel\nTCP: sendANSI\nTCP: sendRadius\nTCP: send3Dsetting\nTCP: sendFirefly\nTCP: sendPentero"] -> w2961
          frame False {
          }
          frame True {
          }
        }
        n1355 = call <vilib>:"Add State(s) to Queue__JKI_lib_State_Machine.vi"("State(s) in Front (\"\")"=w2961, "State(s) in (\"\")"=w2966) -> ("States Out"=w2965:string)  [unwired: 13 in]
      }
      frame "TCP: sendRunNum" {
        # "Send run number to AB PC\n(You can make a copy of, or modify, this frame)"
        n1356 = Unbundle By Name(w2973) -> ("System Status.TCP/IP"=w2970:bool, "IDs.RunID"=w2974:i8)
        n1357 = Increment(x=w2974) -> (x+1=w2969:i8)
        n1358 = case shown="True" w2970 {
          tunnel: w2969 -> [_ w2988]
          tunnel: [w2978 w2980] -> w2972
          tunnel: w2971 -> [w2978 w2979]
          frame False {
          }
          frame True {
            n1359 = Number To Decimal String(number=w2988, width (-)=i16 3) -> (decimal integer string=w2983:string)
            n1360 = call "TcpIDFGV.vi"("Error In"=w2979, "action"=enum16{"write", "read"}."read") -> ("Error Out"=w2981:errorcluster, "connection ID out"=w2985:refnum<k5>)  [unwired: 8 in]
            n1361 = Concatenate Strings("!run:", w2983) -> (w2982:string)
            n1362 = call "TCP_WriteRead.vi"("error in (no error)"=w2981, "data in"=w2982, "connectin ID in"=w2985) -> ("error out"=w2980:errorcluster)  [unwired: 4 in, 2 out]
          }
        }
        n1363 = call <vilib>:"Add State(s) to Queue__JKI_lib_State_Machine.vi"("State(s) in (\"\")"=w2977) -> ("States Out"=w2976:string)  [unwired: 14 in]
      }
      frame "TCP: sendVideoSource" {
        # "Send video source \n(You can make a copy of, or modify, this frame)"
        n1364 = Unbundle By Name(w2990) -> ("System Status.TCP/IP"=w2989:bool)
        n1365 = case shown="True" w2989 {
          tunnel: [w2996 w2998] -> w2992
          tunnel: w2991 -> [w2996 w2997]
          frame False {
          }
          frame True {
            n1366 = case shown="\"Camera\", Default" "Video Source" {
              tunnel: [0 1] -> w3003
              frame "Camera", Default {
              }
              frame "FrameGrabber" {
              }
            }
            n1367 = call "TcpIDFGV.vi"("Error In"=w2997, "action"=enum16{"write", "read"}."read") -> ("Error Out"=w2999:errorcluster, "connection ID out"=w3005:refnum<k5>)  [unwired: 8 in]
            n1368 = Number To Decimal String(number=w3003) -> (decimal integer string=w3001:string)  [unwired: 1 in]
            n1369 = Concatenate Strings("!invivo:" ("data in"), w3001) -> (w3000:string)
            n1370 = call "TCP_WriteRead.vi"("error in (no error)"=w2999, "data in"=w3000, "connectin ID in"=w3005) -> ("error out"=w2998:errorcluster)  [unwired: 4 in, 2 out]
          }
        }
        n1371 = call <vilib>:"Add State(s) to Queue__JKI_lib_State_Machine.vi"("State(s) in (\"\")"=w2995) -> ("States Out"=w2994:string)  [unwired: 14 in]
      }
      frame "TCP: startRun" {
        # "Template Separator\n(You can make a copy of, or modify, this frame)"
        n1372 = Unbundle By Name(w3010) -> ("System Status.TCP/IP"=w3009:bool)
        n1373 = case shown="True" w3009 {
          tunnel: [w3016 w3018] -> w3012
          tunnel: w3011 -> [w3016 w3017]
          frame False {
          }
          frame True {
            n1374 = call "TcpIDFGV.vi"("Error In"=w3017, "action"=enum16{"write", "read"}."read") -> ("Error Out"=w3019:errorcluster, "connection ID out"=w3020:refnum<k5>)  [unwired: 8 in]
            n1375 = call "TCP_WriteRead.vi"("error in (no error)"=w3019, "data in"="!acquire:1", "connectin ID in"=w3020) -> ("error out"=w3018:errorcluster)  [unwired: 4 in, 2 out]
          }
        }
        n1376 = call <vilib>:"Add State(s) to Queue__JKI_lib_State_Machine.vi"("State(s) in (\"\")"=w3015) -> ("States Out"=w3014:string)  [unwired: 14 in]
      }
      frame "TCP: stopRun" {
        # "Send stop run to AB PC\n(You can make a copy of, or modify, this frame)"
        n1377 = Unbundle By Name(w3024) -> ("System Status.TCP/IP"=w3023:bool)
        n1378 = case shown="True" w3023 {
          tunnel: [w3030 w3032] -> w3026
          tunnel: w3025 -> [w3030 w3031]
          frame False {
            # "if not connected, do nothing"
          }
          frame True {
            # "If TCP connected, send stop run"
            n1379 = call "TcpIDFGV.vi"("Error In"=w3031, "action"=enum16{"write", "read"}."read") -> ("Error Out"=w3033:errorcluster, "connection ID out"=w3035:refnum<k5>)  [unwired: 8 in]
            n1380 = call "TCP_WriteRead.vi"("error in (no error)"=w3033, "data in"="!acquire:0", "connectin ID in"=w3035) -> ("error out"=w3032:errorcluster)  [unwired: 4 in, 2 out]
          }
        }
        n1381 = call <vilib>:"Add State(s) to Queue__JKI_lib_State_Machine.vi"("State(s) in (\"\")"=w3029) -> ("States Out"=w3028:string)  [unwired: 14 in]
      }
      frame "TCP: CheckConnection" {
        # "Check TCP/IP connection statuse\n(If connection is lost, throw error)"
        n1382 = Unbundle By Name(w3038) -> ("System Status.TCP/IP"=w3037:bool)
        n1383 = case shown="False" w3037 {
          frame False {
          }
          frame True {
            # "If TCP/IP is true check, otherwise skip"
          }
        }
        n1384 = call <vilib>:"Add State(s) to Queue__JKI_lib_State_Machine.vi"("State(s) in (\"\")"=w3042) -> ("States Out"=w3041:string)  [unwired: 14 in]
      }
      frame "TCP: sendSubjectID" {
        # "Send subject ID"
        n1385 = Unbundle By Name(w3044) -> ("System Status.TCP/IP"=w3043:bool, "CaseID"=w3047:string)
        n1386 = case shown="True" w3043 {
          tunnel: w3047 -> [_ w3058]
          tunnel: [w3051 w3053] -> w3046
          tunnel: w3045 -> [w3051 w3052]
          frame False {
          }
          frame True {
            n1387 = call "TcpIDFGV.vi"("Error In"=w3052, "action"=enum16{"write", "read"}."read") -> ("Error Out"=w3054:errorcluster, "connection ID out"=w3056:refnum<k5>)  [unwired: 8 in]
            n1388 = Concatenate Strings("!subject:", w3058) -> (w3055:string)
            n1389 = call "TCP_WriteRead.vi"("error in (no error)"=w3054, "data in"=w3055, "connectin ID in"=w3056) -> ("error out"=w3053:errorcluster)  [unwired: 4 in, 2 out]
          }
        }
        n1390 = call <vilib>:"Add State(s) to Queue__JKI_lib_State_Machine.vi"("State(s) in (\"\")"=w3050) -> ("States Out"=w3049:string)  [unwired: 14 in]
      }
      frame "TCP: sendScaleBarSetting" {
        # "Template Separator\n(You can make a copy of, or modify, this frame)"
        n1391 = Unbundle By Name(w3062) -> ("System Status.TCP/IP"=w3060:bool, "VideoConfig.Scale Bar"=w3061:bool)
        n1392 = case shown="True" w3060 {
          tunnel: [w3068 w3077] -> w3064
          tunnel: w3063 -> [w3068 w3076]
          tunnel: w3061 -> [_ w3075]
          frame False {
          }
          frame True {
            n1393 = Boolean To (0,1)(Boolean=w3075) -> (0, 1=w3074:i16)
            n1394 = call "TcpIDFGV.vi"("Error In"=w3076, "action"=enum16{"write", "read"}."read") -> ("Error Out"=w3078:errorcluster, "connection ID out"=w3079:refnum<k5>)  [unwired: 8 in]
            n1395 = Number To Fractional String(number=w3074, width (-)=i16 1, precision (6)=i16 0) -> (F-format string=w3072:string)  [unwired: 1 in]
            n1396 = Concatenate Strings("!autocolor:" ("data in"), w3072) -> (w3070:string)
            n1397 = call "TCP_WriteRead.vi"("error in (no error)"=w3078, "data in"=w3070, "connectin ID in"=w3079) -> ("error out"=w3077:errorcluster)  [unwired: 4 in, 2 out]
          }
        }
        n1398 = call <vilib>:"Add State(s) to Queue__JKI_lib_State_Machine.vi"("State(s) in (\"\")"=w3067) -> ("States Out"=w3066:string)  [unwired: 14 in]
      }
      frame "TCP: sendScaleMaxMin" {
        # "Send scale bar max and min to AB PC\n(You can make a copy of, or modify, this frame)"
        n1399 = Unbundle By Name(w3084) -> ("System Status.TCP/IP"=w3081:bool, "VideoConfig.Scale Low"=w3083:dbl, "VideoConfig.Scale High"=w3082:dbl)
        n1400 = case shown="True" w3081 {
          tunnel: [w3090 w3103] -> w3086
          tunnel: w3085 -> [w3090 w3102]
          tunnel: w3083 -> [_ w3101]
          tunnel: w3082 -> [_ w3092]
          frame False {
          }
          frame True {
            n1401 = call "TcpIDFGV.vi"("Error In"=w3102, "action"=enum16{"write", "read"}."read") -> ("Error Out"=w3104:errorcluster, "connection ID out"=w3105:refnum<k5>)  [unwired: 8 in]
            n1402 = Number To Fractional String(number=w3101, width (-)=i16 4, precision (6)=i16 2) -> (F-format string=w3097:string)  [unwired: 1 in]
            n1403 = Number To Fractional String(number=w3092, width (-)=i16 4, precision (6)=i16 2) -> (F-format string=w3093:string)  [unwired: 1 in]
            n1404 = Concatenate Strings("!color:" ("string"), w3097, ";" ("string"), w3093) -> (w3091:string)
            n1405 = call "TCP_WriteRead.vi"("error in (no error)"=w3104, "data in"=w3091, "connectin ID in"=w3105) -> ("error out"=w3103:errorcluster)  [unwired: 4 in, 2 out]
          }
        }
        n1406 = call <vilib>:"Add State(s) to Queue__JKI_lib_State_Machine.vi"("State(s) in (\"\")"=w3089) -> ("States Out"=w3088:string)  [unwired: 14 in]
      }
      frame "TCP: sendDeconChannel" {
        # "Send Decon channel\n(You can make a copy of, or modify, this frame)"
        n1407 = Unbundle By Name(w3108) -> ("System Status.TCP/IP"=w3107:bool)
        n1408 = case shown="True" w3107 {
          tunnel: [w3114 w3119] -> w3110
          tunnel: w3109 -> [w3114 w3118]
          frame False {
          }
          frame True {
            n1409 = local read "Radio Buttons"() -> (w3117:T9)
            n1410 = Increment(x=w3117) -> (x+1=w3116:T9)
            n1411 = Number To Decimal String(number=w3116) -> (decimal integer string=w3115:string)  [unwired: 1 in]
            n1412 = call "TcpIDFGV.vi"("Error In"=w3118, "action"=enum16{"write", "read"}."read") -> ("Error Out"=w3120:errorcluster, "connection ID out"=w3123:refnum<k5>)  [unwired: 8 in]
            n1413 = Concatenate Strings("!channel:", w3115) -> (w3121:string)
            n1414 = call "TCP_WriteRead.vi"("error in (no error)"=w3120, "data in"=w3121, "connectin ID in"=w3123) -> ("error out"=w3119:errorcluster)  [unwired: 4 in, 2 out]
          }
        }
        n1415 = call <vilib>:"Add State(s) to Queue__JKI_lib_State_Machine.vi"("State(s) in (\"\")"=w3113) -> ("States Out"=w3112:string)  [unwired: 14 in]
      }
      frame "TCP: sendANSI" {
        # "Template Separator\n(You can make a copy of, or modify, this frame)"
        n1416 = Unbundle By Name(w3127) -> ("System Status.TCP/IP"=w3125:bool, "VideoConfig.ANSI"=w3126:dbl)
        n1417 = case shown="True" w3125 {
          tunnel: [w3133 w3139] -> w3129
          tunnel: w3128 -> [w3133 w3138]
          tunnel: w3126 -> [_ w3137]
          frame False {
          }
          frame True {
            n1418 = Number To Fractional String(number=w3137) -> (F-format string=w3135:string)  [unwired: 3 in]
            n1419 = call "TcpIDFGV.vi"("Error In"=w3138, "action"=enum16{"write", "read"}."read") -> ("Error Out"=w3140:errorcluster, "connection ID out"=w3141:refnum<k5>)  [unwired: 8 in]
            n1420 = Concatenate Strings("!ansi:" ("data in"), w3135) -> (w3134:string)
            n1421 = call "TCP_WriteRead.vi"("error in (no error)"=w3140, "data in"=w3134, "connectin ID in"=w3141) -> ("error out"=w3139:errorcluster)  [unwired: 4 in, 2 out]
          }
        }
        n1422 = call <vilib>:"Add State(s) to Queue__JKI_lib_State_Machine.vi"("State(s) in (\"\")"=w3132) -> ("States Out"=w3131:string)  [unwired: 14 in]
      }
      frame "TCP: sendRadius" {
        # "Send drawing radius to AB PC\n(You can make a copy of, or modify, this frame)"
        n1423 = Unbundle By Name(w3145) -> ("System Status.TCP/IP"=w3143:bool, "VideoConfig.Radius"=w3144:dbl)
        n1424 = case shown="True" w3143 {
          tunnel: [w3151 w3157] -> w3147
          tunnel: w3146 -> [w3151 w3156]
          tunnel: w3144 -> [_ w3155]
          frame False {
          }
          frame True {
            n1425 = Number To Fractional String(number=w3155) -> (F-format string=w3154:string)  [unwired: 3 in]
            n1426 = Concatenate Strings("!radius:" ("data in"), w3154) -> (w3152:string)
            n1427 = call "TcpIDFGV.vi"("Error In"=w3156, "action"=enum16{"write", "read"}."read") -> ("Error Out"=w3158:errorcluster, "connection ID out"=w3159:refnum<k5>)  [unwired: 8 in]
            n1428 = call "TCP_WriteRead.vi"("error in (no error)"=w3158, "data in"=w3152, "connectin ID in"=w3159) -> ("error out"=w3157:errorcluster)  [unwired: 4 in, 2 out]
          }
        }
        n1429 = call <vilib>:"Add State(s) to Queue__JKI_lib_State_Machine.vi"("State(s) in (\"\")"=w3150) -> ("States Out"=w3149:string)  [unwired: 14 in]
      }
      frame "TCP: send3Dsetting" {
        # "Send 3D setting to AB computer\n(You can make a copy of, or modify, this frame)"
        n1430 = Unbundle By Name(w3163) -> ("System Status.TCP/IP"=w3161:bool, "VideoConfig.3D?"=w3162:bool)
        n1431 = case shown="True" w3161 {
          tunnel: [w3169 w3176] -> w3165
          tunnel: w3164 -> [w3169 w3175]
          tunnel: w3162 -> [_ w3174]
          frame False {
          }
          frame True {
            n1432 = Boolean To (0,1)(Boolean=w3174) -> (0, 1=w3173:i16)
            n1433 = Number To Fractional String(number=w3173) -> (F-format string=w3172:string)  [unwired: 3 in]
            n1434 = call "TcpIDFGV.vi"("Error In"=w3175, "action"=enum16{"write", "read"}."read") -> ("Error Out"=w3177:errorcluster, "connection ID out"=w3178:refnum<k5>)  [unwired: 8 in]
            n1435 = Concatenate Strings("!3dset:" ("data in"), w3172) -> (w3170:string)
            n1436 = call "TCP_WriteRead.vi"("error in (no error)"=w3177, "data in"=w3170, "connectin ID in"=w3178) -> ("error out"=w3176:errorcluster)  [unwired: 4 in, 2 out]
          }
        }
        n1437 = call <vilib>:"Add State(s) to Queue__JKI_lib_State_Machine.vi"("State(s) in (\"\")"=w3168) -> ("States Out"=w3167:string)  [unwired: 14 in]
      }
      frame "TCP: sendFirefly" {
        # "Template Separator\n(You can make a copy of, or modify, this frame)"
        n1438 = Unbundle By Name(w3181) -> ("System Status.TCP/IP"=w3180:bool)
        n1439 = case shown="False" w3180 {
          tunnel: [w3187 w3189] -> w3183
          tunnel: w3182 -> [w3187 w3188]
          frame False {
          }
          frame True {
            n1440 = call "TcpIDFGV.vi"("Error In"=w3188, "action"=enum16{"write", "read"}."read") -> ("Error Out"=w3190:errorcluster, "connection ID out"=w3192:refnum<k5>)  [unwired: 8 in]
            n1441 = call "TCP_WriteRead.vi"("error in (no error)"=w3190, "data in"="!firefly:0", "connectin ID in"=w3192) -> ("error out"=w3189:errorcluster)  [unwired: 4 in, 2 out]
          }
        }
        n1442 = call <vilib>:"Add State(s) to Queue__JKI_lib_State_Machine.vi"("State(s) in (\"\")"=w3186) -> ("States Out"=w3185:string)  [unwired: 14 in]
      }
      frame "TCP: sendPentero" {
        # "Send Pentero setting to AB computer\n(You can make a copy of, or modify, this frame)"
        n1443 = Unbundle By Name(w3195) -> ("System Status.TCP/IP"=w3194:bool)
        n1444 = case shown="True" w3194 {
          tunnel: [w3201 w3203] -> w3197
          tunnel: w3196 -> [w3201 w3202]
          frame False {
          }
          frame True {
            n1445 = call "TcpIDFGV.vi"("Error In"=w3202, "action"=enum16{"write", "read"}."read") -> ("Error Out"=w3204:errorcluster, "connection ID out"=w3206:refnum<k5>)  [unwired: 8 in]
            n1446 = call "TCP_WriteRead.vi"("error in (no error)"=w3204, "data in"="!pentero:0", "connectin ID in"=w3206) -> ("error out"=w3203:errorcluster)  [unwired: 4 in, 2 out]
          }
        }
        n1447 = call <vilib>:"Add State(s) to Queue__JKI_lib_State_Machine.vi"("State(s) in (\"\")"=w3200) -> ("States Out"=w3199:string)  [unwired: 14 in]
      }
      frame "TCP: sendChannel" {
        # "Send DeCon Channel to AB computer\n()"
        n1448 = Unbundle By Name(w3209) -> ("System Status.TCP/IP"=w3208:bool)
        n1449 = case shown="True" w3208 {
          tunnel: [w3215 w3219] -> w3211
          tunnel: w3210 -> [w3215 w3218]
          frame False {
          }
          frame True {
            n1450 = local read "Radio Buttons"() -> (w3217:T9)
            n1451 = case shown="\"No Selection\", Default" w3217 {
              tunnel: ["" ("data in") "!channel:1" ("data in") "!channel:2" ("data in") "!channel:3" ("data in")] -> w3216
              frame "No Selection", Default {
              }
              frame "Ch1" {
              }
              frame "Ch2" {
              }
              frame "Ch3" {
              }
            }
            n1452 = call "TcpIDFGV.vi"("Error In"=w3218, "action"=enum16{"write", "read"}."read") -> ("Error Out"=w3220:errorcluster, "connection ID out"=w3221:refnum<k5>)  [unwired: 8 in]
            n1453 = call "TCP_WriteRead.vi"("error in (no error)"=w3220, "data in"=w3216, "connectin ID in"=w3221) -> ("error out"=w3219:errorcluster)  [unwired: 4 in, 2 out]
          }
        }
        n1454 = call <vilib>:"Add State(s) to Queue__JKI_lib_State_Machine.vi"("State(s) in (\"\")"=w3214) -> ("States Out"=w3213:string)  [unwired: 14 in]
      }
      frame "TCP: startCam" {
        # "Send Pentero setting to AB computer\n(You can make a copy of, or modify, this frame)"
        n1455 = Unbundle By Name(w3228) -> ("System Status.TCP/IP"=w3227:bool)
        n1456 = case shown="True" w3227 {
          tunnel: [w3234 w3236] -> w3230
          tunnel: w3229 -> [w3234 w3235]
          frame False {
          }
          frame True {
            n1457 = call "TcpIDFGV.vi"("Error In"=w3235, "action"=enum16{"write", "read"}."read") -> ("Error Out"=w3237:errorcluster, "connection ID out"=w3239:refnum<k5>)  [unwired: 8 in]
            n1458 = call "TCP_WriteRead.vi"("error in (no error)"=w3237, "data in"="!focus:1", "connectin ID in"=w3239) -> ("error out"=w3236:errorcluster)  [unwired: 4 in, 2 out]
          }
        }
        n1459 = call <vilib>:"Add State(s) to Queue__JKI_lib_State_Machine.vi"("State(s) in (\"\")"=w3233) -> ("States Out"=w3232:string)  [unwired: 14 in]
      }
      frame "TCP: stopCam" {
        # "Send Pentero setting to AB computer\n(You can make a copy of, or modify, this frame)"
        n1460 = Unbundle By Name(w3242) -> ("System Status.TCP/IP"=w3241:bool)
        n1461 = case shown="True" w3241 {
          tunnel: [w3248 w3250] -> w3244
          tunnel: w3243 -> [w3248 w3249]
          frame False {
          }
          frame True {
            n1462 = call "TcpIDFGV.vi"("Error In"=w3249, "action"=enum16{"write", "read"}."read") -> ("Error Out"=w3251:errorcluster, "connection ID out"=w3253:refnum<k5>)  [unwired: 8 in]
            n1463 = call "TCP_WriteRead.vi"("error in (no error)"=w3251, "data in"="!focus:0", "connectin ID in"=w3253) -> ("error out"=w3250:errorcluster)  [unwired: 4 in, 2 out]
          }
        }
        n1464 = call <vilib>:"Add State(s) to Queue__JKI_lib_State_Machine.vi"("State(s) in (\"\")"=w3247) -> ("States Out"=w3246:string)  [unwired: 14 in]
      }
      frame "TCP: Close" {
        # "Close TCP connection\n()"
        n1465 = Unbundle By Name(w3257) -> ("System Status.TCP/IP"=w3255:bool)
        n1466 = case shown="True" w3255 {
          tunnel: [w3263 w3265] -> w3258
          tunnel: w3256 -> [w3263 w3264]
          frame False {
          }
          frame True {
            n1467 = call "TcpIDFGV.vi"("Error In"=w3264, "action"=enum16{"write", "read"}."read") -> ("Error Out"=w3267:errorcluster, "connection ID out"=w3268:refnum<k5>)  [unwired: 8 in]
            n1468 = TCP Close Connection(connection ID=w3268, error in (no error)=w3267) -> (error out=w3265:errorcluster)  [unwired: 1 in, 1 out]
          }
        }
        n1469 = case shown="Error .." w3258 {
          tunnel: [w3271 w3272] -> w3259
          tunnel: w3257 -> [w3270 w3272]
          frame No Error {
            w3269 = FALSE ("System Status.TCP/IP")
            n1470 = Bundle By Name(cluster=w3270, "System Status.TCP/IP"=w3269) -> (w3271:T23)
            n1471 = global write "GlobalVariables.vi" "TCP connected?"(w3269) -> ()
          }
          frame Error {
          }
        }
        n1472 = call <vilib>:"Add State(s) to Queue__JKI_lib_State_Machine.vi"("State(s) in (\"\")"=w3262) -> ("States Out"=w3261:string)  [unwired: 14 in]
      }
      frame "---------- PID ----------" {
        # "Template Separator\n(You can make a copy of, or modify, this frame)"
        n1473 = call <vilib>:"Add State(s) to Queue__JKI_lib_State_Machine.vi"("State(s) in (\"\")"=w3277) -> ("States Out"=w3276:string)  [unwired: 14 in]
      }
      frame "PID: loadPID" {
        # "Template Separator\n(You can make a copy of, or modify, this frame)"
        n1474 = call "readPIDSetting.vi"("Error In"=w3281) -> ("Error Out"=w3282:errorcluster, "Ch3 PID out"=w3278:T8, "Ch2 PID out"=w3279:T8, "Ch1 PID out"=w3280:T8)  [unwired: 7 in]
        n1475 = local write "Ch1 PID gains"(w3280) -> ()
        n1476 = local write "Ch2 PID gains"(w3279) -> ()
        n1477 = local write "Ch3 PID gains"(w3278) -> ()
        n1478 = local write "Ch4 PID gains"(w3278) -> ()
        n1479 = call <vilib>:"Add State(s) to Queue__JKI_lib_State_Machine.vi"("State(s) in (\"\")"=w3286) -> ("States Out"=w3285:string)  [unwired: 14 in]
      }
      frame "---------- Temp ----------" {
        # "Template Separator\n(You can make a copy of, or modify, this frame)"
        n1480 = call <vilib>:"Add State(s) to Queue__JKI_lib_State_Machine.vi"("State(s) in (\"\")"=w3291) -> ("States Out"=w3290:string)  [unwired: 14 in]
      }
    }
    n1481 = Not(x=w80) -> (.not. x?=w79:bool)
    n1482 = local write "ML?"(w79) -> ()
    "ML?" <- TRUE ("main loop running?")
  }
  n1483 = while {
    tunnel: w19 -> [w3330]
    tunnel: w18 -> [w3325]
    tunnel: [w3324] -> w17
    tunnel: w13 -> [w3318]
    tunnel: [w3317] -> w16
    shift-right: [w3309] -> _
    shift-left: _ -> [w3310]
    stop <- w3305 stop-if-true
    # "Read data from notifier and deconvolve it and send to Aiming Beam computer"
    n1484 = Wait on Notification(notifier=w3330, ignore previous (F)=TRUE) -> (notification=w3329:T14, error out=w3321:errorcluster)  [unwired: 2 in, 2 out]
    n1485 = Wait Until Next ms Multiple(millisecond multiple=u32 10) -> ()  [unwired: 1 out]
    n1486 = Unbundle(w3329) -> ("idx"=w3295:i32, "CH1&2"=w3328:dbl[][], "CH3"=w3327:dbl[][], "V cluster"=w3313:cluster{"V1":dbl, "V2":dbl, "V3":dbl, "V4":dbl})
    n1487 = call <vilib>:"High Resolution Relative Seconds.vi"() -> ("relative seconds"=w3309:dbl)
    n1488 = call "SeperateChanData.vi"("Input (Ch1&2)"=w3328) -> ("Ch1"=w3301:dbl[][], "Ch2"=w3299:dbl[][])
    n1489 = call "SeperateChanData.vi"("Input (Ch1&2)"=w3327) -> ("Ch1"=w3297:dbl[][], "Ch2"=w3294:dbl[][])
    n1490 = Subtract(x=w3309, y=w3310) -> (x-y=w3312:dbl)
    n1491 = call "AvgArrayTimeCritical.vi"("2D array"=w3301) -> ("1D Avg"=w3300:dbl[])  [unwired: 10 in]
    n1492 = call "AvgArrayTimeCritical.vi"("2D array"=w3299) -> ("1D Avg"=w3298:dbl[])  [unwired: 10 in]
    n1493 = call "AvgArrayTimeCritical.vi"("2D array"=w3297) -> ("1D Avg"=w3296:dbl[])  [unwired: 10 in]
    n1494 = call "AvgArrayTimeCritical.vi"("2D array"=w3294) -> ("1D Avg"=w3293:dbl[])  [unwired: 10 in]
    n1495 = Multiply(x=w3312, y=1000.0) -> (x*y=→"Decon Loop timing (ms)":dbl)
    n1496 = case shown="\"Ch1\"" "Radio Buttons" {
      selector: "Radio Buttons" -> [_ w3343 w3357 w3372 w3389]
      tunnel: w3300 -> [w3340 w3351 w3363 w3377 w3393]
      tunnel: w3298 -> [w3338 w3348 w3365 w3375 w3391]
      tunnel: w3296 -> [w3336 w3346 w3360 w3380 w3383]
      tunnel: FALSE -> [_ w3354 w3368 w3382 w3396]
      tunnel: w3321 -> [w3334 w3353 w3367 w3371 w3388]
      tunnel: [w3334 w3352 w3366 w3381 w3395] -> w3305
      tunnel: [w3339 w3349 w3361 w3376 w3392] -> w3316
      tunnel: [w3337 w3347 w3362 w3374 w3390] -> w3315
      tunnel: [w3335 w3345 w3359 w3378 w3384] -> w3314
      tunnel: [0.0 ("lifetime (ns)") w3344 w3358 w3373 w3387] -> w3320
      tunnel: w3293 -> [w3332 w3342 w3356 w3370 w3386]
      tunnel: [w3331 w3341 w3355 w3369 w3385] -> w3292
      frame "No Selection", Default {
        n1497 = Build Array(w3340) -> (w3339:dbl[][])
        n1498 = Build Array(w3338) -> (w3337:dbl[][])
        n1499 = Build Array(w3336) -> (w3335:dbl[][])
        n1500 = Build Array(w3332) -> (w3331:dbl[][])
      }
      frame "Ch1" {
        n1501 = call "Deconvolution.vi"("DeconChannel"=w3343, "iRF align"=w3354, "error in (no error)"=w3353, "Waveform"=w3351) -> ("error out"=w3352:errorcluster, "lifetime (ns)"=w3344:dbl, "Fitting"=w3350:dbl[])  [unwired: 5 in]
        "Lifetime 1" <- w3344
        n1502 = Build Array(w3351, w3350) -> (w3349:dbl[][])
        n1503 = Build Array(w3348) -> (w3347:dbl[][])
        n1504 = Build Array(w3346) -> (w3345:dbl[][])
        n1505 = Build Array(w3342) -> (w3341:dbl[][])
      }
      frame "Ch2" {
        n1506 = call "Deconvolution.vi"("DeconChannel"=w3357, "iRF align"=w3368, "error in (no error)"=w3367, "Waveform"=w3365) -> ("error out"=w3366:errorcluster, "lifetime (ns)"=w3358:dbl, "Fitting"=w3364:dbl[])  [unwired: 5 in]
        "Lifetime 2" <- w3358
        n1507 = Build Array(w3363) -> (w3361:dbl[][])
        n1508 = Build Array(w3365, w3364) -> (w3362:dbl[][])
        n1509 = Build Array(w3360) -> (w3359:dbl[][])
        n1510 = Build Array(w3356) -> (w3355:dbl[][])
      }
      frame "Ch3" {
        n1511 = call "Deconvolution.vi"("DeconChannel"=w3372, "iRF align"=w3382, "error in (no error)"=w3371, "Waveform"=w3380) -> ("error out"=w3381:errorcluster, "lifetime (ns)"=w3373:dbl, "Fitting"=w3379:dbl[])  [unwired: 5 in]
        "Lifetime 3" <- w3373
        n1512 = Build Array(w3377) -> (w3376:dbl[][])
        n1513 = Build Array(w3375) -> (w3374:dbl[][])
        n1514 = Build Array(w3380, w3379) -> (w3378:dbl[][])
        n1515 = Build Array(w3370) -> (w3369:dbl[][])
      }
      frame "Ch4" {
        n1516 = call "Deconvolution.vi"("DeconChannel"=w3389, "iRF align"=w3396, "error in (no error)"=w3388, "Waveform"=w3386) -> ("error out"=w3395:errorcluster, "lifetime (ns)"=w3387:dbl, "Fitting"=w3394:dbl[])  [unwired: 5 in]
        "Lifetime 4" <- w3387
        n1517 = Build Array(w3393) -> (w3392:dbl[][])
        n1518 = Build Array(w3391) -> (w3390:dbl[][])
        n1519 = Build Array(w3386, w3394) -> (w3385:dbl[][])
        n1520 = Build Array(w3383) -> (w3384:dbl[][])
      }
    }
    n1521 = Bundle(w3316, w3315, w3314, w3292, "V cluster"=w3313) -> (w3319:T47)  [unwired: 1 in]
    n1522 = Bundle("idx"=w3295, "lifetime (ns)"=w3320) -> (w3326:cluster{"idx":i32, "lifetime (ns)":dbl})  [unwired: 1 in]
    n1523 = Send Notification(notification=w3319, notifier=w3318, error in (no error)=w3305) -> (notifier out=w3317:refnum<notifier>, error out=w3304:errorcluster)
    n1524 = Send Notification(notification=w3326, notifier=w3325, error in (no error)=w3305) -> (notifier out=w3324:refnum<notifier>, error out=w3303:errorcluster)
    n1525 = Merge Errors(w3304, w3303) -> (→"decon error out":errorcluster)
  }
  n1526 = while {
    tunnel: w18 -> [w3407]
    shift-right: [w3400] -> _
    shift-left: u32 0 -> [w3401]
    stop <- w3398 stop-if-true
    # "Send data to AB computer here"
    # "if TCP ip is not open loop will run once and stop. To re-establish connection and start this loop. Reboot softwrae."
    # "Data communication loop"
    n1527 = Tick Count (ms)() -> (millisecond timer value=w3400:u32)
    n1528 = Wait on Notification(notifier=w3407, ignore previous (F)=TRUE) -> (notification=w3405:cluster{"idx":i32, "lifetime":dbl}, error out=w3399:errorcluster)  [unwired: 2 in, 2 out]
    n1529 = Unbundle(w3405) -> ("idx"=w3404:i32, "lifetime"=w3403:dbl)
    n1530 = global read "GlobalVariables.vi" "TCP connected?"() -> (w3397:bool)
    n1531 = Subtract(x=w3400, y=w3401) -> (x-y=→"Communication loop(ms)":u32)
    n1532 = case shown="True" w3397 {
      tunnel: w3404 -> [_ w3416]
      tunnel: w3403 -> [_ w3415]
      tunnel: w3399 -> [w3408 w3412]
      tunnel: [w3408 w3409] -> w3398
      frame False {
      }
      frame True {
        n1533 = Number To Decimal String(number=w3416) -> (decimal integer string=w3424:string)  [unwired: 1 in]
        n1534 = call "TcpIDFGV.vi"("Error In"=w3412, "action"=enum16{"write", "read"}."read") -> ("Error Out"=w3411:errorcluster, "connection ID out"=w3422:refnum<k5>)  [unwired: 8 in]
        n1535 = Concatenate Strings("!idx:", w3424) -> (w3425:string)
        n1536 = call "TCP_WriteRead.vi"("error in (no error)"=w3411, "data in"=w3425, "connectin ID in"=w3422) -> ("error out"=w3410:errorcluster, "connectin ID out"=w3423:refnum<k5>)  [unwired: 4 in, 1 out]
        n1537 = Number To Fractional String(number=w3415, precision (6)=i16 2) -> (F-format string=w3414:string)  [unwired: 2 in]
        n1538 = Concatenate Strings("!lifetime:", w3414) -> (w3421:string)
        n1539 = call "TCP_WriteRead.vi"("error in (no error)"=w3410, "data in"=w3421, "connectin ID in"=w3423) -> ("error out"=w3409:errorcluster, "data out"=→"data out(communcation loop)":string)  [unwired: 4 in, 1 out]
      }
    }
  }
  n1540 = while {
    tunnel: w13 -> [w3436]
    shift-right: [w3427] -> _
    shift-left: w15 -> [w3434]
    shift-right: [w3429] -> _
    shift-left: w15 -> [w3428]
    i -> [w3430]
    stop <- w3431 stop-if-true
    # "Data display loop(30Hz)"
    n1541 = Wait on Notification(notifier=w3436, ignore previous (F)=FALSE) -> (notification=w3432:T13, error out=w3431:errorcluster)  [unwired: 2 in, 2 out]
    n1542 = Wait Until Next ms Multiple(millisecond multiple=u32 33) -> ()  [unwired: 1 out]
    n1543 = Tick Count (ms)() -> (millisecond timer value=w3427:u32)
    n1544 = Subtract(x=w3427, y=w3434) -> (x-y=→"display loop timing(ms)":u32)
    n1545 = case shown="No Error" w3431 {
      tunnel: w3432 -> [w3518 _]
      tunnel: w3428 -> [w3479 w3584]
      tunnel: [w3481 w3584] -> w3429
      tunnel: w3427 -> [w3478 _]
      frame No Error {
        w3455 = 0 ("index (row)")
        n1546 = Subtract(x=w3478, y=w3479) -> (x-y=w3480:u32)
        n1547 = Unbundle(w3518) -> ("CH1"=w3512:dbl[][], "CH2"=w3510:dbl[][], "CH3"=w3507:dbl[][], "CH4"=w3450:dbl[][], "Gain cluster"=w3456:cluster{"V1":dbl, "V2":dbl, "V3":dbl, "V4":dbl})
        n1548 = Unbundle By Name(w3456) -> ("V1"=w3474:dbl, "V2"=w3472:dbl, "V3"=w3470:dbl, "V4"=w3448:dbl)
        n1549 = Index Array(array=w3512, index (row)=w3455) -> (element=w3486:dbl[])  [unwired: 1 in]
        n1550 = Index Array(array=w3510, index (row)=w3455) -> (element=w3484:dbl[])  [unwired: 1 in]
        n1551 = Index Array(array=w3507, index (row)=w3455) -> (element=w3485:dbl[])  [unwired: 1 in]
        n1552 = Index Array(array=w3450, index (row)=w3455) -> (element=w3454:dbl[])  [unwired: 1 in]
        n1553 = call "RemoveDCBG.vi"("Channel"=enum16{"DC Only", "Ch1", "Ch2", "Ch3", "Ch4"}."Ch4", "WF in"=w3454) -> ("DC"=w3452:dbl, "WF out"=w3438:dbl[])  [unwired: 7 in, 1 out]
        n1554 = Greater?(x=w3480, y=u32 200) -> (0:w3482:bool)
        n1555 = call "CtrlVtoGain.vi"("CtrlV(V)"=w3448, "Channel"=enum16{"Ch1", "Ch2", "Ch3", "Ch4"}."Ch4") -> ("Gain"=w3437:dbl)  [unwired: 8 in, 1 out]
        n1556 = call "CtrlVtoGain.vi"("CtrlV(V)"=w3474, "Channel"=enum16{"Ch1", "Ch2", "Ch3"}."Ch1") -> ("Gain"=w3468:dbl)  [unwired: 8 in, 1 out]
        n1557 = call "RemoveDCBG.vi"("Channel"=enum16{"DC Only", "Ch1", "Ch2", "Ch3"}."Ch1", "WF in"=w3486) -> ("DC"=w3514:dbl, "WF out"=w3475:dbl[])  [unwired: 7 in, 1 out]
        n1558 = call "RemoveDCBG.vi"("Channel"=enum16{"DC Only", "Ch1", "Ch2", "Ch3"}."Ch2", "WF in"=w3484) -> ("DC"=w3509:dbl, "WF out"=w3476:dbl[])  [unwired: 7 in, 1 out]
        n1559 = call "CtrlVtoGain.vi"("CtrlV(V)"=w3472, "Channel"=enum16{"Ch1", "Ch2", "Ch3"}."Ch2") -> ("Gain"=w3463:dbl)  [unwired: 8 in, 1 out]
        n1560 = call "RemoveDCBG.vi"("Channel"=enum16{"DC Only", "Ch1", "Ch2", "Ch3"}."Ch3", "WF in"=w3485) -> ("DC"=w3506:dbl, "WF out"=w3477:dbl[])  [unwired: 7 in, 1 out]
        n1561 = call "CtrlVtoGain.vi"("CtrlV(V)"=w3470, "Channel"=enum16{"Ch1", "Ch2", "Ch3"}."Ch3") -> ("Gain"=w3459:dbl)  [unwired: 8 in, 1 out]
        n1562 = Add(x=w3438, y=w3452) -> (x+y=w3451:dbl[])
        n1563 = Less?(x=w3437, y=1.2) -> (x < y?=w3446:bool)
        n1564 = case shown="True" w3482 {
          tunnel: w3475 -> [_ w3545]
          tunnel: w3476 -> [_ w3548]
          tunnel: w3477 -> [_ w3547]
          tunnel: w3478 -> [_ w3563]
          tunnel: [w3527 w3563] -> w3481
          tunnel: w3479 -> [w3527 _]
          tunnel: w3468 -> [_ w3541]
          tunnel: w3463 -> [_ w3540]
          tunnel: w3459 -> [_ w3539]
          tunnel: w3438 -> [_ w3535]
          tunnel: w3437 -> [_ w3532]
          frame False {
          }
          frame True {
            n1565 = call "GetSNR(SubVI).vi"("Waveform"=w3545) -> ("SNR"=→"SNR1":dbl)  [unwired: 10 in]
            n1566 = Array Size(array=w3545) -> (size(s)=w3546:i32)
            n1567 = call "GetSNR(SubVI).vi"("Waveform"=w3548) -> ("SNR"=→"SNR2":dbl)  [unwired: 10 in]
            n1568 = call "GetSNR(SubVI).vi"("Waveform"=w3547) -> ("SNR"=→"SNR3":dbl)  [unwired: 10 in]
            n1569 = call "GetSNR(SubVI).vi"("Waveform"=w3535) -> ("SNR"=→"SNR4":dbl)  [unwired: 10 in]
            n1570 = global read "GlobalVariables.vi" "BG Idx2"() -> (w3534:i32)
            n1571 = Subtract(x=w3546, y=w3534) -> (x-y=w3533:i32)
            n1572 = Array Subset(array=w3545, index=w3534, length=w3533) -> (w3552:dbl[])
            n1573 = Array Subset(array=w3548, index=w3534, length=w3533) -> (w3554:dbl[])
            n1574 = Array Subset(array=w3547, index=w3534, length=w3533) -> (w3556:dbl[])
            n1575 = Array Subset(array=w3535, index=w3534, length=w3533) -> (w3536:dbl[])
            n1576 = Add Array Elements(numeric array=w3552) -> (sum=w3553:dbl)
            n1577 = Add Array Elements(numeric array=w3554) -> (sum=w3555:dbl)
            n1578 = Add Array Elements(numeric array=w3556) -> (sum=w3557:dbl)
            n1579 = Add Array Elements(numeric array=w3536) -> (sum=w3537:dbl)
            n1580 = Divide(x=w3553, y=w3541) -> (x/y=w3558:dbl)
            n1581 = Divide(x=w3555, y=w3540) -> (x/y=w3559:dbl)
            n1582 = Divide(x=w3557, y=w3539) -> (x/y=w3560:dbl)
            n1583 = Divide(x=w3537, y=w3532) -> (x/y=w3531:dbl)
            n1584 = Build Array(w3558, w3559, w3560, w3531) -> (w3561:dbl[])
            n1585 = Add Array Elements(numeric array=w3561) -> (sum=w3562:dbl)
            n1586 = Divide(x=w3561, y=w3562) -> (x/y=w3530:dbl[])
            n1587 = Index Array(array=w3530, index=2) -> (element=→"IntR3":dbl)
            n1588 = Index Array(array=w3530, index=1) -> (element=→"IntR2":dbl)
            n1589 = Index Array(array=w3530, index=0) -> (element=→"IntR1":dbl)
            n1590 = Index Array(array=w3530, index=4) -> (element=→"IntR4":dbl)
          }
        }
        n1591 = Add(x=w3475, y=w3514) -> (x+y=w3511:dbl[])
        n1592 = Add(x=w3476, y=w3509) -> (x+y=w3508:dbl[])
        n1593 = Add(x=w3477, y=w3506) -> (x+y=w3505:dbl[])
        n1594 = Less?(x=w3468, y=1.2 ("x")) -> (x < y?=w3466:bool)
        n1595 = Less?(x=w3463, y=1.2 ("x")) -> (x < y?=w3462:bool)
        n1596 = Less?(x=w3459, y=1.2 ("x")) -> (x < y?=w3458:bool)
        n1597 = case shown="False" w3458 {
          tunnel: [u32 16448250 ("Plot.Plot Color") u32 16711680 ("Plot.Plot Color")] -> w3457
          frame False {
          }
          frame True {
          }
        }
        n1598 = case shown="False" "Show BG removed?" {
          tunnel: w3512 -> [w3570 w3582]
          tunnel: w3511 -> [_ w3581]
          tunnel: [w3570 w3580] -> w3504
          tunnel: w3510 -> [w3569 w3579]
          tunnel: [w3569 w3578] -> w3498
          tunnel: w3508 -> [_ w3577]
          tunnel: w3507 -> [w3568 w3576]
          tunnel: [w3568 w3575] -> w3491
          tunnel: w3505 -> [_ w3574]
          tunnel: [w3567 w3573] -> w3444
          tunnel: w3451 -> [_ w3572]
          tunnel: w3450 -> [w3567 w3571]
          frame False {
          }
          frame True {
            n1599 = Build Array (concatenate)(w3576, w3574) -> (w3575:dbl[][])
            n1600 = Build Array (concatenate)(w3582, w3581) -> (w3580:dbl[][])
            n1601 = Build Array (concatenate)(w3579, w3577) -> (w3578:dbl[][])
            n1602 = Build Array (concatenate)(w3571, w3572) -> (w3573:dbl[][])
          }
        }
        "Channel 1" <- w3504
        "Channel 2" <- w3498
        "Channel 3" <- w3491
        "Channel 4" <- w3444
        n1603 = case shown="False" w3466 {
          tunnel: [u32 16448250 ("Plot.Plot Color") u32 16711680 ("Plot.Plot Color")] -> w3465
          frame False {
          }
          frame True {
          }
        }
        n1604 = case shown="False" w3462 {
          tunnel: [u32 16448250 ("Plot.Plot Color") u32 16711680 ("Plot.Plot Color")] -> w3461
          frame False {
          }
          frame True {
          }
        }
        n1605 = case shown="False" w3446 {
          tunnel: [u32 16448250 ("Plot.Plot Color") u32 16711680 ("Plot.Plot Color")] -> w3440
          frame False {
          }
          frame True {
          }
        }
        n1606 = Array Size(array=w3504) -> (size(s)=w3503:i32[])
        n1607 = Array Size(array=w3498) -> (size(s)=w3497:i32[])
        n1608 = Array Size(array=w3444) -> (size(s)=w3445:i32[])
        n1609 = Index Array(array=w3503) -> (element=w3502:i32)  [unwired: 1 in]
        n1610 = Index Array(array=w3497) -> (element=w3496:i32)  [unwired: 1 in]
        n1611 = Array Size(array=w3491) -> (size(s)=w3492:i32[])
        n1612 = Index Array(array=w3445) -> (element=w3439:i32)  [unwired: 1 in]
        n1613 = Index Array(array=w3492) -> (element=w3490:i32)  [unwired: 1 in]
        n1614 = property on="Channel 1" class="WFGraph (strict)"("Active Plot"=w3502, "Plot.Plot Color"=u32 16741120, "Plot.Line Style"=u8 1, "Plot.Line Width"=u8 2, "BG Color"=w3465) -> ()  [unwired: 2 in, 2 out]
        n1615 = property on="Channel 2" class="WFGraph (strict)"("Active Plot"=w3496, "Plot.Plot Color"=u32 16741120, "Plot.Line Style"=u8 1, "Plot.Line Width"=u8 2, "BG Color"=w3461) -> ()  [unwired: 2 in, 2 out]
        n1616 = property on="Channel 4" class="WFGraph (strict)"("Active Plot"=w3439, "Plot.Plot Color"=u32 16741120, "Plot.Line Style"=u8 1, "Plot.Line Width"=u8 2, "BG Color"=w3440) -> ()  [unwired: 2 in, 2 out]
        n1617 = property on="Channel 3" class="WFGraph (strict)"("Active Plot"=w3490, "Plot.Plot Color"=u32 16741120, "Plot.Line Style"=u8 1, "Plot.Line Width"=u8 2, "BG Color"=w3457) -> ()  [unwired: 2 in, 2 out]
      }
      frame Error {
        w3583 = u32 16448250 ("Plot Area:Colors:BG Color")
        n1618 = property on="Channel 1" class="WFGraph (strict)"("BG Color"=w3583) -> ()  [unwired: 2 in, 2 out]
        n1619 = property on="Channel 2" class="WFGraph (strict)"("BG Color"=w3583) -> ()  [unwired: 2 in, 2 out]
        n1620 = property on="Channel 3" class="WFGraph (strict)"("BG Color"=w3583) -> ()  [unwired: 2 in, 2 out]
      }
    }
    "DisplayLoop" <- w3430
  }
  n1621 = disable-structure "Diagram Disable Structure" shown="Disabled" {
    frame Disabled {
      w3585 = T48 {"Horizontal"=500, "Vertical"=100}  # Top Left Corner
      n1622 = Control Help Window(0:w3585, 1:TRUE ("Show")) -> ()
      n1623 = call <vilib>:"TDMS - File Viewer.vi"() -> ()  [unwired: 6 in, 2 out]
    }
    frame Enabled {
    }
  }
  n1624 = while {
    tunnel: w65 -> [w3599]
    tunnel: w55 -> [w3598]
    tunnel: [w3597] -> w63
    tunnel: w19 -> [w3596]
    tunnel: [w3595] -> w59
    tunnel: w39 -> [w3593]
    tunnel: w48 -> [w3592]
    tunnel: w35 -> [w3587]
    stop <- w3590 stop-if-true
    # "acquire data and send it to processing loop"
    # "Data Aquisition Loop"
    n1625 = event shown="[1] <Start digitizer>: User Event" {
      selector: w3598 -> [_ _]
      dyn-events: [_ _] -> w3597
      timeout: 20 -> [_ _]
      tunnel: w3599 -> [w3605 w3615]
      tunnel: [w3600 _] -> w3590
      tunnel: w3596 -> [w3604 w3622]
      tunnel: [w3604 w3621] -> w3595
      tunnel: w3593 -> [_ w3619]
      tunnel: w3592 -> [w3603 w3614]
      tunnel: w3587 -> [_ w3612]
      event Timeout {
        # "use queue to stop data loop\nwhen queue ref is released, error will stop this loop"
        n1626 = event-data() -> ()  [unwired: 1 in, 3 out]
        n1627 = Get Queue Status(queue=w3605) -> (error out=w3602:errorcluster)  [unwired: 2 in, 7 out]
        n1628 = Get Queue Status(queue=w3603) -> (error out=w3601:errorcluster)  [unwired: 2 in, 7 out]
        n1629 = Merge Errors(w3602, w3601) -> (w3600:errorcluster)
      }
      event User Event {
        w3620 = enum16{"Write", "Read"}."Read" ("Operation")
        n1630 = event-data() -> ("Time"=→"RunStartTime":u32)  [unwired: 1 in, 3 out]
        n1631 = call "FLImDAQ_FGV.vi"() -> ("Read data"=w3617:T6)  [unwired: 10 in, 1 out]
        n1632 = call "Digitizer1_FGV.vi"("Operation (Read)"=w3620) -> ("Read data"=w3611:refnum<k15>)  [unwired: 9 in, 1 out]
        n1633 = call "Digitizer2_FGV.vi"("Operation (Read)"=w3620) -> ("Read data"=w3618:refnum<k15>)  [unwired: 9 in, 1 out]
        n1634 = Unbundle By Name(w3617) -> ("Waveform to Avg"=w3616:i16)
        n1635 = property on="Property Node" class="niScope"(reference=w3611) -> (reference out=w3610:refnum<k15>, "Vertical Range"=w3609:dbl, "Vertical Offset"=w3608:dbl)  [unwired: 1 in, 1 out]
        n1636 = Tick Count (ms)() -> (millisecond timer value=w3607:u32)
        n1637 = while {
          tunnel: w3622 -> [w3682]
          tunnel: [w3681] -> w3621
          tunnel: w3618 -> [w3675]
          tunnel: w3610 -> [w3674]
          tunnel: w3619 -> [w3673]
          shift-right: [w3641] -> _
          shift-left: u32 0 ("millisecond timer value") -> [w3667]
          tunnel: w3616 -> [w3665]
          tunnel: w3615 -> [w3663]
          tunnel: w3614 -> [w3661]
          tunnel: w3612 -> [w3654]
          tunnel: w3609 -> [w3651]
          tunnel: w3608 -> [w3652]
          shift-right: [w3646] -> _
          shift-left: w3607 -> [w3645]
          i -> [w3637]
          stop <- w3644 stop-if-true
          w3633 = enum16{"write", "read"}."read" ("action")
          w3668 = 65536
          # "enqueue V"
          # "enqueue ch3 data"
          # "enqueue ch1&2 data"
          # "acquire ch3"
          # "acquire ch1&2"
          # "send data for processing"
          n1638 = Multiply(x=w3665, y=w3637) -> (x*y=w3630:i32)
          "Fetch Record #" <- w3630
          n1639 = property on="Property Node" class="niScope"(reference=w3674, "Fetch Record Number"=w3630) -> (reference out=w3686:refnum<k15>, error out=w3685:errorcluster, "Records Done"=w3653:i32)  [unwired: 1 in]
          n1640 = Subtract(x=w3653, y=w3630) -> (x-y=→"Record Backlog":i32)
          n1641 = call-poly <instrlib>:"niScope Fetch (poly).vi"("timeout"=0.25, "error in"=w3685, "channels"="0,1", "instrument handle"=w3686) -> ("error out"=w3627:errorcluster, "wfm"=w3628:i16[][], "wfm info"=w3650:T49)  [unwired: 4 in, 1 out]
          n1642 = property on="Property Node" class="niScope"(reference=w3675, "Fetch Record Number"=w3630) -> (reference out=w3679:refnum<k15>, error out=w3676:errorcluster, "Records Done"=w3631:i32)  [unwired: 1 in]
          n1643 = Divide(x=w3628, y=w3668) -> (x/y=w3640:dbl[][])
          n1644 = Tick Count (ms)() -> (millisecond timer value=w3641:u32)
          n1645 = Subtract(x=w3631, y=w3630) -> (x-y=→"Record Backlog 2":i32)
          n1646 = Subtract(x=w3641, y=w3667) -> (x-y=→"Aquisition loop timing(ms)":u32)
          n1647 = Subtract(x=w3641, y=w3645) -> (x-y=w3649:u32)
          n1648 = Multiply(x=w3640, y=w3651) -> (x*y=w3672:dbl[][])
          n1649 = call-poly <instrlib>:"niScope Fetch (poly).vi"("timeout"=0.25, "error in"=w3676, "channels"="0,1", "instrument handle"=w3679) -> ("error out"=w3626:errorcluster, "wfm"=w3669:i16[][])  [unwired: 4 in, 2 out]
          n1650 = Greater?(x=w3649, y=u32 1000) -> (0:w3647:bool)
          n1651 = Add(x=w3672, y=w3652) -> (x+y=w3662:dbl[][])
          n1652 = case shown="True" w3647 {
            tunnel: w3650 -> [_ w3695]
            tunnel: w3641 -> [_ w3694]
            tunnel: [w3688 w3694] -> w3646
            tunnel: w3645 -> [w3688 _]
            tunnel: [errorcluster {"status"=FALSE, "code"=0, "source"=""} ("error constant") w3691] -> w3642
            frame False {
            }
            frame True {
              # "[Covers: REQ29]"
              n1653 = call "CheckFrequency(SubVI).vi"("wfm info"=w3695) -> ("f (Hz)"=w3693:dbl)  [unwired: 10 in]
              "Laser f (Hz)" <- w3693
              n1654 = local read "Laser Rep Rate"() -> (w3690:dbl)
              n1655 = Increment(x=w3690) -> (x+1=w3689:dbl)
              n1656 = Greater?(x=w3693, y=w3689) -> (0:w3692:bool)
              n1657 = case shown="True" w3692 {
                tunnel: [errorcluster {"status"=FALSE, "code"=0, "source"=""} ("error constant") errorcluster {"status"=TRUE, "code"=0, "source"=""} ("error constant")] -> w3691
                frame False {
                }
                frame True {
                }
              }
            }
          }
          n1658 = Divide(x=w3669, y=w3668) -> (x/y=w3671:dbl[][])
          n1659 = Enqueue Element(queue=w3663, element=w3662, error in (no error)=w3627) -> (error out=w3625:errorcluster)  [unwired: 1 in, 2 out]
          n1660 = Multiply(x=w3671, y=w3651) -> (x*y=w3670:dbl[][])
          n1661 = Add(x=w3670, y=w3652) -> (x+y=w3660:dbl[][])
          n1662 = Enqueue Element(queue=w3661, element=w3660, error in (no error)=w3626) -> (error out=w3624:errorcluster)  [unwired: 1 in, 2 out]
          n1663 = Merge Errors(w3625, w3624) -> (w3623:errorcluster)
          n1664 = call "V1FGV.vi"("Error In"=w3623, "action (write)"=w3633) -> ("Error Out"=w3658:errorcluster, "V1 out"=w3656:dbl)  [unwired: 8 in]
          n1665 = call "V2FGV.vi"("Error In"=w3658, "action(write)"=w3633) -> ("Error Out"=w3657:errorcluster, "V2 out"=w3655:dbl)  [unwired: 8 in]
          n1666 = call "V3FGV.vi"("Error In"=w3657, "action(write)"=w3633) -> ("Error Out"=w3636:errorcluster, "V3 out"=w3635:dbl)  [unwired: 8 in]
          n1667 = call "V4FGV.vi"("Error In"=w3636, "action(write)"=w3633, "V3 in"=w3635) -> ("Error Out"=w3634:errorcluster, "V3 out"=w3632:dbl)  [unwired: 7 in]
          n1668 = Bundle("V1 out"=w3656, "V2 out"=w3655, "V3 out"=w3635, "V3 out"=w3632) -> (w3639:T50)  [unwired: 1 in]
          n1669 = Bundle(w3637, w3662, w3660, w3639) -> (w3664:T51)  [unwired: 1 in]
          n1670 = Enqueue Element(queue=w3654, element=w3639, error in (no error)=w3634) -> (error out=w3638:errorcluster)  [unwired: 1 in, 2 out]
          n1671 = Send Notification(notification=w3664, notifier=w3682, error in (no error)=w3638) -> (notifier out=w3681:refnum<notifier>, error out=w3643:errorcluster)
          n1672 = Merge Errors(w3642, w3643) -> (w3659:errorcluster)
          n1673 = case shown="Error .." w3659 {
            selector: w3659 -> [w3698 w3699]
            tunnel: w3673 -> [_ w3702]
            tunnel: [w3698 w3699] -> w3644
            frame No Error {
            }
            frame Error {
              # "Send user event to signal aquisition has stoped"
              n1674 = Generate User Event(priority (normal)=usereventprio."high priority", user event=w3702, event data cluster=TRUE ("event data")) -> ()  [unwired: 1 in, 2 out]
            }
          }
          "aquisition loop Error Out" <- w3644
          "Auisition Loop idx" <- w3637
        }
      }
    }
    n1675 = Unbundle By Name(w3590) -> ("status"=w3589:bool)
    n1676 = Not(x=w3589) -> (.not. x?=w3588:bool)
    n1677 = local write "Aq Loop?"(w3588) -> ()
    "Aq Loop?" <- TRUE ("Aq L?")
  }
  n1678 = while {
    tunnel: w19 -> [w3750]
    shift-right: [w3713] -> _
    shift-left: _ -> [w3746]
    tunnel: [w3704] -> w1 mode=indexing
    i -> [w3730]
    stop <- w3710 stop-if-true
    # "Channel 3"
    # "Channel 2"
    # "Channel 1"
    # "use FGV for gain value"
    # "stop on error"
    # "Gain adjustment and Data processing"
    n1679 = Tick Count (ms)() -> (millisecond timer value=w3713:u32)
    n1680 = Wait on Notification(notifier=w3750, ignore previous (F)=TRUE) -> (notification=w3724:T14, error out=w3703:errorcluster)  [unwired: 2 in, 2 out]
    n1681 = Subtract(x=w3713, y=w3746) -> (x-y=→"PID loop timing(ms)":u32)
    n1682 = Unbundle(w3724) -> ("CH1&2"=w3740:dbl[][], "CH3"=w3739:dbl[][])  [unwired: 2 out]
    n1683 = call "SeperateChanData.vi"("Input (Ch1&2)"=w3740) -> ("Ch1"=w3735:dbl[][], "Ch2"=w3733:dbl[][])
    n1684 = call "SeperateChanData.vi"("Input (Ch1&2)"=w3739) -> ("Ch1"=w3729:dbl[][], "Ch2"=w3722:dbl[][])
    n1685 = call "AvgArrayTimeCritical.vi"("2D array"=w3735) -> ("1D Avg"=w3734:dbl[])  [unwired: 10 in]
    n1686 = call "AvgArrayTimeCritical.vi"("2D array"=w3733) -> ("1D Avg"=w3744:dbl[])  [unwired: 10 in]
    n1687 = call "AvgArrayTimeCritical.vi"("2D array"=w3729) -> ("1D Avg"=w3741:dbl[])  [unwired: 10 in]
    n1688 = call "AvgArrayTimeCritical.vi"("2D array"=w3722) -> ("1D Avg"=w3721:dbl[])  [unwired: 10 in]
    n1689 = Array Max & Min(array=w3734) -> (max value=w3732:dbl)  [unwired: 3 out]
    n1690 = Array Max & Min(array=w3744) -> (max value=w3731:dbl)  [unwired: 3 out]
    n1691 = Array Max & Min(array=w3741) -> (max value=w3714:dbl)  [unwired: 3 out]
    n1692 = Array Max & Min(array=w3721) -> (max value=w3719:dbl)  [unwired: 3 out]
    n1693 = local read "Auto gain ch4"() -> (w3720:bool)
    n1694 = local read "Auto gain ch1"() -> (w3738:bool)
    n1695 = local read "Auto gain ch2"() -> (w3737:bool)
    n1696 = local read "Auto gain ch3"() -> (w3736:bool)
    n1697 = case shown="False" w3720 {
      tunnel: w3719 -> [_ w3797]
      tunnel: "V target(1.0)" -> [_ w3795]
      tunnel: [FALSE w3792] -> w3717
      tunnel: [0.0 ("CtrlV") w3787] -> w3718
      frame False {
        # "Manual control"
      }
      frame True {
        # "PID control"
        n1698 = global read "GlobalVariables.vi" "Ch4GainLim(Log)"() -> (w3798:cluster{"GainMax":dbl, "GainMin":dbl})
        n1699 = call-poly <vilib>:"PID.vi"("output range"=w3798, "PID gains"="Ch4 PID gains", "process variable"=w3797, "setpoint"=w3795) -> ("output"=w3796:dbl)  [unwired: 6 in, 1 out]
        n1700 = Power Of 10(x=w3796) -> (10^x=w3788:dbl)
        "Gain4" <- w3788
        n1701 = call "V4FGV.vi"("action(write)"=enum16{"write", "read"}."read") -> ("Error Out"=w3791:errorcluster, "V3 out"=w3793:dbl)  [unwired: 9 in]
        n1702 = call "GainToCtrlV.vi"("Gain"=w3788, "Channel"=enum16{"Ch1", "Ch2", "Ch3", "Ch4"}."Ch4") -> ("CtrlV"=w3787:dbl)  [unwired: 8 in, 1 out]
        n1703 = call "V4FGV.vi"("Error In"=w3791, "V3 in"=w3787) -> ()  [unwired: 8 in, 2 out]
        n1704 = local write "V 4"(w3787) -> ()
        n1705 = Not Equal?(x=w3787, y=w3793) -> (x != y?=w3792:bool)
      }
    }
    n1706 = case shown="True" w3738 {
      tunnel: "V target(1.0)" -> [_ w3812]
      tunnel: w3732 -> [_ w3809]
      tunnel: [0.0 ("CtrlV") w3801] -> w3711
      tunnel: [FALSE w3803] -> w3728
      frame False {
        # "Manual control"
      }
      frame True {
        # "PID control"
        n1707 = global read "GlobalVariables.vi" "Ch1GainLim(Log)"() -> (w3808:cluster{"GainMax":dbl, "GainMin":dbl})
        n1708 = call-poly <vilib>:"PID.vi"("output range"=w3808, "PID gains"="Ch1 PID gains", "process variable"=w3809, "setpoint"=w3812) -> ("output"=w3807:dbl)  [unwired: 6 in, 1 out]
        n1709 = Power Of 10(x=w3807) -> (10^x=w3806:dbl)
        "Gain1" <- w3806
        n1710 = call "V1FGV.vi"("action (write)"=enum16{"write", "read"}."read") -> ("Error Out"=w3802:errorcluster, "V1 out"=w3804:dbl)  [unwired: 9 in]
        n1711 = call "GainToCtrlV.vi"("Gain"=w3806, "Channel"=enum16{"Ch1", "Ch2", "Ch3"}."Ch1") -> ("CtrlV"=w3801:dbl)  [unwired: 8 in, 1 out]
        n1712 = local write "V 1"(w3801) -> ()
        n1713 = call "V1FGV.vi"("Error In"=w3802, "V1 in"=w3801) -> ()  [unwired: 8 in, 2 out]
        n1714 = Not Equal?(x=w3801, y=w3804) -> (x != y?=w3803:bool)
      }
    }
    n1715 = case shown="True" w3737 {
      tunnel: w3731 -> [_ w3839]
      tunnel: "V target(1.0)" -> [_ w3840]
      tunnel: [FALSE w3833] -> w3727
      tunnel: [0.0 ("CtrlV") w3829] -> w3723
      frame False {
        # "Manual control"
      }
      frame True {
        # "PID control"
        n1716 = global read "GlobalVariables.vi" "Ch2GainLim(Log)"() -> (w3837:cluster{"GainMax":dbl, "GainMin":dbl})
        n1717 = call-poly <vilib>:"PID.vi"("output range"=w3837, "PID gains"="Ch2 PID gains", "process variable"=w3839, "setpoint"=w3840) -> ("output"=w3836:dbl)  [unwired: 6 in, 1 out]
        n1718 = Power Of 10(x=w3836) -> (10^x=w3834:dbl)
        "Gain2" <- w3834
        n1719 = call "V2FGV.vi"("action(write)"=enum16{"write", "read"}."read") -> ("Error Out"=w3830:errorcluster, "V2 out"=w3831:dbl)  [unwired: 9 in]
        n1720 = call "GainToCtrlV.vi"("Gain"=w3834, "Channel"=enum16{"Ch1", "Ch2", "Ch3"}."Ch2") -> ("CtrlV"=w3829:dbl)  [unwired: 8 in, 1 out]
        n1721 = local write "V 2"(w3829) -> ()
        n1722 = call "V2FGV.vi"("Error In"=w3830, "V2 in"=w3829) -> ()  [unwired: 8 in, 2 out]
        n1723 = Not Equal?(x=w3829, y=w3831) -> (x != y?=w3833:bool)
      }
    }
    n1724 = case shown="True" w3736 {
      tunnel: w3714 -> [_ w3824]
      tunnel: "V target(1.0)" -> [_ w3821]
      tunnel: [FALSE w3817] -> w3726
      tunnel: [0.0 ("CtrlV") w3815] -> w3725
      frame False {
        # "Manual control"
      }
      frame True {
        # "PID control"
        n1725 = global read "GlobalVariables.vi" "Ch3GainLim(Log)"() -> (w3825:cluster{"GainMax":dbl, "GainMin":dbl})
        n1726 = call-poly <vilib>:"PID.vi"("output range"=w3825, "PID gains"="Ch3 PID gains", "process variable"=w3824, "setpoint"=w3821) -> ("output"=w3823:dbl)  [unwired: 6 in, 1 out]
        n1727 = Power Of 10(x=w3823) -> (10^x=w3820:dbl)
        "Gain3" <- w3820
        n1728 = call "V3FGV.vi"("action(write)"=enum16{"write", "read"}."read") -> ("Error Out"=w3816:errorcluster, "V3 out"=w3818:dbl)  [unwired: 9 in]
        n1729 = call "GainToCtrlV.vi"("Gain"=w3820, "Channel"=enum16{"Ch1", "Ch2", "Ch3"}."Ch3") -> ("CtrlV"=w3815:dbl)  [unwired: 8 in, 1 out]
        n1730 = local write "V 3"(w3815) -> ()
        n1731 = call "V3FGV.vi"("Error In"=w3816, "V3 in"=w3815) -> ()  [unwired: 8 in, 2 out]
        n1732 = Not Equal?(x=w3815, y=w3818) -> (x != y?=w3817:bool)
      }
    }
    n1733 = call "LabJack_FGV.vi"("Operation(Read)"=enum16{"Write", "Read"}."Read" ("Operation"), "error in (no error)"=w3703) -> ("error out"=w3712:errorcluster, "Read data"=w3748:i32)  [unwired: 8 in]
    n1734 = flat-sequence {
      tunnel: [w3752] -> w3709
      tunnel: w3703 -> [_]
      frame #0 {
        n1735 = Tick Count (ms)() -> (millisecond timer value=w3752:u32)
      }
    }
    n1736 = case "Channel 1" shown="True" w3728 {
      tunnel: w3712 -> [w3778 w3784]
      tunnel: w3748 -> [w3777 w3783]
      tunnel: [w3778 w3779] -> w3707
      tunnel: [w3777 w3782] -> w3743
      tunnel: w3711 -> [_ w3780]
      frame False {
        # "Do nothing"
      }
      frame True {
        # "request V\nupdate FGV"
        n1737 = global read "GlobalVariables.vi" "Ch1 LJ pin"() -> (w3781:string)
        n1738 = call "LJM_eWriteName.vi"("Handle In"=w3783, "Name"=w3781, "Value"=w3780, "error in"=w3784) -> ("Handle Out"=w3782:i32, "error out"=w3779:errorcluster)  [unwired: 10 in]
      }
    }
    n1739 = case "Channel 2" shown="True" w3727 {
      tunnel: w3707 -> [w3769 w3776]
      tunnel: [w3769 w3771] -> w3706
      tunnel: w3743 -> [w3770 w3775]
      tunnel: [w3770 w3774] -> w3742
      tunnel: w3723 -> [_ w3772]
      frame False {
        # "Do nothing"
      }
      frame True {
        # "request V\nupdate FGV"
        n1740 = global read "GlobalVariables.vi" "Ch2 LJ pin"() -> (w3773:string)
        n1741 = call "LJM_eWriteName.vi"("Handle In"=w3775, "Name"=w3773, "Value"=w3772, "error in"=w3776) -> ("Handle Out"=w3774:i32, "error out"=w3771:errorcluster)  [unwired: 10 in]
      }
    }
    n1742 = case "Channel 3" shown="True" w3726 {
      tunnel: w3706 -> [w3762 w3768]
      tunnel: [w3762 w3764] -> w3705
      tunnel: w3742 -> [w3761 w3767]
      tunnel: w3725 -> [_ w3765]
      tunnel: [w3761 w3763] -> w3716
      frame False {
        # "Do nothing"
      }
      frame True {
        # "request V\nupdate FGV"
        n1743 = global read "GlobalVariables.vi" "Ch3 LJ pin"() -> (w3766:string)
        n1744 = call "LJM_eWriteName.vi"("Handle In"=w3767, "Name"=w3766, "Value"=w3765, "error in"=w3768) -> ("Handle Out"=w3763:i32, "error out"=w3764:errorcluster)  [unwired: 10 in]
      }
    }
    n1745 = case "Channel 4" shown="True" w3717 {
      tunnel: w3705 -> [w3754 w3760]
      tunnel: w3716 -> [w3753 w3759]
      tunnel: [w3754 w3755] -> w3710
      tunnel: [w3753 w3758] -> _
      tunnel: w3718 -> [_ w3756]
      frame False {
        # "Do nothing"
      }
      frame True {
        # "request V\nupdate FGV"
        n1746 = global read "GlobalVariables.vi" "Ch4 LJ pin"() -> (w3757:string)
        n1747 = call "LJM_eWriteName.vi"("Handle In"=w3759, "Name"=w3757, "Value"=w3756, "error in"=w3760) -> ("Handle Out"=w3758:i32, "error out"=w3755:errorcluster)  [unwired: 10 in]
      }
    }
    "PID loop error out" <- w3710
    n1748 = flat-sequence {
      tunnel: [w3751] -> w3708
      tunnel: w3710 -> [_]
      frame #0 {
        n1749 = Tick Count (ms)() -> (millisecond timer value=w3751:u32)
      }
    }
    n1750 = Subtract(x=w3708, y=w3709) -> (x-y=w3704:u32)
    "LJ process (ms)" <- w3704
    "PID loop" <- w3730
  }
  "LJ time(ms)" <- w1
  n1751 = Release Notifier(notifier=w16, error in (no error)=w49) -> (error out=w50:errorcluster)  [unwired: 1 in, 2 out]
  n1752 = Release Notifier(notifier=w17, error in (no error)=w38) -> (error out=w43:errorcluster)  [unwired: 1 in, 2 out]
  n1753 = call <vilib>:"Simple Error Handler.vi"("error in (no error)"=w50) -> ()  [unwired: 4 in, 5 out]
  n1754 = call <vilib>:"Simple Error Handler.vi"("error in (no error)"=w43) -> ()  [unwired: 4 in, 5 out]
  n1755 = Unregister For Events(event registration refnum=w46, error in=w4) -> (error out=w52:errorcluster)
  n1756 = Destroy User Event(user event=w39, error in=w52) -> (error out=w3:errorcluster)
  n1757 = Close File(refnum=w21, error in=w3) -> ()  [unwired: 2 out]
  n1758 = Release Notifier(notifier=w59, error in (no error)=w58) -> (error out=w57:errorcluster)  [unwired: 1 in, 2 out]
  n1759 = Unregister For Events(event registration refnum=w63, error in=w61) -> (error out=w62:errorcluster)
  n1760 = call <vilib>:"Simple Error Handler.vi"("error in (no error)"=w57) -> ()  [unwired: 4 in, 5 out]
  n1761 = Destroy User Event(user event=w53, error in=w62) -> ()  [unwired: 1 out]
